vi "Datastream.vi"(0 "Tab Main":T4(tab)=enum."Trap Control (RF)") -> ()   [LabVIEW 2013]
uses:
  <vilib>/rvi/interface/nirviMethod/nirviMethod.xnode
  <vilib>/express/express analysis/Spectral/XNode/ExpressSpectralMeasurementsBlockNode.xnode
  <vilib>/rvi/interface/nirviReadWriteControl/nirviReadWriteControl.xnode
  <vilib>/Analysis/NI_AALBase.lvlib
  <vilib>/express/express analysis/Spectral/Block/exnSpectralBlock spectral measurements PSD poly.vi
  <vilib>/Platform/TimedLoop/XDataNode/XDataNode.xnode
  <vilib>/Platform/TimedLoop/XDataNode/nitl_modes.ctl
  <vilib>/Platform/TimedLoop/XDataNode/XDNodeRunTimeDep.lvlib
  <vilib>/Platform/TimedLoop/XDataNode/wakeup.ctl
  <vilib>/Platform/TimedLoop/XDataNode/timing_clust.ctl
  <vilib>/userdefined/High Color/nirio_resource_hc.ctl
  openfpgaref.8.6.ctl
  <vilib>/Utility/miscctls.llb/LVMinMaxIncTypeDef.ctl
  <vilib>/vision/NI_Vision_Development_Module.lvlib
  <vilib>/rvi/interface/nirviCloseFPGA/nirviCloseFPGA.xnode
  <vilib>/Analysis/baseanly.llb/Mean (DBL).vi
  <vilib>/rvi/errors/niLvFpgaMergeErrorWithErrorCode.vi
  <vilib>/rvi/errors/niLvFpgaAdjustHostInterfaceError.vi
  <vilib>/FPGAPlugInAG/PCIe-7852R/niLvFpga_ReadFifo_PCIe-7852R.vi
  <vilib>/rvi/interface/nirviOpenFPGA/nirviOpenFPGA.xnode
  openfpgaref.initrf.ctl
  FPGA Bitfiles/UHR-FleezersInst_FPGATarget_intitializeRF201804.lvbitx
  <vilib>/FPGAPlugInAG/PCIe-7852R/niLvFpga_ConfigureFifo_PCIe-7852R.vi
  <vilib>/FPGAPlugInAG/PCIe-7852R/niLvFpga_Run_PCIe-7852R.vi
  <vilib>/FPGAPlugInAG/PCIe-7852R/niLvFpga_Close_PCIe-7852R.vi
  <vilib>/FPGAPlugInAG/PCIe-7852R/niLvFpga_Open_PCIe-7852R.vi
  <vilib>/FPGAPlugInAG/PCIe-7852R/niLvFpga_Reset_PCIe-7852R.vi
  NiFpgaLv.dll
  <vilib>/Utility/error.llb/Error Cluster From Error Code.vi
  <vilib>/FPGAPlugInAG/PCIe-7852R/niLvFpga_Abort_PCIe-7852R.vi
  FPGA Bitfiles/UHR-FleezersInst_FPGATarget_UHR-Fleezers_Leonardo042018V4.lvbitx
  <vilib>/express/express analysis/Spectral/Block/exnSpectralBlock spectral measurements PSD WFM.vi
  <vilib>/Waveform/WDTOps.llb/WDT Append Waveforms DBL.vi
  FPGA Bitfiles/UHR-FleezersInst_FPGATarget_UHR-FleezersCont_IqK95Pvv9lYv5.3.lvbitx
panel:
  out "Actual setpoint":fxp<+/-,16,1> format="%.16g"
  in  "Target Force (pN)":dbl=10.5
  out "Current deltaFreq":dbl=20.03845214843774
  out "Tether Extension (nm, calculated)":dbl=1280.0838354247721 format="%0.2f"
  out "Trap X (AI1)":T1={"Trap 1"=0.030792236328125, "Trap 2"=-0.011322021484375}
  out "Trap Positions":waveform(dbl)[](graph)=[{"t0"=timestamp(2751.0000000002074 s since 1904-01-01), "dt"=0.15, "Y"=[-4.784226348419907e-12, -4.784226348419907e-12], "attributes"=variant("NI_ChannelName"=variant(string "Trap 1 Pos."))}, {"t0"=timestamp(2751.0000000002074 s since 1904-01-01), "dt"=0.15, "Y"=[0.0, 0.0], "attributes"=variant("NI_ChannelName"=variant(string "Trap 2 Pos."))}]
  out "Action (%)":dbl(knob)=-100.0 scale=-100.0..100.0
  out "Sigma/Mean 2":dbl=nan caption="Sigma/Mean" format="%#_2g"
  out "Rate sigma (Hz) 2":dbl caption="Sigma (Hz)" format="%0.2f"
  out "APD 2 Rate (Hz)":dbl format="%#_3p"
  out "Waveform Graph":dbl[](graph)=[5.0, 4.0, 2.0, 2.0, 5.0, 3.0, 2.0, 4.0, 0.0, 5.0, 4.0, 3.0, 5.0, 2.0, 4.0, 1.0, 5.0, 3.0, 0.0, 2.0, 2.0, 4.0, 2.0, 1.0, 2.0, 8.0, 2.0, 4.0, 4.0, 3.0, 3.0, 1.0, 5.0, 5.0, 3.0, 2.0, 7.0, 2.0, 4.0, 4.0, 1.0, 1.0, 3.0, 4.0, 3.0, 9.0, 0.0, 6.0, 4.0, 5.0, 2.0, 4.0, 4.0, 4.0, 4.0, 2.0, 3.0, 6.0, 3.0, 4.0, 4.0, 5.0, 5.0, 8.0, 5.0, 4.0, 4.0, 7.0, 4.0, 3.0, 1.0, 4.0, 5.0, 4.0, 2.0, 3.0, 3.0, 1.0, 2.0, 1.0] caption="APD Line Scan"
  in  "APD Ave N":dbl=10.0
  out "Int. Time (s)":dbl=3.0
  out "Sigma/Mean":dbl=nan format="%#_2g"
  out "Rate sigma (Hz)":dbl caption="Sigma (Hz)" format="%0.2f"
  in  "Tab Control 6":T2(tab)
  in  "APD 2 Offset":dbl
  in  "APD 1 Offset":dbl
  out "RMS (Ang)":dbl=0.5623803485708063 format="%_2g"
  in  "Bead Sep. Int. Time (s)":dbl=5.0 caption="Int. Time (s)"
  in  "Offset (nm)":dbl
  out "Mean":dbl=1.039039384389187 caption="Mean (pN)" format="%#_3g"
  out "Force":waveform(dbl)[](graph)=[{"t0"=timestamp(2751.0000000002074 s since 1904-01-01), "dt"=0.15, "Y"=[-1.511324813843883, -1.510992142739303], "attributes"=variant("NI_ChannelName"=variant(string "T1 X"))}, {"t0"=timestamp(2751.0000000002074 s since 1904-01-01), "dt"=0.15, "Y"=[0.567256952484741, 0.566583628488821], "attributes"=variant("NI_ChannelName"=variant(string "T2 X"))}]
  out "APD Chart":waveform(dbl)[](graph)=[{"t0"=timestamp(2751.0000000002074 s since 1904-01-01), "dt"=0.02, "Y"=[0.0, 0.0, 0.0, 0.0, 0.0, 0.0, 0.0, 0.0, 0.0, 0.0, 0.0, 0.0, 0.0, 0.0, 0.0], "attributes"=variant("NI_ChannelName"=variant(string "APD 1"))}, {"t0"=timestamp(2751.0000000002074 s since 1904-01-01), "dt"=0.02, "Y"=[0.0, 0.0, 0.0, 0.0, 0.0, 0.0, 0.0, 0.0, 0.0, 0.0, 0.0, 0.0, 0.0, 0.0, 0.0], "attributes"=variant("NI_ChannelName"=variant(string "APD 2"))}]
  in  "Calibration":u16(ring)=2 items=["None", "Position", "Force"]
  out "T1 X":dbl=-1.511158478291593 caption="T1 X (pN)" format="%0.2f"
  out "T2 X":dbl=0.5669202904867809 caption="T2 X (pN)" format="%0.2f"
  out "Bead Separation":waveform(dbl)(graph)={"t0"=timestamp(2751.0000000002074 s since 1904-01-01), "dt"=0.15, "Y"=[13.487296816964651, 13.48037403257866], "attributes"=variant("NI_ChannelName"=variant(string "T1 X"))}
  out "Bead Mean (nm)":dbl=13.506045465071283 caption="Mean (nm)" format="%0.2f"
  out "Difference":dbl=0.9442381878048121 caption="Difference (pN)" format="%.2g"
  out "APD 2":T3(plugin-control) caption="APD 2 (Cy5)"
  out "APD 1":T3(plugin-control) caption="APD 1 (Cy3)"
  out "Detection Laser Y":T3(plugin-control)
  out "Detection Laser X":T3(plugin-control)
  out "Saved APD":dbl[][](graph) caption="Most Recent Time Trace"
  out "Trap Delta Graph":dbl[](graph)=[195.1277413890926, 194.94364879261857, 195.1277413890926, 194.94364879261857, 195.1457432924014, 195.43991875047658, 195.71957055288706, 195.22283466303207, 195.1027968921228, 194.96782146458364, 195.3831317750734, 195.1011774517534, -429.02175121270034, -525.1398207234975, -525.9023663780167, -523.4888823406284, -525.9473090361441, -523.7419318917771, -524.0949760575616, -524.4391559902058, -526.3291828811887, -525.104560125752, -527.5180711612056, -523.2999128001393, -526.5498888630073, -524.7083600570088, -522.5173776695501, -525.5444120291477, -524.0271757467506, -525.2107691195308, -523.9441905667804, -526.0104515834323, -524.5961470121938, -524.5803642777907, -526.0323679419505, -525.3149691620972, 195.79450497322807, 195.82853060793795, 196.68216279584308, 196.2898441960903, 196.3201650436859, 195.81353342606087, 195.5969971411281, 195.85479324517004, 196.28760584932735, 195.71415572150602, 195.53926387431486, 195.04762359603245, 195.79764921332765, 195.88378244963528, 195.56420539798899, 195.741794878524, 195.6032010481766, 195.13266085703762, 194.68322569301654, 195.35368995164265, 195.60186007511763, 194.99358806317844, 195.21177044926304, 195.52777221791428, 194.99090803446128, 195.33201299997344, 195.42467754091498, 195.65002698602976, 194.27774929170903, 195.22405725927376, 194.985854699991, 194.9996132898822, 194.59974808624202, 195.7220675776397, 196.1457322027774, 195.6360297670298, 195.96840521144586, 195.75840129031178, 195.69255805851046, 196.02312629929207, 195.78888162161752, 195.54391018411803, 195.0409894387586, 195.1408221637013, 194.91519909765543, 194.60594658204025, 195.42734808737038, 195.85580612729714, 195.64566466717764, 195.3641014250282, 195.60986677692284, 195.45013103631618, 195.63127789873494, 195.62251894730127, 195.99686804379996, 195.24774895862328, 195.06110845431786, 194.90555601417262, 195.94974891216094, 195.73211689080654, 195.90340144038692, 194.76751114504316, 195.89818326233888, 196.14575638560157, 195.92471386015143, 196.1084929669487, 195.45133377639888, 196.1373206835992, 195.8163413467349, 195.73025336481143, 194.92953595992012, 194.91910228902657, 195.45385434460823, 194.96091536628842, 195.6577587288838, 194.86529279220602, 196.2093980122397, 195.7594747864935, 196.31704088898084, 196.08130185239867, 196.48443792564595, 196.3348992868127, 196.2353094132675, 195.9846539680845, 195.47411128340255, 196.07032027751424, 195.57883132745593, 195.92315342748176, 195.85849094608133, 195.35857373466646, 195.82252714914577, 196.19266592584984, 196.06829768319847, 196.01367559005777, 196.00825494831406, 195.48130864701162, 196.2637179819214, 196.28036321786578, 196.27834768918302, 195.9718959100877, 196.073961110216, 196.168277786751, 195.9583421843154, 196.86347865832388, 196.2867602914493, 195.78799428339462, 195.98177246709974, 196.13900102930782, 195.92961702885827, 195.43727715700658, 196.06546092635736, 195.6918834481868, 195.88586805630442, 195.04857632560203, 195.62239044470493, 195.69032839316466, 196.0479311245117, 195.8860517125541, 196.07743817657763, 195.3685150169999, 195.35154815641215, 195.28494544155998, 195.66198752530386, 195.05894590580883, 195.52930207065776, 195.84213885187415, 195.270250312172, 194.5866967067168, 195.1520057865041, 194.63999162715328, 194.79036391175285, 194.73194831689696, 194.87558241714495, 195.62504793174674, 195.87081864061898, 195.04954675224616, 195.53796549594406, 195.4517089657777, 194.75239090880007, 195.26541240898192, 195.34084334342066, 194.85592247386344, 195.2100297162633, 194.94549581456255, 195.2667160658109, 195.14476502965616, 195.49592306249042, 195.79311329595134, 195.4708674800024, 194.75395443996715, 194.94709681727662, 196.01273908957424, 195.75008058306295, 195.70936836053775, 194.91080812149102, 194.89789171149482, 194.70971045199803, 193.89929562495644, 193.80041274030728, 194.40324690045244, 194.0311073154403, 194.02319114984687, 194.25570564860837, 194.57546117265005, 194.58434377170832, 194.67543747084193, 194.7473969878548, 194.46456479843326, 193.8038777867239, 194.4581604188575, 194.0567708719643, 194.30607271267488, 194.92391007288865, 194.09807288830496, 194.3748789639088, 194.57307231720893, 194.44126432949685, 194.0117557653911, 192.89703238866568, 193.62791081122523, 193.60939532269603, 193.89644934859842, 194.53132222889602, 194.82081343731693, 194.38390279443533, 194.0012525479571, 195.26222216959474, 194.69722795519345, 195.38021509920873, 194.8573270281239, 195.12432640884418, 195.25967829797577, 195.0898507284719, 195.16239831905807, 195.26944775768956, 195.31153591500367, 195.58319716196473, 195.76877355890178, 195.83960403408346, 195.8370392589554, 195.53000631590126, 196.16564086525855, 196.34263798000939, 195.8933883680877, 195.9151707940182, 195.80431194061444, 195.3372222150889, 195.92415107857158, 196.2964745446386, 196.63500421220948, 196.08233687603504, 195.47185263390796, 196.5818754931753, 196.22140973176298, 196.78008679213448, 196.76596047767455, 196.49098863781165, 196.19992386388378, 196.53797020379224, 196.575766187157, 196.97936702981607, 196.85053141119965, 196.9801672722218, 197.39263003921474, 197.83446346712518, 197.5244908174333, 197.2380008970883, 196.95934976910564, 196.01180980042204, 196.43256420375891, 196.5854667715225, 196.55197882363674, 196.2694654932278, 195.71907476268828, 195.82634298775596, 195.67288078778756, 196.0131850680131, 195.59956348850957, 195.69726536197186, 195.04296079396576, 194.71455960234306, 195.14410588786046, 195.0996201049209, 195.14217745400884, 195.53084374703403, 194.86715896529603, 195.84479012049968, 195.53517964152323, 195.56618039814282, 195.7175436360598, 195.68096667381124, 194.70821036969056, 194.52347606123166, 194.92561086095415, 194.80124578262632, 195.5640837192954, 195.9847215202843, 196.19342135701334, 195.90765267771587, 195.6434435206318, 195.21087823434152, 195.2423992180488, 195.97432124193998, 195.2663250624259, 195.0855628375443, 194.80091416103792, 194.47459153795012, 194.81075498367468, 194.83671226840596, 194.56210196185637, 194.10703186851939, 194.46981481038824, 195.11180930766383, 193.91305219817644, 194.18430948799656, 194.9575411165179, 195.07820912077642, 195.34674885134933, 194.47836161719917, 195.29463805660407, 194.84050999827437, 195.08783111849115, 196.1884163042038, 196.2699018371984, 195.5292119158729, 195.70719232993432, 196.36940129643955, 196.16942126985435, 196.3165764283265, 196.17768578932765, 195.15088353415206, 196.07260691791646, 195.6415891027922, 196.108661317677, 196.47880502982088, 196.52452880433583, 196.68727248008867, 196.44422619042194, 196.39600406355447, 196.26007376364242, 196.6204491434689, 196.4186410090456, 195.8016405243738, 196.50921697938762, 196.58259633169487, 196.67243577614073, 196.2900316470787, 196.23671088707113, 195.8194804876422, 196.16518535142063, 196.39525811959578, 196.24863982455122, 195.8269855866686, 196.54081291328347, 196.21730108688374, 196.19391095115753, 196.18137150608803, 196.55268660065738, 196.1742743563899, 196.08778288288437, 196.60291260155853, 196.54006006546814, 196.80310618780746, 196.43197763196423, 196.35040554044815, 196.4671541475462, 196.2049097757863, 196.1995018668948, 196.43930537222127, 196.4032024932984, 196.08087773133136, 196.1654457677618, 194.30704032663505, 194.66472883168936, 194.65535427206063, 194.73122265123195, 194.22294508643637, 194.21724290353845, 195.0286142357327, 194.88733474368894, 194.5958510601391, 193.81897012957927, 194.39965513804586, 194.30911989595305, 195.00757264606403, 194.39897195475692, 194.80280531139846, 194.96342740324002, 195.37758369709036, 195.84511858630748, 195.28072714210555, 195.63232818111538, 195.67737793086022, 195.60008924848822, 195.6615441091611, 195.25733236105478, 195.11447862337442, 194.91763014472536, 194.3326431389758, 195.54356443200194, 195.41159857074163, 194.68770395597707, 194.1599449535533, 195.36363582231738, 194.4097755136973, 194.55164214258832, 194.435449072337, 194.35313887434836, 194.33667815470136, 194.24468474157248, 194.2621863351487, 194.8867538218054, 195.19463743744896, 194.52931183016503, 194.21932524500096, 194.49538656089823, 194.1072480708982, 194.5534696201468, 194.22744010420928, 194.8542872739206, 193.71302516684005, 194.61903971089458, 193.9507070321269, 193.69954480247395, 194.30996892674085, 193.65166417057253, 193.69637559717873, 193.43911515770657, 194.78014211062734, 194.60606450398814, 194.52636015350427, 193.97328229423835, 194.17940826901872, 194.24259953392726, 194.23630064774665, 194.66895165890557, 194.11122996575915, 194.05615174820468, 194.18420923459277, 193.34126423777033, 193.74941982034994, 194.02821522035066, 194.0143235802746, 194.5717991008229, 194.03019809817712, 194.15932322593778, 194.3911674136095, 194.29192875524998, 193.56380348214665, 192.95633790656558, 193.2013365133113, 193.8506139193916, 194.77516784865435, 194.5528991833616, 194.25360147425582, 192.98559683782972, 193.41911938993405, 193.60977159602885, 193.20952590179087, 194.5058434166223, 194.21209063719593, 194.22170823305427, 193.23243517439985, 193.1127123871724, 192.54648883563667, 192.92238521983057, 192.06859367476207, 192.44140509276582, 193.35890086041124, 193.79014794334574, 193.31056735001624, 193.1665259738477, 193.0388827857606, 192.71990313033305, 192.70330329239854, 192.7122679588063, 192.16677280006456, 192.31602912287073, 192.0943427815283, 192.2820119418231, 192.1158392986349, 193.20070359192638, 192.70871365902408, 192.46853029980988, 192.72811534015727, 193.1788000409978, 192.8693341985182, 192.46521551838663, 193.67564083703763, 193.06520469351142, 193.50016932066208, 192.80541001836727, 193.79229933912217, 193.58954858616968, 193.67582128719323, 192.9037311574721, 193.14449494006413, 193.15973095584442, 193.12103950531363, 194.28317714800906, 194.21254083365224, 193.74671221784445, 193.09919890967458, 192.87734238207454, 193.03679430187267, 193.87237748051479, 193.27024559737947, 193.66799432013477, 193.95690149069807, 194.16492089315312, 193.3065811747802, 193.2837774711388, 193.09561253274575, 193.01059327184754, 192.78761683546705, 192.663255416266, 193.55980370213948, 193.24040973712522, 193.13686947709536, 192.39244762723496, 192.82090494694438, 191.94090598927832, 192.04713180346505, 191.5526769209213, 191.28641504294941, 191.81574333164218, 191.74207311833416, 191.43621977847658, 191.2405059737383, 191.24771653136736, 191.74131024530013, 192.0649596369616, 192.19148253468862, 193.59157032767757, 193.1998221027851, 192.9640603292848, 193.97895901257448, 193.46898284521706, 193.53541329111104, 193.6185982909144, 192.80371343686022, 193.01563848967015, 192.66799142973395, 192.7924233469136, 192.45676375106598, 192.40976045629026, 192.21906102794523, 192.86016782138643, 192.58337912736368, 192.27045957389643, 192.5901304576169, 192.3568525305057, 192.66901308600183, 191.85669308831834, 192.07135419941025, 191.62796553440373, 192.0671644388864, 191.92714520780393, 192.38577475432436, 192.35733041199794, 192.74441784303593, 192.52884324062734, 192.33341422673072, 191.9185101572403, 192.87477604599093, 192.85673854694826, 193.06757755159424, 193.1631221754965, 193.04966121073357, 193.1213975035454, 193.37400225469548, 194.1627499208646, 193.8084620157765, 193.7321356456405, 193.8843407281942, 192.71795172495746, 193.54439590397467, 193.27348714226636, 192.7846248225893, 193.0279461033515, 193.43481950028072, 192.83815393813924, 192.54066379547865, 192.32923485489832, 192.81111835165373, 193.37957491352915, 192.9568944828736, 193.1042479226886, 193.48946801847524, 193.00220096744653, 193.88037287661325, 194.11168966767858, 193.58669080597474, 194.19381976737898, 194.68466295064607, 194.73791107278288, 193.87364925794907, 194.04599057923986, 193.38399371875718, 193.22344366833278, 193.4971347362934, 193.22083366784008, 192.69470990045104, 193.20571265443172, 192.95218272047714, 192.02648380452726, 193.57104885109723, 193.50121752514698, 193.90757358232437, 193.44059973847314, 194.08554655873166, 193.46997590177205, 193.56072623066916, 194.17632006245807, 193.62408119138487, 193.17668554969956, 192.5423219347074, 193.7126269357351, 193.89078914336937, 193.63533823818938, 193.9898962010278, 193.48818778017116, 193.61591375674084, 193.52576127391407, 193.56951285336245, 192.74470045475073, 193.07917877396403, 192.8600777562649, 192.68669541547516, 192.9683465648133, 192.80585511693553, 193.25527147537537, 192.85159117053112, 193.29405807699106, 193.1443122556482, 193.52520298977313, 194.0528551077228, 194.7934476111681, 194.44096891895208, 194.66739013871404, 195.17592945205493, 195.15866506515175, 194.9004811305315, 194.10913524520373, 194.36627181332133, 194.4393959325142, 195.2772829131915, 194.0114140717206, 194.9023642293428, 194.29837644013762, 194.20643924253528, 193.9450673379147, 195.00684849603493, 193.71537067880035, 193.91853312559908, 193.42569085227456, 194.04590805705794, 194.02094630103093, 194.2290305072278, 194.72287086346938, 194.501484602171, 194.45529783511518, 194.8994352870357, 193.57675456052743, 193.65867259748794, 193.67190143887018, 194.70717163867707, 194.41991699917276, 195.4143068845745, 194.6304077052846, 195.64081693525142, 195.14322630262348, 194.94030581030796, 195.01231005264177, 195.04678694616473, 195.31347182315548, 194.87121092959643, 195.0030942815161, 195.54081203906597, 195.41154542350398, 195.83020609312146, 195.28904750547014, 195.07505270182983, 194.94669075808596, 195.13710957596848, 195.29741462786444, 195.40891650935308, 195.02379805363563, 195.13623700503115, 195.29595367090042, 194.9976641459051, 194.8121489929793, 194.85329577095513, 195.66013937053296, 195.04239342081618, 194.28587467238415, 194.20653121724837, 194.2374065045274, 193.99539925124992, 194.76375643498056, 195.29805633182178, 194.5679953783944, 194.60867129694282, 194.3698229115216, 195.60430029047666, 194.28099514951484, 194.63143569668608, 194.35707983482473, 194.60681318037365, 194.84229348847106, 195.09902850311965, 195.137695619025, 194.647730931791, 194.60642059353853, 194.7432410089999, 194.62478788693446, 194.34112778228848, 193.944631425517, 193.60631406555396, 193.8109517870024, 194.3640026344529, 194.1485860478615, 194.44412727798306, 193.9145821450927, 195.31709564463236, 195.428404421401, 195.0560934127227, 194.75344872999446, 194.721769772353, 194.51358268434882, 194.5170195281805, 193.70966946350822, 194.1364054800781, 194.71980119178784, 194.28394175796197, 194.3422998445289, 194.31519880120592, 193.87639094381788, 193.93587478001257, 194.5005168436859, 194.32948537562504, 194.59773770828636, 194.70261575179885, 194.53045322737285, 194.87059323590017, 194.41661229386395, 194.4446677654742, 194.93793458267294, 194.74457398683109, 194.2430294991925, 194.4922544737386, 194.0248974023972, 194.90123369501572, 194.50318649656364, 194.37850403021696, 193.3191410503598, 193.9184273820053, 193.69918121623544, 193.81580819135868, 194.00524747711955, 194.59245896947044, 193.8369730928203, 194.36364588116027, 194.16100021151334, 194.226249782199, 194.1632029388034, 194.35865511881408, 194.37392559584623, 194.89865249009605, 193.8660099379936, 194.43503457839313, 194.1894594532385, 194.41472043789878, 194.27365093149777, 195.25615337690627, 194.2800443838674, 194.0178813174178, 194.72295639964466, 194.9084746551318, 195.1620342982616, 194.9939502088701, 194.9126371433374, 194.92927284376503, 194.23645134185736, 194.59405512800186, 194.50993186791152, 194.59801675640819, 194.949633500534, 194.75392426378946, 194.40343504534133, 194.52520811688404, 194.16311317361254, 194.87344464249588, 195.47458145824078, 195.39570418549187, 195.2938502099509, 195.2058998430147, 195.02258008292463, 195.0331878288569, 195.09163000169818, 195.23456277623202, 194.46804503180383, 194.451228060466, 192.818226505579, 193.21936695829157, 193.8255208213551, 193.99113232942057, 194.038669122063, 193.67222611834262, 193.55372451469594, 192.90710995858603, 193.5531067276803, 193.24463066001027, 192.59722315661452, 192.3700483577156, 192.97633493423714, 192.50935280497376, 192.47135968853576, 193.80654001512045, 194.08250691165034, 193.99547409638433, 194.15360322501365, 194.5665539498847, 194.77924657321535, 194.12506852762925, 194.71964803350727, 193.99352901918613, 194.6430533942662, 194.7839415207895, 194.8438930001213, 193.89786720663693, 194.41376019505628, 194.25937873871788, 194.7453054489786, 194.8827906543466, 194.05549549003277, 194.08703104022322, 194.5113290508469, 193.87547665520748, 194.42061075759838, 194.56150151804698, 194.53975393212573, 194.26591771986688, 194.23343387014086, 195.05276528960343, 194.68676699559848, 194.41024997012573, 194.78441757982256, 195.56715138805436, 195.69030456620303, 196.04383341725605, 195.6577607827503, 196.1027697087297, 194.9568548575708, 194.824216124434, 194.97576250901975, 195.010158058172, 195.0269760143274, 195.4205598203613, 194.81357467939932, 194.63905920593325, 194.9614403360289, 194.73971556431655, 194.75682862628747, 194.84265245695957, 195.1323478168085, 195.19068791895532, 195.22981901673066, 194.8743771528704, 194.24550077104033, 194.28979871373832, 194.59392600904619, 194.779481078806, 195.70705842979552, 194.7566261314893, 195.26349160195727, 194.77165713222504, 194.36946161999265, 195.21909913218636, 195.3669041744504, 195.76404258751694, 195.947887283831, 194.55194484412323, 194.80824313587772, 194.77157334093775, 194.18009532363456, 195.04962885338807, 194.60629729208733, 194.90839930488553, 194.56946754803846, 193.99374435316844, 194.6810730719125, 194.86852444640292, 194.4924721371618, 194.95637557577803, 195.13478588676276, 195.38050749043825, 194.78983154190118, 194.83456463640013, 194.32235859435102, 195.67517738429373, 196.15532830799532, 195.33001983035538, 195.18685910851437, 195.12087583623688, 195.4222387037011, 194.97529659559243, 194.4018380371024, 195.6943699599037, 195.38136018613483, 196.00597591629764, 194.8543456557395, 195.156726090314, 194.731358718926, 193.90004113846422, 194.60950408481727, 193.98545052017897, 194.20080031940742, 194.637252561261, 194.9737106544493, 194.4673524273019, 194.52277430244095, 194.23274763995946, 194.73761057768812, -1.181138255103479, -0.9306612010476698, -0.968697403030232, -0.678816234800252, -0.5560113191591722, -0.4127948071346603, -0.7408470265185336, -0.8480834757737306, -1.0222956314732552, -0.5563786473367922, -0.6418676273555444, -1.2379838563538788, -1.0448697771569941, -1.2372615645938483, -1.6257163283095042, -0.9082354464276396, -1.0242831432790216, -1.1086673647503074, -0.9068727581792908, -0.5190992479509662, -0.4329529060155246, -0.6921237117365915, -1.477156136548249, -0.6807994529225017, -0.7388181038842601, -0.5994707305280262, -1.3281974180488163, -1.1353516882326016, -0.7088383308748933, -1.0274732562996767, -0.6065968003155602, -1.3085944461130268, -0.7661789188806116, -1.1420934946254135, -1.1702478542604915, -0.781602618432724, -1.2012502071892412, -0.9973756771573492, -0.8568881497148246, -0.49425589259117464, -0.9166795925932667, -1.3269864601168613, -0.9182701383355583, -0.7850817917079325, -1.1677923940618449, -0.8204650639218696, -0.7746912042816816, -0.7038488013784088, -1.309462258801505, -0.5958262948242079, -1.0436911456846087, -1.169155553674131, -0.665621790183184, -0.7462416800662273, -0.6910849420477647, -0.6971459724697611, -0.4221445066202163, -1.2493169860682425, -1.406585973419622, -1.0720217246747628, -1.1715994313971696, -1.5258142587014083, -1.1961076591271742, -0.7364053702721676, -1.2195907750064032, -0.9404195726959337, -1.1702950257828069, -0.3711370569602539, -0.9912402964341505, -0.9571005338795922, -1.1074228297493405, -1.266791708511818, -1.1815876194650379, -1.0169525198467362, -0.7364878992502963, -0.8894863894314788, -1.3060005507963233, -0.8342775126161777, -0.9882817866601372, -1.1132789395451401, -0.8479240880011987, -1.0337805905653599, -0.7940971945091877, -1.1503947002112471, -1.2025216621937513, -0.950495964006143, -1.1310221708559887, -1.1050195861421104, -1.1287669873429498, -0.7889214296357241, -1.0220959999223007, -0.9882349027086792, -0.8345184927457132, -0.6978300372188491, -1.1466472317286471, -0.563238729564544, -0.6921745162229245, -0.6537528501936611, -1.0440620431160719, -0.4073378725340491, 11.154952105080923, 10.477872520209203, 10.43494522215152, 9.89510912740074, 9.933179714778685, 9.349136327710386, 9.65964853707204, 9.289632966890554, 9.479632186983054, 9.051483663412565, 8.463894597215319, 8.339417435576323, 8.340843719323859, 8.47211947351163, 8.824545874808024, 7.90359998372694, 7.933833536254328, 7.975535484935174, 7.680553283667431, 7.679946529727328, 8.153372304559573, 7.8368271611012466, 7.605794344154638, 7.711158693673921, 7.868856857006886, 7.291304315927828, 7.210759865513816, 7.429958966537178, 7.3154814826274475, 7.499416537690106, 7.241807839159601, 7.493887616612923, 8.064065742016377, 8.1043153942267, 7.832850984054888, 7.761204475466879, 8.250507372321746, 7.757476580801014, 7.964224325524025, 8.385268583080702, 8.122022261310223, 8.267339430956149, 8.515131135634864, 8.618045620654247, 8.951268577733215, 8.544545827482771, 9.001257459105029, 9.333454227490012, 9.052596353746903, 9.731599488679166, 9.715094760302811, 9.723423794897887, 9.556463961236027, 10.459167408538852, 10.868418385346281, 11.020027214387863, -1.4457845653758916, -3.023268292240515, -4.154664410465992, -6.668532241264293, -8.850183233615645, -10.86431389929157, -13.850132208660863, -17.19279194073515, -21.85801201579043, -26.088628225765884, -32.104704168792296, -38.16843290845312, -45.83146135122661, -53.94509072709745, -63.14698315041828, -72.67062764899414, -82.87304530964586, -94.39433196750909, -106.00593342017147, -118.24070155251609, -125.3204907372069, -132.63232801211478, -145.4899318726121, -158.65518840858337, -171.87672948504053, -185.1293343979983, -198.85004395233537, -211.98216967406464, -211.5284472162117, -198.0631970714449, -184.49459849659073, -170.9347653615273, -157.3880007601632, -144.0100375564163, -131.7862475042209, -123.87560960265046, -117.25854227362635, -105.41214293313234, -93.91104405470622, -82.62793062823654, -72.30068676439792, -62.668788629910395, -53.51041378154629, -45.49587327568823, -38.42304531502697, -31.58838934164615, -26.23051625875261, -21.62893915296762, -17.36691779425857, -13.73571744562537, -10.979747157255638, -8.690768472031039, -6.730374452808182, -4.371269800428158, -2.8965602581654717, -1.93422207774079, -0.4003482182789633, -0.268466419462308, -0.16360446918836502, -0.24410982088309058, -0.4959641819081818, -0.24653370321507867, -0.16923224975874585, -0.5238073335296733, -0.3647660222546121, -0.3658154175791622, 0.1612110082935383, -0.3622105387146643, -0.5994717881763542, -0.09701276946070114, 0.10785832233334691, -0.24287546040553473, -0.3121191611961694, -0.5233152333550284, 0.14874588967650548, -0.6858296085420853, -0.13631478866462698, 0.016529970207016242, -0.4556148631420889, -0.0014818995327366413, -0.3730053961436903, -0.051660525376146404, 0.05745606794886732, -0.09728588482332312, -0.0795508288620185, -0.27454251697094606, 0.032573669651277004, -0.5284999763367715, -0.47659730740020634, 0.08997024413310323, -0.08778634107573982, -0.6922186091249137, -0.7764272051021863, 0.010313340320275144, -0.5975194307390227, -0.15289553091393615, -0.09448127102174819, -0.36662188267750967, -0.291900872705602, -0.23897484488627702, -0.3691012578907352, -0.22066199968620936, 0.13484208801123276, -0.28505840452089826, -0.4189912200496282, -0.08527041517092027, -0.13137304350173573, -0.6812485630823996, -0.37268634759383, 0.06153482204309335, -0.3210139229822432, 0.024066981842467472, -0.3784150474652246, -0.4035409981674658, -0.31629719811781143, -0.21733669266051614, 0.1403607465244281, -0.20108565110209908, -0.0334989225074428, -0.7131640209955665, -0.008283537169177069, -0.10410270961637447, -0.7005327434777248, -0.6375139225980262, -0.1967021333427923, -0.4999719858588917, -0.4125226903637681, -0.15214522151034704, -0.4653484570496326, -0.05683458280531983, 0.07597987759528291, -0.200166769994792, -0.5312128487854051, -0.21912307852912571, -0.27479519550989384, -0.1217214242907867, -0.13592805301805322, -0.09504090319167058, 0.18306036952676907, -0.30334973152022937, -0.0668015864304018, -0.002031001694032253, -0.41183755997104565, -0.5238763835087941, -0.014762064778398032, -0.20708055738365005, -0.765605361803882, -0.2215386931403025, -0.45553093595800637, -0.47049153287583384, -0.5037158560133776, -0.21333163635080488, -0.06602474675418857, -0.18677195432853277, -0.030083866546450844, -0.4659262786423081, -0.3782800560153974, -0.2882719782684533, -0.533960162642943, -0.2760402187016064, -0.5794724901254118, -0.28422949762890354, -0.3029201280188493, -0.13197105407556553, -0.3806528517903496, -0.2413942388503999, -0.1721212928016026, -0.45231230265985356, -0.2335147388027593, 0.1980271577688154, 0.05811690060175212, -0.6489983230354981, -0.02470307340653788, -0.11366370934118908, -0.3126087490796654, -0.051051450039286794, -0.25334810059245083, -0.42665693649162895, -0.40317662083928285, -0.40294034476870594, -0.21426400472946872, -0.04027223842972372, -0.4448269062120699, -0.5556613924247797, -0.011379218946074743, -0.06903910529703539, 0.1210881790036159, -0.4002154323598608, 0.0513405094636149, -0.5108641793254198, -0.3307126623655845, -0.038793910290931155, 0.21987026846631452, -0.13069965777319648, -0.1819820976978921, -0.4061128334220707, -0.23233445876404146, -0.21784579014018812, 0.2041022705071509, 0.07348563542567976, -0.1152909470202379, -0.31721014421313687, 0.3788163074933094, -0.12209198791843279, -0.24069574312894726, -0.18065669720134825, -0.02047655128979553, -0.1851714313482875, -0.5255208558924139, -0.2558007212867448, -0.15840817836840393, 0.303638134063559, -0.6328939314915305, 0.09466138882523167, -0.35261535931591337, -0.019585098826367275, 0.09100368643699519, 0.1621172079354638, -0.4105394739937325, -0.2126743324503957, -0.2703370562974967, -0.2517955610183842, 0.14364668396202007, -0.7488799171411541, 0.021290725337112848, -0.33481807938530517, -0.1686647423017794, -0.0087701175484034, -0.7908262538991352, -0.29154448836299507, -0.5666767203941292, -0.09427221985297585, -0.4569994536186478, -0.34233902145513295, 0.1818393306593813, -0.34699175328680876, -0.5612031837941422, -0.2094915449082917, -0.2826552538900906, -0.13293581458524206, -0.3869360858178711, -0.8100542276330879, -0.1273044517106957, -0.38718489525341915, 0.12390346658815132, -0.6790662580765772, -1.089908691798595, -0.16817951838614387, 0.007636498942218406, -0.25832112901424664, 0.09324635304798001, -0.4471106429408635, 0.14391930531390407, -0.09330029825259156, -0.7842918714677807, -0.5467228576051039, -0.307257078043437, -0.11087579623947813, -0.20682582692623497, -0.46990427527514145, -0.5101931273880314, -0.2761812914109637, -0.20175954604678215, -0.22534458217562636, -0.3984364268846021, -0.2354207368245851, -0.8508320024121924, -0.12342746793590753, -0.34407018937679723, -0.5241976267436832, -0.12022330007904602, -0.2747149884105492, -0.08654690137992804, 0.12157708170854276, -0.06551357930019519, -0.5836800603647656, -0.0004656223845622698, -0.049843414946024844, -0.41593524313210184, 0.2157299762409508, -0.07676665267579108, 0.15031522580948964, -0.17362501155395993, -0.15596738018039424, -0.6171658246397104, -0.2969334293209033, -0.021180188399525512, -0.7959913600629194, -0.07630225261447143, -0.19194168909257647, -0.33821174297839307, 0.5709727817869396, -0.34827366253339087, -0.5349749385605537, -0.09000731512979532, -0.1867526605282378, -0.301012260183506, 0.29019150805320404, -0.08875522841719907, 0.038907934906715624, -0.46386761953670375, 0.12250108878861143, -0.05289854280495121, -0.22315723410823518, -0.043032096339945314, -0.04893127592718882, -0.3514771004373216, -0.029221027610788264, -0.20097986421360714, -1.05306224286927, -0.6114054395320072, -0.23694303698371888, -0.35806358800362226, -0.20819283254667398, 0.13042785650564825, 0.34476399469339647, 0.6205383449009672, 0.04591989294455634, -0.08269813571280582, -0.10267241006421668, 0.13354238261047557, -0.49669424431333375, 0.06473163130509962, -0.26267818376964036, 0.5074445333930585, 0.2413601937336769, 0.11439937734771088, -0.0037242085933533176, -0.01967342681621531, -0.5021093609685235, -0.24119494376530315, -0.35251030211921186, -0.035549066539892316, -0.27187442416289254, -0.34216166532548487, -0.16250037408419993, -0.5120184980956692, -0.3408056270061184, -0.05108972057397343, -0.03551887983503177, -0.1489388837326029, -0.21693038448841695, -0.6059634018552732, -0.14580206536651086, -0.2883437156999552, -0.17223323572511384, -0.46086812987267267, 0.11308377614472398, -0.09484136868919812, 0.21212695783765867, -0.08982731659180387, -0.45072348238573956, -0.11660184595283374, -0.5197312649597258, -0.1590792225662917, -0.2976140385920055, -0.2510614720920258, -0.49806590198980294, -0.42621931328829754, -0.023109617434310503, 0.045972158655654294, -0.26999020816569047, -0.19281765421372882, -0.3266615781840355, -0.3067467153654867, -0.0647415491900385, 0.084274228301912, -0.5248734797464332, -0.1463933090383006, -0.8809021078312524, -0.32324618020988216, -0.10697274406201979, -0.3071225744111721, -0.23398242965515437, 0.1338199230891336, -0.16447171493131352, -0.057722376256272856, -0.38820377305166426, -0.17964880375697356, 0.3059897728205956, -0.31312165571365114, -0.30651344943299025, -0.06721161554854171, -0.4346286869708339, -0.5987781924821751, -0.14296709913526362, -0.03815596251803388, -0.11269431437581445, -0.09079534105561127, -0.44483019277077074, -0.2504967666936232, -0.43089778955502867, -0.25247405207642126, -0.28143724627501365, -0.2778693744942181, 0.009082265501091369, -0.3758316534986055, -0.2681477975584319, -0.3552501015866808, -0.3542966021663698, 0.159257343366896, -0.08557998811112066, 0.634124239690215, 0.021661674558361765, -0.008896997078086555, -0.12067845395755294, -0.3843878378578116, -0.01838732219742767, 0.4445720751525627, 0.041246066869853104, -0.2944000731264599, -0.6996288473868282, 0.09313210038528807, 0.12584448026351336, -0.3874153002397561, -0.7041798988712322, -0.5559437030611865, -0.37675956144835077, -0.11820889511749888, 0.1922172348998441, -0.15688371439208515, 0.11119668218355572, -0.08365493108811606, -0.35690632160430713, -0.27887771037038256, 0.10105950968481148, -0.28378911623955905, 0.2689564673297382, -0.41395951783402585, -0.1279323815856951, -0.13995556773994955, -0.4185514309612067, -0.09971993363991538, -0.273333282640864, -0.19875980957768669, -0.30097463567126403, -0.00913995239022758, -0.09006755964861335, -0.13520552234465388, -0.12539004858533587, -0.2192860789849439, -0.22886855144859275, -0.14189127956923142, 0.09414830699518073, -0.06123822901533815, -0.3650678853735849, 14.58674543997585, 14.58086853086594, 14.874029532086357, 14.74606356131514, 14.634679023324686, 14.413703314420282, 14.116005070713292, 14.713145715101806, 14.692431770347197, 14.730111044630874, 14.877621224724187, 14.377874925443294, 14.112798364413347, 15.028348263927588, 14.203248372689902, 14.66070475228214, 15.302764020955703, 14.636660603832844, 14.422230568609773, 15.23315366556353, 14.044282663649616, 14.737794735672823, 13.940514961236067, 14.589449147346782, 14.425672237609131, 14.416145548371064, 14.852487668491847, 14.566129285481223, 15.334618343113169, 14.053863435574268, 14.879141625650618, 15.067556309753455, 15.41208376062141, 14.607663205453516, 14.893956925913233, 15.05362544780561, 15.102185519836786, 14.77619835143903, 14.084531931230002, 14.524176201904636, 14.71944350002321, 14.940750014555425, 14.60629149989373, 14.943121133617339, 14.847325698391002, 14.383364451932355, 14.958433512392705, 14.606220227973058, 14.89489649111278, 14.900776283709147, 14.398468885978184, 15.326384296821002, 14.97238427149251, 14.866421830707486, 15.272957395031648, 14.544889088680542, 14.406356036182578, 14.544014562132707, 14.595500804297815, 14.834609807509135, 15.229531864953051, 14.835055157742136, 14.747596940062389, 14.170905036002052, 14.206095976497163, 14.530398434656975, 14.784887331146795, 14.314838709804533, 14.776979653447953, 14.434567743078674, 14.80193218375885, 14.833783059181783, 14.816773043923872, 14.695160903327304, 14.816751295739188, 14.603798567711785, 14.791503438203646, 14.644427239666324, 14.346813486445228, 14.602590077275739, 14.32118424340111, 14.782415382163633, 15.076045713457336, 14.529531351203925, 14.78132699392687, 15.009139650856767, 15.079703090967582, 14.37442383958873, 15.01026611958403, 14.404423356340105, 14.72169896457567, 14.597223008148259, 15.105489951922412, 14.284936874591981, 14.302001116956859, 14.127095414658651, 14.660257462017631, 14.742936661815683, 14.483122142327275, 14.582366265315613, 15.275438902211485, 14.638402021123765, 15.102971209412331, 14.339437763696688, 14.695840244536484, 14.348787284017671, 14.941823459504533, 14.988346272486599, 14.892801246087805, 14.680147858355268, 14.862205758798606, 15.137916727483496, 14.529593339136946, 14.645227374774134, 14.69915608302531, 14.881573354564413, 14.308820809064285, 15.05527053114089, 14.552651062148824, 14.368033176517818, 15.05156135077882, 15.376311040251625, 15.495321141780245, 14.644538305599037, 14.530728475052818, 14.90694792193477, 14.46259754723406, 14.83799031587843, 15.140671555996626, 14.672585125371615, 14.270287301745235, 14.692377963106509, 14.503017990885983, 14.126202131103831, 14.534188343478862, 14.758766618184056, 15.305987337918076, 14.287633530486035, 14.469020086702004, 14.165159245796994, 15.179992703336824, 15.368599812895965, 15.513838500491067, 14.357527959071637, 14.67103892152834, 14.718908180249995, 14.572332796620232, 14.751507922826276, 14.773746868921956, 14.83568273187342, 14.440673008507323, 14.40992208707178, 14.074382365895527, 14.67880613813646, 14.947177344046953, 14.63497688221762, 14.238409760045506, 14.668579646772853, 14.91321181349657, 14.810228227698445, 14.727900736991732, 14.808092520827206, 14.876766033697507, 14.879293069275889, 15.08505337024418, 15.10348425284057, 15.11889626590774, 14.921216254068629, 15.037155917980723, 14.929893165111633, 15.504466890316454, 14.379450300817258, 14.52062062590487, 14.635486783710148, 14.477204687484598, 14.834340951259422, 14.263551913983846, 14.129210279052966, 14.662689634011052, 14.297483768503831, 14.224736688059135, 14.076311459853095, 14.708738505307615, 14.102414781489472, 14.948612214796608, 15.787525492101151, 15.524926912717628, 15.862635316751149, 15.260252564624084, 15.45932470579366, 15.296299899917054, 14.797318124560704, 14.668978891775666, 13.833004423238375, 14.884525963522504, 14.167442376533996, 14.554812475005683, 13.989917936779781, 14.349315364834206, 14.392875747875895, 14.491032340950731, 14.748052138015517, 15.133264327323774, 14.908373914681743, 14.30384856586024, 13.967458696316388, 15.457068170870967, 14.696945686160337, 14.368669988991824, 14.855721542961714, 14.77614555125433, 15.025059896138249, 14.87944820008602, 14.632886671111159, 14.598982907315524, 14.556659257334616, 14.760999893572796, 14.072857699680545, 14.208951753393261, 14.933006712078665, 14.825509610336153, 14.603817210102537, 14.502572893905352, 14.674262531782093, 14.69880928408708, 14.897890755726051, 15.130187598020614, 14.699471796075585, 14.812893492771483, 14.330125703669902, 14.825877557624738, 14.814231618398438, 15.421183660100006, 14.526061057389068, 14.301110067176086, 14.190782960637954, 14.087264265918028, 14.841283459995442, 14.468874593848604, 14.913694700797087, 14.661986964687914, 15.203304308335925, 15.475333005130793, 14.85266709671909, 14.643037183340429, 15.073735394579035, 14.899344463483505, 14.880127946507354, 14.834145900155209, 14.536951744513582, 15.355128088568636, 14.760136347520824, 15.212607369838395, 14.677427818156902, 14.810912796338174, 14.69269128532416, 14.02605968657589, 14.486395072845127, 14.29469071240165, 15.749617439132722, 14.609560110166534, 14.790695263936966, 14.61882166960561, 14.81523989386789, 14.89163888927931, 14.154428144592986, 14.587214767568197, 14.558798961108613, 14.739468245742769, 14.552443143668192, 14.710635784683591, 14.885868549397445, 14.163825084088698, 14.165268439677263, 15.034306577063447, 14.97296079443682, 15.113375945279952, 14.56601427767967, 15.008962754490693, 14.757235262352413, 15.09282113688066, 15.155959347307622, 14.893292065442328, 14.79599941353292, 14.805909894780525, 15.314874216930084, 15.329524235648044, 14.528916517777114, 14.77276826436076, 14.659843602018812, 14.326257931167174, 14.516747017389564, 14.207416937651999, 15.000727645549972, 15.000992464442069, 14.790889516290013, 14.772990076156894, 14.486334030988122, 14.323503901697789, 14.895153796144514, 14.23147454922834, 14.52412510469905, 14.611187362245264, 15.238307811114725, 14.389247610356422, 15.188765474797076, 15.514828247709387, 14.708906874268678, 14.886704042714658, 14.673348900663912, 14.514265627625326, 14.968818210509756, 14.477554564994032, 14.66555448893747, 14.585668148632593, 14.558627267385987, 14.131051542687706, 14.68642385433418, 14.658289994664603, 14.274808359245522, 14.810116576093817, 15.071810260116685, 14.818704654906144, 15.348504341182803, 15.278672286989144, 14.408109424515663, 14.802269801579454, 15.021775384529036, 14.798928882887534, 14.284479334773147, 14.721482755417838, 14.143686579099306, 14.93290104564803, 14.46744831884087, 14.366312257950637, 14.70801711777066, 14.788485833677425, 14.87699405875761, 14.33688389986622, 13.962954801216835, 14.15084951133311, 14.042292777939313, 14.90556094188048, 14.448977652339291, 14.39010364042913, 14.585503090275342, 14.26266675029999, 15.092635206955425, 14.898089833357007, 14.523388852755213, 14.738618983578426, 15.275276291614556, 15.003203764692575, 14.526961982760609, 14.453491482988804, 14.300125594292787, 14.085062163297328, 14.85399636682719, 14.672723976334833, 14.390788502630366, 14.794711865570164, 14.621890180482751, 14.295388033184421, 15.796319807144878, 15.487196186563281, 15.201368202428595, 14.749542990524565, 14.78683946797301, 14.453620322607128, 14.421501353012104, 13.959172283048353, 14.726499370638074, 14.784312165341063, 14.88061915372863, 15.166598749980805, 14.47231013316989, 15.497000414443232, 14.268500020674793, 14.648145044222348, 14.806190094250809, 15.24998607141454, 14.675389722468513, 14.65791845285019, 14.901136151593873, 14.431295496085403, 14.290847144769872, 14.24447139894798, 14.792349204583244, 14.614396564393932, 14.54734207295917, 14.978927915527473, 14.695260493128927, 14.985631848826788, 14.251086610121947, 14.53082103249701, 14.600611602099562, 14.29773315102109, 14.46128356704596, 14.549216493376688, 14.77345816516152, 14.557527152323427, 14.232661669637395, 14.844223456582846, 14.277168324284794, 14.758139613594041, 14.639835896501406, 14.625179232335297, 14.885420394022033, 15.339542586279443, 14.085467433275053, 14.95927750618667, -66.06084534839279, -153.5687587415229, -151.73227656412828, -150.8849374320742, -149.88921368841815, -149.7434948463669, -149.32213586968064, -148.42013138702583, -148.79721403068248, -149.3042686018203, -149.51045096838556, -150.68724885182112, -149.8096505665673, -149.69780499660249, -150.28400398623373, -150.67615222441108, -149.60113231479602, -150.11081223999187, -148.83880044942507, -148.21801543658947, -148.86192359695576, -149.27232640619496, -149.7801596898833, -149.4512824775526, -150.04369431178992, -149.54969404473, -147.98649036665503, -148.80654777222207, -149.498566152966, -150.11182253309488, -149.91830031006938, -149.91651646112422, -149.08205344938727, -149.68170229465056, -149.72426218329878, -149.3293791988728, -150.14071102794142, -149.8430952788477, -148.9083792110304, -149.7769522409082, -149.59229088909814, -149.16837001958498, -149.04391317387916, -148.72196239941556, -149.1236986996601, -149.20640542897684, -148.95647719912745, -149.1724570853978, -148.92045852308516, -149.53946655755374, -149.63741914053054, -149.7333801237655, -149.51565938570923, -148.9172547076595, -149.23048627758578, -149.32745185633746, -148.36661434934854, -149.96171865770583, -149.56819528214618, -149.67978453994058, -150.19453806146328, -149.76301199908912, -150.01392419630886, -124.7198894723075, 18.955412619127603, 18.81750146953981, 19.176982860723925, 18.908439659937965, 18.851845780441597, 18.7300453668233, 18.838443095038702, 18.62681078104262, 18.61114861986854, 18.901297322734486, 19.138021135554272, 18.847635937378797, 19.142351426544224, 18.987593943253444, 19.139432820352678, 18.956283548835007, 18.3068258966927, 18.10735779102941, 17.743692691717573, 17.802564159422733, 18.0149181545895, 18.674168398672663, 19.118380930634892, 19.099405375131195, 7.460639649864058, 16.121348204860713, 16.342298527662415, 16.00379978872999, 16.215564979071807, 15.950753718657786, 15.925459492969422, 15.94889321224302, 16.350272447845352, 16.419032487440557, 16.087300547760055, 16.320456918005235, 16.05548405398671, 16.1347934488961, 16.410949637180774, 16.364155407356083, 15.68947281474842, 16.106915802414225, 16.248776699748408, 15.805364961710664, 16.041118051316534, 16.406356189066745, 15.991913527476001, 16.27261885541458, 15.98429568263203, 16.4585182176367, 16.12276694465873, 16.19315917934673, 15.371440404308172, 15.702157092833648, 15.812307077784919, 15.620164095080401, 16.064688806204583, 16.293325258372295, 16.533960458568806, 15.623652201942924, 15.445487590407634, 15.97212452345662, 15.845651606982662, 16.001176358694675, 16.27914251023148, 16.36964033873429, 16.29051294234939, 15.538354564850916, 15.728077973627334, 16.47253054332538, 16.482050881128163, 16.08918117299733, 15.730491465319611, 16.15381480061373, 16.46737881326507, 15.814334645290447, 16.462719458805864, 15.787789715364331, 16.41814002712438, 16.051492170025565, 15.971162135999933, 16.24667568849787, 15.360142321722423, 16.184643685910075, 15.727409482986914, 15.784620995662491, 16.17189475441712, 16.85580302279279, 15.755738017007566, 15.294893587960185, 16.156970077723, 16.15331738854412, 15.904551128583929, 16.401265174611307, 15.586314186230776, 16.09968760796412, 15.61649671464918, 15.861384354928518, 15.925190304638418, 15.938492134741603, 16.069767107273133, 16.305778385270344, 16.342946566696355, 16.248129513040073, 16.52115562473159, 16.217376435434133, 15.75119392527804, 16.008974443557268, 15.861046371271982, 16.206734306603266, 16.344783902787075, 15.865893502111698, 15.860454957202464, 16.119730728691312, 15.686106403036922, 15.776229681230118, 16.50641251403726, 16.75097919504658, 15.841613793229659, 15.970862230380646, 15.4493388952522, 16.384765006499716, 16.296260119583287, 16.472661897931523, 16.09637047132635, 15.832189572422749, 15.657257760945951, 16.13091310852894, 15.542949273253038, 15.610518059063617, 16.264255517264168, 16.026159799417794, 16.06977326879347, 15.982709329861223, 15.680141859526968, 15.930106762330377, 15.702103163703656, 16.332159899704227, 16.710402964858737, 15.493549109697696, 16.210183486309187, 15.822826698500137, 15.497574104248548, 16.052638859949447, 15.478616888392898, 16.057710436328087, 16.149234031846138, 15.704416189163318, 16.27339054959906, 15.451686543238756, 16.048346533729365, 15.855240669086418, 15.708920088024975, 15.69298713536044, 16.287522105485426, 16.357590673236643, 15.703704263774036, 15.905672457859142, 15.610981680356403, 15.891310219811192, 16.022954710083873, 16.081274670191867, 15.948866340800375, 15.832564515939733, 16.338214574475195, 15.869617245853773, 16.566940056792767, 15.970925042590258, 16.42570693195622, 16.42563005122146, 16.324699527391225, 16.012351014860986, 16.68098198510074, 15.910636925794272, 16.11354885746317, 16.443600144809462, 15.799448655147543, 17.1461154172168, 16.03981995134166, 16.45609913595291, 16.437746596187953, 16.56160902767857, 16.143281553720204, 15.684448169023348, 15.520496006253284, 16.106254118153444, 15.819646306170812, 16.141213451013133, 15.89782063479612, 15.718638795206646, 16.196536847517223, 15.872983589943455, 16.69793312466312, 16.14457836605638, 15.959815898324841, 16.135632464426923, 16.429895602212568, 16.147600029118724, 16.27982830250454, 16.52207227650164, 15.165116803280156, 15.776252163577698, 16.348095337076522, 15.794284585357989, 16.028931835978412, 15.658431491195858, 15.954074347266271, 15.88747342161146, 16.36759205757102, 15.5114698768101, 16.250460512486995, 16.072863361801755, 15.273689399948907, 15.77617732743431, 16.234902257299403, 15.587180969286361, 16.285275845099683, 15.921566572622039, 16.470076839576855, 16.201387797677693, 16.027971633360625, 15.821344300181021, 16.58887932642244, 16.37878720649485, 15.930180842881356, 16.322581541729562, 16.409760788663302, 16.500311364124205, 15.419560736572793, 16.283821863547413, 15.688168992047439, 15.186223358198038, 16.357616028387252, 15.899677552009175, 16.11352808450296, 16.416922194993912, 16.06041981617731, 16.168667112474758, 15.862779637351064, 16.19207629968246, 16.082595035090502, 15.849823812645267, 15.882869870479988, 16.084379681300828, 15.787947695074855, 15.517459799515072, 15.823252185483186, 16.35424573251734, 16.30701679688489, 15.724670757435273, 15.990586356523828, 16.439984935533325, 16.338616971334083, 15.847941145120569, 15.767721855639223, 16.071120357425222, 15.931410525708975, 15.811123467989201, 16.832810425671532, 16.27166051984065, 16.5582922355308, 15.85009134721945, 16.124245603664125, 15.62577492364174, 16.5452731492298, 15.230137576186348, 16.210749930760997, 16.098907610058458, 16.367188620252193, 16.72062851102455, 15.12594139443341, 16.605357469723653, 16.79880197363862, 15.933497554062555, 16.172449432844036, 16.760314345841902, 16.357667129655873, 16.367136069778464, 15.808330497761395, 16.883714335439343, 16.576590100294315, 16.288596142105902, 16.229827021025855, 16.329363044767934, 16.346089126407744, 16.648552105185654, 16.46289034367319, 16.315861496515364, 17.05537632969269, 16.495917187737156, 16.933029194570345, 15.869578855723992, 16.059316663980724, 15.346432077653018, 16.289110687165817, 16.02968992876552, 15.769605035193972, 15.695481564065005, 15.290292375417646, 15.89593197795679, 15.821932648673087, 15.822152008042696, 16.172317366544277, 15.907073836457801, 15.335264429465015, 15.308690344629541, 15.409736870824785, 15.171493051944926, 15.421192653595016, 15.159759966241985, 15.161633886690876, 16.162311438679062, 15.42362308717467, 15.800981018479606, 14.741987354006634, 15.31530109589752, 14.952291012234825, 13.969140739481352, 15.315755390011491, 15.971987960769352, 16.05251868530575, 16.11641286706037, 15.477204335483625, 16.59941815533531, 15.696191342596407, 15.825634677188154, 15.81848582229084, 15.966467404196667, 15.181212353889038, 16.064192686639156, 16.008329155267532, 15.995950138373562, 15.487548766897351, 16.245585999924895, 16.319571714043963, 15.82368966700067, 15.65144481174739, 16.153732390039487, 15.778638297912957, 16.185269130701972, 15.731242539389353, 16.165971779236298, 15.63402707575083, 15.441048072675562, 16.021633851151876, 16.079865019235633, 16.204158769966977, 15.38435286319651, 16.173159837931696, 15.82331405266458, 15.922830206729568, 15.806959738212125, 15.483182439577716, 15.765666673683414, 16.921623312775495, 16.453403571262527, 16.04729195268181, 16.8494871384484, 16.555320688609093, 15.82675805366985, 15.93830176982405, 16.141294607343895, 16.313468084772488, 16.206280334394638, 16.352282887773224, 16.399384857534713, 16.7249300728221, 15.50939837356284, 15.91207565589798, 16.559222545245753, 16.25644661873024, 15.977761275421216, 16.195875111604572, 16.092952332922238, 16.003926094558864, 15.42226856399498, 16.500100471452537, 16.16263957041963, 15.502773435207873, 16.10685695471974, 15.915074490950392, 16.359036767257287, 16.079810116951105, 15.876698483591799, 15.960017235365385, 16.375739222665075, 16.243181244200407, 16.10676092146461, 15.597809551696502, 15.964787352713746, 16.19007900365015, 15.890455801176532, 16.06382690322697, 15.734690104549125, 15.822100320590227, 15.90032375765765, 15.925239930501416, 15.905615331872934, 15.815751948011114, 16.19624322543973, 15.680856931080934, 16.36034473726673, 15.826819825934209, 17.00515509521744, 16.49020217427318, 16.36702704695009, 16.625750620531704, 15.957878711763229, 16.33739825577323, 15.891074926150234, 16.254668045556325, 15.49297637532319, 15.68263275927217, 15.764844826837939, 16.102619641377487, 15.898037827687684, 16.08510637117597, 16.175856354624326, 15.751552455098553, 16.350797272770315, 15.735169791221601, 15.928388682283526, 16.016811290308873, 16.086910897427305, 16.255026132606986, 16.363165660991992, 15.470796617167517, 16.395342433725638, 15.983400398977109, 15.782564501352429, 16.488942210819886, 15.446040932149842, 16.329333542761542, 16.197388174345104, 16.08453093219218, 15.623062824959428, 15.681005600685491, 15.521798957586093, 16.630649526198763, 16.53914594910323, 16.791984500732287, 15.514626203714341, 16.22483833068045, 16.107330763876757, 16.10026779123216, 16.482011232189443, 15.715047668522331, 15.507040187304987, 15.883808909546458, 16.410355217843975, 16.495420007180925, 15.746596595091784, 16.24554027755264, 15.924896669331764, 16.146301402151046, 16.737706078308413, 16.016532289969128, 16.13035987093635, 15.544593328474953, 16.478982012256374, 16.017109552313052, 16.67337074297929, 15.954367976445349, 15.90961131347168, 16.235511332100273, 15.981965253764647, 15.533262899964141, 15.473486763583427, 16.19799144071385, 16.230058517433715, 15.62280186971367, 15.893098083024318, 15.52709933824932, 15.828556517688039, 16.068832775864163, 16.29892140379804, 16.462039773468906, 15.782288844590255, 16.342966315095474, 16.086788589945957, 15.70554250889134, 15.652637410008671, 16.387263761417845, 16.094725248426514, 15.856020328583503, 16.119473847697044, 15.928651350376448, 15.693231773413988, 15.654019994844973, 16.53309965336768, 15.690623461021364, 15.658908425158234, 16.254232216256657, 16.34608232069646, 15.765280338858066, 16.19034059122401, 16.385860271851698, 15.7885824633158, 15.790818051358919, 16.039159870081264, 15.751934445257177, 15.582403931131449, 16.33376888929847, 15.843685544823131, 15.1787673964926, 15.967086875339458, 16.09341166985201, 16.220785729451062, 16.076435429428887, 15.581647534470267, 15.173810573926469, 16.034076074549816, 15.771379343965469, 16.287642271609403, 16.093797317523613, 15.765936903386603, 16.49800853297014, 15.775772011038562, 16.423404826780278, 15.761356117737787, 15.39790728515314, 15.826665129973694, 16.298869215232244, 16.180858187145738, 16.022140882336227, 16.074127843888938, 15.615076695288101, 16.0787615118254, 16.208216438283067, 15.383982324479147, 16.571913677029286, 15.698248243739886, 16.175758282184976, 15.794783306823694, 16.145529945568878, 16.353843315243935, 15.45505123914045, 16.706351795346066, 16.15057495398914, 15.70588725671035, 16.39414161913054, 16.22979901177754, 15.796768841004974, 15.479988220315967, 15.939625428661186, 15.991328470330679, 16.114790012950614, 15.668301565555995, 15.753925473416972, 15.890254182784942, 15.831702160173876, 16.280022632214184, 16.474123804070445, 15.630380778033647, 16.78319412582794, 16.097909944459012, 16.290686148726884, 16.277624631631152, 16.111106665510682, 16.183664298176033, 16.002849325503878, 16.401489664016168, 15.782398491809426, 16.017352940319906, 16.13298882743219, 15.990807359878719, 15.750711316868298, 16.246918771249565, 15.598363222221204, 16.01160437577694, 15.844319250608848, 16.085360557899627, 15.516162696331994, 15.702997836266064, 16.71577116505518, 16.11499744804987, 16.028672971916137, 16.412691222614985, 16.227565110085212, 15.675769716103073, 15.77953638167429, 15.605496223996965, 15.23392667091269, 16.019059882034306, 16.410639454208322, 16.044156261355017, 16.182969170679378, 15.901019544979027, 15.642129334591575, 16.67554976895083, 15.914354242573015, 16.18039692232827, 15.371006016748707, 16.103201913160408, 15.702412391961525, 15.796310282288792, 16.32258487885317, 15.581620769049847, 15.756254078037195, 15.342396609269196, 16.090441366593744, 15.871915636061004, 16.31772665783741, 16.790823174633225, 15.939004266107881, 16.081364798236354, 16.296155243065247, 15.998413915283775, 16.11432714267179, 15.925328351902143, 16.337926231175615, 16.312710480973287, 15.513507264401825, 16.05616298907623, 15.449083638647519, 16.105457775472342, 16.00037792745269, 16.726469899900593, 16.612229440384677, 16.01300304518633, 15.759197541730856, 16.396000358353746, 16.377733099661583, 16.15500355491207, 15.861708031900854, 15.81075848871337, 16.44730316482632, 16.320428659027385, 15.974057336392304, 15.801455990320404, 16.441264725892925, 15.79105378485693, 16.30965341083419, 15.866072970226448, 16.473025881959778, 15.982929098517138, 16.426657358995417, 15.87169185736009, 16.0492706376513, 15.693813149520778, 15.552332639521879, 15.972331658831731, 15.762018771574956, 16.115589474755655, 16.253708875746913, 16.352814830722043, 16.388965960368413, 16.022464010208203, 15.932252600023261, 16.106164753591166, 16.662716301727947, 15.833356386073117, 15.884014803954432, 16.074295280456113, 16.225425613347554, 15.6795719146088, 16.743556490416253, 16.25998551954086, 16.573304582345802, 16.03687255645736, 16.09776415521015, 16.23159082242225, 16.11876466145695, 16.336304318086427, 15.925805562567497, 16.425762833009053, 16.484492664113137, 15.895361129882058, 15.80955467549244, 16.244562763493946, 16.11946081391676, 16.099871078098513, 16.295718680284637, 16.053532183005125, 15.913062187292505, 15.49972949604069, 16.073649428985295, 10.036030952845428, 9.52416954207984, 10.22192932323909, 9.564645943856286, 10.07927548083934, 10.058818111997615, 9.991292284060098, 9.944354740259758, 9.742465071839906, 10.182340371197549, 9.672836967467308, 9.661697732555833, 9.855696584076803, 9.554902217667946, 9.990388031459947, 10.583432047614401, 9.62856632901359, 10.052475923566934, 9.658382821576787, 9.484753109557492, 9.76116058493048, 9.651713218339271, 10.009210719800544, 9.844044630837303, 9.671397440377234, 10.541186956335356, 9.966233256190204, 9.434404469801072, 10.327568385633151, 9.706890568933996, 9.453153423443908, 10.047890969448561, 9.684769216241305, 9.661753453763904, 9.926258140861886, 9.721459685987737, 9.508001818047124, 9.589183159050851, 9.70465493622427, 9.655013165717339, 10.225364915017419, 10.218251449099931, 9.389294643387114, 9.625175927959512, 9.49573197576345, 9.625828607646657, 10.111863694698357, 9.803884423477877, 10.188226893530013, 9.579826706489886, 10.350432719527474, 10.319283183301103, 9.550513631218058, 9.987153822262036, 9.827501718091888, 9.768681663581052, 9.552304428987194, 9.783923299745636, 9.969711418976232, 10.063621239047336, 10.03450617279287, 9.990902953337727, 9.87535109276072, 9.948423423533958, 9.969478349768686, 10.214827708686807, 9.681312525728593, 9.621333277090725, 9.688132123037105, 9.866243614667411, 9.75024923851269, 9.976408375093277, 9.967240584769888, 9.976395398423804, 9.660577810046043, 9.784856114117261, 9.755998671381692, 10.227268728783205, 10.012096677935272, 10.23325818232961, 9.980484796815025, 9.725424341652086, 10.05186514042769, 9.1042229746956, 9.603706748114805, 9.772398642149692, 9.697251390869113, 9.933632234287797, 9.83130807461501, 9.572477386816834, 9.761005665614823, 9.879330470473043, 9.663337778952934, 9.875257355935295, 9.491710174865576, 9.635574934932887, 9.941055178110815, 10.005036435971029, 9.805403724984469, 10.042489961861188, 10.054383587575565, 9.740704899953244, 9.743606194267963, 9.591898424742762, 9.649719104269893, 9.387724981404304, 9.702798919481703, 10.139046195164513, 9.424906065429687, 10.279941731954192, 9.743431552116578, 9.477371070540961, 9.688841311086108, 9.827600467074301, 9.650173589212974, 9.712422304780528, 9.656337222885824, 9.626302694906197, 10.104750690366913, 9.792185743899754, 9.746101079535011, 9.535441567335361, 10.183343224762606, 9.791261784486808, 9.900498743289521, 9.640550214902445, 9.417067013052128, 9.695439863596087, 9.75852863226546, 10.157748144971416, 9.770353988376836, 9.974570417022893, 9.915654596102868, 9.757306479233135, 10.223466648612673, 10.092624450288206, 9.4633706341562, 9.912302612571443, 9.629500833256992, 9.78382328126692, 9.942993730194285, 9.940213664412111, 9.72952319187472, 10.078838275759193, 9.565500189820517, 9.641380622006148, 9.656297933057527, 9.765174497974275, 9.578077550434545, 9.52427324169454, 9.674440399527402, 9.688881047378695, 9.564700254737774, 9.585890428137088, 9.85896570463454, 9.40324067480819, 10.023028401448677, 9.870638984777514, 9.68244573469406, 9.6843171567596, 9.573475558360029, 10.115476961582267, 10.54142704814035, 9.846790741626073, 10.027171182407473, 9.695586564014153, 10.025305372984427, 9.197875051717414, 9.849582664156783, 10.185716001552064, 9.715325283581338, 9.723306009692017, 9.536267387173503, 9.245971459407759, 10.409968305980973, 10.12445812981265, 9.602190985409504, 9.549807513241658, 9.659904003784867, 9.409323097925268, 9.642267960664295, 10.057572395608995, 9.619357218508746, 9.393867744045357, 9.816284091808324, 9.670156608581841, 9.654725767634842, 9.687457398747894, 9.426133629180363, 9.820367177947613, 9.625099205752825, 9.607136498470917, 9.853516890671246, 10.08496722832954, 9.742211071696689, 9.616476821318049, 9.683254104045202, 10.096099766690795, 9.563168866543705, 9.782054203295033, 10.163321656270062, 9.552053457096356, 10.170585163891099, 9.733149857559722, 9.15459492753754, 9.499708148140273, 9.288539339794442, 10.235087668568383, 9.823879905568285, 9.883032923138641, 9.357208932643422, 10.222945079515345, 9.547149373051138, 10.238130100383088, 10.016885301775405, 10.25938378097706, 9.921554473734162, 10.13109183153405, 10.028945518424985, 10.01984595835447, 9.884626893589981, 9.925611513590171, 9.89215813501931, 10.39939119820036, 9.71666743298899, 10.081281885587554, 10.501610915261118, 10.235701616969445, 9.399954438782217, 9.929804209193511, 10.22795674482607, 9.428501130073613, 9.805785584734638, 10.283114627230798, 10.184721590892627, 9.629876572920567, 9.714072289410385, 9.73237551671277, 10.065047577523202, 10.10689437499627, 9.832063572691146, 10.225971175917556, 10.084932065495062, 9.527666895248144, 9.748147328436088, 9.543291925552666, 10.055439821735202, 9.70351916981603, 9.7217163597074, 10.199096210043185, 9.806637835046175, 10.308250370957575, 9.86738314811878, 9.352620472855302, 10.079112487428207, 9.450277848854254, 9.775066060331833, 9.616163766572093, 10.018362161538978, 9.788258097034257, 10.009405657030864, 9.980978175953336, 10.130690955983155, 9.946244826315931, 9.688180712953525, 9.78279832854851, 9.424144189370494, 10.110956390479119, 10.081520250385163, 10.177815669153965, 9.854672265341787, 9.701052482728867, 9.48158473374066, 9.4517839513364, 9.8553539866621, 9.899468541313162, 9.97619362530691, 9.474119643324844, 10.145212049524485, 10.120647911024598, 9.822234789075445, 9.67880485262821, 9.95903857514082, 10.102748542790849, 9.641796853827278, 9.713503076950671, 10.246639578004324, 9.762750849877255, 9.848443703673894, 9.938923477407958, 9.713323769686955, 9.486187527889573, 9.77006400681944, 9.191062812914733, 9.702982902380466, 9.727233487565258, 9.823467968372988, 9.96516773687097, 9.945104945879676, 9.802456371313127, 10.178094100510714, 9.764736495511114, 9.784630251965433, 9.881048559068963, 9.776917255772304, 9.881951588090217, 9.73409100669575, 10.028073603215352, 9.780215179322326, 10.033178290851026, 9.801260594908873, 9.685473235202979, 9.680036918288831, 9.483984318108487, 10.164424958262362, 9.985465201383661, 9.891123177923284, 9.549262292366409, 9.973741218829076, 10.025080904602248, 29.28380147012024, 28.855850762104048, 28.2383529871353, 27.714113515941087, 26.95336994134646, 26.336941358816205, 26.039846788943887, 26.186804598580913, 26.510728957075305, 26.66705243349079, 26.446102919968016, 26.212617394476602, 25.86572747627675, 25.741708440838366, 25.580049744509175, 25.24340824669468, 25.58798502343151, 25.75635364852762, 25.85988765264062, 25.92967844621668, 26.045989005518773, 26.071900965537328, 25.992158844611936, 25.79715021763733, 25.396967873225837, 24.955667619411457, 24.58331442543134, 24.21001377307663, 23.851901000781886, 23.42220530425081, 22.87061765282377, 22.482597619575557, 22.180360678637385, 21.948666871286203, 22.046433701485668, 22.590926528590366, 23.3458066325338, 23.422786972712437, 23.1604438005215, 22.99059764354573, 22.868273491402768, 22.769490027613934, 22.60663401259764, 22.478182695906145, 22.383331148164892, 22.239892922633302, 22.123191632193006, 22.021574328314657, 21.912832033994476, 21.7538641707476, 21.646686093499696, 21.5116673990089, 21.365558974115892, 21.288478172953766, 21.161502151515773, 21.032122010043924, 20.932782002118604, 20.83350967578524, 20.74591152706154, 20.614819155373198, 20.52827826070299, 20.414981817690563, 20.32983249942402, 20.280234082931294, 20.192334707299732, 20.24553215914265, 20.27957239043449, 18.969686185628987, 18.083643975679777, 18.063262238729397, 18.38880011733283, 18.544733056260785, 18.645590715798697, 18.75818478133457, 18.737718254189442, 18.695918788155108, 18.640233329788643, 18.68801838445178, 18.41142624558797, 18.020626846705685, 17.681810388441455, 17.585714404789666, 17.43095935908741, 17.304924139205035, 17.1723674093001, 17.13592372835623, 17.036757755360277, 16.844089668888195, 16.72914400121355, 16.62999028055708, 16.442438628858486, 16.417185494125306, 16.289818998075017, 16.219717400096837, 16.177088963683328, 16.12963732831257, 15.931638188159848, 15.842961121771493, 15.630234646923729, 15.271361994054931, 14.96547945623347, 14.700680989274673, 14.454470921120405, 14.345646668405507, 14.106069522801604, 13.864640906036607, 13.646376205767027, 13.338466024629321, 13.086411716453513, 13.03682953748545, 12.992639051519856, 12.945646034363822, 12.767732585878647, 12.578476544185092, 12.299781802104892, 12.047685714885855, 12.033396504586738, 12.001757273456239, 11.93915292519657, 11.9080331854743, 11.844621021438956, 11.750500794480876, 11.729464766794328, 11.596726910777814, 11.485090822319826, 11.281268965691714, 11.087229870799158, 10.942751601981584, 10.764823631907685, 10.665465261696276, 10.556585112296109, 10.479428841881012, 10.436439366117643, 10.340509016653499, 10.501347096878108, 10.702073226330349, 10.67862900704085, 10.720338623193264, 10.665136623457103, 10.581089359422009, 10.539949866734853, 10.672426011246571, 10.821265796589335, 11.12612685555938, 11.512148225680189, 11.818324645342582, 12.124558667984175, 12.54802139366178, 12.837639308676287, 13.051347333938269, 13.303171771161107, 13.401729296733697, 13.492344364213245, 13.614751218796009, 13.688507558398166, 13.81067216271785, 13.867258241365501, 13.99667456312079, 14.08709932200747, 14.19787227478547, 14.383385801423362, 14.487166313948096, 14.605604245125644, 14.767665514227831, 14.880988538570794, 14.968217828206186, 15.17692369497242, 15.303488520263437, 15.469886061734927, 15.67369861836895, 15.840235933405161, 15.958846695610537, 16.191997439802574, 16.2975610062381, 16.389436203907557, 16.575310136816928, 16.725744560355814, 16.814914948637593, 17.028471020207995, 17.13333758416733, 17.253721869037854, 17.368881089337393, 17.519356247609508, 17.628242381589676, 17.732212927472702, 17.911771628991755, 17.993441236638038, 18.1027474202987, 18.294831074142927, 18.407960703237222, 18.53431127675006, 18.718536827061392, 18.85979453674774, 18.967764378136174, 19.13614828554018, 19.261479343105684, 19.426596346012914, 19.565241572614372, 19.73984129431605, 19.86925454928538, 20.052029037144614, 20.231447955962604, 20.372857924631127, 20.49762098197742, 20.693766499016558, 20.81031135787173, 20.95755114365393, 21.111696382705478, 21.231792628718814, 21.323359316655804, 21.451504548956514, 21.52782539004932, 21.60845736279192, 21.753767172223657, 21.88805389660359, 22.010372955288297, 22.176242117296756, 22.300741810167803, 22.42741311839772, 22.51792908790115, 22.64365275111282, 22.69784620393916, 22.772026041801425, 22.904512192760837, 23.026655997395782, 23.112804363518023, 23.23976661703296, 23.32945151855742, 23.409747537880968, 23.55636120444674, 23.601896458364436, 23.7373370369509, 23.826978315508818, 23.926685956604192, 24.089567863963662, 24.19055974091759, 24.314860675611122, 24.473921324031114, 24.574099311937577, 24.707704538742387, 24.862497103627053, 24.975182987791282, 25.104924562850034, 25.176330200456714, 25.254307826338604, 25.355798395571696, 25.479645046375435, 25.58326264639573, 25.7476867921, 25.913814540200708, 26.063805952222445, 26.23055756992977, 26.393119199387296, 26.496761332264942, 26.68013220098038, 26.79926590657292, 26.924836896173783, 27.018581006342977, 27.16374525782122, 27.251874525939183, 27.407612035847308, 27.56749500849837, 27.678299728858704, 27.852391716460517, 27.987989463564777, 28.108008793516692, 28.162880274368213, 28.17253579673766, 28.363327133636606, 28.253351024582045, 28.099984163594527, 28.01703773385302, 27.900926370283194, 27.745206980861944, 27.651639378690888, 27.503563848075707, 27.352071254837334, 27.23540585553999, 27.065154459231405, 26.864341823509672, 26.805996613220785, 26.752347749171392, 26.690265096065485, 26.65506354276404, 26.502955721845765, 26.367528946258318, 26.229404446795783, 26.093235080582367, 25.98423849887039, 25.879680118130473, 25.778141540309782, 25.71134070890073, 25.57967697281905, 25.499946840827945, 25.429030961479377, 25.334663676076843, 25.260816673680733, 25.174988396717346, 25.058553304537266, 24.921662141983365, 24.8028151287338, 24.635925267095928, 24.496190355965922, 24.378955139689538, 24.175120002889958, 24.051364063688148, 23.917085840996034, 23.768845618992287, 23.595489999188892, 23.479847561521016, 23.319509142103783, 23.180486986476026, 23.077337055345165, 22.927792029117647, 22.778490920491198, 22.662443551963687, 22.543428643438833, 22.35940986828133, 22.23876138890968, 22.0834423009285, 21.927412017797195, 21.831273784155062, 21.68853279386608, 21.537530199442557, 21.39203220878636, 21.26389847801503, 21.13196296744019, 20.962924641690336, 20.837678542312545, 20.69709109580729, 20.562597805811773, 20.472589127463408, 20.324227016127697, 20.172864841789302, 20.058533576310985, 19.899124291893894, 19.714184586642173, 19.59220253384138, 19.446142218227518, 19.267207909130455, 19.14970380690583, 19.043265079548814, 18.85628713970961, 18.78417021955325, 18.608226536895224, 18.410792660089694, 18.306040740544162, 18.132148352097847, 17.914646609647072, 17.838655345874386, 17.656996612863995, 17.54675186768321, 17.409890927508766, 17.30776130953445, 17.15763861429936, 16.993809124275366, 16.885920402909882, 16.778349446831044, 16.538582770690773, 16.490249066497892, 16.323933289379557, 16.162752250273996, 16.08216322906554, 15.919720713220562, 15.722371056327495, 15.644226901463433, 15.50592291654254, 15.313225783345489, 15.224461637985549, 15.098170994820098, 14.886740190522609, 14.804197407779295, 14.623372917048176, 14.435680754398179, 14.31370051029928, 14.136514976801493, 13.949789922616205, 13.838410542490585, 13.658959729707828, 13.515762404945448, 13.343128053136013, 13.235940687854452, 13.026311634029677, 12.818569251955916, 12.742502510820545, 12.581285758625164, 12.311739521358408, 12.057433664676308, 11.822002844937401, 11.425768226442544, 10.91900176768002, 10.36743323913363, 9.972719322677554, 8.96502178877903, 3.693620115907079, -6.705225495915015, -5.019991780753701, -5.1429300422992785, -5.105868172849589, -5.725086573076386, -6.003149243819397, -5.567549600747633, -5.331373204485708, -5.216718828051388, -5.082114638553193, -4.795893745385522, -4.626744366698205, -4.746634321817684, -4.241222881474529, -4.38474423003947, -3.8019711334359365, -3.722907376899032, -3.6669454621778566, -3.384083191453509, -2.9079826954716856, -2.7768343779369395, -2.4280858594175525, -2.6070453610322972, -1.8407313555921618, -1.7330418348373704, -1.5458047411697793, -1.1060290296065345, -0.8633541780751242, -0.9289629227937635, -0.5141789515171604, -0.5073285601636539, 0.023548162720735455, 0.2208646941786192, 0.5300660170512672, 0.47689083823609124, 1.042894720186946, 1.2493858110248377, 1.5616441466363216, 1.7535935852094235, 1.9244853012324725, 2.1027686539727495, 2.274075078741522, 2.259280023053692, 3.034530573367663, 3.002879730054053, 3.341566268864793, 3.7563310214274033, 3.7647181361330126, 3.8850485669971473, 4.312245622486614, 4.359448932129542, 4.478640209753913, 5.049556170499718, 5.1490275380855905, 5.702519493621559, 5.643943449614121, 5.495333384043621, 5.958987990425897, 6.116089305804019, 6.241506002725941, 6.564068385491933, 6.569837855242216, 6.671088277340115, 6.737867787115353, 6.937705746412705, 7.190173465780598, 7.4579982643306515, 7.521628702340976, 7.422786678991427, 7.682280455531379, 7.730349664615977, 7.803941286816093, 8.076988250750865, 8.301083754435588, 8.60903969646005, 8.492513852694731, 8.583914906058792, 8.989533591586657, 8.8468334902202, 9.137764094493566, 9.414362054831631, 9.738416329250526, 9.562216365162314, 9.829556865860866, 9.686962331097174, 10.198234630064848, 10.320999689200384, 10.562448796896236, 10.680252442998018, 11.141519798740589, 11.129248909429592, 11.260490645176505, 11.533390692716242, 11.955724843965301, 11.99038335825744, 12.20056413169609, 12.265034805387014, 12.480324607685963, 12.646845865553118, 12.846839231226948, 13.064963706439386, 13.08969826147575, 13.194029516029927, 13.361230033723846, 13.016857307254286, 13.409405682969911, 13.502998027104477, 13.73958180342214, 13.391455298157837, 13.501337408849682, 13.40946074604658, 13.444491938489483, 13.561742593073454, 13.446046302739543, 13.327228179268378, 13.213368575206125, 13.134885204314553, 13.178140580192792, 12.992316162754555, 13.033310645695579, 12.885424215552659, 12.997856421722457, 12.706525981150445, 12.951083270653017, 12.952275132002042, 12.970575499043111, 12.72599403218738, 12.859988039840117, 12.961321928875108, 13.201858778725104, 12.961448379875677, 13.08269908155694, 12.7698408543673, 13.175788493970536, 13.646933797705142, 13.242204724970613, 13.534405636239445, 13.343225187495678, 13.39408622765902, 13.429838966753662, 13.475376846283302, 13.064429608689167, 12.824961343652582, 12.675081356511166, 12.58885926768505, 12.332100997992095, 12.227616667760048, 12.20724007222619, 11.950595547620734, 11.981200879877786, 11.946889452720912, 11.99018208582321, 11.790895852292465, 12.140729449348699, 11.877006549619495, 11.630456778713471, 11.845407209677528, 11.663941371903302, 11.763485427688746, 12.147038657301255, 11.819970412114559, 11.81401097389339, 12.110369041736426, 12.227502511818333, 12.217511654084584, 12.500098355706735, 12.651345488557538, 12.398598588219405, 12.334319234652146, 12.248637274790942, 12.682407066907901, 12.329650526858671, 12.391044231898368, 12.295547629025874, 12.097560635109755, 12.057493980648854, 12.15654054517533, 12.046098563511002, 12.419730049345883, 11.648032254205518, 11.810150542020436, 11.417117681931153, 11.570887233497714, 11.097759085906413, 11.092097254063251, 11.032433777402915, 10.86809945004855, 10.67866829022733, 10.396583390091582, 10.41037171860063, 10.075023272079633, 10.00915745002164, 9.739269348217238, 9.613293963952572, 9.695801945905181, 9.6400450782293, 9.267277805778804, 9.285653436281592, 9.019351715644149, 8.794427614411113, 8.678332738745375, 8.470559715588063, 8.419195810215548, 8.093654624835528, 7.703931861942598, 7.898189442462748, 7.843772261967006, 7.425356124826763, 7.326242832825505, 7.229819206819126, 6.990690652836754, 6.763956574866841, 6.280230338925216, 6.465482950620629, 6.385740705481803, 6.254302493295772, 5.772007899524432, 5.759767116634666, 5.564327856857893, 5.700433936855302, 5.138143021502353, 5.010004903422173, 4.86009041815105, 4.480578209592095, 4.258799641965825, 4.22998339761339, 3.992923269126989, 3.983976215674625, 3.495136198053337, 3.775910678332031, 3.187740990132246, 3.1345003395475457, 2.880139754745274, 2.806876373465082, 2.6856959029264384, 2.233741931056107, 2.1749157925622944, 1.8696808958947622, 1.9301138464954493, 1.8629616172209578, 1.4192539153981043, 1.1822209077931136, 0.8550188359635555, 0.7056417641917081, 0.7829481960031393, 0.04445088685299847, -0.13428713013756965, -0.17853922325292704, -0.5660373257467155, -0.5586810364767762, -1.0593910465349676, -0.9423479614496708, -1.6227308420610251, -1.9145111378927924, -1.7795985041234088, -2.0501527473726195, -2.3019337349554982, -2.6977920308856476, -2.6320455451064335, -3.0879498670615924, -2.950720264274815, -3.2802418612556883, -3.4953384719252965, -3.5887905996263747, -3.7376871570518544, -4.088424621510533, -4.319162938619369, -4.816320944058791, -4.984256201062925, -4.802832547165761, -5.301177833125873, -5.663161153585592, -5.492288024322468, -5.591667108973079, -5.832605767918858, -5.712287930472244, -5.342928313354063, -5.576056572786711, -5.0660800467404705, -5.117876865874063, -5.343617412969936, -4.983450744856476, -5.084332271293897, -4.842883763261444, -4.672838482369811, -4.373277682778183, -4.276256918365337, -3.878085211295708, -3.3920844697559622, -3.1332046771802666, -2.879081073956859, -2.5107686158361893, -2.442821545576887, -2.06705488674453, -1.6411530300560502, -1.7220839333673226, -1.5588757253340053, -0.9167856244418954, -0.7839194118820447, -0.33961163433789, -0.15236186231114163, -0.04486614277854223, 0.43546183834933083, 0.5044989225644902, 0.8165726562220523, 0.7889410631514072, 1.346807222763394, 1.2383098815342255, 1.1362862976236638, 1.3822523312531367, 1.5231460505114858, 1.8150065909760378, 1.9146721788384093, 1.966412014336341, 2.263181012566054, 2.237514962005805, 2.926429823980852, 3.350111295898376, 3.1542080013638873, 3.751066999616351, 3.9130358583278775, 4.13520313082802, 4.323750266552105, 4.651317248068186, 4.7650005384534175, 4.7923989977319925, 5.092882650243138, 4.95175208108743, 5.144657020793701, 5.153490056229116, 5.5909211532248895, 5.202714329921465, 5.708371788425102, 5.839756547364665, 5.868393344665464, 5.978614255838053, 6.30983143722152, 6.336683278749941, 6.363017045554367, 6.5106725151543365, 6.651123262048696, 6.768015663820039, 6.745101164622604, 7.25507988695253, 7.010046767795046, 7.5212134398509205, 7.583348298045014, 7.846487630515144, 7.923998049907523, 8.007911536048802, 8.270141496063225, 8.191328426887399, 8.351262995597306, 8.723616763104058, 8.689600930799351, 9.012747105714395, 9.197248559869841, 9.497725590521188, 9.314314774325613, 9.602009813104596, 10.028304523023987, 10.027802610940784, 10.066311690764735, 10.046929878192676, 10.430589480096085, 10.51717242946731, 10.900348242510503, 11.025498189622224, 11.3622727007585, 11.488782155179198, 11.407581773615867, 11.79014114313772, 12.114366806414756, 12.068015903580257, 11.652055246161684, 12.38220156234749, 12.19711095398372, 12.292946743397419, 12.357806475020677, 12.56014797820815, 12.45119899776593, 12.339491129763168, 12.443308307460564, 12.300469921544519, 12.662376204605833, 12.586491510260991, 12.736395396259029, 12.335706539788067, 12.5942700565413, 12.361505453502538, 12.968912070147116, 12.689939951632272, 12.556973682781274, 12.575524450033296, 12.761548717073314, 12.618457912314625, 12.861290924173899, 12.657393729044696, 12.761204925947581, 12.544123142963777, 12.788455858731767, 12.595408423083438, 13.192769351934174, 13.173076460675315, 13.221466416809882, 13.1518809584042, 13.260542025856491, 13.485893478684911, 13.263048668879403] caption="Most Recent Time Trace"
  out "Save APD Deriv":dbl[][](graph)=[[950.0, 950.0, 4283.333333333336, -20058.333333333336, -366.66666666666606, 66.66666666666606, 13191.666666666666, -8641.666666666668, -150.0, 966.6666666666661, 4041.6666666666642, -24908.333333333336, 533.3333333333339, 291.66666666666606, 14275.000000000002, -7141.666666666668, -341.66666666666606, 91.66666666666788, -2316.666666666666, -716.6666666666661, 4283.333333333334, -4158.333333333332, 58.33333333333394, 425.0, 41.66666666666788, 1783.3333333333321, -10258.333333333334, 458.33333333333394, 400.0, 14208.333333333334, -1691.6666666666679, -541.6666666666661, -175.0, 1650.0, -15399.999999999998, 75.0, 16.66666666666606, 3300.000000000002, -7258.333333333334, -8.33333333333394, 274.9999999999991, 8691.666666666668, -7500.0, -250.0, 291.66666666666606, 9808.333333333334, -5800.000000000002, -675.0, -108.33333333333394, 2933.333333333334, -9308.333333333332, -141.66666666666788, 66.66666666666606, 8683.333333333332, -7624.999999999998, 75.0, -358.3333333333321, 3791.666666666666, -2508.333333333334, -775.0, 591.6666666666661, 2700.0, -4975.0, -200.0, 641.6666666666661, 658.3333333333339, -3591.666666666666, -91.66666666666788, 400.0, 1175.0, -3641.666666666666, -208.33333333333212, -50.0, 2675.0, -1525.0, 83.33333333333212, -200.0, 1533.333333333334, -3508.333333333334, 325.0, -158.33333333333212, 4633.333333333334, 25.0, 208.33333333333394, 433.33333333333394, 958.3333333333321, -2083.333333333334, -108.33333333333212, -133.33333333333394, 550.0, 366.66666666666606, 350.0, -266.66666666666606, -300.0, -300.0, 75.0, 75.0, 91.66666666666606, -208.33333333333212, 75.0, 241.66666666666606, 116.66666666666606, -233.33333333333394, 41.66666666666788, -75.0, 433.33333333333394, -158.33333333333394, 541.6666666666661, 450.0000000000009, -166.66666666666606, -824.9999999999991, 183.33333333333394, 83.33333333333212, -358.33333333333303, -400.0, 175.0, -283.33333333333394, -50.0, 591.6666666666661, 8.33333333333394, -166.66666666666606, 408.33333333333394, 0.0, 33.33333333333394, -175.0, 424.9999999999991, 575.0, -25.0, -383.33333333333394, 308.33333333333394, -458.33333333333394, 450.0, 716.6666666666679, -433.33333333333394, -41.66666666666606, -283.33333333333394, 316.66666666666606, -183.33333333333394, -450.0, -58.33333333333394, -633.3333333333339, -925.0000000000009, -300.0, 275.0000000000009, -408.33333333333394, 258.3333333333321, 733.333333333333, 125.0, 350.0, -83.33333333333394, 83.33333333333394, -708.333333333333, -108.33333333333394, -141.66666666666788, 550.0, 16.66666666666788, 225.0, 308.33333333333303, 33.33333333333394, -316.66666666666606, -758.3333333333321, -191.66666666666788, -366.66666666666606, -233.33333333333394, -400.0, -308.33333333333394, -291.66666666666606, -216.66666666666606, 191.66666666666788, -100.0, 608.3333333333339, -183.33333333333394, -241.66666666666788, -266.6666666666679, -316.66666666666697, 50.0, 75.0, 66.66666666666788, 125.0, 16.66666666666606, -358.33333333333303, 533.3333333333321, 41.66666666666606, -325.0, -291.66666666666606, -1275.0, -941.6666666666661, 375.0, -75.0, 441.66666666666606, -2700.0, -166.66666666666788, -841.6666666666661, 1316.6666666666642, -2258.333333333334, 0.0, -166.66666666666606, 1175.0, -1533.3333333333321, -175.0, -400.0, 2475.0, -3391.666666666668, 200.0, -316.66666666666606, 1408.333333333334, -2941.666666666668, -466.6666666666679, -583.3333333333339, 1691.6666666666679, -633.3333333333339, 541.6666666666679, -250.0, -66.66666666666606, -41.66666666666606, -191.66666666666606, 116.66666666666606, 250.0, -2200.0, -558.3333333333339, 75.0, -1850.0, -1141.666666666666, -408.33333333333394, -216.66666666666606, 150.0, -2800.0, 516.6666666666679, 241.66666666666606, 1091.666666666666, -1466.666666666666, 58.33333333333394, -41.66666666666788, 1308.333333333334, -1100.0, -75.0, 266.66666666666606, 2950.0, -1575.0, 175.0, -116.66666666666606, 2108.333333333332, -583.3333333333339, -375.0, 183.33333333333212, 675.0, -800.0, 183.33333333333394, 241.66666666666788, 241.66666666666606, 175.0, -91.66666666666788, 291.6666666666679, 2533.333333333334, -25.0, -925.0, -16.66666666666606, 3358.333333333334, -2425.0, 8.33333333333212, 850.0, 2208.333333333334, -5733.333333333334, -50.0, 483.3333333333321, 6450.000000000002, -1141.6666666666679, -141.66666666666606, -50.0, 1150.0, -7691.666666666668, -100.0, 400.0, 4191.666666666666, 50.0, 383.33333333333303, -616.6666666666661, 4275.0, -4300.0, 616.6666666666661, -241.66666666666606, 1875.0, -3908.333333333334, 658.3333333333339, -566.666666666667, 4116.666666666668, 75.0, 141.66666666666606, 358.3333333333321, 2833.333333333332, -266.6666666666679, 483.3333333333321, -108.33333333333394, -158.33333333333394, -525.0, 1716.666666666666, -841.6666666666661, -291.6666666666679, -75.0, 766.666666666667, 25.0, 566.6666666666661, -1033.3333333333321, -258.33333333333394, 666.6666666666679, 2125.0, -1116.6666666666679, 58.33333333333394, -308.33333333333394, -58.33333333333212, -625.0, 691.6666666666661, 125.0, 2166.666666666668, -2316.666666666668, -475.0, 233.33333333333394, 3558.333333333332, -1791.6666666666679, -200.0, -883.333333333333, 33.33333333333212, 8.33333333333212, 291.66666666666606, -458.3333333333321, 3916.666666666666, -1166.666666666666, 175.0000000000009, 466.66666666666606, 2766.666666666668, -75.0, -325.0, 33.33333333333212, 2866.666666666668, -5625.0, -633.3333333333339, 158.33333333333212, 2291.666666666668, -1283.3333333333321, 375.0, -233.33333333333394, 1100.0, -2741.666666666666, 125.0, 308.33333333333394, 575.0, -2100.0, -175.0, -33.33333333333394, 3158.333333333332, -116.66666666666606, 25.0, 558.333333333333, 1366.666666666666, -3050.0, 225.0, -66.66666666666788, -416.66666666666606, -1433.333333333334, -166.66666666666788, 8.33333333333212, 1216.6666666666679, -1591.666666666666, -566.6666666666661, -316.66666666666606, 308.33333333333394, -400.0, 166.66666666666606, 125.0, 1025.0, 291.6666666666679, 266.66666666666606, -225.0, 241.66666666666788, 408.33333333333394, 200.0, 483.3333333333321, 633.3333333333321, 616.6666666666679, 433.33333333333394, 33.33333333333394, 1000.0, -283.33333333333394, -200.0, -433.3333333333321, 458.33333333333394, -3850.0, -75.0, 33.33333333333394, -91.66666666666606, -100.0, 133.33333333333394, 466.66666666666606, 191.66666666666606, -183.33333333333212, 83.33333333333212, 200.0, 216.66666666666788, -591.6666666666661, -225.0, 458.33333333333394, 658.3333333333339, -8.33333333333394, 241.66666666666788, 216.66666666666788, -108.33333333333212, -691.6666666666661, -1241.666666666666, -66.66666666666606, 350.0, -675.0, -908.3333333333339, 583.333333333333, -433.33333333333394, -675.0, 308.33333333333394, -16.66666666666606, 33.33333333333212, -58.33333333333394, -550.0, -408.3333333333321, 166.66666666666606, 333.3333333333321, 208.33333333333394, 258.3333333333321, 333.33333333333394, -250.0, -258.33333333333394, -191.66666666666606, -316.66666666666606, 100.0, 500.0, -200.0, 908.3333333333339, -608.3333333333339, 308.33333333333394, -41.66666666666606, 1308.3333333333321, 158.33333333333394, -58.33333333333394, 708.3333333333339, -300.0, -466.66666666666606, -425.0, 283.33333333333303, 266.66666666666606, -700.0, 8.33333333333394, 291.66666666666697, 1133.333333333334, 125.0, 533.3333333333339, 141.66666666666606, 525.0000000000009, 333.3333333333321, -324.9999999999991, 1133.333333333333, 183.33333333333394, -525.0, -158.33333333333212, 75.00000000000001, 91.66666666666667, 25.0, -75.0, 8.333333333333343, -66.66666666666666, 0.0, 16.666666666666657, 33.33333333333333, -83.33333333333334, -16.666666666666657, -108.33333333333334, -58.33333333333334, 50.0, 16.666666666666657, -41.66666666666667, -25.0, 33.33333333333333, 0.0, -58.33333333333334, 74.99999999999999, -33.33333333333334, -66.66666666666666, 25.0, -8.333333333333343, 50.0, 0.0, -33.33333333333334, 16.666666666666657, 0.0, -25.0, 0.0, -108.33333333333333, -25.0, -25.0, -33.33333333333333, -16.66666666666667, 16.666666666666657, 25.0, 8.333333333333343, 91.66666666666666, -91.66666666666667, 16.666666666666664, -41.66666666666666, -25.000000000000014, -16.666666666666657, 16.666666666666657, 58.33333333333333, -116.66666666666666, -33.33333333333333, 58.333333333333314, -99.99999999999997, 16.666666666666686, -16.666666666666686, -33.33333333333334, -133.33333333333337, 58.333333333333314, -16.666666666666657, 16.666666666666657, 75.0, 8.333333333333343, 83.33333333333333, 25.0, 0.0, 0.0, -33.33333333333334, -33.33333333333334, -16.666666666666686, 8.333333333333343, 66.66666666666669, -58.333333333333314, 0.0, 50.0, 25.0, 50.0, 83.33333333333331, -58.33333333333334, -41.66666666666666, 41.66666666666666, 16.666666666666657, -33.333333333333314, 83.33333333333334, 8.333333333333343, -25.0, 8.333333333333343, 8.333333333333343, 75.00000000000001, 66.66666666666667, 33.333333333333314, 100.00000000000001, 41.66666666666667, -25.000000000000014, 141.66666666666666, 58.33333333333334, -41.66666666666667, 58.33333333333333, 0.0, 25.0, 75.0, -50.000000000000014, -50.0, 8.333333333333314, 25.0, 133.33333333333334, 116.66666666666666, -33.333333333333314, -75.00000000000001, 0.0, -16.666666666666657, -91.66666666666666, 58.33333333333333, 41.66666666666667, -50.000000000000014, -100.0, -16.66666666666667, -50.0, -58.33333333333334, 8.333333333333343, 74.99999999999999, 49.999999999999986, -33.33333333333333, -24.999999999999986, 0.0, 33.33333333333333, 8.333333333333329, -33.33333333333334, 8.333333333333329, -58.33333333333333, 16.66666666666667, -25.0, 58.33333333333333, -33.33333333333333, 33.333333333333336, -49.999999999999986, -25.0, 8.333333333333329, -41.666666666666664, -16.66666666666667, 41.66666666666667, -650.0, -41.66666666666666, 0.0, -16.66666666666667, 25.0, -16.666666666666657, 8.333333333333329, -50.0, -16.66666666666667, 0.0, 8.333333333333314, 58.33333333333334, -41.66666666666666, 0.0, -8.333333333333343, -25.0, -41.66666666666666, 25.0, 266.6666666666667, -316.66666666666663, 33.33333333333333, -25.0, 0.0, -8.333333333333343, 933.3333333333334, -158.33333333333331, 550.0, -1341.6666666666667, -16.66666666666667, -66.66666666666666, 33.33333333333333, 58.33333333333333, 1833.3333333333335, -241.66666666666666, 1158.3333333333333, -1491.6666666666667, -8.333333333333314, -41.666666666666664, 0.0, -8.333333333333329, 3500.0, -641.6666666666666, 2883.3333333333335, -3683.333333333333, 41.66666666666667, 8.333333333333314, -16.66666666666667, -41.66666666666667, 4966.666666666666, -1366.6666666666665, 3800.0, -5200.0, -41.66666666666667, -66.66666666666666, -8.333333333333314, -41.66666666666666, 3475.0, -1650.0, 3158.3333333333335, -4158.333333333333, -58.33333333333333, -33.33333333333334, -116.66666666666667, 25.0, 3083.333333333333, -2408.3333333333335, 4191.666666666667, -916.6666666666666, 0.0, -8.333333333333329, -124.99999999999997, 33.33333333333334, 1725.0, -2900.0, 5600.0, -799.9999999999998, 49.999999999999986, 0.0, -41.66666666666666, 8.333333333333329, 1450.0, -2333.3333333333335, 3133.3333333333335, -775.0, 8.333333333333343, 8.333333333333329, -41.66666666666667, 8.333333333333329, 850.0000000000001, -3475.0, 4783.333333333333, -1216.6666666666667, 50.0, -41.66666666666666, -33.33333333333334, -25.0, -891.6666666666665, -3433.333333333333, 5208.333333333333, -2150.0000000000005, 0.0, 8.333333333333329, -91.66666666666667, 8.333333333333329, -1141.6666666666665, -908.3333333333333, 1125.0, -3966.666666666667, 25.0, -49.99999999999999, 8.333333333333314, -58.333333333333336, 2750.0, -1983.3333333333333, 3091.6666666666665, -6408.333333333333, 83.33333333333333, -125.00000000000001, -100.00000000000001, 16.666666666666657, 1533.3333333333335, -3741.6666666666665, 783.3333333333334, -5125.0, 25.0, -16.666666666666657, -166.66666666666666, -91.66666666666666, 3883.3333333333335, -2508.333333333333, 3033.333333333333, -3116.666666666667, 8.333333333333329, -58.33333333333333, 0.0, -25.0, 4250.0, -1608.3333333333333, 1666.6666666666665, -1775.0, 66.66666666666667, -25.0, 8.333333333333343, 0.0, 6291.666666666666, -1566.6666666666667, 1125.0, -899.9999999999999, -58.33333333333333, -25.0, -24.999999999999986, 33.33333333333334, 2050.0, -550.0, 416.66666666666663, -816.6666666666666, -75.0, 8.333333333333329, -83.33333333333331, 16.666666666666657, 666.6666666666666, -241.66666666666669, 33.33333333333333, -41.66666666666667, 33.33333333333333, -16.666666666666657, -8.333333333333343, -66.66666666666666, 41.66666666666667, -66.66666666666667, 208.33333333333331, -58.33333333333334, 41.66666666666666, 16.66666666666667, -16.66666666666667, -99.99999999999999, -8.333333333333343, -58.33333333333334, 225.00000000000003, -66.66666666666666, 25.0, -16.666666666666657, 8.333333333333343, 16.666666666666657, 83.33333333333334, -516.6666666666666, 1225.0, 75.0, -100.0, -66.66666666666667, 41.66666666666666, -25.0, 266.6666666666667, -1075.0, 1075.0000000000002, -66.66666666666666, -66.66666666666666, -50.0, -50.0, 41.66666666666666, 125.0, -2408.3333333333335, 1266.6666666666665, -200.00000000000003, 50.000000000000014, 0.0, 58.333333333333336, 66.66666666666667, 449.99999999999994, -4141.666666666667, 983.3333333333339, -441.66666666666663, -33.33333333333334, 25.0, 16.66666666666667, -25.000000000000014, 500.0, -3808.333333333333, -141.66666666666652, -75.0, -91.66666666666666, 8.333333333333343, -16.666666666666657, 8.333333333333329, 508.3333333333333, -658.3333333333335, -1825.0, -1091.6666666666667, 75.0, 41.66666666666667, 0.0, 75.0, 325.0, -1391.6666666666667, -1675.0, -475.0, -91.66666666666667, 33.33333333333333, -91.66666666666667, 75.0, 1141.6666666666667, 1366.666666666667, -1791.6666666666665, -1158.3333333333333, -8.333333333333329, 16.66666666666667, 0.0, -33.33333333333334, 1833.3333333333335, -633.3333333333333, -816.6666666666667, -1500.0, 16.66666666666667, 0.0, -16.66666666666667, -8.333333333333343, 4241.666666666666, 1241.666666666667, -3583.333333333333, -366.66666666666663, 124.99999999999999, 75.0, 8.333333333333343, -75.0, 808.3333333333334, 275.0000000000002, 308.3333333333335, -1325.0, 16.666666666666664, -25.0, 33.33333333333334, -108.33333333333331, 2391.666666666667, 1833.3333333333335, -2233.333333333333, -558.3333333333333, 25.0, 25.0, -33.33333333333333, -16.66666666666667, 1541.6666666666665, -3025.0, 58.33333333333303, -416.6666666666667, 33.333333333333314, -16.666666666666657, -33.333333333333314, -66.66666666666666, 1033.3333333333333, -6175.0, 2500.0, -200.00000000000003, 0.0, -16.666666666666657, 75.0, 25.0, 741.6666666666666, -3900.0, 4025.0000000000005, -141.66666666666669, 75.0, 8.333333333333329, -41.66666666666666, -83.33333333333333, 483.3333333333333, -4516.666666666667, 1224.9999999999998, 0.0, -8.333333333333343, -16.666666666666657, -25.0, 8.333333333333329, 175.0, -2058.333333333333, 916.6666666666667, -16.66666666666667, -66.66666666666667, -74.99999999999999, 49.999999999999986, -8.333333333333329, 25.0, -416.66666666666674, 58.33333333333333, 8.333333333333329, 8.333333333333314, 25.0, -33.33333333333333, 0.0, 50.0, -49.999999999999986, 91.66666666666669, 0.0, -50.0, 16.66666666666667, -8.333333333333343, -25.000000000000014, 41.66666666666667, -58.33333333333333, 383.33333333333337, -8.333333333333329, 8.333333333333336, 33.33333333333333, 33.333333333333336, -16.666666666666657, -100.0, -225.00000000000003, 1391.6666666666665, -49.999999999999986, -16.666666666666657, 33.333333333333336, 0.0, 8.333333333333329, 258.33333333333337, -1591.6666666666667, 1333.3333333333333, -58.33333333333333, -49.999999999999986, -33.33333333333333, -8.333333333333329, -33.33333333333333, 525.0, -3008.333333333333, 2200.0, -133.33333333333331, 33.33333333333333, 16.666666666666657, -33.33333333333334, 16.666666666666657, 33.33333333333333, 41.66666666666666, -66.66666666666666, 50.0, -58.33333333333333, -50.0, 8.333333333333329, -83.33333333333333, 8.333333333333329, -16.666666666666657, 0.0, -41.66666666666667, 8.333333333333329, -33.33333333333333, -16.666666666666657, 8.333333333333343, -41.66666666666667, -58.33333333333333, 0.0, -8.333333333333336, -41.66666666666667, 16.666666666666657, -16.66666666666667, -41.66666666666667, -25.0, -16.666666666666657, -8.333333333333343, -108.33333333333333, 33.33333333333334, -8.333333333333343, -66.66666666666666, 58.33333333333333, 16.66666666666667, 41.66666666666667, 16.666666666666657, -41.66666666666667, 25.0, 58.33333333333333, 0.0, -16.666666666666657, 66.66666666666667, -16.66666666666667, -25.0, 58.33333333333334, 66.66666666666666, -50.0, -25.0, 16.666666666666686, 850.0, -2166.666666666667, 1433.3333333333335, -316.66666666666663, -25.0, 66.66666666666666, -33.33333333333333, 8.333333333333329, 683.3333333333333, -1966.6666666666665, 1891.6666666666665, 41.66666666666666, 66.66666666666666, 8.333333333333329, 91.66666666666666, 50.00000000000001, 600.0, -2091.6666666666665, -133.33333333333326, -108.33333333333333, -58.33333333333334, 16.66666666666667, 50.00000000000001, 50.0, 308.3333333333333, -2466.666666666667, 1541.6666666666665, -16.66666666666667, 25.000000000000014, -91.66666666666666, -58.333333333333336, -16.666666666666657, 100.0, -2266.6666666666665, 1600.0, -50.0, -24.999999999999993, -33.33333333333334, 33.33333333333333, 41.66666666666667, 208.33333333333331, -716.6666666666666, 958.3333333333334, -25.0, 0.0, -8.333333333333329, 41.66666666666667, -66.66666666666667, 16.66666666666667, -783.3333333333333, 391.66666666666663, 66.66666666666666, -25.0, -91.66666666666667, 25.000000000000014, -25.0, 16.66666666666667, -333.33333333333337, 150.0, 50.0, -49.99999999999999, -33.33333333333334, 41.66666666666667, -100.0, 41.66666666666667, -200.0, -33.33333333333333, 16.666666666666657, -16.66666666666667, -91.66666666666666, -25.0, -16.66666666666667, -83.33333333333331, -16.666666666666657, -41.66666666666667, -25.0, -33.33333333333334, -16.66666666666667, -33.33333333333333, 0.0, -74.99999999999999, 25.0, -41.66666666666667, 58.33333333333334, -33.33333333333333, 75.0, 16.66666666666667, 0.0, -41.66666666666666, -41.66666666666666, -41.666666666666686, 183.33333333333334, -91.66666666666667, -25.0, 58.33333333333334, 91.66666666666667, -141.66666666666669, -58.33333333333334, -16.666666666666657, 491.66666666666663, -8.333333333333329, 8.333333333333343, -25.0, 91.66666666666667, -83.33333333333331, -124.99999999999997, 116.66666666666663, 1000.0, 8.333333333333343, -66.66666666666666, -50.0, 75.0, -275.0, -375.0, -208.33333333333331, 583.3333333333334, -8.333333333333343, 108.33333333333333, 41.66666666666667, 200.0, -275.0, -300.00000000000006, -300.0, 1616.6666666666667, -99.99999999999999, 25.0, 66.66666666666667, 358.3333333333333, -258.33333333333337, -408.33333333333337, 158.33333333333337, 983.3333333333335, 16.666666666666657, -25.000000000000014, -66.66666666666667, 316.6666666666667, -950.0000000000001, -191.66666666666669, 58.33333333333337, 116.66666666666669, -25.000000000000014, -58.33333333333333, -16.66666666666667, 150.0, -158.33333333333334, -283.3333333333333, 58.33333333333337, 225.00000000000006, -416.6666666666667, 8.333333333333329, -41.66666666666666, 275.0, -391.66666666666663, 8.333333333333371, 99.99999999999994, 108.33333333333337, -216.66666666666666, -41.66666666666667, 0.0, 308.33333333333337, -66.66666666666663, -141.66666666666663, 66.66666666666669, -33.33333333333337, -66.66666666666666, 0.0, 100.00000000000001, 150.00000000000003, -208.33333333333331, -416.6666666666667, 33.33333333333337, 574.9999999999999, 41.66666666666666, 33.33333333333334, 33.33333333333333, 133.33333333333334, -1058.3333333333333, -333.33333333333337, 8.333333333333371, 766.6666666666666, -25.0, -41.66666666666667, 91.66666666666669, 150.0, -500.0, -183.33333333333337, -150.0, 550.0, 0.0, 8.333333333333336, -16.66666666666667, 8.333333333333343, -1050.0, -291.6666666666667, 33.33333333333334, 241.66666666666666, 0.0, -33.33333333333334, 58.33333333333334, 66.66666666666666, -241.66666666666669, -208.33333333333334, 91.66666666666667, 58.33333333333334, -8.333333333333329, -41.66666666666667, 33.33333333333334, 50.0, -141.66666666666666, -124.99999999999999, 16.66666666666667, -41.66666666666666, -116.66666666666666, -33.33333333333334, -83.33333333333331, 16.66666666666667, -99.99999999999999, 0.0, -83.33333333333334, 150.0, -41.66666666666667, 25.0, -58.33333333333333, 41.66666666666667, -58.33333333333334, -16.666666666666657, 16.666666666666657, 8.333333333333329, -8.333333333333329, -25.0, 16.666666666666657, -16.666666666666657, 8.333333333333343, -66.66666666666667, 33.33333333333334, -50.0, -16.666666666666657, 50.0, -8.333333333333343, -50.0, 8.333333333333343, -8.333333333333329, 16.666666666666664, 8.333333333333343, -25.0, 33.33333333333334, 25.000000000000014, 75.0, -66.66666666666667, -83.33333333333331, 33.33333333333333, -49.999999999999986, -8.333333333333343, 25.0, -25.0, 8.333333333333329, -16.666666666666657, 0.0, 83.33333333333333, -191.66666666666669, 100.0, 41.66666666666666, 8.333333333333329, -400.0, 125.0, -16.66666666666667, 66.66666666666667, -341.66666666666663, 683.3333333333334, 33.33333333333333, 125.00000000000001, -733.3333333333333, 66.66666666666666, 158.33333333333331, 0.0, -350.0, 1100.0, -41.66666666666667, -33.33333333333333, -466.6666666666667, 116.66666666666669, -141.66666666666666, -91.66666666666666, -216.66666666666663, -191.66666666666674, -33.33333333333333, -83.33333333333333, -1533.3333333333335, -408.3333333333333, -66.66666666666667, 25.0, -475.0, 425.0, 58.33333333333333, 49.999999999999986, -633.3333333333333, 183.33333333333331, -58.33333333333333, 108.33333333333331, -266.66666666666663, -191.66666666666663, -8.333333333333329, 91.66666666666667, -125.0, 166.66666666666669, -25.0, 41.66666666666667, -58.333333333333314, 199.99999999999994, -41.66666666666666, 141.66666666666669, -33.333333333333314, -50.0, 16.666666666666657, 33.33333333333334, 433.3333333333333, 291.6666666666667, -33.33333333333333, 16.66666666666667, -483.3333333333333, -33.33333333333337, -33.33333333333334, -8.333333333333329, -16.66666666666667, 0.0, 16.666666666666657, -33.33333333333334, 16.66666666666667, -33.33333333333334, -58.333333333333336, 41.66666666666667, 33.33333333333333, -33.33333333333333, 83.33333333333333, 8.333333333333329, 0.0, 58.333333333333336, 0.0, 58.333333333333336, -58.33333333333333, -41.66666666666667, -33.333333333333336, -16.66666666666667, -16.666666666666657, -8.333333333333329, -33.33333333333333, 16.66666666666667, 41.66666666666667, -16.666666666666657, -75.0, 41.66666666666667, -16.66666666666667, 50.0, 0.0, 0.0, -158.33333333333334, 133.33333333333334, -16.66666666666667, 58.33333333333333, 25.000000000000014, -116.66666666666666, -25.0, 25.0, -83.33333333333334, 175.0, -241.66666666666669, 158.33333333333331, -116.66666666666667, -133.33333333333334, -25.000000000000014, 16.666666666666657, -66.66666666666666, 283.3333333333333, -183.33333333333331, 625.0, -275.0, -25.0, -33.333333333333336, -33.333333333333336, 100.0, 1016.6666666666666, -41.66666666666667, 200.0, -566.6666666666667, 741.6666666666667, 16.66666666666667, 8.333333333333329, 216.66666666666669, 750.0, -141.66666666666669, 658.3333333333334, -283.33333333333337, -300.0, 75.0, 16.666666666666657, -8.333333333333314, 425.0, -225.0, 241.66666666666666, -141.66666666666669, -191.66666666666669, 8.333333333333314, -25.0, -75.0, 616.6666666666667, -75.0, 283.3333333333333, -266.66666666666663, 33.333333333333314, -116.66666666666667, 24.999999999999986, -58.333333333333314, 108.33333333333331, -116.66666666666667, 266.6666666666667, -758.3333333333334, 16.666666666666686, 8.333333333333343, 0.0, -2016.6666666666667, 475.0, -358.33333333333337, 716.6666666666667, -533.3333333333334, -75.0, 33.33333333333333, -16.666666666666657, -166.66666666666669, 666.6666666666667, -175.0, 416.66666666666663, -133.33333333333334, 66.66666666666663, -41.66666666666667, -25.0, -41.666666666666686, 1341.6666666666667, -133.33333333333331, 533.3333333333333, -225.00000000000003, -16.66666666666663, 125.0, -58.333333333333336, -58.333333333333314, 950.0, -66.66666666666667, 258.33333333333337, -483.33333333333337, -75.00000000000003, -50.0, 74.99999999999999, -41.666666666666686, 858.3333333333334, -83.33333333333334, 25.0, -408.33333333333337, -16.66666666666667, -58.333333333333336, -8.333333333333329, -33.33333333333334, 475.00000000000006, -33.333333333333336, 58.33333333333334, -466.6666666666667, 83.33333333333333, -66.66666666666666, -41.66666666666667, -50.0, 166.66666666666666, -41.66666666666667, -8.333333333333329, -75.0, -33.33333333333333, 41.66666666666667, -24.999999999999986, 8.333333333333329, 166.66666666666669, -58.33333333333334, -8.333333333333329, -41.66666666666666, 41.66666666666667, 50.0, 0.0, 0.0, 0.0, 0.0, 0.0, 0.0, 0.0, 0.0, 0.0, 0.0, 0.0, 0.0, 0.0, 0.0, 0.0, 0.0, 0.0, 0.0, 0.0, 0.0, 0.0, 0.0, 0.0, 0.0, 0.0, 0.0, 0.0, 0.0, 0.0, 0.0, 0.0, 0.0, 0.0, 0.0, 0.0, 0.0, 0.0, 0.0, 0.0, 0.0, 0.0, 0.0, 0.0, 0.0, 0.0, 0.0, 0.0, 0.0, 0.0, 0.0, 0.0, 0.0, 0.0, 0.0, 0.0, 0.0, 0.0, 0.0, 0.0, 0.0, 0.0, 0.0, 0.0, 0.0, 0.0, 0.0, 0.0, 0.0, 0.0, 0.0, 0.0, 0.0, 0.0, 0.0, 0.0, 0.0, 0.0, 0.0, 0.0, 0.0, 0.0, 0.0, 0.0, 0.0, 0.0, 0.0, 0.0, 0.0, 0.0, 0.0, 0.0, 0.0, 0.0, 0.0, 0.0, 0.0, 0.0, 0.0, 0.0, 0.0, 0.0, 0.0, 0.0, 0.0, 0.0, 0.0, 0.0, 0.0, 0.0, 0.0, 0.0, 0.0, 0.0, 0.0, 0.0, 0.0, 0.0, 0.0, 0.0, 0.0, 0.0, 0.0, 0.0, 0.0, 0.0, 0.0, 0.0, 0.0, 0.0, 0.0, 0.0, 0.0, 0.0, 0.0, 0.0, 0.0, 0.0, 0.0, 0.0, 0.0, 0.0, 0.0, 0.0, 0.0, 0.0, 0.0, 0.0, 0.0, 0.0, 0.0, 0.0, 0.0, 0.0, 0.0, 0.0, 0.0, 0.0, 0.0, 0.0, 0.0, 0.0, 0.0, 0.0, 0.0, 0.0, 0.0, 0.0, 0.0, 0.0, 0.0, 0.0, 0.0, 0.0, 0.0, 0.0, 0.0, 0.0, 0.0, 0.0, 0.0, 0.0, 0.0, 0.0, 0.0, 0.0, 0.0, 0.0, 0.0, 0.0, 0.0, 0.0, 0.0, 0.0, 0.0, 0.0, 0.0, 0.0, 0.0, 0.0, 0.0, 0.0, 0.0, 0.0, 0.0, 0.0, 0.0, 0.0, 0.0, 0.0, 0.0, 0.0, 0.0, 0.0, 0.0, 0.0, 0.0, 0.0, 0.0, 0.0, 0.0, 0.0, 0.0, 0.0, 0.0, 0.0, 0.0, 0.0, 0.0, 0.0, 0.0, 0.0, 0.0, 0.0, 0.0, 0.0, 0.0, 0.0, 0.0, 0.0, 0.0, 0.0, 0.0, 0.0, 0.0, 0.0, 0.0, 0.0, 0.0, 0.0, 0.0, 0.0, 0.0, 0.0, 0.0, 0.0, 0.0, 0.0, 0.0, 0.0, 0.0, 0.0, 0.0, 0.0, 0.0, 0.0, 0.0, 0.0, 0.0, 0.0, 0.0, 0.0, 0.0, 0.0, 0.0, 0.0, 0.0, 0.0, 0.0, 0.0, 0.0, 0.0, 0.0, 0.0, 0.0, 0.0, 0.0, 0.0, 0.0, 0.0, 0.0, 0.0, 0.0, 0.0, 0.0, 0.0, 0.0, 0.0, 0.0, 0.0, 0.0, 0.0, 0.0, 0.0, 0.0, 0.0, 0.0, 0.0, 0.0, 0.0, 0.0, 0.0, 0.0, 0.0, 0.0, 0.0, 0.0, 0.0, 0.0, 0.0, 0.0, 0.0, 0.0, 0.0, 0.0, 0.0, 0.0, 0.0, 0.0, 0.0, 0.0, 0.0, 0.0, 0.0, 0.0, 0.0, 0.0, 0.0, 0.0, 0.0, 0.0, 0.0, 0.0, 0.0, 0.0, 0.0, 0.0, 0.0, 0.0, 0.0, 0.0, 0.0, 0.0, 0.0, 0.0, 0.0, 0.0, 0.0, 0.0, 0.0, 0.0, 0.0, 0.0, 0.0, 0.0, 0.0, 0.0, 0.0, 0.0, 0.0, 0.0, 0.0, 0.0, 0.0, 0.0, 0.0, 0.0, 0.0, 0.0, 0.0, 0.0, 0.0, 0.0, 0.0, 0.0, 0.0, 0.0, 0.0, 0.0, 0.0, 0.0, 0.0, 0.0, 0.0, 0.0, 0.0, 0.0, 0.0, 0.0, 0.0, 0.0, 0.0, 0.0], [-100.0, -100.0, 166.66666666666697, -708.333333333333, -550.0, -225.0, 700.0, -1041.666666666667, 91.66666666666697, 108.33333333333394, 208.33333333333303, -1441.666666666667, 250.0, -166.66666666666697, 633.333333333333, 316.66666666666697, -83.33333333333303, 316.66666666666697, 33.33333333333394, -475.0, -283.33333333333394, 416.66666666666697, 150.0, -258.33333333333394, -166.66666666666697, 166.66666666666697, -225.0, 366.66666666666697, 308.33333333333303, 658.333333333333, -541.666666666667, -291.66666666666697, 66.66666666666697, 516.666666666667, -791.666666666667, 258.33333333333303, 391.66666666666697, -483.33333333333303, -325.0, -425.0, 316.66666666666697, 483.33333333333303, -400.0, 175.0, -158.33333333333303, 41.66666666666697, -675.0, 16.66666666666606, 108.33333333333303, 333.33333333333303, -150.0, 433.33333333333394, 316.66666666666697, 141.66666666666606, -741.6666666666661, -116.66666666666697, 291.66666666666697, 266.66666666666697, -66.66666666666697, 350.0, 75.0, -75.0, -316.66666666666697, -141.66666666666606, -116.66666666666697, -383.33333333333303, 25.0, 116.66666666666697, 208.33333333333303, 641.666666666667, -250.0, 175.0, -533.333333333333, 600.0, -525.0, -25.0, 83.33333333333303, -541.6666666666661, -141.66666666666697, 650.0, 508.33333333333303, 191.66666666666606, 691.666666666667, 91.66666666666697, -191.66666666666606, -8.33333333333303, -75.0, -108.33333333333303, 391.66666666666697, 175.0, -166.66666666666606, 749.9999999999995, -16.66666666666606, -16.66666666666606, -391.66666666666697, 58.33333333333303, 225.0, -158.33333333333303, 108.33333333333303, -133.33333333333303, -291.66666666666606, -166.66666666666606, 58.33333333333394, 133.33333333333394, 125.0, -291.66666666666697, 141.66666666666606, -200.0, 341.66666666666697, -183.33333333333303, 100.0, -16.66666666666697, 583.333333333333, -108.33333333333303, 0.0, 0.0, 416.66666666666697, 125.0, 150.0, -375.0, 133.33333333333303, -16.66666666666697, 316.66666666666697, -191.66666666666606, 658.333333333333, 33.33333333333303, 283.33333333333303, -150.0, 83.33333333333303, -225.0, 50.0, -483.33333333333394, -150.0, -241.66666666666606, -150.0, -50.0, -41.66666666666697, -250.0, -358.33333333333394, 658.3333333333339, 58.33333333333303, 508.33333333333303, -283.33333333333303, 58.33333333333303, 158.33333333333303, 400.0, 491.66666666666697, 458.33333333333394, 391.66666666666697, -83.33333333333303, -150.0, -100.0, -325.0, 350.0, 425.0, 25.0, 125.0, 133.33333333333394, 200.0, 233.33333333333303, -275.0, -500.0, 275.0, -33.33333333333303, -250.0, 275.0, 83.33333333333303, -233.33333333333303, -325.0, 50.0, -225.0, -275.0, -233.33333333333303, 8.33333333333303, 116.66666666666606, -191.66666666666697, 200.0, -58.33333333333303, 358.33333333333394, 633.333333333333, -425.0, -58.33333333333303, 375.0, -191.66666666666697, 258.33333333333303, -91.66666666666606, 75.0, -241.66666666666697, -150.0, 175.0, 266.66666666666697, 291.66666666666606, -541.666666666667, 50.0, 100.0, -41.66666666666606, 0.0, -191.66666666666697, -16.66666666666606, 250.0, 266.66666666666606, 108.33333333333303, -400.0, 200.0, 325.0, 83.33333333333303, -241.66666666666606, -275.0, -166.66666666666697, 125.0, -108.33333333333303, -241.66666666666606, 500.00000000000045, 200.0, -425.0, 425.0, -266.66666666666606, -91.66666666666606, -575.0, 108.33333333333394, 116.66666666666606, 608.333333333333, -200.0, -183.33333333333348, 308.33333333333303, -450.0, -341.66666666666606, -575.0, -8.33333333333303, -158.33333333333303, -341.66666666666606, -175.0, -183.33333333333303, -208.33333333333303, -300.0, 50.0, 66.66666666666697, -316.66666666666697, -366.66666666666606, 125.0, 133.33333333333303, -33.33333333333303, -100.0, 166.66666666666606, 541.666666666667, -133.33333333333394, 175.0, -100.0, 108.33333333333394, -391.66666666666697, -350.0, -491.66666666666697, 316.6666666666665, 350.0, -150.0, -66.66666666666697, 266.66666666666697, 58.33333333333394, -191.66666666666697, 66.66666666666697, -516.6666666666661, -58.33333333333303, -641.666666666667, 33.33333333333303, -133.33333333333394, -41.66666666666606, -375.0, 375.0, -108.33333333333303, 58.33333333333394, 225.0, -100.0, 300.0, 383.33333333333394, 0.0, -383.33333333333303, 158.33333333333303, 358.33333333333394, -333.33333333333303, -41.66666666666697, -216.66666666666697, 366.66666666666697, -8.33333333333394, -483.33333333333303, -141.66666666666697, -8.33333333333303, -191.66666666666697, 8.33333333333394, 16.66666666666697, 233.33333333333303, -633.333333333333, -58.33333333333303, 41.66666666666606, 16.66666666666697, -141.66666666666697, 208.33333333333303, 983.3333333333335, 25.0, 183.33333333333394, 200.0, -325.0, 300.0, 233.33333333333394, -350.0, -441.66666666666697, 241.66666666666697, -8.33333333333303, -133.33333333333303, -433.33333333333303, -91.66666666666606, -58.33333333333394, 141.66666666666697, 16.66666666666697, 141.66666666666606, 66.66666666666697, -100.0, 300.0, -450.0, -191.66666666666697, -91.66666666666606, -41.66666666666606, 433.33333333333303, 108.33333333333303, 175.0, 8.33333333333394, 225.0, -250.0, 408.33333333333303, 275.0, 358.33333333333394, -208.33333333333303, 150.0, 258.33333333333303, -308.33333333333303, 66.66666666666606, 233.33333333333394, -25.0, 141.66666666666697, -41.66666666666697, 316.66666666666697, 183.33333333333303, 75.0, 91.66666666666697, 16.66666666666606, -25.0, -50.0, 8.33333333333303, -333.33333333333303, -466.66666666666697, -133.33333333333303, -200.0, 50.0, -416.66666666666697, 300.0, 141.66666666666606, 100.0, -108.33333333333303, 383.33333333333394, -658.3333333333339, -158.33333333333394, -66.66666666666697, 275.0, 8.33333333333303, 108.33333333333394, 333.33333333333394, 166.66666666666697, 258.33333333333303, 166.66666666666697, -175.0, 233.33333333333303, -350.0, 241.66666666666606, -25.0, 175.0, 300.0, 150.0, -50.0, -75.0, -216.66666666666697, -483.33333333333303, -8.33333333333394, 183.33333333333394, 141.66666666666697, -58.33333333333303, 116.66666666666606, -108.33333333333303, -58.33333333333394, -241.66666666666697, 125.0, 25.0, 191.66666666666606, 33.33333333333394, 141.66666666666606, 433.33333333333303, -33.33333333333303, 291.66666666666697, 166.66666666666697, 133.33333333333303, 308.33333333333303, -475.0, 183.33333333333303, -16.66666666666606, -383.33333333333303, -8.33333333333394, -66.66666666666606, -33.33333333333303, -125.0, -283.33333333333303, -291.66666666666697, 108.33333333333303, -108.33333333333394, -258.33333333333303, 150.0, -8.33333333333303, -50.0, -216.66666666666606, 425.0, 433.33333333333394, -225.0, 208.33333333333303, -91.66666666666697, 16.66666666666697, 325.0, 541.6666666666661, -16.66666666666697, -16.66666666666697, 258.33333333333303, 66.66666666666697, -8.33333333333394, -350.0, 141.66666666666697, -191.66666666666697, 66.66666666666697, 325.0, 291.66666666666697, -250.0, 83.33333333333303, 183.33333333333303, -233.33333333333303, 33.33333333333303, 191.66666666666697, 216.66666666666697, -133.33333333333303, 33.33333333333303, 75.0, -366.66666666666697, -400.0, 83.33333333333303, 141.66666666666606, -33.33333333333303, -258.33333333333303, -391.66666666666697, 758.333333333333, -58.33333333333303, 41.66666666666697, 383.33333333333303, 8.33333333333394, -133.33333333333394, 150.0, -150.0, 33.33333333333334, 41.66666666666666, 25.0, 25.0, -8.333333333333343, -66.66666666666669, -16.666666666666657, 8.333333333333343, -50.0, -8.333333333333343, -91.66666666666669, 16.666666666666686, 50.0, 16.666666666666686, -58.33333333333334, -8.333333333333314, -25.0, 41.66666666666666, 8.333333333333343, 83.33333333333334, 41.66666666666666, 33.33333333333334, 50.0, -75.0, -8.333333333333314, 75.0, -33.33333333333334, 41.666666666666686, -16.666666666666657, 25.0, 66.66666666666666, -116.66666666666666, 66.66666666666667, 25.0, -91.66666666666669, 50.0, 8.333333333333343, 150.00000000000003, 0.0, -41.66666666666666, -91.66666666666666, -33.333333333333314, -58.333333333333314, -41.666666666666686, -75.0, 0.0, 33.33333333333334, 41.666666666666686, 8.333333333333314, 25.0, 41.666666666666686, 16.666666666666686, -41.66666666666667, 58.333333333333314, 25.0, 50.0, 33.333333333333314, -16.666666666666657, -50.0, -75.0, 41.666666666666686, -58.33333333333334, -83.33333333333334, 58.33333333333334, 66.66666666666669, 133.33333333333331, 74.99999999999999, 116.66666666666667, -16.666666666666657, 108.33333333333333, -75.0, -116.66666666666667, -91.66666666666666, -33.333333333333314, -50.0, -8.333333333333314, 25.0, 8.333333333333343, 0.0, -25.0, 8.333333333333343, -83.33333333333333, -41.66666666666666, 41.666666666666686, 8.333333333333314, 75.00000000000001, -16.666666666666657, 50.0, 50.0, -83.33333333333334, 0.0, 83.33333333333334, -58.333333333333314, 33.33333333333333, -25.0, -16.666666666666686, 41.66666666666666, 0.0, -58.333333333333314, -33.33333333333334, -41.666666666666686, 25.0, 25.0, 83.33333333333334, 41.666666666666686, 58.33333333333333, -100.0, 50.0, -33.333333333333314, -8.333333333333343, 75.0, -33.333333333333314, -58.33333333333334, 8.333333333333343, 50.0, 150.0, 50.0, 66.66666666666669, -16.666666666666657, 8.333333333333314, 8.333333333333314, -33.333333333333314, -8.333333333333343, 8.333333333333314, 33.333333333333314, -8.333333333333314, 66.66666666666666, 8.333333333333343, 25.0, -50.00000000000003, 41.66666666666666, 116.66666666666666, -50.0, 33.33333333333334, 0.0, 8.333333333333343, 41.66666666666666, 8.333333333333314, -16.666666666666657, -16.666666666666657, 74.99999999999999, 141.66666666666669, 41.66666666666666, -49.99999999999997, -41.66666666666666, -25.0, -108.33333333333331, 33.33333333333334, 50.0, -33.333333333333314, -58.33333333333334, 0.0, 16.666666666666657, -58.33333333333334, -8.333333333333343, 50.0, 33.33333333333334, 41.666666666666686, -75.0, -41.66666666666667, -66.66666666666669, 25.0, 0.0, -8.333333333333343, 33.333333333333314, 58.333333333333314, 8.333333333333314, 50.0, 8.333333333333343, 24.999999999999986, -58.33333333333334, 41.666666666666686, -33.333333333333314, 41.66666666666666, -91.66666666666669, -25.0, 16.666666666666657, 58.33333333333333, -33.33333333333334, 216.66666666666666, -8.333333333333343, 41.66666666666666, -16.666666666666686, 75.0, -58.33333333333334, 16.666666666666657, -8.333333333333343, 225.0, -25.00000000000003, 166.66666666666666, -158.33333333333334, 0.0, 50.0, 58.33333333333334, -16.666666666666657, 216.66666666666666, -108.33333333333334, 58.333333333333314, -200.00000000000003, 33.33333333333334, 33.33333333333334, 8.333333333333343, 25.0, 99.99999999999997, -175.0, 216.66666666666666, -50.0, -74.99999999999999, 16.666666666666657, -25.0, 100.0, 58.33333333333334, -133.33333333333334, 249.99999999999997, -333.33333333333337, -91.66666666666667, -83.33333333333331, 58.33333333333334, 141.66666666666669, 149.99999999999997, -216.66666666666666, 283.33333333333337, -91.66666666666669, -50.0, -25.0, 66.66666666666666, 75.0, 8.333333333333314, -250.00000000000003, 300.0, -66.66666666666669, 33.33333333333334, -25.0, 50.0, -116.66666666666666, 0.0, -125.0, 266.66666666666663, 33.333333333333314, 16.666666666666686, -8.333333333333343, 83.33333333333333, -33.33333333333334, 33.333333333333314, -124.99999999999997, -16.666666666666686, -283.33333333333337, 8.333333333333314, 16.666666666666686, -33.333333333333314, 33.33333333333334, 158.33333333333331, -33.333333333333314, 75.00000000000003, -341.66666666666674, -50.0, 33.33333333333334, -50.0, 0.0, 150.0, -91.66666666666666, -33.33333333333334, -125.0, 25.0, 108.33333333333331, 33.333333333333314, -50.0, 275.0, -166.66666666666666, 0.0, -225.0, 33.333333333333314, -50.0, -75.0, -25.0, 258.3333333333333, -33.333333333333314, 16.666666666666686, -216.66666666666669, 33.33333333333334, -16.66666666666667, -50.0, -25.0, 266.66666666666663, -108.33333333333331, 33.33333333333334, -108.33333333333334, -16.666666666666686, -50.0, -8.333333333333314, -66.66666666666666, 41.666666666666686, 16.666666666666657, -58.333333333333314, -33.33333333333334, 25.0, -16.666666666666657, -33.333333333333314, -8.333333333333343, -41.666666666666686, -91.66666666666666, 124.99999999999999, 16.666666666666657, 0.0, -75.0, -58.33333333333334, -33.333333333333314, 33.33333333333334, 41.66666666666666, 8.333333333333343, -8.333333333333343, -25.0, -33.33333333333334, 25.0, 8.333333333333314, 0.0, 16.666666666666686, -8.333333333333314, -58.333333333333314, 50.0, 33.333333333333314, 75.0, -133.33333333333334, 66.66666666666667, 33.33333333333334, -16.666666666666657, -58.33333333333334, 91.66666666666666, 58.333333333333314, -33.33333333333334, -83.33333333333331, -50.0, -133.33333333333331, 75.0, 0.0, 75.0, 16.666666666666657, 0.0, -74.99999999999997, 16.666666666666657, -150.00000000000003, 16.666666666666686, -16.666666666666686, 8.333333333333343, 83.33333333333331, 8.333333333333343, 58.33333333333333, 83.33333333333331, -166.66666666666669, 75.0, -33.33333333333334, -16.666666666666657, -8.333333333333343, -33.33333333333334, 8.333333333333329, 16.66666666666667, -175.0, 83.33333333333331, 58.33333333333334, -50.0, -74.99999999999999, 58.33333333333334, 33.33333333333334, -41.66666666666666, -33.333333333333314, -91.66666666666663, 83.33333333333334, 141.66666666666666, 50.0, -75.0, -16.666666666666657, 75.0, -141.66666666666666, -41.666666666666686, -33.333333333333314, -66.66666666666666, -66.66666666666669, -25.0, 0.0, 49.99999999999997, 16.666666666666686, -16.666666666666686, -83.33333333333331, -75.00000000000003, -58.33333333333334, 50.0, 16.666666666666686, 150.0, 8.333333333333314, 75.00000000000003, -116.66666666666667, -50.0, 50.0, 58.333333333333314, -8.333333333333314, 191.66666666666669, -241.66666666666663, -66.66666666666669, -83.33333333333334, -33.33333333333334, -100.0, -8.333333333333314, -16.666666666666686, 99.99999999999997, 8.333333333333314, 33.333333333333314, -41.66666666666666, -108.33333333333334, 125.0, -75.0, 8.333333333333343, 25.0, 33.33333333333334, -50.0, -75.0, -58.33333333333334, 50.0, -50.0, 8.333333333333343, 58.333333333333314, -116.66666666666666, 166.66666666666669, 58.33333333333334, -100.0, -41.66666666666666, 16.666666666666657, 33.33333333333334, 83.33333333333331, -166.66666666666663, 58.333333333333314, 58.33333333333334, 58.333333333333314, 41.66666666666666, -91.66666666666666, -50.0, 141.66666666666669, -166.66666666666669, 41.666666666666686, -50.0, -41.66666666666666, 99.99999999999999, -133.33333333333331, -25.0, 124.99999999999999, -166.66666666666669, 83.33333333333334, 66.66666666666669, -33.33333333333334, 50.0, 33.33333333333334, 33.33333333333334, 66.66666666666666, -66.66666666666666, 66.66666666666666, -8.333333333333314, 33.33333333333334, -50.0, -66.66666666666669, 41.66666666666666, 0.0, 0.0, -24.999999999999986, -25.0, -16.666666666666657, -33.33333333333334, -50.0, 25.0, -33.33333333333334, -75.0, -41.66666666666666, -49.999999999999986, 8.333333333333343, 75.0, 41.66666666666666, 0.0, 50.0, -16.666666666666657, -16.666666666666657, -66.66666666666669, -8.333333333333343, 16.666666666666686, -75.0, -33.33333333333334, -8.333333333333314, -8.333333333333343, 58.333333333333314, 16.666666666666657, 25.000000000000014, 25.0, 25.0, 25.0, -49.999999999999986, -116.66666666666669, 8.333333333333371, -75.0, -75.0, -133.33333333333334, 50.0, -133.33333333333331, -8.333333333333343, -200.00000000000003, 66.66666666666669, -16.666666666666686, 41.66666666666666, 108.33333333333334, 16.666666666666686, 58.33333333333334, 91.66666666666667, -58.33333333333334, 0.0, -50.0, 0.0, -25.0, -141.66666666666669, -41.66666666666666, 183.33333333333331, -16.666666666666657, 91.66666666666666, -25.0, -16.666666666666657, -66.66666666666666, 16.666666666666657, 0.0, -66.66666666666666, 25.0, 58.33333333333334, 0.0, 33.33333333333334, -41.666666666666686, 0.0, 66.66666666666666, 33.33333333333334, 16.666666666666657, -91.66666666666666, 0.0, -66.66666666666666, -8.333333333333343, -83.33333333333334, 16.666666666666657, -41.66666666666666, -41.66666666666666, -8.333333333333343, -33.33333333333334, 8.333333333333314, 33.33333333333334, -66.66666666666666, -25.0, 33.333333333333314, 8.333333333333314, -16.666666666666686, 83.33333333333334, -8.333333333333343, -16.666666666666657, -50.0, -24.999999999999986, 158.33333333333334, -149.99999999999994, 249.99999999999994, -91.66666666666667, 25.0, -25.0, -125.00000000000003, -50.0, 116.66666666666669, -375.00000000000006, 116.66666666666669, -41.666666666666686, -50.0, 25.0, 8.333333333333343, -83.33333333333331, -83.33333333333331, -308.33333333333326, 116.66666666666663, 50.0, 75.0, 8.333333333333314, 41.666666666666686, -75.0, 100.0, -325.0, 200.0, -16.666666666666657, -33.33333333333334, -133.33333333333334, 50.0, 16.666666666666657, 50.0, -333.3333333333333, 166.66666666666669, -25.0, 8.333333333333343, 66.66666666666669, -16.666666666666657, -8.333333333333314, -49.999999999999986, -49.99999999999997, 66.66666666666666, 150.0, -108.33333333333334, -33.333333333333314, 33.33333333333334, 66.66666666666667, 25.0, -91.66666666666669, 41.66666666666666, 66.66666666666669, 41.66666666666666, -83.33333333333334, 0.0, 8.333333333333343, 8.333333333333314, -91.66666666666667, -50.0, -16.666666666666686, -58.33333333333334, -50.0, 25.0, -25.0, -8.333333333333314, 25.0, 8.333333333333314, -33.33333333333334, -8.333333333333314, 99.99999999999997, 41.66666666666666, -33.33333333333334, 16.666666666666686, -16.666666666666686, -50.0, 75.0, 58.33333333333334, 0.0, -8.333333333333343, 33.33333333333334, 41.666666666666686, -16.666666666666657, -50.0, 50.0, -25.0, 41.666666666666686, 33.33333333333334, 99.99999999999999, -83.33333333333331, -41.66666666666666, 24.99999999999997, 25.0, -50.0, 41.66666666666666, -66.66666666666666, -41.66666666666666, -49.999999999999986, -25.0, -50.0, 133.33333333333334, 25.0, -25.0, 25.0, -100.0, -50.0, -66.66666666666669, -33.33333333333334, 166.66666666666669, 0.0, 33.33333333333334, 75.0, 25.0, -74.99999999999997, -50.0, 125.0, 250.00000000000003, -58.333333333333314, 0.0, -25.0, 125.00000000000001, -133.33333333333334, -33.333333333333314, -83.33333333333337, 275.0, 83.33333333333334, 41.66666666666666, -25.0, 108.33333333333331, -75.0, -58.33333333333337, 25.0, 233.33333333333334, 100.0, -16.666666666666657, 50.0, 25.0, -108.33333333333334, 41.66666666666666, -83.33333333333331, 108.33333333333334, 33.333333333333314, -33.33333333333334, 33.33333333333334, 83.33333333333334, -16.666666666666657, -66.66666666666669, 99.99999999999997, 91.66666666666666, -100.0, -58.33333333333334, 16.666666666666657, 125.00000000000003, 33.333333333333314, -66.66666666666666, 50.0, 16.666666666666686, 50.0, -100.0, 8.333333333333343, 216.66666666666669, -8.333333333333314, -8.333333333333314, -91.66666666666666, -41.666666666666686, -141.66666666666669, -75.0, 66.66666666666666, -141.66666666666666, -16.666666666666657, -83.33333333333331, -108.33333333333331, 175.0, 58.333333333333314, 41.66666666666666, 16.666666666666686, 16.666666666666686, -216.66666666666666, -41.666666666666686, 75.00000000000003, 83.33333333333334, 0.0, 16.666666666666657, 8.333333333333343, 66.66666666666666, -124.99999999999997, -100.0, 8.333333333333343, 233.33333333333331, -16.666666666666686, -8.333333333333343, -33.33333333333334, -16.666666666666657, -258.33333333333337, -41.66666666666666, -83.33333333333333, -8.333333333333314, -16.666666666666657, -33.33333333333334, -175.0, 49.99999999999997, -124.99999999999997, -50.0, 100.00000000000003, 33.33333333333334, -33.33333333333334, 8.333333333333343, 66.66666666666669, 25.0, 0.0, -66.66666666666669, 41.66666666666666, 8.333333333333314, 116.66666666666667, -25.0, 16.666666666666657, 33.33333333333334, 75.0, -33.333333333333314, -8.333333333333343, 66.66666666666666, 58.33333333333334, 0.0, 50.0, 100.0, 75.00000000000001, 8.333333333333343, -25.0, 33.333333333333314, -83.33333333333334, -25.0, 66.66666666666666, -16.666666666666657, -33.333333333333314, 75.0, -16.666666666666657, -58.33333333333334, -41.666666666666686, 8.333333333333343, -58.33333333333334, -41.66666666666666, -66.66666666666666, 0.0, -16.666666666666657, -58.33333333333334, -58.33333333333334, 16.666666666666686, -33.33333333333334, 8.333333333333314, 25.0, -8.333333333333314, 8.333333333333343, -8.333333333333314, 25.0, 25.0, 41.66666666666666, 16.666666666666686, -8.333333333333343, 41.66666666666666, -16.666666666666686, -75.0, 16.666666666666657, 25.0, -8.333333333333314, 16.666666666666657, 25.0, -33.33333333333334, 8.333333333333343, -191.66666666666669, 100.0, 58.333333333333314, 0.0, -16.666666666666657, -8.333333333333371, -58.33333333333334, 41.66666666666666, -91.66666666666666, 8.333333333333314, -66.66666666666667, 8.333333333333343, -124.99999999999997, 74.99999999999997, -25.000000000000014, 16.666666666666686, 66.66666666666666, -8.333333333333343, 41.66666666666666, 66.66666666666667, -83.33333333333331, 0.0, -91.66666666666666, 141.66666666666669, -316.66666666666663, -33.33333333333334, 0.0, -58.33333333333334, -58.33333333333334, 149.99999999999997, 0.0, -74.99999999999999, 58.33333333333334, -58.333333333333314, -75.0, 66.66666666666667, -50.0, 158.33333333333331, 58.33333333333334, 133.33333333333334, -50.0, -33.33333333333334, -124.99999999999999, 58.33333333333334, -83.33333333333334, 41.666666666666686, -8.333333333333343, -41.66666666666666, 175.0, 166.66666666666669, 66.66666666666669, 166.66666666666666, 50.0, 41.66666666666666, -33.333333333333314, 25.0, -75.0, -33.33333333333334, 83.33333333333334, 16.666666666666657, -66.66666666666666, 25.0, 33.333333333333314, -108.33333333333333, 8.333333333333343, 150.0, 100.0, 50.0, -58.33333333333333, -91.66666666666666, -16.666666666666657, -58.33333333333334, -108.33333333333334, -8.333333333333314, 8.333333333333314, 8.333333333333314, 0.0, 8.333333333333314, 0.0, 0.0, -8.333333333333314, -58.33333333333333, 83.33333333333331, 8.333333333333343, 0.0, 0.0, -16.666666666666657, -41.666666666666686, -41.666666666666686, 75.0, 8.333333333333343, 8.333333333333314, 25.0, -50.0, -41.66666666666666, 99.99999999999999, 16.666666666666657, 125.0, -66.66666666666669, 100.00000000000001, 58.333333333333314, 49.99999999999997, -83.33333333333334, -33.33333333333334, -133.33333333333331, -8.333333333333343, -58.333333333333314, 133.33333333333334, -108.33333333333334, 8.333333333333343, -25.0, 50.0, -33.33333333333334, 158.33333333333331, 75.0, 41.66666666666666, -16.666666666666657, 25.0, 0.0, -8.333333333333343, -91.66666666666666, 66.66666666666669, -83.33333333333334, 41.66666666666666, -83.33333333333334, 16.666666666666657, 0.0, -50.0, -108.33333333333334, 50.00000000000003, -91.66666666666669, 91.66666666666669, 16.666666666666657, 75.0, -16.666666666666686, 16.666666666666657, 8.333333333333343, 133.33333333333331, -16.666666666666657, 16.666666666666686, -124.99999999999997, 116.66666666666669, -33.33333333333334, 50.0, -8.333333333333343, 33.333333333333314, -150.0, 91.66666666666669, -75.0, -24.99999999999997, 49.999999999999986, 0.0, 0.0, 158.33333333333334, -41.666666666666686, 225.0, -33.333333333333314, -33.33333333333334, -75.00000000000001, -16.666666666666686, -99.99999999999997, 150.00000000000003, 16.666666666666686, 25.0, 8.333333333333343, -58.33333333333334, -83.33333333333334, 8.333333333333314, -58.333333333333314, 100.00000000000003, 25.0, 108.33333333333331, -158.33333333333334, -41.66666666666666, 91.66666666666666, 0.0, 58.33333333333334, 91.66666666666666, -66.66666666666669, 125.0, 0.0, -66.66666666666669, 66.66666666666666, 41.66666666666667, -83.33333333333334, 125.00000000000003, 41.66666666666667, -8.333333333333314, -141.66666666666666, 25.0, 41.666666666666686, -16.666666666666686, -33.33333333333334, 25.0, -83.33333333333334, 50.0, 41.66666666666666, -41.66666666666666, 16.666666666666657, 66.66666666666669, 41.66666666666666, 33.333333333333314, -33.33333333333334, 50.0, -91.66666666666666, -50.0, 8.333333333333314, -58.33333333333334, -33.333333333333314, 41.666666666666686, 58.33333333333333, -16.666666666666657, 16.666666666666657, 41.666666666666686, -8.333333333333343, 0.0, 0.0, 0.0, 0.0, 0.0, 0.0, 0.0, 0.0, 0.0, 0.0, 0.0, 0.0, 0.0, 0.0, 0.0, 0.0, 0.0, 0.0, 0.0, 0.0, 0.0, 0.0, 0.0, 0.0, 0.0, 0.0, 0.0, 0.0, 0.0, 0.0, 0.0, 0.0, 0.0, 0.0, 0.0, 0.0, 0.0, 0.0, 0.0, 0.0, 0.0, 0.0, 0.0, 0.0, 0.0, 0.0, 0.0, 0.0, 0.0, 0.0, 0.0, 0.0, 0.0, 0.0, 0.0, 0.0, 0.0, 0.0, 0.0, 0.0, 0.0, 0.0, 0.0, 0.0, 0.0, 0.0, 0.0, 0.0, 0.0, 0.0, 0.0, 0.0, 0.0, 0.0, 0.0, 0.0, 0.0, 0.0, 0.0, 0.0, 0.0, 0.0, 0.0, 0.0, 0.0, 0.0, 0.0, 0.0, 0.0, 0.0, 0.0, 0.0, 0.0, 0.0, 0.0, 0.0, 0.0, 0.0, 0.0, 0.0, 0.0, 0.0, 0.0, 0.0, 0.0, 0.0, 0.0, 0.0, 0.0, 0.0, 0.0, 0.0, 0.0, 0.0, 0.0, 0.0, 0.0, 0.0, 0.0, 0.0, 0.0, 0.0, 0.0, 0.0, 0.0, 0.0, 0.0, 0.0, 0.0, 0.0, 0.0, 0.0, 0.0, 0.0, 0.0, 0.0, 0.0, 0.0, 0.0, 0.0, 0.0, 0.0, 0.0, 0.0, 0.0, 0.0, 0.0, 0.0, 0.0, 0.0, 0.0, 0.0, 0.0, 0.0, 0.0, 0.0, 0.0, 0.0, 0.0, 0.0, 0.0, 0.0, 0.0, 0.0, 0.0, 0.0, 0.0, 0.0, 0.0, 0.0, 0.0, 0.0, 0.0, 0.0, 0.0, 0.0, 0.0, 0.0, 0.0, 0.0, 0.0, 0.0, 0.0, 0.0, 0.0, 0.0, 0.0, 0.0, 0.0, 0.0, 0.0, 0.0, 0.0, 0.0, 0.0, 0.0, 0.0, 0.0, 0.0, 0.0, 0.0, 0.0, 0.0, 0.0, 0.0, 0.0, 0.0, 0.0, 0.0, 0.0, 0.0, 0.0, 0.0, 0.0, 0.0, 0.0, 0.0, 0.0, 0.0, 0.0, 0.0, 0.0, 0.0, 0.0, 0.0, 0.0, 0.0, 0.0, 0.0, 0.0, 0.0, 0.0, 0.0, 0.0, 0.0, 0.0, 0.0, 0.0, 0.0, 0.0, 0.0, 0.0, 0.0, 0.0, 0.0, 0.0, 0.0, 0.0, 0.0, 0.0, 0.0, 0.0, 0.0, 0.0, 0.0, 0.0, 0.0, 0.0, 0.0, 0.0, 0.0, 0.0, 0.0, 0.0, 0.0, 0.0, 0.0, 0.0, 0.0, 0.0, 0.0, 0.0, 0.0, 0.0, 0.0, 0.0, 0.0, 0.0, 0.0, 0.0, 0.0, 0.0, 0.0, 0.0, 0.0, 0.0, 0.0, 0.0, 0.0, 0.0, 0.0, 0.0, 0.0, 0.0, 0.0, 0.0, 0.0, 0.0, 0.0, 0.0, 0.0, 0.0, 0.0, 0.0, 0.0, 0.0, 0.0, 0.0, 0.0, 0.0, 0.0, 0.0, 0.0, 0.0, 0.0, 0.0, 0.0, 0.0, 0.0, 0.0, 0.0, 0.0, 0.0, 0.0, 0.0, 0.0, 0.0, 0.0, 0.0, 0.0, 0.0, 0.0, 0.0, 0.0, 0.0, 0.0, 0.0, 0.0, 0.0, 0.0, 0.0, 0.0, 0.0, 0.0, 0.0, 0.0, 0.0, 0.0, 0.0, 0.0, 0.0, 0.0, 0.0, 0.0, 0.0, 0.0, 0.0, 0.0, 0.0, 0.0, 0.0, 0.0, 0.0, 0.0, 0.0, 0.0, 0.0, 0.0, 0.0, 0.0, 0.0, 0.0, 0.0, 0.0, 0.0, 0.0, 0.0, 0.0, 0.0, 0.0, 0.0, 0.0, 0.0, 0.0, 0.0, 0.0, 0.0, 0.0, 0.0, 0.0, 0.0, 0.0, 0.0, 0.0, 0.0, 0.0, 0.0, 0.0, 0.0, 0.0, 0.0, 0.0]] caption="Most Recent Time Trace"
  out "Delta Fl. 1":dbl
  out "Delta Fl. 2":dbl
  out "All Signals":waveform(dbl)[](graph)=[{"t0"=timestamp(2751.0000000002074 s since 1904-01-01), "dt"=0.02, "Y"=[0.0, 0.0, 0.0, 0.0, 0.0, 0.0, 0.0, 0.0, 0.0, 0.0, 0.0, 0.0, 0.0, 0.0, 0.0], "attributes"=variant("NI_ChannelName"=variant(string "APD 1"))}, {"t0"=timestamp(2751.0000000002074 s since 1904-01-01), "dt"=0.02, "Y"=[0.0, 0.0, 0.0, 0.0, 0.0, 0.0, 0.0, 0.0, 0.0, 0.0, 0.0, 0.0, 0.0, 0.0, 0.0], "attributes"=variant("NI_ChannelName"=variant(string "APD 2"))}, {"t0"=timestamp(2751.0000000002074 s since 1904-01-01), "dt"=0.15, "Y"=[-0.020049210394969354, -0.02003592505550746], "attributes"=variant("NI_ChannelName"=variant(string "T1 Y"))}, {"t0"=timestamp(2751.0000000002074 s since 1904-01-01), "dt"=0.15, "Y"=[0.03074231675925172, 0.03074526419399293], "attributes"=variant("NI_ChannelName"=variant(string "T1 X"))}, {"t0"=timestamp(2751.0000000002074 s since 1904-01-01), "dt"=0.15, "Y"=[2.9160941496017294, 2.916128360850853], "attributes"=variant("NI_ChannelName"=variant(string "T1 Sum"))}, {"t0"=timestamp(2751.0000000002074 s since 1904-01-01), "dt"=0.15, "Y"=[-0.002644972968316131, -0.002638961391604115], "attributes"=variant("NI_ChannelName"=variant(string "T2 Y"))}, {"t0"=timestamp(2751.0000000002074 s since 1904-01-01), "dt"=0.15, "Y"=[-0.011335016186436862, -0.011341032214389745], "attributes"=variant("NI_ChannelName"=variant(string "T2 X"))}, {"t0"=timestamp(2751.0000000002074 s since 1904-01-01), "dt"=0.15, "Y"=[2.746599475081634, 2.746642933439132], "attributes"=variant("NI_ChannelName"=variant(string "T2 Sum"))}, {"t0"=timestamp(2751.0000000002074 s since 1904-01-01), "dt"=0.15, "Y"=[-0.526083166086966, -0.5261552546492463], "attributes"=variant("NI_ChannelName"=variant(string "T1 FB X"))}, {"t0"=timestamp(2751.0000000002074 s since 1904-01-01), "dt"=0.15, "Y"=[3.0920304879909737, 3.0920243537705665], "attributes"=variant("NI_ChannelName"=variant(string "T2 FB Sum"))}, {"t0"=timestamp(2751.0000000002074 s since 1904-01-01), "dt"=0.15, "Y"=[-0.7128125059590501, -0.7128388598091219], "attributes"=variant("NI_ChannelName"=variant(string "T2 FB X"))}, {"t0"=timestamp(2751.0000000002074 s since 1904-01-01), "dt"=0.15, "Y"=[2.9122738731040343, 2.91227808465834], "attributes"=variant("NI_ChannelName"=variant(string "T2 FB Sum"))}, {"t0"=timestamp(2751.0000000002074 s since 1904-01-01), "dt"=0.15, "Y"=[-0.0023344523453474137, -0.002339854121524665], "attributes"=variant("NI_ChannelName"=variant(string "PSD Y"))}, {"t0"=timestamp(2751.0000000002074 s since 1904-01-01), "dt"=0.15, "Y"=[-0.0026477858821374683, -0.002642139957884409], "attributes"=variant("NI_ChannelName"=variant(string "PSD X"))}, {"t0"=timestamp(2751.0000000002074 s since 1904-01-01), "dt"=0.15, "Y"=[0.014415417950986964, 0.014429639576402777], "attributes"=variant("NI_ChannelName"=variant(string "PSD Sum"))}]
  in  "Signals to Plot":i32(listbox)=9
  out "Trap Disp. Freq. (Hz)":dbl=6.666666666666667 caption="Freq. (Hz)" format="%#_6p"
  out "Display Period (s)":dbl=0.15 caption="Period (s)" format="%#_6p"
  in  "Trap Disp. Downsample":dbl=10000.0 caption="Downsample" max=20000.0
  in  "APD Disp. Scale":dbl=0.1 caption="Scale (Divide,\nfor above plot only)"
  in  "APD Disp. Downsample":dbl=2.0 caption="Integrate" min=1.0 max=30.0 step=1.0
  out "APD Display Freq. (Hz)":dbl=50.0 caption="Freq. (Hz)"
  out "APD Display Period (s)":dbl=0.02 caption="Period (s)"
  out "FFT 1":cluster{"f0":dbl, "df":dbl, "magnitude":dbl[]}[](graph)=[{"f0"=0.0, "df"=16.666666666666668, "magnitude"=[-331.1367572010275, -79.05506245821404, -86.61411242440559, -88.4728176091699, -90.3181253945935, -94.12566333707997, -92.52740723119955, -94.92192587982518, -99.60936585245742, -96.87568627870715, -94.02570383337763, -83.8058550151726, -97.57441397235512, -101.59968530846606, -101.523049255742, -103.35038532190343, -101.58594091014982, -102.96098031851216, -91.39759462745924, -103.75019963279499, -104.45030075054324, -103.04245334279298, -104.0720279134107, -106.06482372394834, -103.69131867828104, -104.40395035115309, -105.96420043276396, -107.6735556337804, -106.673030006608, -107.34889066208132, -108.05626565233933, -106.25659018850432, -105.29934513380842, -105.43096056709592, -108.3728498841465, -106.0555440144992, -105.78001282181421, -107.48741857324953, -108.67624970548897, -105.39976667156175, -105.91413119232612, -109.4222808198164, -107.0898971593174, -107.91164191890915, -108.26032038855709, -107.58332347164534, -108.23559688234297, -108.01271040303237, -107.66511723652701, -106.51901583170391, -109.27249501469946, -108.55647681594805, -107.93499259231463, -107.05068166453935, -109.13641475410455, -109.29679733781423, -108.19360835527803, -109.57747591546632, -109.58364591011674, -110.47061433372711, -109.8144340420426, -108.79067462293897, -107.54887553357234, -107.99559866705923, -108.85023923652685, -109.68733225238618, -108.51101278437793, -108.51620475114115, -108.22212402200637, -104.63726950302143, -110.2989919678048, -107.61796444414897, -108.68882962798736, -104.79193983043893, -103.59504263746938, -93.64633660288543, -101.9191640501395, -105.73717393151816, -108.92572458793902, -107.43962662800902, -107.79595323081325, -107.0923101993207, -108.17603277205289, -107.87074270713183, -109.20899066381877, -108.61832060412445, -109.10072003106593, -105.76480632823524, -108.60877649218978, -109.67541158970121, -110.2286232768028, -109.84952155309578, -109.33772024076384, -109.95251642394683, -110.14777282585466, -109.13825677905699, -110.05989365698167, -109.39359990189426, -110.56255614635295, -109.66477183197163, -108.9397158528824, -110.26529907650465, -109.20049464984628, -108.20183857013548, -109.09752250184418, -108.00440442238454, -108.35465963524055, -111.16774134451799, -110.34812550238405, -108.94506763426756, -108.72845542102493, -109.41512344014713, -112.44661664432377, -110.35437330889101, -111.32939440655925, -109.42989530434981, -110.98084669076195, -111.92160561143541, -108.57755551751093, -111.40042616180912, -110.15284955891853, -112.21455132279115, -111.40787773511747, -108.82949641635288, -110.13442122547907, -111.42229298204664, -112.06314940885191, -110.6015308813694, -109.51144097251623, -111.15989713761475, -110.25535755335385, -109.65868178057926, -110.51649885452997, -109.77194745285269, -108.4234206864394, -109.50892632093968, -109.46471287444389, -107.92241289271415, -109.72283805386196, -108.63426821579918, -110.37316681536255, -111.09713996884652, -110.32903619589223, -105.32012665515045, -107.36858557554393, -108.00382215905725, -110.06430686942338, -108.81666625979916, -110.01277074453823, -110.94194741225512, -109.65934609082873, -107.80979136006962, -112.81333866824724, -111.61474300955487, -109.83998277184975, -109.45953946904639, -109.79640584952526, -108.19172301667324, -109.28894656674316, -107.61471301278785, -108.83814006090513, -109.08866847726084, -108.20250571862371, -107.96222236861584, -107.03811197900873, -108.93533000393974, -107.74482548035408, -110.79811544577694, -111.1387476496877, -107.42970105883512, -109.18442281176472, -108.73546184641192, -108.71800246690864, -108.51945944378063, -108.06825856571285, -107.27210712368412, -108.12304695877637, -107.84933283677306, -109.73682373154998, -109.32284761503395, -109.31328817453769, -106.68762108642842, -109.79203616876461, -109.9020278896408, -110.27080024357275, -108.54152101558762, -111.00464391726017, -112.42244020766577, -110.82707315747889, -111.00344011890857, -109.90461839395674, -109.42877207451863, -109.73549298167016, -111.67494793393293, -108.85799077901427, -108.5348443278263, -109.803781083881, -108.30644755543659, -108.5079527456017, -111.2055351312823, -108.53089994340155, -108.01739789012176, -108.70360662855235, -107.95873456794631, -109.58297170693093, -108.9372401694271, -110.15921663527153, -109.22399119911955, -110.89883651739237, -108.92840112258382, -110.0545300523626, -109.05961065387005, -109.45831398589371, -108.61239387653227, -110.13001256174265, -108.80060224137931, -109.46327400696283, -108.0177965824709, -109.29727944627197, -110.3237255895986, -109.03258262543821, -110.97880178489321, -109.70034895077919, -111.16405638194153, -109.17324451464711, -109.65698250854277, -108.96750235822178, -112.00534231585624, -108.69274607723942, -108.98110446396657, -108.40723795464795, -111.44459094807324, -111.74799245277113, -111.1601960491512, -108.92048232753773, -110.30506377784799, -111.33145973979093, -110.91850998672503, -110.33684985776448, -108.90206518366908, -109.28458878227542, -108.98773986023751, -110.85813863075646, -109.00041591105906, -110.84543686681204, -109.84382395806176, -109.69722434763266, -108.50915601095721, -107.80829925826895, -110.59736107582401, -109.75377770317087, -109.3992084496136, -110.51151565846742, -112.49753959826434, -109.7299632589479, -109.54070743868353, -109.90314341132164, -111.05974202976806, -109.03766862152392, -109.46667095459878, -109.52800799036197, -111.3163121356807, -110.07817134522178, -108.69251657453547, -109.40472158898045, -109.71400709815576, -110.60534468715097, -109.46937396724682, -107.70342491418788, -109.86331122597839, -108.64971387994616, -110.90117371097081, -108.34928840565928, -110.04172889660904, -111.52979926554961, -110.34759300823305, -109.62712781837159, -109.24131154553284, -110.23196152450447, -108.68509612326807, -108.0246905483419, -106.61876139289784, -101.5519630114271, -80.57695480953835, -102.03744443354402, -107.1449217193017, -110.0695213407169, -106.61597783999268, -110.79221011808191, -109.58974545931426, -109.1149802216988, -109.20993813088597, -109.63768480465863, -110.10428394219181, -109.08445084271477, -108.83472375362581, -109.69508502050168, -108.05588796178941, -110.62586360101581, -109.95315261676905, -107.52208264977473, -108.80708007514875, -110.43484881098874, -110.45942171588936, -107.83804717866751, -109.98973910294193, -109.3496496054193, -108.425252911127, -110.94579264380809, -108.54181722177951, -108.67696070083541, -108.4150202151644, -109.24973583101504, -112.0454922608961, -111.29046597340738, -110.75018248960077, -109.38326363603683, -109.2033340336957, -109.45076170874889, -109.52878049853727, -109.32340869724774, -110.98123395128233, -110.75736340635505, -109.7218385823809, -107.97422606064993, -109.77313701758703, -110.95948744392717, -110.08996774172691, -108.51011830110778, -109.78063140243836, -110.65996628628228, -109.83684298615616, -110.33329049188029, -110.13755118968292, -110.3717925645783, -108.55302219178951, -106.86811628734195, -108.6302156589162, -108.75341391045045, -108.32589578384841, -108.70061474734084, -112.30742263527534, -109.16842570592085, -109.29767035534508, -108.87829025017463, -108.2255616391397, -108.4316108616088, -108.82995906929271, -110.40135575415563, -109.51623498946435, -109.79409808792403, -107.03832759632121, -108.36534528684132, -109.72010868372905, -107.90933028179892, -106.95643597294047, -111.29929166165778, -110.23001135794706, -108.98838015381585, -109.79115357104436, -108.18627479511115, -108.14988122174307, -109.12074063466532, -109.41904850488358, -111.40409873721113, -108.83156790193294, -108.77032248953847, -108.88363158686694, -108.47515048290681, -105.94172147874599, -109.38146940214403, -109.21277078848794, -108.11309390545507, -110.70840012427504, -109.5504457849329, -109.52330684534209, -110.06776026911132, -108.21949434182314, -111.21266686269992, -108.78581501170974, -108.43115799297222, -109.63260325780062, -109.84070220619535, -109.72041980780126, -110.29615941882527, -110.60316734262464, -108.79165446414692, -110.95840439895592, -109.64926233107009, -109.16526769544322, -108.65292362430982, -109.56113898129935, -109.85693046339026, -108.92316027325207, -109.79492493553914, -109.38157962945887, -110.24545136266825, -109.30031463492487, -109.0795429936869, -111.4091719525013, -108.63499083917162, -108.43863465339358, -109.23207864880891, -111.21947487191643, -109.24525201480154, -109.56842406077318, -109.46711940800672, -111.91389548262572, -108.15655736690546, -108.71882059966947, -111.26328503478568, -110.95027143873176, -108.4853106242357, -110.36902802777546, -109.9314203579182, -108.77686164101732, -108.71871020068312, -111.04829661168574, -109.95072655339462, -109.88221342875462, -109.53241732756136, -108.2625005404823, -108.00677030040697, -110.19659317581693, -108.93858924796267, -109.46817875483995, -110.78063992017232, -111.11066570318451, -110.78774336696706, -109.19199744617812, -108.54914256407436, -109.28414960420909, -110.64143585101183, -110.5855350821307, -109.47578632252726, -108.89705360836223, -109.89214013612292, -107.93271261027171, -109.32631601340563, -108.60274611341092, -109.40110159872573, -110.889237682208, -110.01391165813328, -109.99747108785071, -108.65542819213674, -110.37211847668736, -110.44656500845738, -110.8128133834973, -108.8909299260433, -110.19551227077532, -111.37647266643523, -110.83802189730321, -109.98519377913681, -110.52378970770522, -108.16970420057817, -110.70974729773344, -110.76836765494402, -110.26884275594577, -109.22041044268806, -109.87809744746195, -107.76823252107832, -109.12119474042969, -110.28066108731146, -108.55000033509207, -110.18152097767907, -110.73030521152278, -111.49470908029893, -110.2320929919509, -110.03370979233021, -109.79181668155233, -108.6673501209991, -109.86695766650877, -107.88926518046961, -110.95525003776572, -109.18130359755742, -110.42618009658618, -107.90341931158893, -111.44736855661769, -110.72634267386593, -109.29945988519303, -107.67889101961411, -108.81148059987765, -109.13375212757057, -109.8122873383549, -109.80176697684155, -109.96342275204768, -109.90406635707086, -108.75674342748256, -110.12362902701081, -109.82151095527837, -108.62543344241836, -110.09171852771195, -110.21434637862887, -109.97254504855631, -109.27043209093468, -111.35149588204125, -110.12399876776051, -111.65983675538546, -109.28788875768564, -110.86554069990251, -111.26990906470603, -108.60956517491746, -111.49613890850938, -111.79685722966795, -109.26269485364045, -110.38555615546439, -109.40641023162068, -110.966136593156, -108.78892524584494, -110.29340727375603, -111.44032043281035, -109.95212021173755, -109.79233511584334, -112.41184021118175, -109.73687851881148, -108.65493879781806, -110.76132988919045, -108.43230346094671, -110.32968175895853, -110.29890782023821, -108.77609076424456, -110.3298662333555, -109.47734504217333, -108.2677295732245, -109.21234363352882, -107.83278941978479, -108.85136784424789, -108.43241251530755, -109.76609391460555, -108.53204373005357, -110.9660641972934, -110.3152512161094, -110.72570499399905, -109.23877906286317, -111.72407743101837, -109.20311421918561, -108.06021800233717, -109.29288625761943, -108.78395253409145, -111.85250172876302, -108.78827588901797, -109.79775055719482, -109.12089297455859, -109.49896359356035, -110.34432647103819, -107.94700097960238, -109.30489238477631, -108.89170290869342, -108.82574563272509, -110.11024077194833, -107.37946433552314, -109.60167933458756, -107.80625057819019, -110.11489057210264, -107.35436859378505, -105.69819484613895, -109.11280625683739, -109.27770293057978, -107.7053735252589, -109.75022444894368, -109.3310543596577, -107.87683693707739, -108.19931495338068, -109.26462246191564, -106.71885779297867, -100.00018022217961, -92.54434511397295, -107.20472143807373, -107.39203415155283, -110.04461177268398, -108.48860496315312, -109.0057168110333, -108.37627790492552, -108.4108380728248, -109.65509454313073, -109.64243000632982, -97.04219069306761, -109.0928856629964, -107.9760697315632, -107.52611064047497, -108.87702814778996, -109.08437599027614, -110.70097118837974, -109.00969860961283, -110.38275386163214, -110.0699155421545, -106.91498895181175, -106.22178738309017, -109.36827866896039, -107.59953130968307, -109.19516217272808, -108.31502495393616, -109.384158926223, -107.11670654202719, -108.09436312738853, -110.14559230873704, -109.84997663447679, -107.83465335309926, -108.60947100624459, -108.9932479423645, -109.17174810371898, -108.79457339828916, -109.40909327982367, -109.6328723628302, -109.51081854476179, -107.63054408568418, -109.63728404010122, -108.51163794839918, -107.55002282725216, -108.97796212764939, -107.24648164623483, -112.21470452291085, -108.74294024554423, -109.62070777514892, -108.05768666239368, -109.8224946685739, -109.34575507446003, -108.53536952609525, -109.60789300457671, -107.56681538208278, -109.22777325016398, -108.79047910308894, -110.10332477250668, -108.00206387955672, -108.45604004720035, -109.00645795765472, -109.81039564269616, -108.92785144634745, -108.3978471520567, -107.94411095685999, -110.53486519304262, -108.8773780319227, -109.03345093296107, -107.30746693745031, -108.54277704832029, -108.77629108166091, -108.91111762599647, -107.74965195880401, -109.97375370738439, -109.76326492689246, -107.91717581777407, -109.0730556927617, -107.66804873204664, -110.40438871064791, -108.05794247751498, -108.80206615156494, -107.51329354700796, -108.83687012994949, -107.57713176895379, -107.94774159581414, -109.41894615439651, -107.10869425078764, -110.51480854078629, -108.92221367099775, -109.91358786461535, -110.1744263092835, -109.30795472883494, -107.91359710691006, -109.77888185049835, -109.52060975706438, -108.66686651982212, -108.71041801553639, -110.13619546359467, -108.87957097273856, -109.72150387215271, -109.00776068810654, -109.70251113927438, -110.75769213896399, -108.53234896741436, -109.69439526582246, -110.15412541604617, -108.25183374628219, -107.97402569656481, -110.34920156998648, -108.45106995186384, -108.82031145748209, -111.38690005057539, -107.01968459818563, -110.3044500039584, -110.8755481852125, -111.08915057663255, -107.94824988655199, -110.21669144934839, -109.90539774633154, -109.58985438756767, -110.12258796623348, -109.41689951612143, -109.31128210476795, -109.00258476567323, -109.11093063041056, -108.83347064311234, -108.32685287566952, -109.44770946560935, -108.40145063144861, -109.68448193892085, -108.76525439243828, -107.62837139034596, -107.39300298848994, -109.36993934990318, -109.2465218489418, -106.66307369796812, -110.15891092764934, -109.57151745419041, -108.92425698310808, -109.8036704717834, -108.79751146756549, -109.25926431818017, -108.46260574057584, -109.1967554647261, -110.63319560262356, -109.02343067385144, -111.22073171487528, -109.4731095097105, -109.69335000085164, -109.48782989577005, -107.95204227683271, -108.19468255763758, -111.36195112053247, -109.55696116543685, -110.3130767640534, -108.9621824253354, -109.99735074896789, -109.20198058456344, -108.12100614259485, -111.27227490807289, -110.09248554008288, -109.14395535060149, -110.80882692379708, -109.22632926901655, -108.64497210802793, -111.00030482190711, -111.1317849358033, -107.43140429257826, -107.9783302193555, -109.2639893652291, -108.97008485446163, -108.66556668859064, -108.12995785876932, -109.73001061107855, -108.09691302413727, -110.68391499215569, -112.78583642012705, -108.7093037763389, -110.67868795924797, -109.0190959349128, -108.36247198231372, -109.82829353258869, -108.24916379311045, -109.84154533905823, -108.55470160833775, -109.75438989348815, -108.82865632118325, -107.63622268162582, -111.00943492886312, -110.81824358463759, -109.46028423652966, -107.52479398900992, -108.99087806823736, -109.94494831750349, -110.26788355564504, -109.8954055022304, -106.9478122391182, -108.91705388158901, -107.76095584490312, -109.28456723055147, -109.7982307261767, -108.98552661346622, -109.98937979783426, -110.57907422426224, -108.68113463944836, -108.06257240208589, -110.0707224529617, -109.19515280354733, -109.35868842818849, -110.37311467065695, -109.0404734478992, -108.16686395270187, -108.61859220485148, -109.19986437876149, -108.19707189725302, -110.06564239663074, -108.87850403465154, -110.63824157544798, -107.36918104067212, -108.7008736325543, -110.9359398265406, -111.08529123080929, -108.44209934821818, -109.79529621208783, -108.38917887958179, -108.169117639508, -109.24332926356216, -110.50584058811704, -109.63592524002665, -109.32261039377495, -109.16720880524552, -109.3084314664462, -109.5812223978583, -107.70213196487856, -108.0557884982431, -110.67058020007828, -111.68459781023608, -109.66270627185824, -110.52536245663693, -109.70208409132103, -108.78645420809342, -109.23122088059863, -109.24601474121832, -111.25604763816514, -109.50225851581177, -107.32434217163818, -109.28548556764925, -107.59972621660836, -110.46928774723048, -109.25950101547609, -110.32016453935465, -107.78482761561703, -107.89462895091089, -107.51366154391481, -108.08036891159172, -109.53371809947035, -101.2452927166745, -109.32763325689056, -107.52166868423687, -109.89648659445174, -109.11350200980485, -109.81336712738089, -110.02799517445062, -108.02767143538516, -107.97850220501483, -109.50772934896838, -109.31069875721964, -108.49991657749598, -105.60880911233095, -109.79128597340213, -106.91084537903113, -107.84880087118997, -109.63628170511824, -109.03203967193224, -110.64186113413658, -110.98027990365594, -112.33841002907062, -111.01793075565425, -108.58025797022215, -110.4259296883756, -110.38643255981424, -108.93051671115133, -110.97544177116494, -108.63883100482677, -108.37581711765226, -108.90240163126536, -107.94688047875466, -109.9482937437732, -110.09097112364414, -110.09805032265376, -111.44307114024532, -109.15483789122554, -110.9713708217832, -107.8548737634672, -111.41418477109195, -109.45699779859628, -97.03595099331734, -109.16746744169623, -109.66209204485918, -112.57048704774604, -109.73989735035725, -108.16252575067017, -110.7546980664636, -108.91536673403449, -109.20509151422344, -111.0260632167785, -109.62924582406518, -110.45466277291722, -110.2973970018937, -109.67550222925419, -108.84481022020094, -107.23686414357573, -111.79004633370906, -109.85453094194085, -109.45617270081004, -110.73920606732504, -108.90879956851099, -109.67774425528265, -109.4745715721361, -110.18080454693559, -109.26079184315502, -109.41692499885505, -109.02240975088358, -107.80833423058168, -109.32657361431549, -107.87138278655101, -110.910364670719, -109.70067156846706, -108.55301754282077, -109.4243252157005, -109.77567725161107, -107.83737232063925, -110.36509412773016, -109.6371048811367, -109.49430894422814, -108.55509251499753, -108.03996302911446, -110.4385715838736, -110.08864436068788, -109.48922484379962, -109.90865554258562, -109.7491963238264, -110.04796094537969, -107.413043439116, -108.54229076126079, -108.2522516728666, -109.75464941327974, -110.26795832300996, -109.28073673851144, -108.62990200974927, -109.89408067552287, -109.09160284731726, -109.90740624925795, -109.92534708896517, -109.79578862362752, -109.97278346890566, -107.80679350393824, -112.81728446281548, -108.09689504419987, -109.89549991422173, -108.43930976031248, -109.95153099843282, -108.18277483720716, -111.89607792605433, -109.52567003805, -109.17125106979698, -109.64300739407085, -108.21045178846524, -109.64036472149706, -109.02324448538845, -109.039163008889, -110.41006510134076, -109.50289952116489, -110.4732620447796, -110.08777181504614, -110.15589511434341, -109.55705089158471, -109.2547682932589, -110.86823885471617, -109.96330502176939, -109.85995369810554, -110.63211290903473, -112.08007783432191, -110.24725218052279, -107.62861148917592, -110.08691795849435, -108.89793794632287, -111.07702220466341, -109.46946126482341, -109.19747345337464, -110.70018609416007, -109.66366205691908, -110.78032312133551, -108.05724200456513, -108.195661625627, -110.90724508408255, -110.08307674771669, -110.76863516643007, -110.46620425061583, -109.16986788877276, -109.61921294239114, -108.51159432329543, -109.96308336765689, -107.38178944242856, -111.95930944846394, -109.3329826827624, -109.59119636368249, -108.83148571828912, -110.46194288788257, -105.87694286145472, -107.985886302892, -109.2975019660806, -111.05138725716857, -109.60005889204612, -110.92871351729086, -110.73480546964537, -108.41587420326718, -109.84275465824477, -108.8249071047676, -107.65358887817105, -108.3254150042995, -111.47362100321767, -112.7287536850025, -108.8217125660507, -109.50232320231771, -110.29587061625348, -109.30644535112089, -107.69178032077258, -110.84522325672016, -109.3735891463141, -109.12506388923123, -109.65582307934665, -111.11427272192576, -112.19827973435466, -109.11306367925813, -108.19203577968261, -107.89831568266465, -108.85805249169313, -109.51100049661844, -111.71546684086955, -109.53880495724334, -107.07739286222231, -110.66836728754211, -111.5415170557177, -110.16051267940297, -110.6107546662698, -111.36389129556191, -107.77888179117923, -110.34160392509817, -109.61287125994414, -110.23791773883013, -111.00669159903549, -110.97165069538953, -109.43965413392434, -110.6813161690388, -110.31441293654314, -111.96129906273796, -108.15998218707462, -110.08095912053633, -109.41084567452768, -109.28774416263552, -110.80159950384204, -110.41956747809755, -108.85005186267244, -107.9069227847757, -108.84249369063123, -109.92569208845894, -109.34109797584448, -109.41334788055491, -108.76462023086997, -108.22069272136177, -107.0786679601274, -108.30206755098202, -108.57613406368954, -110.83330887636482, -111.93966942736989, -109.76373713473264, -108.25782074884941, -108.16490627215555, -109.93351470267982, -110.75525684428368, -108.22814762283093, -109.73442331991602, -107.53145627482685, -108.27195221226805, -110.33032779278457, -109.48951857415828, -108.12599093700939, -107.97627415508097, -108.81426859968796, -111.21764717894752, -109.80856212352333, -110.92658779118501, -109.71551885834796, -110.38682741010847, -108.87671328341361, -109.68368600774755, -108.35359806351899, -111.7519400010676, -109.89407081573103, -108.24301180922755, -110.00646944788126, -108.6685299083706, -107.52856885980722, -111.7622363038509, -111.0025144494897, -108.64719599357296, -110.62968467177518, -108.821509935539, -107.94915453463719, -111.53070432277694, -109.87282048586256, -110.71167589371663, -109.79225006081626, -109.96203471712074, -110.29921092232489, -110.10644439440416, -111.28815007382043, -111.19165661703703, -108.46024117100558, -110.22528296512183, -110.32184972386672, -110.05120383416072, -109.78792549362107, -109.00355659956696, -108.85989369286315, -113.00899556732638, -110.91756826567867, -111.25016866167897, -111.84225040552181, -110.54451635944174, -110.72722829912917, -109.60759702177283, -110.49362602516815, -108.74419542915284, -110.3379671069179, -109.66259088220754, -110.45956400953156, -109.13956157147233, -109.27130155486806, -110.83015602667983, -109.17970724944131, -109.09662765889193, -108.0447366108107, -108.9536269357457, -110.35663108940085, -108.73418835472056, -113.42965806805827, -111.81270536656905, -110.06155590173537, -108.76582224646269, -106.7488061675813, -108.5700320158723, -111.11038264410035, -110.41435767488723, -109.12763443489911, -109.30517580756394, -111.61251165371237, -109.8116632664339, -109.36845864976851, -109.00390009629231, -110.54359197165573, -109.52629258465976, -110.75932197632896, -109.50903215359567, -107.42652056246085, -107.81146496533543, -103.22224383145215, -108.53803076819163, -109.78623360072066, -109.66306634612869, -110.80245829141279, -111.87835085452016, -102.27372781471168, -111.27763038431458, -108.45838423437681, -108.79077917058028, -109.31951755762685, -110.05415097017186, -109.5535934823387, -111.62732254641111, -110.73478247119641, -109.9468722686683, -110.39698367573979, -109.30612942398305, -109.7578384694043, -109.34817295524313, -105.56944757301993, -110.1940418750125, -109.27076023513962, -111.03491935225027, -112.2980497521063, -110.65725497955563, -109.0567530102422, -110.31700596563523, -109.64508026365678, -109.6190471404421, -110.52566833759428, -109.68595899227789, -109.7431160985074, -110.4798230300751, -109.45506977604765, -110.69504157940786, -110.63067849573177, -108.06456949500138, -107.99354148885966, -108.11349194720599, -109.15944121207349, -110.61766925164031, -110.14145801314527, -110.67420842201165, -111.91532881806512, -112.15901550030345, -109.94774413630104, -109.2819568305201, -110.94623189179737, -110.17685430287735, -110.39082916961016, -109.53953238698966, -110.76940623620611, -109.89327922318515, -109.10275695043765, -110.21445972656734, -110.58968777252528, -110.57016757660259, -109.59208496373341, -109.07946946465374, -109.10762003745964, -110.36892993974607, -109.81864495218393, -112.12972189864566, -109.26185849434863, -111.56305819991357, -111.36019621828058, -110.3397604159226, -109.58675612753163, -110.58041217474447, -106.34739062044932, -108.6722699609389, -110.03906060709869, -109.16794717548382, -109.65012481802809, -109.35377624077988, -110.51889143862303, -110.03397458059777, -110.7981307056636, -110.56653507062292, -107.61367005067231, -109.99279736988825, -111.79875182878175, -108.60382315996031, -109.71381533228038, -108.60388131505613, -107.0933685540362, -107.86037690830757, -108.40980028847238, -108.83869602763895, -110.76921375395764, -109.96766364716046, -110.8256171465781, -110.13805084291067, -108.5349140035878, -110.57158437465219, -110.8920694413417, -108.71646695477324, -108.33274238445665, -108.96152108305608, -111.03750932994224, -109.48915027983756, -110.29725207211165, -110.79527247268442, -109.47969936716117, -109.79306701834035, -110.16840035577498, -110.29840230783668, -109.15306387075587, -110.72651274964761, -109.08881658764956, -110.8349724030761, -110.64653625576447, -111.40392562616867, -109.94581588927414, -108.85136340231294, -109.77228546607624, -111.48297395390018, -109.7334001251941, -109.30537415590783, -109.63937411233408, -109.69785848648013, -109.3523781030017, -112.04667421182404, -111.56311816195343, -108.18548447362308, -110.63388993686104, -111.39768634137992, -109.87157345395542, -108.6734208287271, -109.46213300216168, -111.75774769437145, -110.10245994173216, -109.52385139033495, -110.96513097775451, -111.8709319163154, -111.54948269614047, -110.29760900080463, -108.52168175904663, -111.09033925738258, -111.14752744054172, -108.83074523709202, -109.05704141259113, -111.74377805749482, -109.57200906899736, -108.84121318623825, -110.86657990204343, -109.54363603755047, -110.89448416316372, -109.58965570570145, -110.21012263847972, -110.4063470702923, -109.5021950342969, -110.33648801598177, -110.90551031296536, -109.69205870504638, -109.8648503154861, -110.28183391384131, -109.65970942950766, -108.43615680946908, -111.11790511866548, -110.89043476451553, -113.64898442872548, -113.08004494963895, -110.81525412051718, -113.91009875719509, -110.95802128672312, -110.40944585634135, -110.33464695414992, -109.98984645778987, -110.18795067005652, -110.62364351231234, -110.44029833291248, -109.01598585569788, -110.95430216511514, -109.77987141110621, -108.54452361812068, -111.41780266439777, -110.47172771858405, -109.06084635984516, -109.30794593246578, -108.8764083815745, -108.18222749506985, -110.31330487887435, -109.04176821738014, -108.8558386035048, -109.47888284507395, -110.01459604573937, -110.48596659065309, -112.6781342298378, -109.85522803775775, -109.0569534499285, -109.08991286548698, -110.89485727880403, -109.18715778948663, -111.50381433568144, -111.3545424730884, -110.07710926239977, -111.99977850157067, -109.47444853853723, -109.81605328527645, -110.74995213151195, -112.56834665925544, -108.52052472391404, -110.89121213995557, -112.02004142355113, -108.66413739656008, -111.10053848695652, -110.41241079991636, -111.80152991764473, -110.21746151515111, -110.63265128607344, -109.483042128511, -112.78639954059729, -109.47114195846122, -109.23309637902875, -108.97133643967169, -110.08909147812822, -111.01105271457081, -111.18602432128249, -110.04633990216801, -109.53453538673071, -108.81939452082017, -111.13486114285661, -111.65877073200598, -111.63763706753498, -112.14107810664572, -113.6231865196724, -109.31743865878806, -109.18551713085722, -108.74951309653638, -109.28206426212142, -112.36687029711229, -110.10933061193728, -111.29501093502684, -108.19021080564794, -109.34497312126749, -110.37228033937312, -108.63277512903049, -110.61033993911002, -111.2975761598062, -111.49780004751436, -109.91019436685814, -109.32789992989028, -111.4482538110117, -110.1538439123475, -110.66347034043578, -110.05055133068794, -108.53002033538341, -111.7522199783972, -113.49108651193104, -108.03793940563418, -110.07108694011555, -110.83958739865201, -109.62805629409038, -112.69637731014087, -109.57996950503268, -110.104850643722, -108.83376203949506, -108.69400304840181, -110.59434352922563, -110.69121011800921, -110.18694553784364, -111.90598571547098, -110.30230802494223, -109.66810649416752, -112.6017099000434, -111.00296745333219, -110.64462650261785, -111.4775358707403, -111.98753241268494, -112.26574909791167, -112.04796822399412, -110.65853064447325, -109.6623218025264, -109.40559579075378, -110.42174451813142, -109.18991987957241, -111.02050178263048, -112.77950487440032, -110.42443751566815, -111.35440372400903, -108.5263524245987, -105.07498063939795, -107.15444425741984, -110.4508720018025, -110.25163264819463, -111.1383261104107, -109.91171620173931, -110.52200560606038, -110.5299174299573, -109.34628087255733, -110.26101817411786, -109.65071853372183, -109.66953335961068, -110.83590602054682, -110.980546313788, -109.4110066989163, -111.47223607390256, -110.00281523859483, -109.4088722967626, -109.00401922839337, -109.59655302543185, -109.7359970854586, -111.46016206343049, -110.23478747568004, -109.29441275295858, -109.82941912510167, -110.43088525283673, -108.21649744751299, -108.70220592702613, -105.2334473604296, -110.60620657984927, -107.97533820921146, -110.7664079806058, -110.56406610911355, -111.76465470250328, -108.84172809688911, -111.03661078143631, -109.85351980370237, -110.70091167176791, -109.52380717508088, -108.4356492672842, -112.25498760397127, -110.69648730540193, -110.36748838594507, -109.99090797924349, -111.2678642544111, -110.42541694325627, -111.4575545259775, -109.3211175669008, -112.7465573314208, -109.56208667784249, -111.59733497772172, -109.42295730962105, -108.55804089331346, -108.71397903286748, -110.09188290952392, -108.90810063278326, -110.31333217069538, -109.69794714542728, -109.06210020835357, -112.42465112160288, -111.74630553904855, -109.99304310093493, -108.93867687355595, -113.1669287525049, -109.09193568851137, -109.27500368450697, -108.99643325722404, -110.53962759110647, -111.2052088429852, -110.05855563908841, -110.30763723153481, -110.03411001268613, -109.6161415052669, -110.6304714466923, -110.17116005754627, -109.0753171640551, -110.92564270851628, -109.60831770517053, -110.25913363817017, -107.76644895378317, -109.2619309023068, -107.64198246311884, -107.37056168314048, -107.31978563121643, -107.68171928702894, -104.57515288104209, -104.75187637758803, -105.27246893266054, -106.96524396060869, -105.93920355631757, -103.66449995825586, -104.08476660009461, -104.53081578265315, -103.0148493379086, -106.74751670818362, -104.92309629919443, -103.98320340724693, -104.81633219413234, -105.77996356028235, -107.12559309216644, -107.28196039053535, -108.84583578337953, -109.4494696919565, -109.15525441177898, -109.7634811359225, -110.79433338587495, -108.44440079452527, -108.79597700117748, -109.98590735173822, -110.72144284267539, -109.30550753718086, -109.70072152916897, -109.65801130162137, -109.65949265997646, -109.82238573025273, -110.30669821947491, -109.83394128869384, -108.90433312205332, -110.664046708231, -110.39926453734134, -110.37725911098757, -112.12508639032839, -110.26795666332589, -108.98741993218054, -107.76168841100478, -109.82334992872889, -110.83516363498563, -112.60649745671253, -111.1960726449926, -111.03919163866381, -112.05129034965563, -108.83187987662883, -109.57240688505179, -109.32857861150738, -109.54934849013647, -108.29359879300195, -111.5179112931669, -109.52702486426027, -109.95429980789645, -110.7011078611564, -109.43204524997455, -105.56031249677113, -107.70609254346495, -108.78303653454363, -108.11457060956113, -110.44215460317537, -110.78267897406572, -110.33119812901934, -109.34449539666907, -108.82636558484161, -107.1834151347969, -108.83808254322192, -108.2542825327446, -108.80298057862501, -107.59922121598055, -108.9131916496929, -109.51519107961856, -107.7704986323755, -108.79678029009878, -111.13791068210752, -110.402746275919, -111.31702623823912, -108.49812727557243, -110.63723264798182, -109.32890666586829, -110.29721723278237, -111.66560929315017, -111.04227698307153, -111.36927505376269, -112.5203298417673, -109.93967930487354, -110.14533835678606, -110.3868348991775, -110.85413569165249, -108.44519725537315, -107.93391978795047, -109.82778679299085, -109.79311153223738, -109.25261055399044, -111.47738679135526, -111.11775495397512, -108.65898844492045, -110.26505495390529, -111.02017977446526, -110.34817965403467, -107.55161094495372, -110.21667403085983, -112.43970497917284, -110.70535338255132, -110.79438078890512, -109.81809822502822, -108.99167960596515, -106.5556893069368, -97.51736665041192, -105.29926513345109, -108.72453297392224, -108.23203912463346, -109.50324111400698, -110.9939986929772, -108.05367524487318, -108.37339392211176, -109.8553291283933, -110.46179639493138, -112.48795697163695, -111.88145079973545, -110.8678969738583, -110.62677605624849, -111.83824818603244, -109.76798658735359, -109.6654742351465, -112.58543522753767, -110.3406716250781, -109.55013159400883, -108.00481229232405, -109.90793236599207, -111.28597960985334, -110.54144527494444, -110.14704702870655, -111.2652554338908, -110.97520848958668, -108.63647576273343, -110.52472680617548, -113.16137826273847, -109.62457037485827, -109.53869420402964, -110.71399284283449, -108.55435337782664, -108.09492728294455, -112.2373886856363, -110.3693019226993, -111.65116752865308, -111.3223986412311, -109.67734725401074, -111.36420709226297, -109.14293108556625, -110.5982939020188, -110.29596476096043, -112.69847120697035, -108.39052787054206, -109.06205229490357, -110.00045399262885, -110.71775009467346, -110.69530760167493, -112.54144940754935, -109.55755373438097, -107.88943697845929, -109.98578587243783, -110.14202980613851, -110.80051915904802, -109.11327182471621, -109.50637030500913, -109.77023677605327, -109.98552825925917, -110.40235854896, -109.37603004890141, -111.36989177909379, -110.8399811877331, -109.30394670937987, -112.2769814990538, -109.10893172594731, -109.17733972841754, -108.35968166480572, -112.64492569586005, -110.13779257328873, -110.64439690778532, -108.45446935516622, -108.97325006911116, -110.54637968933774, -110.66412364132371, -111.38627695224784, -109.8942998516069, -110.36392017322382, -109.92355133054227, -109.61886697310419, -109.71969465343778, -109.85627196259388, -112.1407808286419, -111.1013489416651, -110.70428953307596, -109.3454280179969, -110.22984684615578, -109.53826801613613, -107.83673208330934, -108.72742563398342, -109.5745872123195, -108.83031823548816, -110.89059911076627, -109.87842545384129, -109.21980161063786, -109.07140273870678, -109.04628915564135, -108.79255665097845, -105.20875397856382, -110.0838008881032, -109.68293832806683, -111.24644641302518, -110.01257579497496, -110.99281477454484, -108.99296184719546, -110.96495665514604, -110.70404386182749, -108.25078498739035, -100.77667501455139, -107.61479263900088, -110.06600976399395, -110.02035637581871, -111.45524052052504, -109.975541184397, -111.07333860975358, -108.4808974233161, -109.59513524582242, -110.74711589861774, -109.50005300854993, -105.23071652566294, -111.81094849223531, -109.0168079712372, -111.89029991620679, -109.90672274216391, -109.30959446424889, -108.23718655264584, -110.10868108588909, -109.21139771899594, -110.33333323577992, -110.25792318324204, -110.67825932924109, -112.33148517950511, -108.9724848367048, -110.78371843797613, -111.40913868573313, -110.2930522718577, -111.9538408094371, -108.63639312641844, -112.4462941079034, -110.40266356498321, -108.66617580940074, -109.44306834729083, -111.08962916641603, -110.52132608161017, -110.53757698855654, -111.5587344449704, -109.77722315102946, -110.40060629757771, -109.45395807961631, -108.77558572395142, -109.0151938598724, -109.80739619986889, -108.9332873172888, -112.49933978358132, -111.28667321897437, -110.40629082858706, -109.9829216820938, -108.85102919990373, -110.84179127037925, -110.27309817549309, -109.88857884367955, -112.24517967927224, -110.23377125710859, -111.26951227953063, -110.09782138347559, -109.77508406986834, -110.55359722398646, -110.09534729906368, -109.96333904888587, -110.29372855476366, -111.36651812163072, -109.97141184588116, -110.16701683369045, -112.8562627359291, -110.66651146857079, -108.78873821095968, -108.59208174618087, -110.31784275318834, -109.43177042415276, -112.80272887161644, -111.79874205007107, -111.08216899537892, -110.73699224045636, -111.04738767291953, -110.43395896705012, -111.62106163510778, -111.32599933330843, -110.29360981749807, -109.66562228449096, -109.21316193790335, -110.06363162177448, -110.54480468587292, -109.31791670875509, -112.65386492377107, -109.91857609999171, -110.57233605624137, -110.7597333064856, -111.49767138733276, -109.36548654843229, -112.34145274183716, -110.52831153822652, -111.55802243871352, -111.81399803046556, -110.17680125962372, -111.23811621944807, -110.48042049674514, -112.43786993562033, -109.56507357271987, -110.67030752598993, -110.86377249100713, -109.06001892813467, -111.37023727930494, -109.52881096984436, -112.95107295160436, -110.49467818026214, -109.29804210589607, -109.89270706931751, -109.46354468058833, -112.10350702955014, -111.06083529077077, -110.49996587015904, -111.1617248913634, -108.84725633199014, -111.42852695852422, -110.01433866707184, -109.11616968390972, -110.76961079765468, -111.80403513904453, -109.84442686379181, -109.65447921666167, -111.3378640555306, -110.8882647652338, -112.58014202075226, -109.67128881545659, -111.73429980763389, -110.82258070774773, -110.71895931098041, -112.5117489008152, -109.16182299471309, -109.71651258790612, -109.7770618808562, -111.94294809571427, -111.1629115541574, -109.57489224865171, -109.8402445779754, -111.17931450307283, -110.09045865447595, -109.23658206733491, -112.54929616847242, -110.5150381158864, -111.32296447909377, -111.64472156295191, -111.65832771066007, -111.03359562742956, -110.85303206770837, -110.80655337650862, -109.3712696310075, -110.57313454785879, -111.18525355670417, -111.67423695430561, -112.00829831274282, -111.08915434609605, -110.3298290221436, -108.68552957386795, -112.11377370993225, -110.80288297661977, -110.33640536217185, -109.5907971201988, -107.9195263775506, -108.50223113159429, -111.91191347156142, -110.29585599512956, -109.50902788911351, -110.76819145749467, -108.86899533416589, -112.09963049260891, -110.13374376572433, -110.15881393584463, -110.87392107947531, -109.18658540731009, -109.72734703956934, -110.18732487568724, -108.76554115185057, -109.94122289815374, -110.39583285609643, -111.09540935727229, -110.6618176357367, -111.6281345666718, -109.69686483639367, -110.31633402076315, -110.61246951748903, -111.73300235294965, -111.34221378834899, -109.46708370903485, -110.70412671997354, -110.7007891485379, -110.31685483435038, -111.03016917417074, -110.94517365625376, -109.46580797053619, -111.20935248224806, -109.20661126636224, -109.50147037097533, -110.14241781654353, -109.8510950344643, -111.3794198224028, -111.28966889207122, -110.43347441663424, -109.86759980279523, -111.92101892013198, -109.31594011390644, -112.92253433794441, -110.74000829597605, -110.3690783911604, -111.9386136764295, -111.04196305034188, -110.41800427558245, -110.94287511448232, -111.66035388807579, -107.53723747644062, -110.68014818358719, -111.86628806511304, -110.12097497430523, -109.69880468221378, -111.4312783987915, -109.18240866486639, -111.45649839248873, -110.1242345454651, -113.75911576151633, -112.71747598882953, -110.9614554157337, -110.92294419716129, -110.87229098694876, -111.09943759113875, -109.48107247947176, -108.62783006742795, -110.8108025857779, -111.63342408317932, -112.0221522906341, -109.96411229549527, -111.29821085030613, -110.04566676239914, -108.41674583097112, -107.50256474992416, -108.68086611003493, -110.3738906060137, -108.86763212826641, -109.81681043446049, -111.04539822346567, -111.73290882980949, -109.75238769150758, -110.55268275367449, -110.48423701377924, -112.1116140908134, -109.53952175199518, -108.538611608547, -111.3788321484912, -110.36378736224961, -110.37712171023523, -109.82150687920334, -109.17046632238393, -105.1169578108227, -110.84067642540583, -112.91626789016587, -111.32030958133453, -108.93375913686056, -112.44450956563915, -111.1596840012794, -110.17380444915341, -109.634859036508, -110.68819277718731, -110.0648098825346, -108.87385575091399, -111.99676414571755, -111.32585405719519, -110.59892045991457, -110.32589048340424, -111.1172696292077, -109.79946399891651, -110.10030723919304, -110.71841081343656, -112.23013150012054, -108.94400401141407, -109.71044551701596, -111.77560214164039, -109.68779520039777, -110.96119601299907, -113.66477058855787, -110.17794649102234, -110.30159876509862, -110.11953836266514]}, ...(2 in all)]
  out "FFT 2":cluster{"f0":dbl, "df":dbl, "magnitude":dbl[]}[](graph)=[{"f0"=0.0, "df"=16.666666666666668, "magnitude"=[-324.19011195451765, -78.1272953812706, -85.85545438627958, -89.30587144190069, -92.90590394398903, -93.63083388385274, -91.8644929119412, -95.26924857401164, -97.0710469181336, -98.01148078956652, -99.33043660296804, -95.58776817681839, -99.9570097527269, -101.45494093095093, -101.51838334751548, -101.00386616525799, -103.01963069818913, -103.20223925731209, -103.53783076500916, -103.48065647812659, -103.97797518531912, -104.58942778240602, -104.46991277190502, -104.59813972158683, -104.56685024229951, -104.69893799348945, -105.05669000016238, -106.17061117835001, -106.43303821862656, -107.39468286383597, -106.2899368267905, -105.7863846168199, -105.17170638885071, -104.53818172761852, -106.70340956723133, -106.55444321137247, -106.67654843051936, -107.79888413750199, -107.86424326005849, -106.09722609215336, -107.71648639013972, -107.79500725395155, -106.17330953637067, -105.43663624517525, -108.04970689199158, -109.92106271611999, -106.2505251183406, -110.60221373795562, -107.11377887451098, -108.4126937286195, -108.37794745021417, -113.22457316369011, -106.38281814065472, -107.55385617652075, -108.93026538982782, -106.19334142366085, -108.90462602264525, -107.63084712174981, -109.12192537022624, -107.90627042480016, -109.44472079190832, -108.91731458372392, -105.74102972706788, -105.74407510394178, -107.5989477192235, -106.2838630137392, -107.46190542725505, -107.38881299750702, -109.08024783239452, -104.97871836903269, -106.65424712290651, -107.04966019632134, -106.16202578092883, -102.98374199247179, -99.1568704142098, -87.07383781389657, -96.41471411313154, -102.65176579899618, -107.65674867775193, -102.85397890306213, -107.58658613411464, -104.79044898833125, -106.65282019869865, -108.65027966345534, -109.46169054950127, -108.69969979291741, -110.4048706652988, -108.81020193837274, -109.42808902484134, -108.85398463561398, -108.3849716744813, -109.1844457168716, -109.32787859535676, -111.01992124870878, -106.64843449415699, -108.9926343573667, -111.59837822080355, -110.57121677672183, -111.17280164669164, -110.68901970586144, -111.69013245592781, -109.90200577018311, -109.3554172126163, -110.7515368822992, -109.2863324212524, -109.66209701262974, -108.50795548698007, -110.58126481096504, -112.36093896766921, -109.78612141282203, -108.85120530917233, -109.91424431080952, -109.84698632196245, -110.93960894966105, -109.77214706089354, -110.30762971422381, -108.77791302937449, -110.79522659679036, -108.47242514643455, -111.20629758187835, -109.05996769621125, -111.13574821570619, -107.79388178889101, -111.5768481279296, -110.52058839597171, -111.58729762739313, -108.99000864386126, -111.6585121505227, -110.50715371958135, -108.87151956974363, -110.30486244367107, -108.32392040018144, -108.1769507919999, -110.43198471512189, -109.81454097966842, -110.26717009815644, -110.82924135076777, -110.34103661156989, -110.0692667126265, -109.34555682020833, -109.1694484721415, -109.9940980324044, -110.81940616215803, -108.21162003366862, -107.97087538330561, -107.55312461506225, -110.60339321606872, -110.09004629292225, -109.05860430198882, -113.1412749514818, -109.81628200948371, -108.62343219429849, -109.48172424209761, -110.85978755785311, -109.47778611557064, -108.81728552967951, -107.47864241666747, -107.61735128422292, -109.62511618983821, -110.32417726356636, -108.24287897478176, -108.60460879530194, -110.2181558494026, -107.95550802888957, -110.80234484950323, -111.09955733353904, -109.43923052503506, -108.98949130235951, -110.05778199870154, -110.36224432927585, -108.13523430027999, -110.681114579241, -110.49106131529867, -108.73493328004297, -110.07663907252234, -109.9968931372618, -112.10715231091008, -108.80994125105168, -111.63774865669372, -111.54355694032755, -111.64024217585788, -109.34986300492378, -108.88053713185408, -111.14370830146245, -111.17327416167232, -110.36311492990576, -109.99414559884396, -112.96912007380595, -111.43191437097785, -111.71327312809349, -108.77202323682606, -110.25970374932486, -112.59574277180732, -109.77247894866957, -110.09219852365874, -111.7197662726775, -109.85454092697009, -110.06789440397942, -110.38055758638309, -111.04251386932805, -111.54279434240568, -109.74385329575985, -110.98924544863415, -111.17898077762852, -110.98364252730245, -110.75024385843372, -109.24766708578407, -109.67753987004863, -110.6537235844391, -111.84436313010086, -109.12654337292446, -109.65519521121124, -111.1845162935778, -110.5009101465602, -110.22980642268818, -110.88540043278346, -110.29249073109453, -108.80459864528464, -107.49372141121728, -108.50353962704821, -110.00730069533373, -112.012876492648, -109.01283702976382, -109.07442203290057, -108.2961442983685, -111.60962842680907, -108.84312815413224, -108.6276642979969, -108.75132871638827, -109.30004903844721, -107.20359872252604, -109.12175943862074, -110.43914247337625, -109.55954680842791, -110.37116786618797, -108.55907813251434, -110.19249995041955, -106.95269845697632, -111.07027929458712, -110.1073996792702, -110.61729280468039, -109.6419175310234, -109.47995019876329, -109.66602827275211, -110.01953864498805, -108.45989120418268, -109.79778555296474, -109.94663827736616, -109.52410616839379, -110.58014441463794, -110.09182359045897, -111.0487262011397, -110.49609187214915, -110.6114701312941, -111.17752423063314, -109.74965389041003, -108.58973724447526, -108.84292130035902, -108.90689510645983, -110.69840140049361, -111.30494362640982, -111.00224390075273, -110.50848328538423, -111.59232911931113, -109.30826761863756, -108.44510893127558, -109.63744704504391, -108.95037574307332, -111.36486409910674, -112.74508631930381, -111.03952454593811, -110.57133212903979, -110.59969855145111, -108.25570461975128, -110.44617635200193, -110.32190307214704, -110.95204704643322, -112.0595421753479, -110.45342552693265, -112.50183987758867, -110.08217804938009, -108.90353583389084, -107.02032313792242, -88.3334978919524, -107.92027625495886, -109.83148570028482, -110.30427997450572, -110.92855407802753, -109.67404674397338, -111.03606345823586, -110.58277018943096, -109.77692362669393, -109.39170901729935, -110.20711662408928, -109.41601946806779, -110.34213214925832, -111.2283900972803, -111.51682597931386, -110.47069117801351, -110.93808974285523, -111.11277478000933, -112.50698886748012, -112.12918507523611, -110.46316790252011, -109.9387334819968, -109.78723249688426, -107.13037722044297, -108.16132376075751, -109.07255491017162, -108.85068428558272, -110.28038153100799, -107.77611023481016, -110.69754506886444, -110.09495581837979, -109.21214884561816, -112.62718526248648, -109.22048725312992, -109.17793923163308, -110.87372121410577, -109.71902632604333, -112.61041177225496, -109.6374750969677, -110.74738952366951, -108.93404661877067, -109.84938675700889, -112.25316361679832, -110.30788094875312, -109.26929069321925, -111.20853536783942, -110.05212566057608, -111.72448131932816, -111.55474439772887, -111.81988954424324, -108.44452452934028, -109.21897824914645, -109.55634869894358, -111.36318572800242, -110.05777399011298, -109.64458567712875, -108.73315084760529, -108.93332091319675, -108.4816455312154, -108.80120578498936, -108.1804470361839, -109.7177707524778, -109.31977709844544, -109.33603116022124, -111.46120546572519, -111.7480378245176, -109.17907150677627, -110.47970652472505, -109.73718750984082, -109.7935026884937, -110.40458408612054, -110.91781389491092, -108.39352075861481, -108.27512197925346, -109.59155075404814, -110.40183121737397, -109.25423373270381, -108.37769008625712, -107.91335995938509, -109.5576520703013, -107.27392145737491, -110.98592762117059, -108.41809950647861, -111.48163889400448, -109.70961684769624, -109.22952568656495, -109.76504719131209, -108.86928627177666, -107.97855299877004, -109.8412204399902, -109.6690048999326, -112.28329030175193, -111.54977099314607, -109.55689540119126, -107.93716711232997, -109.84247640855929, -111.5098351445789, -109.14317615215809, -110.28319116384824, -110.57901069942578, -107.2890252845352, -109.66754569546274, -110.15708115946433, -108.83782190109405, -111.60783857760667, -111.46884385151185, -109.21985333366634, -109.63605494317056, -110.87999187262697, -112.26992029775087, -111.05491095860552, -109.22795442529183, -108.99135781712076, -110.46475190704264, -109.35746113713218, -109.29125989270668, -107.40922407684049, -109.24391685563656, -110.41554602144217, -110.68952735085914, -110.62457364102458, -110.39856310555466, -108.84256124354566, -110.01614601335088, -109.8071306678428, -110.2804500736802, -108.76205061238203, -110.3962440297242, -108.98253716257014, -109.32990745926702, -111.17276766165281, -110.41113652364085, -110.36616199963426, -112.09767002991742, -108.43599666470733, -110.91876588140981, -109.05329272502944, -107.07198690769708, -108.72934463903034, -108.6666471996132, -108.97529973794413, -109.68895260146817, -109.2658844652487, -109.75690097249196, -109.38585024123027, -110.17593039468063, -107.87223111061134, -108.15261097418302, -110.09277437980633, -110.8665497655964, -108.43061614348413, -110.3052458526819, -109.22446919161898, -110.51909692711594, -110.06620699121913, -109.53439413051383, -110.31952463872884, -111.4732125902982, -110.41443606663168, -109.9579358088152, -109.930778061577, -108.5473214465574, -109.34719220288939, -109.16964653934396, -110.04824158176345, -109.42616539603762, -108.3556027482992, -110.62331917617789, -111.3652147859356, -110.12362012120938, -110.13175448595814, -111.20110099151856, -111.50643914621541, -108.11659117128028, -111.06037600347967, -109.03822892917451, -108.25678204604324, -110.82608024151122, -109.15887945314851, -109.88255674562845, -111.18322672526185, -110.95836040044516, -107.91535345885436, -110.66285812468733, -109.61906549925033, -109.58059721670746, -109.65198009505977, -109.65950565672951, -108.95264505276342, -109.23343669003113, -110.74308548011575, -106.39170014998685, -109.61471203101753, -108.24258770956924, -109.84609566640096, -107.83834185503922, -108.93052854090027, -107.55568820082641, -109.758551082242, -110.65892780872205, -111.99907420485852, -110.71043004141137, -110.62257237494617, -109.15610413532767, -106.87403836327807, -108.19175324576331, -110.27819583792918, -110.23918003777561, -108.29703377268754, -110.07182881114713, -109.60256111108491, -111.00394752430006, -110.30750337485472, -108.78309624082331, -109.24103013025798, -108.76979253891403, -109.91618737478264, -108.83915940855513, -110.92536150834754, -109.72250903746432, -108.96533939688658, -111.08949280651164, -109.20335070860871, -109.37826578362439, -109.77953166722301, -110.1867310744785, -110.07114559821346, -110.7003631567182, -107.86455899696074, -108.94113264174617, -109.35999427135138, -109.33627364788704, -108.96588828808375, -109.08716536982254, -108.73575375369026, -109.47770132070654, -109.83726171472907, -110.73516506891792, -110.56827134787686, -107.65667508354096, -109.30200115708924, -109.28406803847896, -110.55374624323233, -111.2017766725333, -108.50851279608973, -109.79494403619485, -109.08320018013063, -110.21850624918747, -108.4652936555984, -108.74837610538873, -108.81326140648238, -108.83830180036702, -108.785270477003, -110.01845876259073, -108.76030368637825, -108.57879884880157, -110.6610608456059, -108.74669367794318, -111.55956030460833, -110.22906685783455, -110.48411613865359, -109.48060880085136, -112.77556331479562, -108.2676071206087, -108.8571136162698, -108.56944905160177, -109.16406757131058, -111.42259299295839, -108.25216316582294, -110.48487127684025, -109.69532331373831, -108.13992755196784, -109.2987762526628, -109.82536192480795, -111.28650061088359, -109.12820736404241, -109.37960655471406, -108.96014976926716, -107.97535047619023, -112.31953123574708, -109.06198330523004, -107.52722515967098, -107.31555373665437, -99.89671790804692, -107.44442600896275, -110.6549218761941, -108.02265794322076, -109.63582761762919, -110.00574746987859, -109.51565124961209, -109.3550083591902, -110.4541529175301, -107.85799722437162, -105.1197113090786, -110.25038075579738, -110.39710812865657, -109.3618876098789, -107.6131301952152, -109.21529527621463, -108.7995754403799, -108.48347353145697, -106.45678488065816, -109.60427918561142, -110.81194387812535, -109.52215044127382, -109.88751598659705, -109.30205143590227, -110.74984456751768, -109.03952092986351, -110.69170786328897, -110.39236248162467, -108.65456161733339, -107.60439764386904, -109.97367926606955, -110.2754359970249, -108.81546418006434, -106.99691398176165, -108.42047325825182, -107.24499915944605, -109.28116135603187, -108.70650358781573, -108.05516916105047, -107.20893100196241, -112.07029265690055, -109.38099990478445, -111.53461820465232, -108.11312509555277, -108.76714028655223, -109.89565008459624, -107.71879172001115, -108.08434857420214, -108.79142773619792, -107.25153085963885, -110.05595039449301, -109.31604222314259, -109.94405791565286, -109.04715370361387, -108.89278831045846, -108.84682466376424, -110.0067927716526, -107.63768959294084, -108.98109382020348, -111.4720219575084, -110.76023788797733, -108.78599647633777, -106.59726674064618, -108.66715709719243, -107.99134359630926, -110.11396713841884, -107.21091759882775, -108.08576824949941, -108.80217666857972, -111.72949572713338, -107.33126296136014, -107.33731660097102, -108.04470462977443, -109.42963925921418, -111.03517778720736, -109.55293581015796, -107.99948151285162, -106.59480934999681, -107.63777243313498, -108.96490626068824, -108.8948210299064, -108.30870516747477, -109.13612869658097, -109.59971429402015, -110.2571461001396, -108.7655464686992, -109.81144209568883, -109.80796806645141, -109.20948481699544, -108.68653880881129, -109.26329796696166, -109.22428132233863, -110.12571678351438, -109.14615461144786, -107.08261621308327, -109.11338327144382, -107.75421565039201, -107.45291780756361, -109.00477000647248, -107.41031480478154, -109.98948062864928, -107.45953654921264, -106.37522884807879, -107.7786128523167, -108.03610987358499, -108.05926797128022, -108.59400205554164, -109.89620453365603, -109.03811240487515, -109.96909236705363, -109.28212981785472, -109.6772152101994, -108.26493868190678, -110.55558039199732, -106.6252818398841, -110.19075011176416, -109.56520012524705, -109.8023423576176, -111.2697570480663, -108.26752571816566, -112.00337375484828, -109.85709226796116, -109.36922081321148, -108.8424844298318, -111.2512302139209, -110.61775974680471, -110.22501328999012, -107.76874906708105, -110.71023653476604, -109.4025656165291, -107.66667684986125, -107.59759854092948, -107.94763263251238, -107.3888591871119, -108.62692803125044, -109.18012867988286, -107.78662871481455, -108.5072814073944, -109.50348958982907, -109.95177634938378, -107.78756251182895, -108.03865042797304, -110.1814993556385, -109.34937567548833, -109.52162025123161, -109.50819015441117, -108.20953105254624, -110.52154040214435, -109.3324404469266, -109.2696617050831, -109.54675609195674, -108.5940367000989, -109.40184828664549, -108.2518305610941, -108.55972691669434, -109.03647225394408, -108.48166656251695, -107.42023429066523, -109.42453054302521, -110.09532345960083, -108.78315822119662, -109.97508586102265, -108.22687406536997, -109.17110028890058, -110.15390449992647, -107.88577458651508, -108.28851074361447, -108.52030295163331, -110.03496861709483, -109.40014319167584, -107.73048113044877, -108.17571683963915, -110.34839852994926, -108.55894048192191, -108.74107339998285, -111.17734138993401, -110.22946440841412, -109.45511941802884, -108.0657300641843, -109.33797363184166, -106.95974095511333, -107.93068343723691, -109.78867669512647, -107.2087297624043, -109.542665021243, -110.05035859052961, -110.30235238883523, -109.20586170783808, -109.2796396673401, -109.14260673746566, -108.22019460542734, -109.99011886871159, -109.89103038547285, -110.36964772493243, -108.62340319923602, -109.06779821699769, -109.21830861066148, -107.7402395759509, -107.7178850938205, -113.45665085929117, -109.24039191621704, -109.30387033426037, -107.61849760982835, -109.41430582703529, -109.11482836392241, -111.89328423764577, -111.84653367963301, -109.00674896486915, -109.84488648739638, -109.41914760797953, -108.53442910169935, -109.66883322968232, -107.68762956301386, -109.82583101109167, -107.83405397804887, -108.78052031141966, -107.37842078941692, -105.40843158543845, -108.81430898189338, -109.57374640194516, -109.41111270322058, -108.82621700188898, -110.2552502368822, -110.23903890097205, -110.52171662278697, -108.21249857906324, -109.97268479379733, -108.20088823960992, -108.85682002802234, -110.11642849164285, -109.94087886999255, -111.63180946270296, -108.20899499456195, -106.73341567332112, -109.90003508676807, -110.14688274481229, -109.62259307329889, -107.57811196819495, -106.88584597822792, -109.16132624528932, -109.78677836397806, -108.59319344451784, -108.55877448618652, -109.46883711353044, -108.47309455543844, -108.09487065732198, -109.82219079158135, -109.63780237877428, -109.28348848877269, -107.62893405379826, -109.46986737961593, -108.03089712610223, -110.3931917410696, -106.06970126043262, -109.41866550703786, -105.31710372440419, -109.20218082282653, -108.28467118008108, -108.80026326744611, -107.40729224715713, -111.07322915141532, -107.1057186510818, -107.98286374205958, -108.51298722989311, -108.69632670891366, -107.96509231988331, -108.15882223414738, -106.85862416470376, -109.70705792539056, -108.64519930633055, -106.78708421443504, -109.43552377900174, -109.4474526498122, -109.10135248755788, -111.43316642580763, -109.33457343739448, -110.23547887071898, -108.95690647379442, -109.21159903769149, -108.12969562680841, -110.82751409340537, -108.55724349027832, -109.8796329603075, -108.50369978374582, -107.43145467247209, -108.60003323209516, -108.77155705999647, -109.33806063660796, -108.37500858898439, -109.65641721611547, -109.81905873737344, -108.03483220769625, -110.48028107566635, -108.60527372219985, -109.28768201151478, -99.8804125587218, -108.8913334544964, -108.23534920737794, -111.07646463287153, -108.59029790589766, -110.3405916586831, -107.66387718565608, -108.73793152614131, -110.61440166477816, -108.76211382544581, -110.23236978486065, -109.10669297094852, -109.15247609779597, -109.00539004923506, -110.14424353412238, -110.55445060661157, -109.48721312920799, -108.17040942305823, -108.77592227268228, -108.77130256578067, -107.82494496098512, -109.57266989523707, -108.75767497229612, -108.13688624150026, -107.8280716764963, -105.676279602552, -107.6370316684844, -109.73508547021689, -109.25365178573009, -108.86767843317584, -109.70969944273735, -108.91917504090888, -109.97734866522867, -112.17308993943783, -110.28356299479682, -110.7927103729386, -110.30837645846702, -107.56364161860179, -109.50188349731121, -109.36065627483853, -109.75389877587511, -109.81713476007774, -108.14524057525358, -109.43832376796216, -110.89342891210596, -108.15657882822792, -106.84106061627887, -107.83091759905821, -108.61794662682962, -109.57142366843581, -109.85402645528154, -110.12877022469837, -109.19414429724044, -110.56168468006764, -108.74720588273881, -107.90448559921305, -108.54421401507743, -105.06700039841249, -109.17937358052484, -108.94317576365822, -107.79410219455083, -109.24955437598658, -108.23334395173994, -108.98759227946937, -107.05986359444529, -107.20956512998849, -109.00295831471958, -109.43119556916457, -108.93348410522628, -108.99932477701081, -106.6448790859128, -109.06877251308666, -107.67053918439544, -109.15052780608639, -110.16878033319385, -106.55101141640301, -108.02811045752685, -111.52173447126572, -110.16854119242062, -110.93164036911654, -111.25979320890855, -108.82629030379024, -108.52004501839738, -107.09697056562636, -108.94233383169858, -107.37962568194772, -109.1239201710643, -108.93949898577122, -110.62573772949195, -110.09592372075662, -107.56136391005947, -110.45600430869621, -108.79481000016084, -109.41462449554598, -109.30248158488335, -108.70735295493108, -109.9174743694956, -109.94232543385962, -110.71725446170196, -110.0346196158573, -110.34814317845934, -110.6651078322521, -107.55409880424479, -108.71734776861287, -109.50902203986271, -110.40207542979611, -108.7847687630861, -111.10599488129682, -109.30824728923263, -108.20134064331717, -110.55959112431609, -107.77099734327174, -110.23862843385446, -108.48520797666865, -108.54205896654946, -107.79288769037599, -109.84022250170581, -108.02758364115576, -109.35132492327935, -108.87009749667932, -109.86905123364855, -109.19826752168308, -106.835240323691, -109.37910022114056, -110.80633973102931, -109.12703823829597, -111.07432699570984, -111.8064506085314, -110.09349947650527, -108.66467295777367, -108.75119108236053, -112.63983351316729, -110.90940743670113, -110.27973159222081, -109.57141664526549, -108.61645363771719, -109.31742355616147, -109.5839599160637, -110.01188998365383, -110.01923429741011, -108.94779759137936, -108.26169431000017, -109.24553201026085, -109.95709526422822, -110.68677343596859, -108.7678734483002, -110.47090469179284, -110.31604700116512, -110.10256600741997, -109.76634647265719, -110.8830805828562, -109.94609564072982, -109.20662382740542, -108.12492970530919, -110.5274435478767, -108.02351960398035, -110.6264936805739, -107.14559226383577, -109.13821777857531, -111.05324489472586, -110.15190797512811, -107.96366234783144, -110.03950681967147, -109.17476300510336, -110.41251816187909, -111.39219865477246, -111.32530426869943, -109.97369363558423, -108.98666403063845, -109.62049358645565, -109.58130494498671, -111.72738873188874, -110.39825891106616, -108.57430325757545, -111.28625510212446, -108.77421250595326, -109.75025415031793, -109.51948456745635, -108.82129398637998, -109.81362137198361, -107.86292494316123, -107.49318292857053, -109.66948564589373, -109.54288390056654, -107.99912445612077, -110.3497559614379, -108.00549349666127, -110.01361420523357, -108.4977916421456, -109.67078387286976, -109.85678367732866, -112.01237658746248, -108.4855625950998, -110.84880875737286, -110.9178674382154, -110.44187536727453, -108.75076921971127, -110.04946286646651, -109.99780941000827, -110.14242932305507, -109.56343773672316, -109.6278993388131, -108.77419573790174, -109.10543670530926, -109.7801848627463, -110.30733124104881, -113.13440550301436, -109.32709134514755, -109.74136656933283, -110.01525283266193, -109.43924662938396, -110.25325289253, -107.75460576671303, -110.60057027395933, -110.71458404922404, -110.15788509050662, -110.69167485018224, -110.96006652476157, -111.01156633983031, -111.6058448010008, -109.51364005052672, -109.76058205940885, -108.43421621088261, -109.47973949170208, -109.25533250208288, -109.47422603921065, -111.36411644613841, -107.27566171102698, -110.45098686173688, -109.93589296291184, -109.03803734663714, -110.53118128434016, -110.2408872254969, -110.0532234862915, -109.94185495614619, -110.2662004220774, -109.51094016962288, -108.5210104215432, -108.13691752270934, -110.18460088390265, -108.32609309150783, -109.89652230508281, -109.80923900768477, -109.01917388968883, -110.01248300968739, -109.43415605440147, -108.09823485138017, -107.40637725320931, -109.40632232658412, -111.97981999127656, -111.16609811629485, -111.64500793960192, -110.99793748693381, -109.55531276386903, -110.2535662621666, -108.17429802469516, -109.09425673355422, -110.23187110421917, -110.55358397926925, -109.93461124753053, -109.55604345832225, -109.44569510408274, -109.72185151080762, -109.52963702944834, -109.2303630328152, -109.74819502244243, -109.3932530349457, -109.17096788339686, -110.46153727064616, -113.1073731246639, -109.43753070459397, -108.13332547768168, -109.42294574929969, -108.45798401969856, -110.29453435046327, -112.66249403705643, -108.78314667434937, -105.9634478773668, -109.14327524669528, -108.50645190860273, -100.81571594994128, -104.4482859840643, -110.68926237051092, -109.12362553230196, -109.45234390564677, -107.91461416156068, -110.67788819353727, -110.05744935668449, -111.78333392154664, -106.83628914455993, -110.11115457346548, -109.13434608275826, -110.80006861194663, -110.35323502651462, -112.29149906501372, -109.01656376530778, -109.30871662948859, -109.79736315392456, -109.17848983603582, -108.09752397056482, -111.6039030763455, -109.27008844877828, -110.84475733314184, -109.72393917557073, -111.31060762894991, -110.78858793807466, -107.12841545099752, -109.54510865218204, -105.2805426080281, -106.28514149354733, -109.50656759582803, -110.14700878401054, -110.49737016725709, -109.19811547071924, -109.92527399676051, -110.7961615015146, -109.7447227818197, -109.49432012009893, -108.714081576733, -110.09766801550917, -109.08448507943001, -110.36154838733857, -109.86328656267403, -109.21144237434696, -112.4145136888034, -108.57567151011159, -109.66748589540896, -109.72985837578446, -109.29989238126763, -109.85868902806475, -111.01778182304162, -111.23625326328558, -110.01270868104203, -109.27067928081415, -109.71171312410247, -109.28697459293629, -110.67868067201007, -110.91353786857455, -111.21479955051575, -109.11315965407708, -109.40418681804496, -107.80511819596003, -107.37201025889816, -111.81969609169838, -109.89875624306032, -110.29328043898657, -109.74853280072202, -111.39527865400605, -109.47746221101964, -111.75141177452517, -109.31325306583483, -109.30117448911659, -109.3997781364162, -109.45356931295724, -109.60585285774386, -111.33951689512735, -107.74187210470228, -109.62706021606415, -108.72139655505221, -109.79552836110567, -110.64354037499807, -110.96138240913136, -110.02215059889615, -110.92978442698893, -110.0620778287114, -110.85019647293322, -111.77397403227091, -109.81257196800128, -109.15643451383403, -110.72777566469594, -108.7463769025616, -109.80959395914073, -111.24500986151126, -110.48863498350322, -110.30863780110901, -109.79331354195703, -110.34087081762074, -109.45183222569266, -109.6440990067103, -111.15034876658994, -112.14912485578341, -111.8886180186196, -110.57054820211916, -111.07556239924551, -110.5872832735073, -110.28912501038172, -108.91501133754849, -111.44575118962761, -109.90799859177967, -109.74421995550023, -108.70941446115883, -110.28822893097275, -109.70039554000401, -110.33701797570251, -110.79445894683306, -109.57694314608153, -108.816904416038, -109.66517126767175, -109.39501469321644, -110.85775022889956, -109.3689402795614, -112.09107318723095, -110.67985626248422, -110.32971146814747, -112.08166943494875, -109.93955548712543, -109.31722953035252, -110.2062913031861, -108.22565380081006, -110.680898028151, -111.95386604441454, -110.83354130587097, -108.5873626748948, -111.97536144124408, -109.23944159551515, -111.57859477689586, -110.80135186615524, -110.4800953731021, -110.14040729648133, -109.25873050390551, -108.87000960474569, -110.97091597211167, -110.15787270199012, -111.62434537618091, -108.5421625277294, -110.42258666403919, -110.96896115868603, -108.98253068925274, -109.54245055160168, -110.28051096122468, -109.48060498658319, -109.77618362117276, -111.64513838754992, -111.13945484239875, -110.18094280356001, -110.43757222770748, -110.81588360154201, -110.11656805555333, -108.47936291282355, -109.16476249859961, -109.3549985917136, -110.77753190334253, -111.46065694661178, -110.40387985996301, -109.95673803226478, -111.58660981285446, -108.59894875229345, -109.37333363882607, -110.26849699991793, -109.30500469266264, -109.23789020998296, -110.82000706486865, -109.25927538839868, -111.03285659417519, -111.08899832832414, -110.69361682858042, -109.45187168573815, -109.9614018482838, -109.70209527974106, -112.11903952100165, -109.59713611623246, -110.70292028698111, -110.12743849746808, -110.63315585514292, -108.60450276298175, -109.32832664986026, -109.99753023477764, -109.46644696130294, -109.1781290160558, -111.58830180575129, -111.67229040267557, -111.3750024136205, -108.33616679452298, -109.99797067800029, -110.50892429124391, -108.66074740829372, -111.17094662568759, -109.87538933985836, -109.152526628291, -110.44623159817101, -110.21603106403009, -110.64376935639365, -109.36897426842583, -108.67303022227141, -109.89327693080823, -111.50442955563923, -111.37532237834381, -109.38132821290205, -109.73509680539144, -110.53918379735906, -111.22869870340647, -109.39977573957616, -110.3674665334106, -110.5366125953241, -109.99025356764304, -109.97300035646616, -109.87631077033762, -109.64608829594286, -113.02486102973394, -108.26250283140733, -109.62234918138763, -111.18766216512655, -110.33666026406992, -110.5808115327039, -108.2971671321189, -110.10964334161903, -110.61254021379767, -109.89852549557533, -110.16562049054073, -109.41433790018287, -111.2453823439446, -110.45554802599901, -113.11454453784393, -110.7333866145056, -110.00858191882439, -108.54745315874294, -110.08430415376903, -111.9006972727596, -110.3031506154679, -110.26331790366497, -109.36797925566673, -109.04860552478912, -111.83514212681175, -111.38960737633833, -109.01429665187288, -110.96404839103826, -108.95488871107163, -109.09652004914592, -111.884304581971, -110.57566691021339, -111.95113404442795, -110.13677174050159, -108.10078686353354, -107.69442565416006, -112.42676605669463, -109.12681161784135, -109.23120766087519, -110.57649395555585, -110.22143082743162, -108.40065951773644, -109.46923168308618, -111.39095086729745, -110.46375658526013, -111.45145283328486, -112.22610823637353, -110.61090190564383, -112.22250292674809, -111.7379343196361, -110.18530386733481, -108.93867365671692, -111.89304844956082, -109.06146134986984, -110.98405731832798, -109.76366821333497, -108.08326795663608, -109.95041147835065, -112.94140614324155, -111.79814935135965, -108.07337559063119, -109.13733403265212, -111.74906646037496, -111.12228668433455, -110.02899450462209, -110.22237716929811, -109.0224776891049, -110.18135850497721, -113.32516073881047, -111.3576490243877, -110.60510094465171, -109.6935518470342, -110.36313473154901, -111.95933240129618, -109.49625308071019, -109.18827910216122, -110.54311407822692, -108.4811035913567, -112.81280225723607, -108.86530665787413, -110.85796435061886, -110.40059714639627, -108.19250716343407, -108.96956521802292, -108.61281798886506, -109.78061525370413, -111.58885511891798, -109.06279169160345, -111.43043988466789, -111.63169336321079, -109.54702536206447, -109.62860636296405, -109.47865811135546, -108.02265793654806, -109.97461304995515, -110.72549884050886, -111.57309413919933, -110.03317891949746, -110.39570411598524, -110.27606115470397, -110.63294457306095, -110.71821689302902, -110.38076268941819, -111.51223508887897, -110.40703572670697, -112.24933273737743, -109.74954300082398, -108.46020292937696, -111.05315219575881, -110.38635148390118, -109.58268303790976, -112.34211536832117, -108.45894118755307, -108.96463982695337, -110.56040438523046, -110.67803313671729, -111.07349872375121, -110.42184162876096, -111.82081126435692, -108.85923651136297, -112.57723799596502, -113.65690874668172, -112.62314325834605, -110.70357529341362, -110.959925221544, -111.26336183001875, -108.1350700630152, -107.94545932312926, -111.17610778209841, -110.20386728310686, -108.55646511121591, -109.8400922569145, -111.73466587035968, -110.47272877573613, -108.33011124048193, -107.93042857580332, -108.60928277989103, -109.25240966798974, -108.96403833602028, -106.94222615757475, -109.37086694261907, -106.72743097285155, -109.03160193412796, -107.3549903889451, -106.8543848510082, -107.83503929060929, -106.30745467433752, -108.36915807168845, -107.13065938379303, -107.84769200880969, -106.08004345082777, -108.15244601930225, -108.37254117816573, -106.57863034819223, -108.1283698227614, -108.19776505569902, -107.58283412238643, -108.17365133196301, -108.6794309781181, -107.91552140588759, -111.60122989270022, -107.04360635941174, -111.55535949001795, -109.39870426166594, -109.55937904851662, -111.81389508925734, -109.88957041098786, -110.84764586896561, -110.59130246272693, -111.15944135223884, -110.19496154041607, -111.51861903129362, -110.74798816525838, -111.37312965175558, -110.10842817220238, -110.73198099204856, -111.36708667993291, -110.30840247819665, -110.11744489669044, -110.55237850846444, -108.2073528237766, -112.70750856801911, -110.99917956040802, -109.84949484779976, -111.3403161887679, -110.08924435263565, -110.17749213365616, -112.10849123224503, -110.94270741299202, -109.29350963424746, -110.33477486966507, -112.19620157705627, -111.45484078395934, -111.86858843505124, -110.22491147345858, -108.96177661263177, -108.67862820579893, -107.55155410582937, -108.27984439169573, -108.72682528077233, -110.64231212183269, -109.32873093119183, -112.98564364754564, -110.78933114228725, -108.50921025910479, -107.91087245586935, -112.57350030929283, -111.75871577457525, -108.42095298945462, -112.31266064114303, -110.1295657579673, -109.67444664474456, -110.33749884929306, -109.16098218724147, -109.63554874360221, -109.15892392675141, -111.90580809179818, -108.81196712336858, -111.42223552606656, -109.90571484965518, -109.99739812086352, -111.64103850263211, -111.31463957090885, -110.61247447444549, -110.20960333715526, -110.1707327818923, -109.70412636554525, -110.97278093107532, -110.24386747740314, -109.81378546061525, -110.83784085086458, -109.77357954318757, -111.22663832948885, -111.14563050139252, -110.87152231402447, -110.34246044319893, -109.97174570657546, -110.23599592972218, -111.08206161770731, -110.0073315341242, -111.11748366902188, -112.04005964728601, -109.81290191679287, -109.68543639040858, -112.01143296194752, -110.13641850530031, -108.19348942447623, -109.7534468948808, -109.36697824644176, -97.56454580435337, -104.97829040517887, -108.1539132982256, -110.048991273122, -107.46172505860011, -110.49269280640675, -109.94209901400029, -109.38576869679022, -111.43699124347364, -110.89973083498887, -111.2994445418276, -109.25144782032437, -113.25676258473536, -110.82078737428088, -109.97779571182073, -113.36294799183014, -111.38584551238931, -112.17267897274873, -108.56430946159155, -112.06841286528645, -110.36822473102735, -109.54758527532016, -110.48190506674653, -110.03535695860182, -109.3951469796576, -112.41910682256774, -111.38124138857238, -109.37850389100952, -111.65544568836181, -111.55876881606889, -109.3029209617236, -109.20030046194076, -108.82610577621037, -110.53329453526098, -109.96090595542142, -109.67834229432077, -110.62303603007352, -109.8388817181171, -109.22430039793213, -108.92749786663613, -110.05794249283548, -109.58534943218437, -110.50493887507297, -109.96373022997366, -111.0645036323456, -111.28501675364454, -109.77386932343008, -108.8952247140968, -110.09242801628717, -112.90943444063141, -110.72299296247249, -109.39094335967056, -110.95165384057718, -109.59809519359453, -110.4978602309597, -109.67109981692639, -111.2489619905986, -110.0937750887109, -109.76771021128954, -108.32976315018955, -111.3058145792439, -111.09464974601362, -110.99797900696136, -109.174315000222, -109.630351559617, -110.26289147175856, -110.22688407202517, -109.96748050100612, -112.13247633583758, -110.59994952890855, -110.93023020153811, -109.22457750926695, -110.26162558926984, -110.09713110375579, -111.73858994918328, -109.78183160058515, -109.7603471824367, -110.96016892586911, -111.23309626937036, -109.83093663960678, -114.05354944347246, -111.58202863059464, -110.42281828744524, -110.9521484732059, -112.5120328206343, -111.614891937737, -109.84428787405484, -111.61119567831453, -110.43095563229411, -111.71833448430398, -110.01132196809407, -109.37558169247951, -109.14091380022785, -110.42663661754088, -110.3598013572826, -109.78207135281417, -109.94058843992468, -109.88210328447205, -108.6217811850147, -107.17834387173707, -110.6447226986756, -111.10704778101115, -111.24396771977769, -110.47849395539598, -110.75150631628034, -109.67662689396347, -109.23145032835053, -108.83780193265358, -109.43468321661163, -102.22521103859944, -106.90009867479111, -108.91580608784525, -109.58671397003187, -110.56692028436989, -108.75103142680105, -111.00795573084157, -110.75039085328763, -109.48222099288613, -111.8621134816908, -110.26507966786443, -108.885924716389, -109.30841399453053, -112.3188631425597, -111.05677697153163, -108.8268571902449, -109.63028152237679, -114.82339015806369, -107.03435216376964, -111.34847692589166, -109.61354114874855, -112.32687758049907, -109.59816404231358, -111.64248480241805, -111.84075757907273, -110.44017657636552, -110.15181635726277, -111.93813663582833, -109.11826378836209, -109.99779889778326, -109.927119030584, -109.4389650887841, -111.52448814187727, -111.38736268499642, -110.51920914917922, -108.64230614681055, -108.90307263595304, -110.57246891832371, -109.65575340646116, -109.80359672370373, -108.83368585528197, -111.09385004343437, -108.83430005497769, -112.37784208819113, -109.50005381621696, -109.67421750136593, -111.39664088797532, -109.70867599669316, -109.52498993629875, -111.12341349673187, -110.0484037026941, -109.55138667646308, -111.06614422098669, -109.4785941493091, -110.25724082617013, -110.93950616855716, -110.53487953881397, -111.45722057988401, -110.32393446412904, -110.34361936710438, -108.6610336097813, -109.53631603696368, -108.06930707969195, -107.68056561368934, -108.73860971027449, -108.87111384617579, -108.40433837098611, -110.55999576884835, -106.83832061167207, -108.28786975902513, -109.18482905697472, -107.81071696594883, -107.91047268802457, -108.79613111673706, -111.05361322310213, -109.97897453479862, -109.12920563729425, -111.20538391490288, -109.26286135293664, -111.31400407177502, -109.92167984752287, -110.70854322826071, -108.59406515713611, -109.69371333227458, -109.36664873267313, -110.35521729513704, -110.40667924006368, -112.0181844636846, -111.01529188207431, -110.59246505728431, -109.95068312717868, -110.75807466894047, -109.58596443762707, -111.12127793384956, -109.59041634463125, -111.56255571372793, -110.43405578864342, -108.39660324329928, -111.1420710307505, -113.64788483868595, -111.67645688353934, -111.36878760365944, -109.68523694561108, -110.11608766310304, -109.25670490330123, -110.73546181099229, -111.77855039399805, -107.9662794718261, -109.67483334602832, -109.891258579519, -110.24757768183042, -109.50202895993814, -110.07763831916637, -109.96891925839451, -110.97268925927641, -109.31698133827767, -112.27933593506792, -110.36206721075725, -109.47379463718867, -110.27836850941338, -110.63738280998388, -111.3611682777485, -110.72689155959884, -111.55480904927032, -111.16689658479412, -110.35555645743601, -111.56609319131051, -110.88279459952174, -114.73607246523177, -109.95813757295693, -107.64639932425493, -111.26486783320321, -112.03946356928121, -111.8915972448334, -110.35245920812773, -110.83155104803564, -110.67437747473863, -110.9959682920065, -110.7815352345103, -111.13722283763049, -112.54797265493127, -110.06894780898469, -111.65186554925783, -111.83545188116254, -110.65894756123697, -108.48458025065264, -112.43760714427981, -114.1368408201927, -110.40065777895025, -110.1066998945526, -108.60654239598591, -110.5716060205154, -110.74257357180736, -111.1136089342442, -111.53539811075092, -113.2559601458872, -109.2003227548348, -110.42285840441025, -111.4086884998834, -111.61503050693868, -110.8194303494779, -108.9701587059964, -112.58521089509063, -110.10873915265242, -112.43440038319561, -110.03468788439882, -111.57896603236308, -110.21939233582523, -109.03614470500777, -110.11738923539659, -109.55359574898291, -110.416473622654, -109.4626868574157, -111.17164025076731, -110.3579689035081, -109.04338716157822, -112.36157114517567, -109.32125615922843, -112.71105693789394, -110.11019129547768, -108.96439402555632, -111.107663418839, -111.48306369859839, -110.9317530461794, -107.98628540532181, -111.1636972328743, -110.47837837583148, -109.04649309175733, -110.27110334963734, -111.35803630614352, -110.77259078859605, -111.46352820533895, -111.16789261049541, -109.2376344776325, -111.6795794983659, -111.74292205167644, -109.40835022991612, -111.02163652600731, -108.79482078001607, -110.6718658416566, -111.08747067599332, -112.15383726791498, -109.47049126158717, -109.061574046483, -111.23993049318979, -111.02521156588335, -109.46012868444186, -110.13918914826291, -112.08180381836377, -110.61929875223015, -111.4424805369965, -111.43420275069585, -109.71347556238717, -110.24726273025648, -109.7860268673935, -109.94126895018422, -111.41948668868926, -108.90555991781676, -110.81242861886172, -109.65007052722677, -112.12672329335953, -110.01123170946096, -111.13980448279096, -113.92013682657084, -108.6000853867411, -110.66793592761913, -110.61237681642844, -110.00839105230496, -109.38083187034974, -109.46119372195675, -110.3708067287448, -108.55518656223285, -113.33935987443276, -111.92184778392033, -111.80820718236087, -107.36852757311246, -109.51077803361602, -110.066791721019, -108.756710558672, -107.91391289865918, -110.72851430959301, -111.39074956442978, -112.928843679455, -109.87348280521556, -112.21371750380071, -110.82495902297394, -109.94006136010094, -110.58757785050143, -110.2790091349881, -111.43884888223081, -108.09540986530712, -109.63783244641691, -110.19577975613292, -110.01690033746098, -112.75938920157155, -109.27158857362184, -111.19519821680541, -110.14381902425255, -110.45955291199236, -111.55660330002316, -110.75604254261134, -111.02122553784838, -111.6490091060193, -110.93362819419399, -110.49033159684308, -110.70789549836027, -110.41991882034145, -110.0264093421208, -109.18432746063652, -110.15292268755287, -112.40733942236504, -111.32869665965416, -110.95418667871114, -111.14291568823575, -111.75555369152653, -112.98146297069803, -109.73870744292117, -111.33806139459435, -110.18838799491355, -112.60408243005732, -110.26112648646833, -110.58257045107274, -109.75155437454112]}, ...(2 in all)]
  in  "FFT 1 Choice 1":u16(ring) items=["T1 Y", "T1 X", "T1 Sum", "T2 Y", "T2 X", "T2 Sum", "T1 FB X", "T1 FB Sum", "T2 FB X", "T2 FB Sum", "PSD Y", "PSD X", "PSD Y Sum", "none"]
  in  "FFT 2 Choice 1":u16(ring)=3 items=["T1 Y", "T1 X", "T1 Sum", "T2 Y", "T2 X", "T2 Sum", "T1 FB X", "T1 FB Sum", "T2 FB X", "T2 FB Sum", "PSD Y", "PSD X", "PSD Y Sum", "none"]
  in  "FFT 1 Choice 2":u16(ring)=1 items=["T1 Y", "T1 X", "T1 Sum", "T2 Y", "T2 X", "T2 Sum", "T1 FB X", "T1 FB Sum", "T2 FB X", "T2 FB Sum", "PSD Y", "PSD X", "PSD Y Sum", "none"]
  in  "FFT 2 Choice 2":u16(ring)=4 items=["T1 Y", "T1 X", "T1 Sum", "T2 Y", "T2 X", "T2 Sum", "T1 FB X", "T1 FB Sum", "T2 FB X", "T2 FB Sum", "PSD Y", "PSD X", "PSD Y Sum", "none"]
  in  "Compute FFT":bool
  in  "Reset FFT":bool
  in  "# Spectra to Ave.":dbl=25.0
  out "Ave. Time (s)":dbl=1.5
  out "1 Channel":waveform(dbl)(graph)={"t0"=timestamp(0 s since 1904-01-01), "dt"=1.4999999999999999e-05, "Y"=array[20000 elements], "attributes"=variant("NI_ChannelName"=variant(string "T1 Y"))}
  out "Slow mean":dbl=-0.021350993491001932 format="%0.2f"
  in  "Slow mean N ave.":dbl=1.0 min=1.0 step=1.0
  out "Mean Intensity":dbl=-0.021350993491001957
  out "Sigma":dbl=0.006231607115497778
  out "Sigma/Mean":dbl=-0.2918649719098079
  in  "Subtract mean":bool
  in  "High Res. Display":u16(ring) items=["T1 Y", "T1 X", "T1 Sum", "T2 Y", "T2 X", "T2 Sum", "T1 FB X", "T1 FB Sum", "T2 FB X", "T2 FB Sum", "PSD Y", "PSD X", "PSD Y Sum"]
  out "APD 1 Rate (Hz)":dbl format="%#_3p"
  out "Feedback overload":bool
  in  "Confocal Linescan":bool
  in  "Speed (nm/s)":dbl=100.0
  in  "Furthest Withdraw (MHz)":dbl=15.0
  in  "Confocal Image":bool
  in  "T1 offset_x (mV)":dbl=44.132512662199076 format="%#_2g"
  in  "T1 kappa_x (pN/nm)":dbl=0.1608167093260824 min=0.0 step=0.001 format="%#_2g"
  out "Time (s)":dbl=40.5
  in  "Start Saving":bool
  in  "Cal sets to save":u32=50 min=1 step=1
  in  "Comment (data description)":string="testing confocal setup"
  out "Calibrating Trap...":bool
  in  "Save Calibration":bool
  in  "N sets to save":u32=200 caption="N Sets"
  in  "Save N Sets":bool
  out "Progress":u16(slide) scale=0.0..100.0
  out "Buffer Status":dbl(slide) scale=0.0..1.0
  out "Overflow (data lost)":bool
  in  "Reset":bool
  in  "T1 alpha_x (nm/V)":dbl=701.8425766517444 step=10.0 format="%#_3g"
  in  "T2 alpha_x (nm/V)":dbl=806.869454518421 step=10.0 format="%#_3g"
  in  "T2 kappa_x (pN/nm)":dbl=0.13871102209446912 min=0.0 step=0.001 format="%#_2g"
  in  "T2 offset_x (mV)":dbl=-16.403354316809207 format="%#_2g"
  in  "Trap Raster Scan":bool
  out "Current Position":dbl[](array[numeric])=[4.2944, 4.91027471, 2.9278058] format="%7_7g"
  in  "Pump write delay (ms)":dbl=300.0
  in  "All Pump Parameters":T5={"Pump 1"={"Diameter (mm)"=4.61, "Units"=4.0, "Volume"=100.0, "Rate"=50.0}, "Pump 2"={"Diameter (mm)"=4.61, "Units"=3.0, "Volume"=0.0, "Rate"=0.0}, "Pump 3"={"Diameter (mm)"=4.61, "Units"=4.0, "Volume"=100.0, "Rate"=250.0}}
  in  "Tab Interlacing Feedback":T6(tab)=enum."Feedback on Trap Position"
  in  "RF phase reset before cycles":bool
  in  "Phase increment trap 2":fxp<+/-,64,32>
  in  "Phase increment trap 1":fxp<+/-,64,32>
  in  "Phase offset method":u8=3
  in  "Next trap write delay (ticks)":u16
  in  "DIO count 3 (ticks)":u32=200
  in  "DIO count 2 (ticks)":u32=200
  in  "DIO count 1 (ticks)":u32=200
  in  "BD 2 Amplitude 3 (%)":dbl min=0.0 max=75.0 step=1.0
  in  "BD 2 Amplitude 2 (%)":dbl min=0.0 max=75.0 step=1.0
  in  "BD 2 Amplitude 1 (%)":dbl min=0.0 max=75.0 step=1.0
  in  "BD 1 Amplitude 3 (%)":dbl min=0.0 max=75.0 step=1.0
  in  "BD 1 Amplitude 2 (%)":dbl=42.0 min=0.0 max=75.0 step=1.0
  in  "BD 1 Amplitude 1 (%)":dbl=40.0 min=0.0 max=75.0 step=1.0
  in  "Freq or Amp switch first":bool=TRUE
  in  "Swap F1 and F2":bool
  in  "Freq switch delay":u16=9
  in  "Amp switch delay":u16=4
  in  "Raster to target force?":bool
  in  "MCL Step Increment (V_int)":dbl=3.0
  in  "MCL/AOM Scale Tweak":dbl=1.0
  in  "MCL Step Position Ratio":dbl=0.5
  in  "Move MCL Also?":bool
  out "Initial delta (MHz)":dbl=20.0
  in  "Restart DMA? (AOD)":bool=TRUE caption="Restart DMA?"
  in  "Save scans":bool=TRUE
  out "AOD Scan I":u64=2 caption="Scan I"
  out "AOD Scanning":bool caption="Scanning"
  in  "Start AOD Scan":bool caption="Start Scan"
  out "Progress 2":u16(slide) caption="Progress" scale=0.0..100.0
  in  "Abort save 2":bool caption="Abort save"
  out "MCL Count":dbl=782931.6080202644
  out "Trap 2 amplitude":ext
  out "Trap 1 amplitude":ext
  in  "PID gains":T7={"proportional gain (Kc)"=0, "integral gain (Kc*Ts/Ti)"=5, "derivative gain (Kc*Td/Ts)"=0}
  in  "Semi Passive ON":bool
  in  "DNA stiffness (pN / nm)":dbl=0.1
  in  "Semi Passive mode":enum16{"None", "Use Feedback", "Sharp Jump"}(ring)
  in  "Jump Force (pN)":dbl
  in  "Tab Control 8":enum32{"Main Setting", "Details"}(tab)
  in  "Real time offset \ncorrection for setpoint":bool=TRUE
  in  "Negate offset difference":bool
  out "B factor":dbl=0.9916156324677038
  out "Trap Pos FB Int Signal":fxp<+/-,24,9>=42.09515380859375 format="%.18g"
  out "Trap Pos FB Int-Norm Signal":fxp<+/-,16,1>=0.042083740234375 format="%.16g"
  out "Trap X AI1 (DMA)":T8={"Set 1"=0.030731201171875, "Set 2"=-0.0113525390625}
  in  "N El. to Ave.":dbl=10000.0
  out "Trap Pos FB Action":i64=-32767
  out "Mean T1 Position (nm)":dbl=-4.784226348419907e-12 caption="Mean T1 (nm)" format="%0.2f"
  out "Trap 1 Position RMS (A)":dbl caption="RMS (Ang)"
  in  "Setpoint offset\nCorrection values":dbl[](array[numeric])=[0.024496601698410773, 0.024671186719617436, 0.024845771740824106, 0.025020356762030765, 0.02519494178323743, 0.025369526804444095, 0.025544111825650764, 0.025718696846857424, 0.025893281868064093, 0.026067866889270756, 0.026242451910477423, 0.026417036931684082, 0.02659162195289075, 0.026766206974097418, 0.02694079199530408, 0.027115377016510744, 0.027289962037717407, 0.027464547058924076, 0.02763913208013074, 0.027813717101337402, 0.027988302122544065, 0.02816288714375073, 0.028337472164957394, 0.02851205718616406, 0.028686642207370723, 0.028861227228577393, 0.02903581224978405, 0.029210397270990722, 0.029384982292197385, 0.02955956731340405, 0.02973415233461071, 0.029908737355817377, 0.030083322377024047, 0.03025790739823071, 0.030432492419437372, 0.030607077440644035, 0.0307816624618507, 0.030956247483057368, 0.03113083250426403, 0.0313054175254707, 0.03148000254667736, 0.03165458756788402, 0.03182917258909068, 0.03200375761029735, 0.032178342631504014, 0.03235292765271068, 0.03252751267391735, 0.03270209769512401, 0.03287668271633068, 0.033051267737537346, 0.033225852758744005, 0.03340043777995067, 0.03357502280115733, 0.033749607822364, 0.033924192843570664, 0.03409877786477733, 0.034273362885983996, 0.034447947907190656, 0.03462253292839732, 0.03479711794960398, 0.03497170297081065, 0.035146287992017314, 0.03532087301322398, 0.035495458034430646, 0.035670043055637306, 0.03584462807684397, 0.036019213098050645, 0.036193798119257305, 0.03636838314046397, 0.03654296816167063, 0.0367175531828773, 0.03689213820408396, 0.03706672322529063, 0.037241308246497296, 0.037415893267703955, 0.03759047828891062, 0.03776506331011729, 0.03793964833132395, 0.03811423335253061, 0.03828881837373728, 0.038463403394943946, 0.038637988416150605, 0.03881257343735727, 0.03898715845856393, 0.0391617434797706, 0.03933632850097726, 0.03951091352218393, 0.039685498543390596, 0.03986008356459726, 0.04003466858580393, 0.040209253607010595, 0.040383838628217254, 0.04055842364942392, 0.04073300867063058, 0.040907593691837246, 0.04108217871304391, 0.04125676373425058, 0.041431348755457245, 0.0416059337766639, 0.041780518797870564, 0.04195510381907723, 0.042129688840283896, 0.04230427386149057, 0.04247885888269723, 0.042653443903903895, 0.04282802892511056, 0.04300261394631722, 0.04317719896752389, 0.043351783988730554, 0.04352636900993721, 0.04370095403114388, 0.043875539052350546, 0.04405012407355721, 0.04422470909476388, 0.04439929411597054, 0.044573879137177204, 0.04474846415838387, 0.044923049179590537, 0.045097634200797196, 0.04527221922200386, 0.04544680424321053, 0.045621389264417195, 0.04579597428562386, 0.04597055930683052, 0.04614514432803718, 0.046319729349243846, 0.04649431437045051, 0.04666889939165718, 0.046843484412863845, 0.04701806943407051, 0.04719256456184452, 0.04736536676840916, 0.04753446267808822, 0.047696991448649737, 0.04784953848765512, 0.04799284096907562, 0.048127712917801824, 0.048257934523222495, 0.04838705366421733, 0.04851995197559876, 0.04865949840047511, 0.04880178465045004, 0.0489357994772595, 0.04905304538798107, 0.0491519464532862, 0.049234486275402736, 0.04930263064515607, 0.04935733149089569, 0.04939552771001872, 0.04941451823245213, 0.04941830757306315, 0.049410747020732684, 0.049392795273013504, 0.049367258833286985, 0.049339629147657244, 0.049311849604908836, 0.04928407006216041, 0.049256290519411994, 0.04922851097666357, 0.04920073143391515, 0.04917295189116673, 0.04914517234841831, 0.049117392805669895, 0.049089613262921473, 0.04906183372017306, 0.04903405417742463, 0.04900627463467622, 0.0489784950919278, 0.048950715549179374, 0.04892293600643097, 0.04889515646368254, 0.048867376920934125, 0.0488395973781857, 0.04881181783543728, 0.04878403829268886, 0.04875625874994044, 0.048728479207192026, 0.0487006996644436, 0.04867292012169519, 0.04864514057894676, 0.04861736103619835, 0.048589581493449926, 0.048561801950701505, 0.04853402240795309, 0.04850624286520466, 0.04847846332245625, 0.04845068377970783, 0.04842290423695941, 0.048395124694210985, 0.04836734515146257, 0.04833956560871415, 0.04831178606596573, 0.048284006523217314, 0.048256226980468886, 0.04822844743772048, 0.04820066789497206, 0.048172888352223636, 0.048145108809475215, 0.048117329266726794, 0.04808954972397837, 0.04806177018122996, 0.048033990638481544, 0.048006211095733116, 0.0479784315529847, 0.04795065201023628, 0.04792287246748786, 0.04789509292473944, 0.04786731338199102, 0.0478395338392426, 0.04781175429649418, 0.04778397475374576, 0.047756195210997346, 0.047728415668248925, 0.047700636125500503, 0.04767285658275208, 0.04764507704000366, 0.04761729749725524, 0.047589517954506826, 0.047561738411758404, 0.04753395886900998, 0.04750617932626157, 0.04747839978351315, 0.047450620240764727, 0.047422840698016305, 0.047395061155267884, 0.04736728161251948, 0.047339502069771056, 0.047311722527022634, 0.04728394298427421, 0.04725616344152579, 0.04722838389877737, 0.047200604356028956, 0.047172824813280535, 0.047145045270532114, 0.0471172657277837, 0.04708948618503528, 0.04706170664228686, 0.047033927099538436, 0.047006147556790015, 0.0469783680140416, 0.04695058847129318, 0.04692280892854476, 0.046895029385796344, 0.04686724984304792, 0.0468394703002995, 0.04681169075755108, 0.04678391121480266, 0.04675613167205424, 0.046728352129305824, 0.0467005725865574, 0.04667279304380899, 0.04664501350106057, 0.046617233958312146, 0.046589454415563725, 0.046561674872815303, 0.04653389533006689, 0.046506115787318475, 0.046478336244570054, 0.04645055670182163, 0.04642277715907321, 0.04639499761632479, 0.04636721807357637, 0.046339438530827955, 0.04631165898807953, 0.04628387944533112, 0.0462560999025827, 0.04622832035983428, 0.046200540817085856, 0.046172761274337434, 0.04614498173158901, 0.04611720218884059, 0.04608942264609218, 0.046061643103343757, 0.04603386356059534, 0.04600608401784692, 0.0459783044750985, 0.04595052493235008, 0.04592274538960166, 0.045894965846853236, 0.045867186304104815, 0.0458394067613564, 0.045811627218607986, 0.045783847675859565, 0.045756068133111144, 0.04572828859036272, 0.0457005090476143, 0.04567272950486588, 0.04564494996211747, 0.04561717041936905, 0.04558939087662063, 0.04556161133387221, 0.04553383179112379, 0.04550605224837537, 0.045478272705626946, 0.045450493162878525, 0.04542271362013011, 0.045394934077381696, 0.045367154534633275, 0.045339374991884854, 0.04531159544913643, 0.04528381590638801, 0.04525603636363959, 0.04522825682089117, 0.045200477278142755, 0.045172697735394333, 0.04514491819264592, 0.0451171386498975, 0.04508935910714908, 0.045061579564400656, 0.045033800021652234, 0.04500602047890381, 0.04497824093615539, 0.044950461393406985, 0.04492268185065856, 0.04489490230791014, 0.04486712276516172, 0.0448393432224133, 0.04481156367966488, 0.044783784136916464, 0.04475600459416805, 0.04472822505141963, 0.04470044550867121, 0.044672665965922786, 0.044644886423174365, 0.044617106880425944, 0.04458932733767752, 0.04456154779492911, 0.044533768252180694, 0.04450598870943227, 0.04447820916668385, 0.04445042962393543, 0.04442265008118701, 0.04439487053843859, 0.04436709099569017, 0.04433931145294175, 0.04431153191019333, 0.04428375236744492, 0.044255972824696496, 0.044228193281948075, 0.044200413739199654, 0.04417263419645123, 0.04414485465370281, 0.0441170751109544, 0.04408929556820598, 0.04406151602545756, 0.04403373648270914, 0.04400595693996072, 0.0439781773972123, 0.043950397854463884, 0.04392261831171546, 0.04389483876896704, 0.04386705922621863, 0.043839279683470206, 0.043811500140721785, 0.04378372059797336, 0.04375594105522494, 0.04372816151247652, 0.04370038196972811, 0.04367260242697968, 0.043644822884231264, 0.04361704334148285, 0.04358926379873443, 0.04356148425598601, 0.043533704713237587, 0.043505925170489165, 0.04347814562774075, 0.04345036608499233, 0.043422586542243916, 0.043394806999495494, 0.04336702745674707, 0.04333924791399865, 0.04331146837125023, 0.043283688828501816, 0.0432559092857534, 0.04322812974300498, 0.04320035020025656, 0.04317257065750814, 0.04314479111475972, 0.043117011572011296, 0.04308923202926288, 0.04306145248651446, 0.04303367294376604, 0.043005893401017625, 0.0429781138582692, 0.04295033431552078, 0.04292255477277236, 0.04289477523002394, 0.04286699568727552, 0.0428392161445271, 0.042811436601778684, 0.04278365705903027, 0.04275587751628185, 0.04272809797353343, 0.042700318430785006, 0.042672538888036585, 0.042644759345288163, 0.04261697980253975, 0.04258920025979133, 0.04256142071704291, 0.04253364117429449, 0.04250586163154607, 0.04247808208879765, 0.04245030254604923, 0.04242252300330081, 0.042394743460552387, 0.04236696391780398, 0.04233918437505556, 0.04231140483230714, 0.042283625289558716, 0.042255845746810294, 0.04222806620406188, 0.04220028666131346, 0.04217250711856504, 0.042144727575816616, 0.0421169480330682, 0.04208916849031978, 0.04206138894757136, 0.04203360940482294, 0.04200582986207452, 0.0419780503193261, 0.041950270776577675, 0.04192249123382926, 0.041894711691080846, 0.041866932148332425, 0.041839152605584004, 0.04181137306283558, 0.04178359352008716, 0.04175581397733874, 0.04172803443459032, 0.0417002548918419, 0.04167247534909349, 0.04164469580634507, 0.04161691626359665, 0.04158913672084823, 0.041561357178099806, 0.0415335776353514, 0.04150579809260298, 0.041478018549854556, 0.041450239007106135, 0.041422459464357714, 0.04139467992160929, 0.04136690037886087, 0.04133912083611246, 0.04131134129336403, 0.04128356175061562, 0.04125578220786719, 0.04122800266511878, 0.04120022312237036, 0.04117244357962194, 0.041144664036873516, 0.041116884494125094, 0.04108910495137668, 0.04106132540862826, 0.04103354586587984, 0.041005766323131417, 0.040977986780383, 0.04095020723763458, 0.04092242769488616, 0.04089464815213774, 0.04086686860938932, 0.0408390890666409, 0.04081130952389249, 0.04078352998114407, 0.040755750438395646, 0.040727970895647225, 0.040700191352898804, 0.04067241181015039, 0.040644632267401976, 0.04061685272465355, 0.04058907318190513, 0.04056129363915671, 0.04053351409640829, 0.04050573455365987, 0.04047795501091145, 0.040450175468163034, 0.04042239592541461, 0.0403946163826662, 0.04036683683991778, 0.04033905729716935, 0.040311277754420935, 0.040283498211672514, 0.0402557186689241, 0.04022793912617567, 0.04020015958342725, 0.040172380040678836, 0.04014460049793042, 0.040116820955182, 0.04008904141243358, 0.04006126186968516, 0.04003348232693674, 0.04000570278418832, 0.03997792324143991, 0.03995014369869149, 0.039922364155943066, 0.039894584613194645, 0.03986680507044622, 0.0398390255276978, 0.03981124598494939, 0.03978346644220096, 0.039755686899452546]
  in  "Tab Green Scanning":enum32{"Timing", "MCL Scan", "Analog Out"}(tab)=enum."MCL Scan"
  out "APD 2 Gate Late Counter":u32
  out "APD 2 Gate Relative Phase":i16
  in  "Phase Adj. (APD 2 Gate)":i16=20
  in  "Initial Phase Adjustment (APD 2 Gate)":i16=45
  out "APD 1 Gate Late Counter":u32
  out "APD 1 Gate Relative Phase":i16
  in  "Phase Adj. (APD 1 Gate)":i16=20
  in  "Initial Phase Adjustment (APD 1 Gate)":i16=50
  in  "Save APD Data\nwith Trap Data":bool=TRUE
  out "APD FIFO Elements Remaining":u32
  out "APD Acq Late Counter":u32
  out "APD Acq Relative Phase":i16
  in  "Phase Adj. (APD Acq)":i16=20
  in  "Initial Phase Adjustment (APD Acq)":i16
  in  "Invert APD Gate":bool caption="Invert Gate"
  in  "APD Gate OFF Count":u32=450 caption="Gate OFF Count"
  in  "APD Gate ON Count":u32=150 caption="Gate ON Count"
  in  "APD Gate":enum32{"ON", "OFF", "Interlace"}(radio)=enum."Interlace"
  in  "APD Integration Time (s)":dbl=0.01 caption="Integration Time (s)"
  out "APD Int. Count":u32=400000 format="%.0p"
  in  "Tab Control 5":enum32{"PSD X", "PSD Y", "Other Data Channel"}(tab)
  out "Data map":dbl[][](graph)=[[-0.01671932143166878, -0.016392818706373227, -0.016060241502617766, -0.016885058281480972, -0.016633639866051188, -0.01614297111485056, -0.01624632439809061, -0.016223291898502697, -0.016322135358181895, -0.015998827366942206, -0.01674383457317074, -0.016349622303473588, -0.01611571290004051, -0.015972334649942688, -0.016306900004507047, -0.016265804263496074, -0.0160006281874421, -0.01579815848604542, -0.015557994770877373, -0.01623934207097493], [-0.016401746716030643, -0.016486228679580477, -0.016405819418185925, -0.017006941359896506, -0.01609698301441303, -0.0159938373980257, -0.015449969664593804, -0.016068061784641922, -0.016115383931390913, -0.015648222289449794, -0.01653040435156989, -0.01664368093936457, -0.015976629115606142, -0.015769041987412753, -0.015716784490458328, -0.016104708313091028, -0.015807740113897233, -0.016007795937736217, -0.015716865824611653, -0.016131560547170874], [-0.016881180243279052, -0.016682362901092443, -0.01653521208533211, -0.016569663649832547, -0.016584350108926265, -0.015788034358096, -0.01572997381191265, -0.016848256863673278, -0.016450971094654886, -0.016646544202256155, -0.016533647976865372, -0.01643411945121718, -0.01642968729491641, -0.015287525792493872, -0.015664412933211656, -0.016705160893495323, -0.01634751515697455, -0.016385950364931786, -0.01641611962972788, -0.016336369365154098], [-0.016944386833653874, -0.017209095062396696, -0.01643647162326984, -0.0169434622427136, -0.01645749558522405, -0.016283892481898044, -0.016603972603686925, -0.016019804038190342, -0.01633990863890397, -0.016779562572954584, -0.01649257003377154, -0.01633196294664365, -0.01681717360495772, -0.016151141680784836, -0.015631110690343758, -0.01616762209708058, -0.01570812545409377, -0.016238042109499973, -0.016140009377557954, -0.015480352129179791], [-0.016627380272623872, -0.016987040432100503, -0.0162998105424607, -0.01635693474229572, -0.016728613514399027, -0.015877063835195653, -0.01632422175035657, -0.015987062444069455, -0.016082210905250194, -0.016795453503208664, -0.0170165982501747, -0.016041147401410074, -0.015844635002206515, -0.01588368721722097, -0.016415515701510675, -0.01625686223052733, -0.015522307984761095, -0.016125254990784654, -0.016133227363549094, -0.016093654313254407], [-0.016918226627058684, -0.016546339201955095, -0.016238630263811032, -0.01698719582491472, -0.016111760237599002, -0.016169388046078873, -0.01635628471807927, -0.016477982760217016, -0.016022494806163096, -0.01635452184408291, -0.016437829589091835, -0.01620151587720066, -0.016192846971583803, -0.016361330735626047, -0.015920360440429684, -0.015596058601637491, -0.015839057608204695, -0.01590683226225114, -0.016147455226815495, -0.016061133185195295], [-0.016634948322751798, -0.016569012123295146, -0.01662465918442623, -0.01677966319575081, -0.016244237674368125, -0.016934028324529424, -0.015994902143504568, -0.01577806108898649, -0.015702882269567658, -0.01637426003303808, -0.016516796952512437, -0.01646180977161214, -0.017050841082784957, -0.015210920961454804, -0.016180578875882937, -0.01607665952058283, -0.01643056573904152, -0.01624726697921726, -0.016811320756287537, -0.015704237088347145], [-0.016797771368752906, -0.01616083928333069, -0.016453251971550422, -0.01638112181272177, -0.01590261356594244, -0.01608147749759244, -0.016020370516697566, -0.01666407664114518, -0.01638481284701757, -0.016175328500489604, -0.015634096607040564, -0.01659680945708638, -0.01626086024191585, -0.016096523812787963, -0.015760521307245458, -0.01615157630765101, -0.01563169067138887, -0.016252628883934674, -0.016238504839935688, -0.016296984466382107], [-0.01667963634531472, -0.015869270181190567, -0.01639782773103042, -0.01636439382881424, -0.01666285543553242, -0.016692875783958446, -0.016121724588237546, -0.016079967645743654, -0.01632967716613466, -0.0165840590606689, -0.01625421166976198, -0.016098422085292646, -0.016839026057991122, -0.01618499247497865, -0.015391600029151147, -0.016339655626827314, -0.015612166346566772, -0.015935379715422582, -0.015751812989013417, -0.016043659821299468], [-0.016548348623009697, -0.016991017407413864, -0.016507403110123067, -0.016536793878207376, -0.016691120016137963, -0.01577327808799238, -0.016241167864690632, -0.016068735698142586, -0.015840387814149363, -0.016134357225980472, -0.015841333026290365, -0.0163038114660657, -0.01664004009343323, -0.015517995684912076, -0.01510255011893393, -0.016011490555515644, -0.01579492187645071, -0.016061693314939115, -0.016070791499276448, -0.015958266458419586], [-0.017158052821315092, -0.016990745992594425, -0.01659770916824297, -0.016038631482428484, -0.016146804022232154, -0.01576224906436341, -0.016188682344964726, -0.016682643876198163, -0.016363274145684666, -0.01639850086318443, -0.015896821220835786, -0.015725853678146523, -0.01601090474694708, -0.015561700057052, -0.015999978841264924, -0.01601836056022779, -0.016765653382201824, -0.016096916088969352, -0.016073837821775124, -0.015692878955540758], [-0.01663419671959083, -0.016709422884628247, -0.017440867448447667, -0.016794212435564802, -0.016747490720603195, -0.017381751349696366, -0.016447004176656708, -0.016200072448833015, -0.016045160782039845, -0.01632124390318996, -0.01679169430451878, -0.016160654157203025, -0.016749084172300182, -0.015317451826774697, -0.01616958983467165, -0.015522373654827837, -0.016042029406509332, -0.016273918604509642, -0.016417636335760946, -0.01644358854973573], [-0.016334373306253872, -0.016757773312361682, -0.016379901767213538, -0.016648254461466998, -0.016415141976627915, -0.016163802224577726, -0.01585938187523836, -0.01585373106879133, -0.015975877635193418, -0.01599748687305492, -0.016737850820893803, -0.01594503246026053, -0.01605934628998727, -0.0158171814426758, -0.015143820145612868, -0.016535815039113604, -0.01611350163485256, -0.01603586147994221, -0.016191023597649318, -0.015673182413705102], [-0.016700857633048308, -0.017051706885756718, -0.016395162126784154, -0.016864165985049667, -0.01667278712452, -0.016023236569300325, -0.015936447644162688, -0.01626053315184134, -0.016666644977778797, -0.01651990276982608, -0.01690611112853018, -0.016570014742366936, -0.016014494913507715, -0.016334286074074115, -0.01621235686701924, -0.01653022812336152, -0.01583634924223019, -0.016281303974484927, -0.01653990312391212, -0.015384206653677268], [-0.016471441301573585, -0.01647096314202187, -0.016715886966535524, -0.015878302888681167, -0.016818970876684446, -0.016713152489800882, -0.0154648252478201, -0.016328530500277577, -0.015836781582585016, -0.01591923201699931, -0.016315094505816256, -0.015951841421804724, -0.01608430179945204, -0.015957272458344565, -0.015751249520465478, -0.016350306857141315, -0.015517909552404317, -0.015884662571158274, -0.016211720964471307, -0.01537858018482844], [-0.01674440523726064, -0.016870567772511377, -0.016213148874409115, -0.016888734754126403, -0.017090609693170035, -0.01659256562080198, -0.01625635717081822, -0.016107107745803876, -0.016234190134722645, -0.016577197956586683, -0.01658670958631228, -0.016563728816596346, -0.016688515093891267, -0.016736196160361996, -0.015994597797780702, -0.016061666241292242, -0.015206770358209283, -0.01656914278587982, -0.01606315534154764, -0.015681866815853374], [-0.016944331036564515, -0.017205260427342613, -0.01677120483170293, -0.016402843466637763, -0.01674116281665193, -0.016423395631415146, -0.01525500299962603, -0.01627542397053335, -0.016664853908603776, -0.01620332976021642, -0.015950564835878013, -0.01610107356411497, -0.016396683154864377, -0.015976631236977498, -0.015478300298060717, -0.015835627632208554, -0.01604600189786053, -0.015850180758366084, -0.01603596051783181, -0.015769623989901102], [-0.016857923835780924, -0.016573198672727902, -0.016660307411618773, -0.016198760579099178, -0.016151481374992453, -0.01623511193332007, -0.015818969815924802, -0.01644510963983431, -0.015972042272190907, -0.01666642359581892, -0.01666443700190194, -0.016438254918363447, -0.016138118663893655, -0.015691974269895034, -0.016587077315345165, -0.015965118060360686, -0.015699839910512218, -0.01561194620613338, -0.016186792034230305, -0.016197922335520733], [-0.016756662992071368, -0.017021980605505502, -0.01671540550240299, -0.016161860765568574, -0.016256637402529132, -0.01604906368842445, -0.016092507257301394, -0.01617438393323743, -0.016105543848009572, -0.016246592326198385, -0.016142744624025374, -0.016159689527728567, -0.016177575339496836, -0.015961391152738445, -0.015789242903564853, -0.016290502978789936, -0.01590902706214275, -0.016035878036151207, -0.0163699057102928, -0.016166856731619543], [-0.016230743921604517, -0.01699457586491366, -0.01691575006710251, -0.01691567874763252, -0.016632348348462205, -0.01564006866069024, -0.015669555325846102, -0.01675726036853814, -0.015659388136628594, -0.01633203630678029, -0.016275904140963263, -0.01599466989252362, -0.01670183436780044, -0.016544315654085533, -0.015882735536646285, -0.01634814491721433, -0.015693511174422668, -0.015857069610244905, -0.015293298228102974, -0.01570879180052374], [-0.016746550537387085, -0.016635756849929545, -0.01704192789682773, -0.01592942336549498, -0.016565335498658518, -0.016559981627150607, -0.016370390094235444, -0.016204117687222342, -0.01636993721064581, -0.016019023809705737, -0.01624713908528634, -0.01653713290533686, -0.01654191191022731, -0.015871787270804183, -0.016600435605206076, -0.016053794928515903, -0.015786397557799592, -0.016167422435048453, -0.016149009764007245, -0.015779827376486453], [-0.017141787830569893, -0.01685604196926299, -0.016770676218784503, -0.01657265724540346, -0.016973351148096293, -0.016347677914333066, -0.015700463473615457, -0.0157292679709582, -0.016282549721629708, -0.015799962485816943, -0.0169651499113691, -0.017005390716294616, -0.01616841590634147, -0.01579805772887789, -0.015884669429112312, -0.01687947774540062, -0.015546104827296667, -0.01606408203496036, -0.015764690031214893, -0.016077969368821936], [-0.01755128513645066, -0.016614441354853425, -0.01642295621649906, -0.016572002735089818, -0.016539344978417192, -0.01665672671509038, -0.01610564101766388, -0.0167710479608722, -0.01604147346071364, -0.015915051759660022, -0.01690954942974296, -0.01618215110656205, -0.01687103577661275, -0.015704550539293104, -0.01567934362211993, -0.015968805810754147, -0.01586985536309292, -0.015848872001954256, -0.015923479964089694, -0.015604572794266433], [-0.01700702905775247, -0.016405242404623068, -0.016957584669743626, -0.01649808356316003, -0.015831866505709048, -0.01650461850371917, -0.015987113078007254, -0.015834023912635466, -0.015505062044615166, -0.016233666617861173, -0.016028249584376462, -0.016292798595496677, -0.016811560188299345, -0.015802581883183398, -0.015195148613460024, -0.015765465657774175, -0.016294889918615045, -0.01647530657977607, -0.016354233471026363, -0.01618598563271133], [-0.016283357847285636, -0.01655641981831666, -0.016127059444156554, -0.016293855360523378, -0.01631947219897442, -0.016398508430939616, -0.0164960599809452, -0.01635229032278839, -0.016150072161158744, -0.01646190473964058, -0.016283962555137702, -0.01689040784367708, -0.016767163139998632, -0.016438000493173108, -0.015954956500429416, -0.016569056147695202, -0.016605504963760735, -0.015329313107534112, -0.01578842030659742, -0.015421959499234628], [-0.016479987599589248, -0.01644678482494596, -0.016512996052180717, -0.01623094473834884, -0.016604746810030113, -0.016230213519226107, -0.016359208382350467, -0.01609761921903255, -0.016464485575532387, -0.015985272322973462, -0.015774520381458212, -0.01632178510310122, -0.016823351362691343, -0.01643553466150876, -0.015434648968053383, -0.01640702032901096, -0.015639626970513753, -0.01608966370811705, -0.016018362361111357, -0.01607982188546427], [-0.016959739645157706, -0.016680901866661726, -0.015836205448559966, -0.016650560318028734, -0.015979362423611275, -0.015641297610719303, -0.015788746501915876, -0.016033508703118756, -0.01595573902096323, -0.016363948579213562, -0.016349864006002027, -0.016495398899173445, -0.016242648234899834, -0.016920033344786076, -0.016276181128461735, -0.016473741446416813, -0.015963577017676644, -0.015565621002678179, -0.01634988477510272, -0.016759987490697584], [-0.016465195958807775, -0.016666490625723715, -0.016658908615375, -0.01597417902764041, -0.016394946754303752, -0.016153528909152313, -0.016275277887248356, -0.016575820504070977, -0.016165440248126276, -0.0158334592734765, -0.016393067206609387, -0.016885479811953534, -0.016471593134372298, -0.017124297138208497, -0.01548599428740715, -0.016309544928836586, -0.015739577267293366, -0.016315386973421362, -0.016361118135948566, -0.016635949477566882], [-0.016680470580762462, -0.016967020008211, -0.017070403001069857, -0.015793158201855152, -0.01661718510493328, -0.01621301409151063, -0.015497330917384148, -0.016267684516616924, -0.015545683307124036, -0.01584462817622427, -0.016830529260392843, -0.016203294725707643, -0.016943290418910587, -0.015581438668509352, -0.015578492450734066, -0.01643368853494311, -0.016285119780950222, -0.015912568651561352, -0.015719368411857025, -0.015732642681635923], [-0.017056323385982973, -0.017071971641855074, -0.01624203196673346, -0.016577086084052214, -0.016198385464505236, -0.015959998936922397, -0.015388246890736087, -0.01690871560472578, -0.016520770777269024, -0.016719342780151844, -0.01589885976225658, -0.016316317143634285, -0.015927259253864068, -0.01613903479860508, -0.015938319643326725, -0.015996730877187566, -0.01552190097834432, -0.016279927776335308, -0.015995176436170485, -0.015804091652970826], [-0.017190435316337342, -0.016575163169333516, -0.01629659819256952, -0.016774256975583077, -0.015978440181354282, -0.016162892801179076, -0.01620143768882657, -0.016215940324925678, -0.016085616640623322, -0.01624795446292185, -0.015590279490139558, -0.016351775677783426, -0.01628162630120476, -0.016736583715483217, -0.015290607493835316, -0.01675006130238602, -0.016112399997689694, -0.016085396155956493, -0.01584495781031281, -0.016031709625742012], [-0.017226310157841672, -0.0164663033859778, -0.01638852606295136, -0.01642215259901681, -0.016566243818266997, -0.016484045986143257, -0.016452209817223822, -0.016464707609223313, -0.01598467645947642, -0.016476401570535384, -0.015529223129381136, -0.016802343788985992, -0.016417294815804, -0.016305476633183012, -0.015407470515554668, -0.01588918182788552, -0.015839354895906106, -0.016859219988342257, -0.016188952756112908, -0.015382351679335257], [-0.017044276140355946, -0.016525294382434108, -0.01600036800318285, -0.01692841042125611, -0.016063543400203904, -0.0167008216867912, -0.01583944304325613, -0.015982843969462788, -0.01610446772754332, -0.01650934416727942, -0.016660683575282727, -0.016326108469991264, -0.01614299940648814, -0.016050548764700443, -0.016131072933532012, -0.016315196635999143, -0.016225473554238007, -0.01551847935196565, -0.015874550726858914, -0.01566897000262655], [-0.016174756903461544, -0.01692999553661901, -0.01705167048362926, -0.01660949009366751, -0.016107419352032235, -0.016188509519945497, -0.015585853922651487, -0.01612262091090234, -0.016426426055949322, -0.01609822137272688, -0.016735004284984756, -0.016043599908818165, -0.016651804571551146, -0.01556136051538674, -0.015408827232157843, -0.015855874683892428, -0.015887023972496795, -0.01599811437353065, -0.015655637769778918, -0.015893480415302176], [-0.016396467105890343, -0.01690556505247584, -0.0163054855200399, -0.016446662941364928, -0.01622691165873451, -0.016690239637868323, -0.015785441074554568, -0.016620593981308673, -0.015765446409343138, -0.016270811628848948, -0.016094841434208293, -0.01632812303243944, -0.01619217328151394, -0.015836234359203484, -0.016074598803568225, -0.01532030760600064, -0.01657169575010852, -0.016393493124135967, -0.01597552762388542, -0.015565046037824628], [-0.016299520764774443, -0.016637551393085426, -0.016299287907039765, -0.01610813956937386, -0.016305200311999217, -0.016601228593523636, -0.016288899767132464, -0.016305235511310533, -0.016063090550620947, -0.01683118193989227, -0.015518909238992087, -0.01620458965118359, -0.01645647074542291, -0.015677575909554008, -0.015332584749786342, -0.016079840062543812, -0.016278322310175185, -0.01605786016548567, -0.01657700147769983, -0.01606751816440997], [-0.016441387384698882, -0.017325914631361444, -0.017225293509456174, -0.016118796157285526, -0.016362377734664042, -0.01516634537172325, -0.01608508664570788, -0.01572299536201756, -0.01616493137153105, -0.01621315960010322, -0.016750280429064943, -0.016228195768808316, -0.01653543568323192, -0.01645026349483051, -0.016050647149129828, -0.01642593239180811, -0.0161192309302286, -0.01629438826737352, -0.015557310160813994, -0.016021567325025916], [-0.01686693458295582, -0.016740786564424494, -0.01648453245605215, -0.01640092243822592, -0.01555424864442638, -0.01667099748425638, -0.016069415470156286, -0.01638225749592203, -0.01607630099787768, -0.01614344420814296, -0.016216929728619375, -0.016309670684273796, -0.015741358140653132, -0.015770999475234804, -0.01601963602183988, -0.01615265943136728, -0.016152653946118384, -0.01698528285009184, -0.015969420465915152, -0.01578449323306024], [-0.01598619419452168, -0.016362732490235912, -0.016433844312774552, -0.016357999277320685, -0.015969441982301692, -0.01621147526376268, -0.016085473373391473, -0.016306341052304336, -0.015855664982231947, -0.015900633884010838, -0.016902356755211914, -0.016434765274207237, -0.016180164153866673, -0.015973977144992546, -0.01589274164800459, -0.01640268056199417, -0.016415161422386984, -0.01617112040367598, -0.016354725082739732, -0.016206639631885546], [-0.016048964224847716, -0.016745007333129024, -0.017180534108641177, -0.016329775174222558, -0.016582289070660373, -0.016075138720435006, -0.016345162602564738, -0.016090296577092385, -0.016153752753705675, -0.016379459268123033, -0.016228628993078524, -0.016712275509199688, -0.015795168051192618, -0.015386431874568587, -0.01610093851445945, -0.01633598707495066, -0.015921284689633122, -0.016330315102764423, -0.015994974665173196, -0.015537812293197398]]
  in  "Channel":i32=4
  out "MCL Scan I":u64=2
  out "MCL Scanning":bool
  in  "Start MCL Scan":bool
  out "wait to reset values":bool
  in  "Tab Scan Settings":enum32{"Scan Settings", "MCL FPGA Loop Timing"}(tab)
  in  "Restart DMA? (MCL)":bool=TRUE caption="Restart DMA?"
  in  "Center Scan":bool=TRUE
  in  "Save Data (MCL)":bool=TRUE caption="Save Data"
  out "Relative Phase (MCL)":i16 caption="Relative Phase"
  in  "Initial Phase Adj. (MCL)":i16 caption="Initial Phase Adj."
  out "MCL Late Counter":u32
  in  "APD 1 AO Mult.":i16=1 min=1
  in  "APD 2 AO Mult.":i16=1 min=1
  in  "Tab Control 7":enum32{"Green FB Signals", "Slow MCL Scan"}(tab)
  out "Green FB Plot":dbl(graph)=-10.00030518509476
  out "GI Late Counter":u32
  out "GI relative phase":i16
  in  "Initial Phase Adjustment (GI)":i16=4
  out "Green FB Signals (V)":cluster{"Y":dbl, "X":dbl, "Sum":dbl}={"Y"=-0.999969482421875, "X"=1.0, "Sum"=-10.00030518509476}
  out "Relative phase (Green FB)":i16
  in  "Initial Phase Adjustment (Green FB)":i16=50
  in  "Current When FB OFF (%)":dbl=10.0 min=0.0 max=100.0 step=1.0
  in  "Green int current ON count adj":u32=150
  in  "Green FB Gains":T7={"proportional gain (Kc)"=10, "integral gain (Kc*Ts/Ti)"=5, "derivative gain (Kc*Td/Ts)"=0}
  in  "Green FB Setpoint (mV)":dbl=100.0
  in  "Initial Phase Adjustment (GI) 2":i16=-100
  out "GI relative phase 2":i16
  out "GI Late Counter 2":u32
  in  "Negate X signals":bool
  in  "Trap Position FIFO Depth":u32=300000 format="%.0p"
  out "Trap AI FIFO El. Rem.":u32 format="%.0p"
  out "Relative phase (AI1)":i16
  out "Late Counter (AI1)":u32
  in  "Initial Phase Adjustment (AI1)":i16=185
  in  "AI Count (ticks)":u32=200
  in  "Trap AI FIFO Depth":u32=340000 format="%.0p"
  in  "Detector Type":string(combo)="UCB Fleezers 052511"
  in  "FPGA Ave.":dbl=1.0 min=1.0 step=1.0
  out "Trap Pos FIFO El Remaining":u32=171
  out "Trap AI FIFO Timeout":u16
  out "Trap Pos FIFO Timeout":u16
  out "Waveform Chart":i32(graph)=320000
  in  "Lost Tether Alarm Threshold (pN)":dbl=0.5
  in  "AOM X Cal (nm/MHz)":dbl=174.0
  in  "MCL X Cal (nm/V)":dbl=1174.0
  out "X RF Amplitude Limits (%)":T9={"Minimum"=0.0, "Maximum"=75.0, "Increment"=1.0}
  out "Y RF Amplitude Limits (%)":T9={"Minimum"=0.0, "Maximum"=75.0, "Increment"=1.0}
  in  "Read Lateness and Rel Phase":bool
  out "Vec Mean of T1 T2":dbl[](array[numeric])=[1.039290883164312, 1.038787885614062]
  out "AI labels":string[](array[string])=["T1 Y", "T1 X", "T1 Sum", "T2 Y", "T2 X", "T2 Sum", "T1 FB X", "T2 FB Sum", "T2 FB X", "T2 FB Sum", "PSD Y", "PSD X", "PSD Sum"]
  in  "Save Trap Pos. Data":bool=TRUE
  out "Current MCL (V)":dbl=5.657514378627918
  in  "Tracking factor":dbl=-0.45
  # "Trap interlacing RF phase control\n\n0 = no phase control\n1 = offset increments each trap cycle by values below\n2 = offset increment increases by increment factor each cycle\n3 = random phase (no parameters set)"
  # "Save Positions of Cambers"
  # "Trap Display:"
  # "APD Display:"
  # "originally 10k"
  # "Data Saving"
  # "Trap Manipulation"
  # "DAQ"
  # "Central frequency 80 MHz"
  # "F9"
  # "F10"
  # "Bead Calibration"
  # "Current Location"
  # "Select the chamber to go to"
  # "F4"
  # "Press F12 to move stage\nwith the mouse. F12 to cancel."
  # "F5"
  # "F6"
  # "F7"
  # "F8"
  # "Harvard Pump\n(sample channel for flow exp)"
  # "Chemyx Pump 2"
  # "Units: \n1 = ml/m\n2 = ml/h\n3 = ul/m\n4 = ul/h"
  # "Rate param is ul/h\nVolume param is ul"
  # "Oscillate Set 2 freq. (debugging)"
  # "BD 1"
  # "BD 2"
  # "X"
  # "Y"
  # "AOD Raster Scan"
  # "Approx. trap separations"
  # "X"
  # "Y"
  # "DON'T TURN ON\nUNTIL YOU CLOSE\nTHE LOOP"
  # "FPGA\nreading"
  # "DMA\ntransfer"
  # "APD Gates"
  # "APD 2"
  # "APD 1"
  # "X"
  # "2D"
  # "Y"
  # "1D"
  # "Green FB Measurement"
  # "Green Laser Interlacing"
  # "Digital Gate"
  # "Current Analog Control"
  # "was 87"
  # "originally 600k"
  # "Total AI Rates (NOT rates/trap)"
  # "originally 20k"
  # "(Samples/trap x Trap Sets)"
  # "(Samples/channel x\n8 if averaging (8 channels)\n4 if no averaging)"
  # "Trap 1"
  # "Trap 2"
  # "Flour./Trap 3"
  # "External Video Window"
  # "MCL Position Debugging"
  # "Temporary Control Storage\n(these used to be somewhere else, still want to keep them)"
  # "Y"
  # "X"
  # "Trap Position Difference Limits"
  # "Joystick Control"
  # "Setting Limit for the z-axis"
  # "Errors detected in determing Current Location"
  # "High Jog Velocity"
  # "Low Jog Velocity"
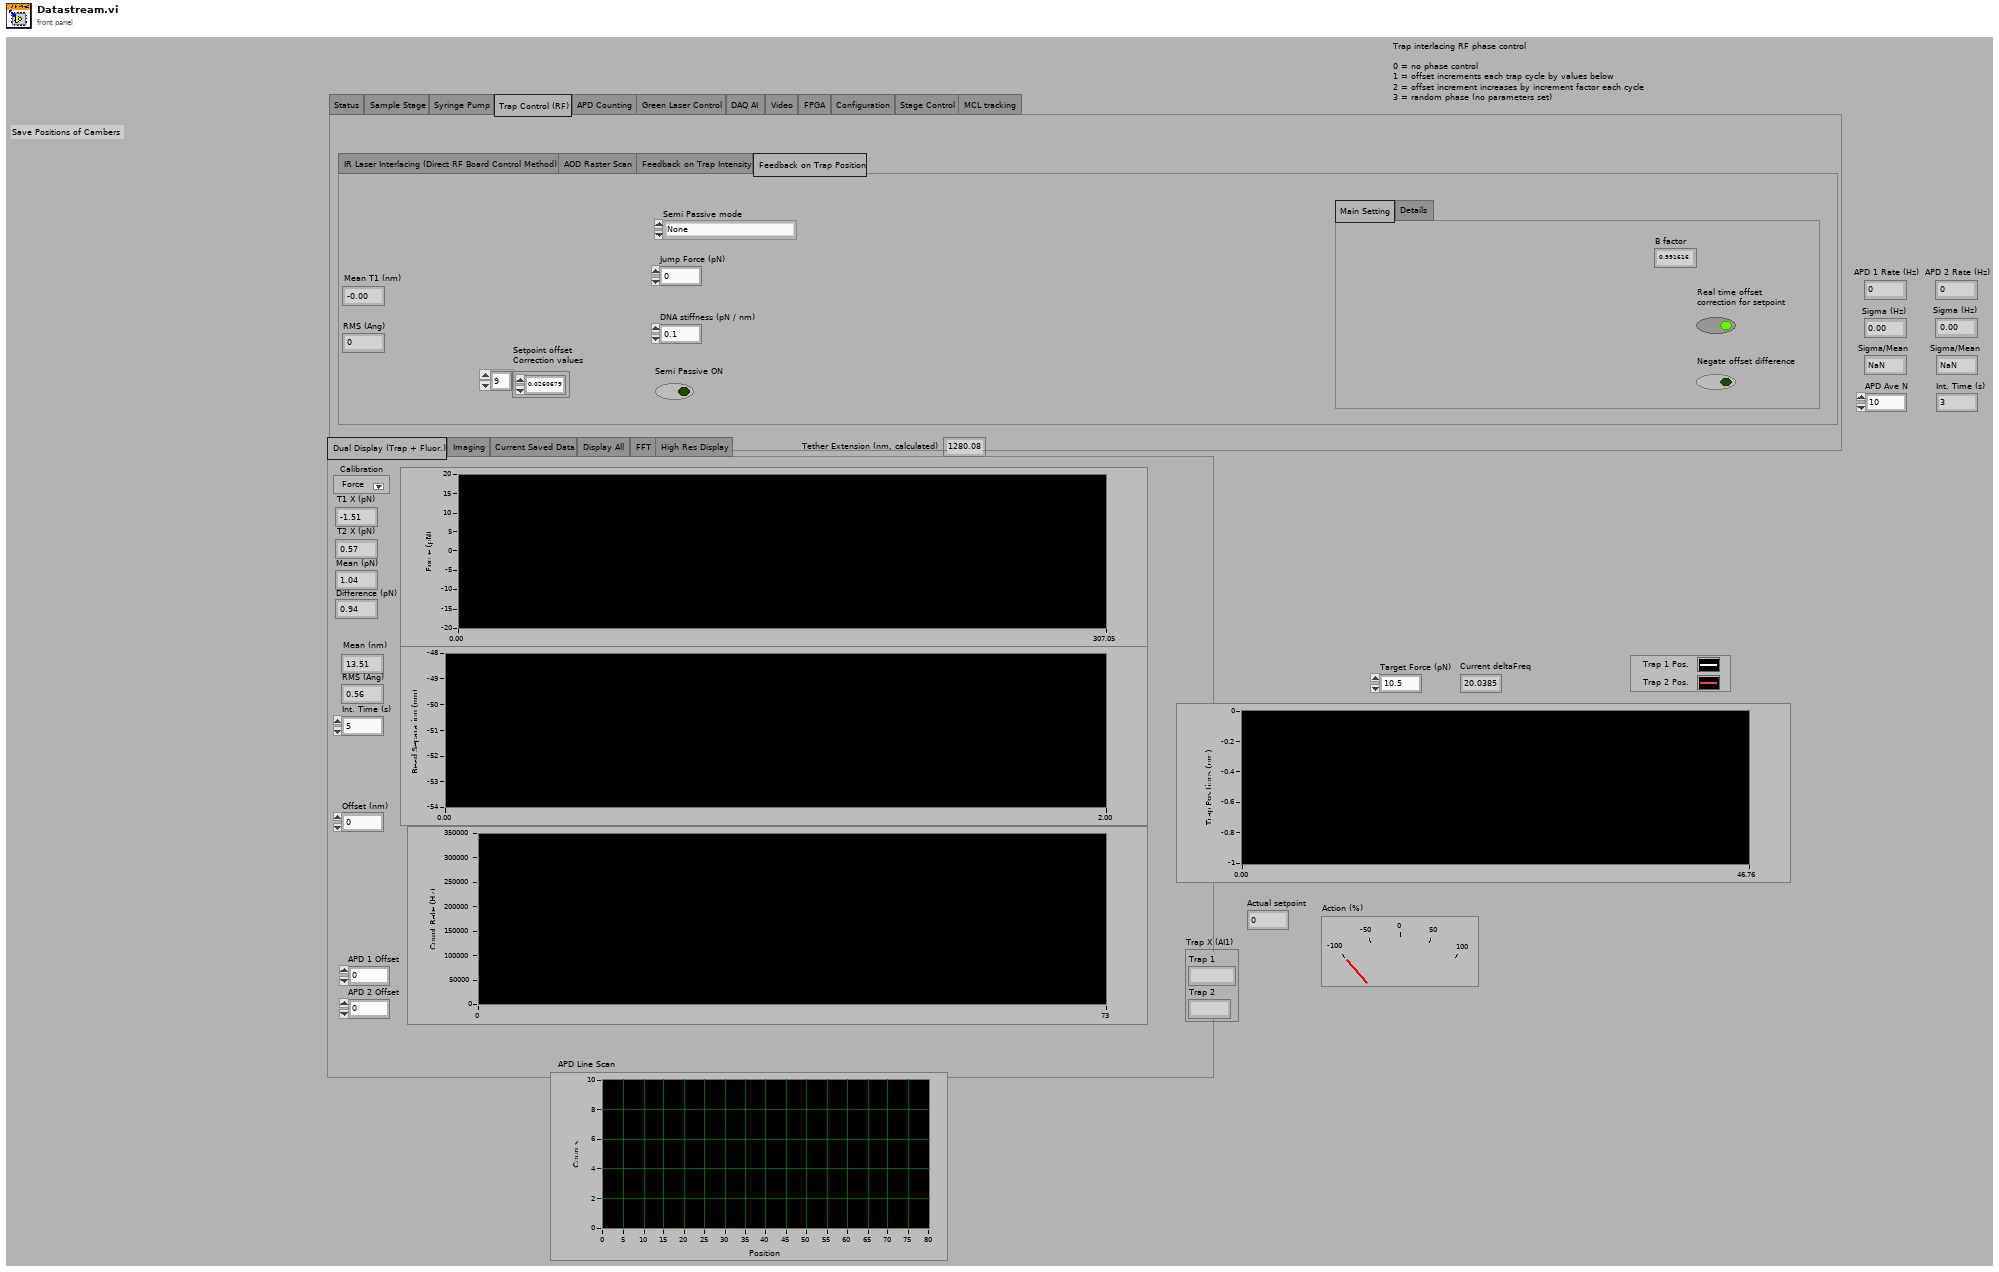
[diagram p1: front panel]
types:
  T1 = cluster{"Trap 1":fxp<+/-,16,1>, "Trap 2":fxp<+/-,16,1>}
  T2 = enum32{"Dual Display (Trap + Fluor.)", "Imaging", "Current Saved Data", "Display All", "FFT", "High Res Display"}
  T3 = typedef "IMAQ Image.ctl" = refnum<image>
  T4 = enum32{"Status", "Sample Stage", "Syringe Pump", "Trap Control (RF)", "APD Counting", "Green Laser Control", "DAQ AI", "Video", "FPGA", "Configuration", "Stage Control", "MCL tracking"}
  T5 = cluster{"Pump 1":cluster{"Diameter (mm)":dbl, "Units":dbl, "Volume":dbl, "Rate":dbl}, "Pump 2":cluster{"Diameter (mm)":dbl, "Units":dbl, "Volume":dbl, "Rate":dbl}, "Pump 3":cluster{"Diameter (mm)":dbl, "Units":dbl, "Volume":dbl, "Rate":dbl}}
  T6 = enum32{"IR Laser Interlacing (Direct RF Board Control Method)", "AOD Raster Scan", "Feedback on Trap Intensity", "Feedback on Trap Position"}
  T7 = cluster{"proportional gain (Kc)":i16, "integral gain (Kc*Ts/Ti)":i16, "derivative gain (Kc*Td/Ts)":i16}
  T8 = cluster{"Set 1":fxp<+/-,16,1>, "Set 2":fxp<+/-,16,1>}
  T9 = typedef "LVMinMaxIncTypeDef.ctl" = cluster{"Minimum":dbl, "Maximum":dbl, "Increment":dbl}
  T10 = typedef "Image Type" = u32
  T11 = typedef "nirio_resource_hc.ctl" = tag
  T12 = typedef "openfpgaref.initrf.ctl" = refnum<k20>
  T13 = typedef "openfpgaref.8.6.ctl" = refnum<k20>
  T14 = enum16{"CONNECT", "INITIALIZE VALVES", "DISCONNECT", "MOVE VALVE"}
  T15 = typedef "XDNodeRunTimeDep.lvlib/timing_clust.ctl" = cluster{"Expected End [f-1]":u64, "Actual End [f-1]":u64, "Finished Late? [f-1]":bool, "Expected End [i-1]":u64, "Actual End [i-1]":u64, "Finished Late? [i-1]":bool, "Expected Start [i]":u64, "Actual Start [i]":u64, "Expected Start [f]":u64, "Actual Start [f]":u64, "Source Name":string, "Structure Name":string, "Period":i64, "Deadline":i64, "Offset":i64, "Start":i64, "Priority":i32, "Timeout":i32, "Mode":T16, "Wakeup Reason":T17, "Error":errorcluster, "Source Type":string, "Secondary Source Type":string, "Global End Time":u64, "Global Start Time":u64, "Frame Duration":u64, "Iteration Duration":u64, "Assigned CPU":i32, "I/O Scan Engine Mode":u32}
  T16 = typedef "XDNodeRunTimeDep.lvlib/nitl_modes.ctl" = enum32{"No Change", "Process missed periods, maintain original phase", "Discard missed periods, maintain original phase", "Process missed periods, ignore original phase", "Discard missed periods, ignore original phase"}
  T17 = typedef "XDNodeRunTimeDep.lvlib/wakeup.ctl" = enum32{"Normal", "Aborted", "Asynchronous wakeup", "Timing source error", "Timed loop error", "Timeout"}
  T18 = cluster{"New Image":T3, "New Image":T3, "New Image":T3, "New Image":T3}
  T19 = enum32{"Normal Display", "Dual Display (APD)", "FFT", "High Res Display"}
  T20 = cluster{"Origin Pixel":cluster{"X":sgl, "Y":sgl}, "Angle Relative to Horizontal (deg)":sgl, "Axis Reference":u32}
  T21 = typedef "Simple Grid Descriptor" = cluster{"X Step":sgl, "Y Step":sgl, "Unit":T22}
  T22 = typedef "Image Unit" = enum32{"Undefined", "Angström", "Micrometer", "Millimeter", "Centimeter", "Meter", "Kilometer", "Microinch", "Inch", "Feet", "Nautical miles", "Standard miles", "Steps"}
  T23 = cluster{"averaging mode":u16, "weighting mode":u16, "number of averages":u32}
  T24 = cluster{"dB On (F)":bool, "unwrap phase (F)":bool, "convert to degree (F)":bool}
  T25 = enum16{"open", "replace", "create", "open or create", "replace or create", "replace or create with confirmation"}
  T26 = enum16{"big-endian, network order", "native, host order", "little-endian"}
  T27 = cluster{string, string, string, string, string, string, string, string}
  T28 = cluster{string, string, string, string, string, string, string, string, string, string, string, string}
  T29 = cluster{string, string, string, string, string, string, string, string, string, string, string, string, string}
  T30 = cluster{string, string, string, string, string, string, string, string, string, string, string, string, string, string}
  T31 = cluster{"f0":dbl, "df":dbl, "magnitude":dbl[]}[][]
  T32 = cluster{"Green FB Ch 0":i16, "Green FB Ch 1":i16, "Green FB Ch 2":i16}
  T33 = cluster{"Green FB Ch 0":dbl, "Green FB Ch 1":dbl, "Green FB Ch 2":dbl}
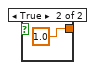
[diagram p4: hidden frame]
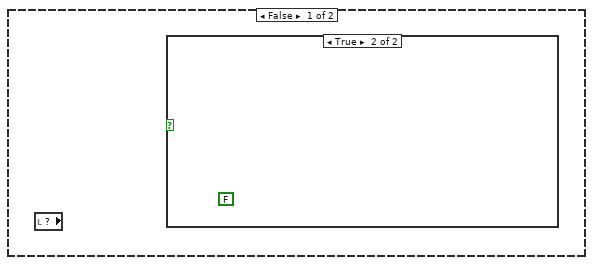
[diagram p7: hidden frame]
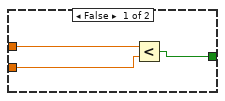
[diagram p10: hidden frame]
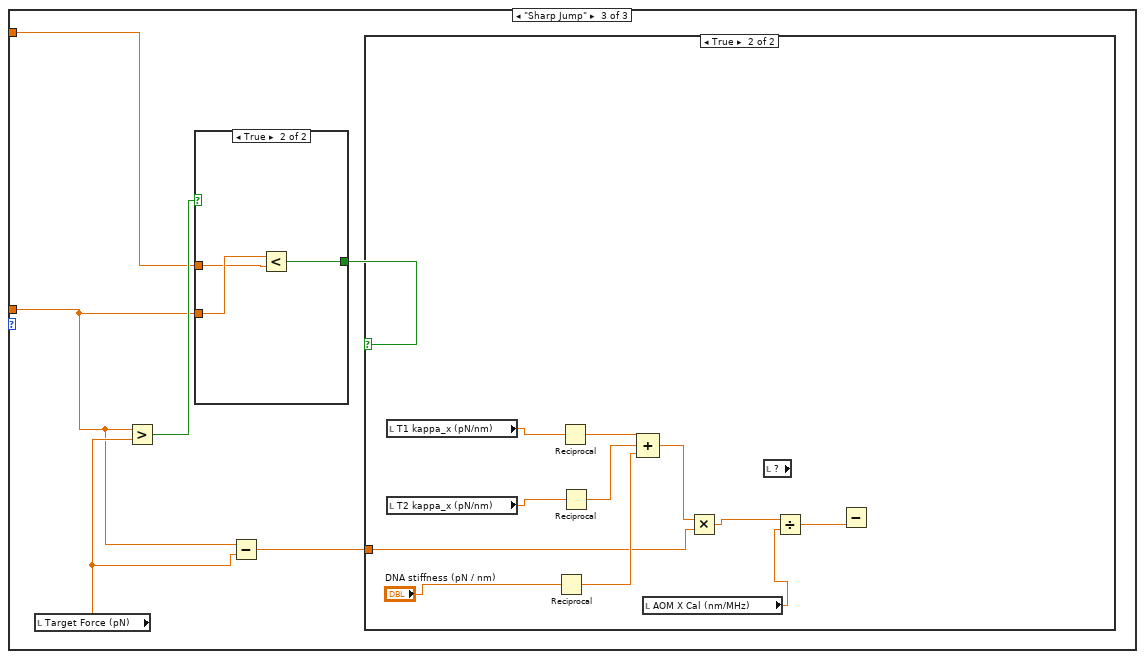
[diagram p11: hidden frame]
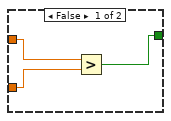
[diagram p13: hidden frame]
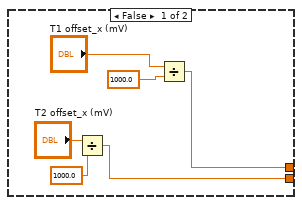
[diagram p14: hidden frame]
diagram:
  w87 = T9 {"Minimum"=60.0, "Maximum"=90.0, "Increment"=1.0}  # Bd 2 Freq Limits (MHz)
  w86 = T9 {"Minimum"=0.0, "Maximum"=75.0, "Increment"=1.0}  # Bd 1 Amp Limits (%)
  w26 = T9 {"Minimum"=60.0, "Maximum"=90.0, "Increment"=1.0}  # Bd 1 Freq Limits (MHz)
  w88 = T9 {"Minimum"=0.0, "Maximum"=75.0, "Increment"=1.0}  # Bd 1 Amp Limits (%)
  w73 = enum32{"Laser ON", "Laser OFF", "Interlace"}."Laser OFF" ("Green laser mode")
  w20 = 48
  w23 = 1000000.0
  (unwired) 3 ("Processor")
  w57 = T10 2 items=["Grayscale (U8)", "Grayscale (I16)", "Grayscale (SGL)", "Complex (CSG)", "RGB (U32)", "HSL (U32)", "RGB (U64)", "Grayscale (U16)"] ("Image Type")
  w118 = 40000000.0  # 40MHz, the FPGA tick rate
  w132 = 10.0 ("y")
  w131 = 32767.0 ("y")
  w139 = 6.0  # clock mult.
  w140 = 49152000.0  # TCXO frequ.
  # "Set starting RF limits"
  n1 = flat-sequence {
    tunnel: [w159] -> w10
    tunnel: [w167] -> w1
    tunnel: [w168] -> w103
    tunnel: w10 -> [w174]
    frame #0 {
      w159 = T11 "RIO0" ("resource name")
      # "init. FPGA board, mostly to initialize the RF board"
      n2 = xnode "Open FPGA VI Reference"("resource name"=w159) -> ("FPGA VI Reference Out"=w166:T12)  [unwired: 1 in, 1 out]
      n3 = xnode "Invoke Method"("FPGA VI Reference In"=w166) -> ("FPGA VI Reference Out"=w165:T12, "error out"=w164:errorcluster)  [unwired: 1 in]
      n4 = xnode "Invoke Method"("FPGA VI Reference In"=w165, "error in"=w164) -> ("FPGA VI Reference Out"=w162:T12, "error out"=w163:errorcluster)  [unwired: 1 in]
      n5 = call "Initialize RF boards - with FPGA init only vi v1.vi"("error in"=w163, "FPGA Interface"=w162) -> ("error out"=w160:errorcluster, "FPGA Interface 2"=w161:T12)
      n6 = xnode "Close FPGA VI Reference"("FPGA VI Reference In"=w161, "error in"=w160) -> ()  [unwired: 1 out]
    }
    frame #1 {
      w169 = TRUE
      # "run FPGA VI"
      n7 = xnode "Open FPGA VI Reference"("resource name"=w174) -> ("FPGA VI Reference Out"=w173:T13, "error out"=w172:errorcluster)  [unwired: 1 in]
      n8 = xnode "Invoke Method"("FPGA VI Reference In"=w173, "error in"=w172) -> ("FPGA VI Reference Out"=w171:T13, "error out"=w170:errorcluster)
      n9 = xnode "Read/Write Control"("FPGA VI Reference In"=w171, "error in"=w170, "PMODE"=w169, "RD"=w169) -> ("FPGA VI Reference Out"=w167:T13, "error out"=w168:errorcluster)
    }
  }
  n10 = To Unsigned Byte Integer() -> (unsigned 8bit integer=w81:u8)  [unwired: 1 in]
  n11 = Build Array("DIO count 1 (ticks)", "DIO count 2 (ticks)", "DIO count 3 (ticks)") -> (w83:u32[])
  n12 = Split 1D Array(array=w83) -> (first subarray=w85:u32[])  [unwired: 1 in, 1 out]
  n13 = Index Array(array=w83, index=w81) -> (element=w82:u32)
  n14 = Multiply(x="APD Integration Time (s)", y=40000000.0) -> (x*y=w94:dbl)
  n15 = Reciprocal(x="APD Integration Time (s)") -> ()  [unwired: 1 out]
  n16 = Add Array Elements(numeric array=w85) -> (sum=w84:u32)
  n17 = To Unsigned Long Integer(number=w94) -> (unsigned 32bit integer=w93:u32)
  "APD Int. Count" <- w93
  n18 = local read item#-1() -> ()  [unwired: 1 out]
  n19 = local read item#-1() -> ()  [unwired: 1 out]
  n20 = local read item#-1() -> ()  [unwired: 1 in]
  n21 = local read item#-1() -> ()  [unwired: 1 out]
  n22 = local read item#-1() -> ()  [unwired: 1 out]
  n23 = Select(t=w84, f=w82) -> ()  [unwired: 1 in, 1 out]
  n24 = local read item#-1() -> ()  [unwired: 1 out]
  n25 = Multiply(y=w131) -> (x*y=w128:dbl)  [unwired: 1 in]
  n26 = Multiply(y=w131) -> (x*y=w130:dbl)  [unwired: 1 in]
  n27 = local read item#-1() -> ()  [unwired: 1 out]
  n28 = local read item#-1() -> ()  [unwired: 1 out]
  n29 = Divide(x=w128, y=w132) -> (x/y=w127:dbl)
  n30 = Divide(x=w130, y=w132) -> (x/y=w129:dbl)
  n31 = local write "Trap Pos FIFO Timeout"(u16 0 ("Trap Pos FIFO Timeout")) -> ()
  n32 = local read item#-1() -> ()  [unwired: 1 out]
  n33 = local read item#-1() -> ()  [unwired: 1 out]
  n34 = To Word Integer(number=w127) -> (16bit integer=w126:i16)
  n35 = To Word Integer(number=w129) -> (16bit integer=w125:i16)
  n36 = Not() -> (.not. x?=w119:bool)  [unwired: 1 in]
  n37 = local read item#-1() -> ()  [unwired: 1 in]
  n38 = local read item#-1() -> ()  [unwired: 1 in]
  n39 = Multiply(y=1000.0) -> (x*y=w142:dbl)  [unwired: 1 in]
  n40 = local read item#-1() -> ()  [unwired: 1 out]
  n41 = local read item#-1() -> ()  [unwired: 1 out]
  n42 = local read item#-1() -> ()  [unwired: 1 out]
  n43 = local read item#-1() -> ()  [unwired: 1 out]
  n44 = local read item#-1() -> ()  [unwired: 1 out]
  n45 = Scale By Power Of 2(n=48, x=w142) -> (x*2^n=w143:dbl)
  n46 = local read item#-1() -> ()  [unwired: 1 out]
  n47 = local read item#-1() -> ()  [unwired: 1 out]
  n48 = local read item#-1() -> ()  [unwired: 1 out]
  n49 = Multiply(x=w140, y=w139) -> (x*y=w138:dbl)
  n50 = Divide(x=w143, y=w138) -> (x/y=w137:dbl)
  n51 = To Quad Integer(1:w137) -> (0:w135:i64)
  n52 = Multiply(y=32767.0) -> (x*y=w122:dbl)  [unwired: 1 in]
  n53 = local read item#-1() -> ()  [unwired: 1 out]
  n54 = local read item#-1() -> ()  [unwired: 1 out]
  n55 = Divide(x=w122, y=10.0) -> (x/y=w121:dbl)
  n56 = Multiply() -> (x*y=w134:dbl)  [unwired: 2 in]
  n57 = local read item#-1() -> ()  [unwired: 1 out]
  n58 = Multiply(x=3276.7) -> (x*y=w144:dbl)  [unwired: 1 in]
  n59 = local read item#-1() -> ()  [unwired: 1 out]
  n60 = To Word Integer(number=w121) -> (16bit integer=w120:i16)
  n61 = local read item#-1() -> ()  [unwired: 1 out]
  n62 = Multiply(x=w134, y=u64 2) -> ()  [unwired: 1 out]
  n63 = To Word Integer(number=w144) -> ()  [unwired: 1 out]
  n64 = local read item#-1() -> ()  [unwired: 1 out]
  n65 = Multiply() -> ()  [unwired: 2 in, 1 out]
  n66 = And() -> ()  [unwired: 2 in, 1 out]
  n67 = Divide() -> ()  [unwired: 2 in, 1 out]
  n68 = Unbundle By Name() -> ()  [unwired: 1 in, 2 out]
  n69 = Divide(x=w118, y="AI Count (ticks)") -> ()  [unwired: 1 out]
  n70 = local read item#-1() -> ()  [unwired: 1 out]
  n71 = Unbundle By Name() -> ()  [unwired: 1 in, 3 out]
  n72 = Unbundle By Name() -> ()  [unwired: 1 in, 2 out]
  n73 = local read item#-1() -> ()  [unwired: 1 out]
  n74 = local read item#-1() -> ()  [unwired: 1 in]
  n75 = Divide(y="FPGA Ave.") -> ()  [unwired: 1 in, 1 out]
  n76 = property on="AI Count (ticks)" class="DigNum (strict)"("Val(Sgnl)"="AI Count (ticks)") -> ()  [unwired: 2 in, 2 out]
  n77 = local read item#-1() -> ()  [unwired: 1 in]
  n78 = Reciprocal() -> ()  [unwired: 1 in, 1 out]
  n79 = local read item#-1() -> ()  [unwired: 1 out]
  n80 = local read item#-1() -> ()  [unwired: 1 in]
  n81 = local read item#-1() -> ()  [unwired: 1 in]
  n82 = local read item#-1() -> ()  [unwired: 1 in]
  n83 = local read item#-1() -> ()  [unwired: 1 in]
  n84 = xnode "Initialize FPGA settings (a mess)"("FPGA VI Reference In"=w1, "error in"=w103, "ai count"="AI Count (ticks)", "FB Gains"="PID gains", "FB output range"=cluster{"output high":i16, "output low":i16} {"output high"=3000, "output low"=0} ("FB output range 1"), "Scan freq.  increment"=w135, "AO1 (Y)"=w126, "AO2 (X)"=w125, "Scan freq.  increment (MCL)"=w120, "MCL Scan Axis"=w119, "BD 1 Delay (ticks)"="Freq switch delay", "Amp switch delay"="Amp switch delay", "Swap F1 and F2"="Swap F1 and F2", "APD Acq Rate Count"=w93, "APD to FIFO"=FALSE, "APD Gate Operating Mode"="APD Gate", "APD Gate ON Count"="APD Gate ON Count", "APD Gate OFF Count"="APD Gate OFF Count", "Invert APD Gate"="Invert APD Gate", "DIO count 1 (ticks)"="DIO count 1 (ticks)", "DIO count 2 (ticks)"="DIO count 2 (ticks)", "DIO count 3 (ticks)"="DIO count 3 (ticks)", "APD 1 AO scale factor"="APD 1 AO Mult.", "APD 2 AO scale factor"="APD 2 AO Mult.", "Next trap write delay (ticks)"="Next trap write delay (ticks)", "Phase offset method"="Phase offset method", "Phase Trap 1"="Phase increment trap 1", "RF phase reset before cycles"="RF phase reset before cycles", "Phase Trap 2"="Phase increment trap 2") -> ("FPGA VI Reference Out"=w75:T13, "error out"=w77:errorcluster)  [unwired: 25 in]
  n85 = Multiply(x="Current When FB OFF (%)", y=655.35) -> (x*y=w68:dbl)
  n86 = Multiply(x="Green FB Setpoint (mV)", y=3.2767) -> (x*y=w65:dbl)
  n87 = local read item#-1() -> ()  [unwired: 1 out]
  n88 = local read item#-1() -> ()  [unwired: 1 out]
  n89 = To Unsigned Word Integer(number=w68) -> (unsigned 16bit integer=w66:u16)
  n90 = local read item#-1() -> ()  [unwired: 1 out]
  n91 = local read item#-1() -> ()  [unwired: 1 out]
  n92 = To Word Integer(number=w65) -> (16bit integer=w63:i16)
  n93 = local read item#-1() -> ()  [unwired: 1 out]
  n94 = local read item#-1() -> ()  [unwired: 1 out]
  n95 = local read item#-1() -> ()  [unwired: 1 out]
  n96 = local read item#-1() -> ()  [unwired: 1 out]
  n97 = local read item#-1() -> ()  [unwired: 1 out]
  n98 = local read item#-1() -> ()  [unwired: 1 out]
  n99 = local read item#-1() -> ()  [unwired: 1 out]
  n100 = local read item#-1() -> ()  [unwired: 1 out]
  n101 = xnode "Initialize FPGA settings (cont.)"("FPGA VI Reference In"=w75, "error in"=w77, "Operating Mode 2"=w73, "Green FB Gains"="Green FB Gains", "Green FB Setpoint"=w63, "Current Out"=w66, "Green int current ON count adj"="Green int current ON count adj", "Operating Mode"=w73, "Force feedback"=FALSE, "Trap Pos to FIFO"=TRUE) -> ("FPGA VI Reference Out"=w74:T13, "error out"=w76:errorcluster)  [unwired: 16 in]
  n102 = xnode "Set QPD FIFO Depth"("FPGA VI Reference In"=w74, "error in"=w76, "Requested Depth"="Trap AI FIFO Depth") -> ("FPGA VI Reference Out"=w51:T13, "error out"=w50:errorcluster)  [unwired: 1 out]
  n103 = xnode "Set Position FIFO Depth"("FPGA VI Reference In"=w51, "error in"=w50, "Requested Depth"="Trap Position FIFO Depth") -> ("FPGA VI Reference Out"=w45:T13, "error out"=w44:errorcluster)  [unwired: 1 out]
  n104 = xnode "Invoke Method"("FPGA VI Reference In"=w45, "error in"=w44) -> ("FPGA VI Reference Out"=w33:T13, "error out"=w32:errorcluster)  [unwired: 1 in]
  n105 = flat-sequence "Initial FPGA Loop Relative Phase Adjustment, to store \"correct\" phases" {
    tunnel: w32 -> [w176]
    tunnel: w33 -> [w177]
    tunnel: [w177] -> w37
    tunnel: [w176] -> w36
    tunnel: [w189] -> w109
    tunnel: [w186] -> w107
    tunnel: w37 -> [w188]
    tunnel: w36 -> [w187]
    tunnel: w109 -> [w191]
    tunnel: [w192] -> w108
    tunnel: w107 -> [w192]
    tunnel: [w191] -> w106
    tunnel: w108 -> [w195]
    tunnel: w106 -> [w194]
    tunnel: [w197] -> w105
    tunnel: [w196] -> w104
    tunnel: [w199] -> w31
    tunnel: [w200] -> w34
    tunnel: w105 -> [w200]
    tunnel: w104 -> [w199]
    frame #0 {
      n106 = Wait (ms)(milliseconds to wait=u32 1000) -> ()  [unwired: 1 out]
    }
    frame #1 {
      n107 = xnode "Read/Write Control"("FPGA VI Reference In"=w188, "error in"=w187, "Phase count adjustment"="Initial Phase Adjustment (AI1)", "Phase count adjustment (GI)"="Initial Phase Adjustment (GI)", "Phase count adjustment (MCL)"="Initial Phase Adj. (MCL)", "Phase Count Adjustment (APD Acq)"="Initial Phase Adjustment (APD Acq)", "Phase count adjustment (APD 1 Gate)"="Initial Phase Adjustment (APD 1 Gate)", "Phase count adjustment (APD 2 Gate)"="Initial Phase Adjustment (APD 2 Gate)", "Phase count adjustment (Green FB)"="Initial Phase Adjustment (Green FB)", "Phase count adjustment (GI) 2"="Initial Phase Adjustment (GI) 2") -> ("FPGA VI Reference Out"=w186:T13, "error out"=w189:errorcluster)
    }
    frame #2 {
      n108 = Wait (ms)(milliseconds to wait=u32 1000) -> ()  [unwired: 1 out]
    }
    frame #3 {
      w193 = TRUE
      n109 = xnode "Read/Write Control"("FPGA VI Reference In"=w195, "error in"=w194, "+ phase"=w193, "+ phase (GI)"=w193, "+ phase (MCL)"=w193, "+ phase (APD Acq)"=w193, "+ phase (APD 1 Gate)"=w193, "+ phase (APD 2 Gate)"=w193, "+ phase (Green FB)"=w193, "+ phase (GI) 2"=w193) -> ("FPGA VI Reference Out"=w196:T13, "error out"=w197:errorcluster)
    }
    frame #4 {
      n110 = Wait (ms)(milliseconds to wait=u32 1000) -> ()  [unwired: 1 out]
    }
  }
  n111 = local read item#-1() -> ()  [unwired: 1 out]
  n112 = local read item#-1() -> ()  [unwired: 1 out]
  n113 = local read item#-1() -> ()  [unwired: 1 out]
  n114 = local read item#-1() -> ()  [unwired: 1 out]
  n115 = local read item#-1() -> ()  [unwired: 1 out]
  n116 = xnode "Final FPGA Phase Adjustment, to adjust on the fly"("FPGA VI Reference In"=w31, "error in"=w34, "Phase Count Adjustment (APD Acq)"="Phase Adj. (APD Acq)", "Phase count adjustment (APD 1 Gate)"="Phase Adj. (APD 1 Gate)", "Phase count adjustment (APD 2 Gate)"="Phase Adj. (APD 2 Gate)") -> ("FPGA VI Reference Out"=w8:T13, "error out"=w7:errorcluster)  [unwired: 5 in]
  n117 = Unbundle By Name(w26) -> ("Minimum"=w25:dbl, "Maximum"=w24:dbl)
  n118 = call "set RF board frequency - interlace.vi"("Board 2 Frequency Limits"=w87, "Board 1 Frequency Limits"=w26, "error in"=w7, "FPGA VI Reference In"=w8) -> ("error out"=w156:errorcluster, "FPGA VI Reference Out"=w157:T13)  [unwired: 6 in]
  n119 = Multiply(x=w25, y=w23) -> (x*y=w21:dbl)
  n120 = Multiply(x=w24, y=w23) -> (x*y=w22:dbl)
  n121 = Scale By Power Of 2(n=w20, x=w21) -> (x*2^n=w17:dbl)
  n122 = Scale By Power Of 2(n=w20, x=w22) -> (x*2^n=w16:dbl)
  n123 = Multiply(x=49152000.0, y=6.0) -> (x*y=w15:dbl)
  n124 = property on="BD 1 Amplitude 1 (%)" class="DigNum (strict)"("Data Range"=w88) -> ()  [unwired: 2 in, 2 out]
  n125 = property on="BD 1 Amplitude 2 (%)" class="DigNum (strict)"("Data Range"=w88) -> ()  [unwired: 2 in, 2 out]
  n126 = property on="BD 1 Amplitude 3 (%)" class="DigNum (strict)"("Data Range"=w88) -> ()  [unwired: 2 in, 2 out]
  n127 = Divide(x=w17, y=w15) -> (x/y=w14:dbl)
  n128 = Divide(x=w16, y=w15) -> (x/y=w13:dbl)
  n129 = To Unsigned Quad Integer(1:w14) -> (0:w12:u64)
  n130 = To Unsigned Quad Integer(1:w13) -> (0:w11:u64)
  n131 = xnode "Min/Max RF Bd Freq (FPGA units)"("FPGA VI Reference In"=w8, "FB Min frequency"=w12, "FB Max Frequency"=w11) -> ()  [unwired: 1 in, 2 out]
  n132 = property on="BD 2 Amplitude 1 (%)" class="DigNum (strict)"("Data Range"=w86) -> ()  [unwired: 2 in, 2 out]
  n133 = property on="BD 2 Amplitude 2 (%)" class="DigNum (strict)"("Data Range"=w86) -> ()  [unwired: 2 in, 2 out]
  n134 = property on="BD 2 Amplitude 3 (%)" class="DigNum (strict)"("Data Range"=w86) -> ()  [unwired: 2 in, 2 out]
  n135 = call "set RF board amplitude - interlace.vi"("Board 2 Amplitude Limits"=w86, "Board 1 Amplitude Limits"=w88, "error in"=w156, "FPGA VI Reference In"=w157, "Board 2 Amplitude 3 (%)"="BD 2 Amplitude 3 (%)", "Board 1 Amplitude 3 (%)"="BD 1 Amplitude 3 (%)", "Board 2 Amplitude 2 (%)"="BD 2 Amplitude 2 (%)", "Board 2 Amplitude 1 (%)"="BD 2 Amplitude 1 (%)", "Board 1 Amplitude 2 (%)"="BD 1 Amplitude 2 (%)", "Board 1 Amplitude 1 (%)"="BD 1 Amplitude 1 (%)") -> ("error out"=w29:errorcluster, "FPGA VI Reference Out"=w30:T13)
  n136 = flat-sequence "Trap, Fluidics Init." {
    tunnel: w30 -> [w202]
    tunnel: w29 -> [w201]
    tunnel: [w202] -> w149
    tunnel: [w201] -> w148
    tunnel: [w204] -> w147
    tunnel: w149 -> [w204]
    tunnel: [w203] -> w146
    tunnel: w148 -> [w203]
    tunnel: w147 -> [w207]
    tunnel: w146 -> [w206]
    tunnel: [w207] -> w28
    tunnel: [w206] -> w27
    tunnel: [w209] -> w42
    tunnel: [w213] -> w35
    tunnel: w28 -> [w213]
    tunnel: w27 -> [w208]
    frame #0 {
      (unwired) 1.0 ("Index")
      n137 = local read item#-1() -> ()  [unwired: 1 out]
      n138 = local read item#-1() -> ()  [unwired: 1 in]
    }
    frame #1 {
      n139 = Wait (ms)(milliseconds to wait=u32 50) -> ()  [unwired: 1 out]
      n140 = local read item#-1() -> ()  [unwired: 1 out]
    }
    frame #2 {
      n141 = local read item#-1() -> ()  [unwired: 1 out]
    }
    frame #3 {
      n142 = call "hamilton_controller.vi"("error in"=w208, "action"=T14."CONNECT") -> ("error out"=w210:errorcluster)  [unwired: 9 in]
      n143 = call "hamilton_controller.vi"("error in"=w210, "action"=T14."INITIALIZE VALVES") -> ("error out"=w209:errorcluster)  [unwired: 9 in]
    }
  }
  n144 = call "IMAQ Create"("Image Name"="APD 1 Image", "Image Type"=w57) -> ("New Image"=w56:T3)  [unwired: 3 in, 1 out]
  n145 = call "IMAQ Create"("Image Name"="APD 2 Image", "Image Type"=w57) -> ("New Image"=w55:T3)  [unwired: 3 in, 1 out]
  n146 = call "IMAQ Create"("Image Name"="Det. X Image", "Image Type"=w57) -> ("New Image"=w54:T3)  [unwired: 3 in, 1 out]
  n147 = call "IMAQ Create"("Image Name"="Det. Y Image", "Image Type"=w57) -> ("New Image"=w53:T3)  [unwired: 3 in, 1 out]
  n148 = node-c288(i64 1 ("Period"), 1 ("Processor")) -> (w115:T15)  [unwired: 2 out]
  n149 = Bundle("New Image"=w56, "New Image"=w55, "New Image"=w54, "New Image"=w53) -> (w52:T18)  [unwired: 1 in]
  n150 = timed-loop "Acquire Data" {
    tunnel: w35 -> [w500]
    tunnel: w42 -> [w499]
    tunnel: [w528] -> w39
    tunnel: [w522] -> w38
    timing: w115 -> [_]
    timing-out: [_] -> w114
    tunnel: w52 -> [w352]
    stop <- _ stop-if-true
    (unwired) u32 0 ("Number of Elements")
    w340 = "NI_ChannelName" ("name")
    n151 = node-c288() -> ()  [unwired: 2 out]
    n152 = First Call?() -> (First Call?: T/F=w306:bool)
    n153 = Or(x="Reset", y=w306) -> (x .or. y?=w307:bool)
    n154 = case "Check for reset" shown="True" w307 {
      tunnel: w500 -> [w631 w639]
      tunnel: w499 -> [w630 w638]
      tunnel: [w631 w633] -> w251
      tunnel: [w630 w632] -> w495
      frame False {
      }
      frame True {
        w636 = TRUE ("AI to FIFO")
        n155 = call "reset FPGA DMA.vi"("error in"=w638, "FPGA VI Reference In"=w639) -> ("error out"=w634:errorcluster, "FPGA VI Reference Out"=w635:T13)
        n156 = local write "Overflow (data lost)"(FALSE ("Overflow (data lost)")) -> ()
        n157 = xnode "Read/Write Control"("FPGA VI Reference In"=w635, "error in"=w634, "AI to FIFO"=w636, "APD to FIFO"=w636) -> ("FPGA VI Reference Out"=w633:T13, "error out"=w632:errorcluster)
      }
    }
    n158 = local read item#-1() -> ()  [unwired: 1 out]
    n159 = Or(x="Start AOD Scan", y="Trap Raster Scan") -> (x .or. y?=w454:bool)
    n160 = case "Start AOM raster scan" shown="True" w454 {
      tunnel: w251 -> [w1341 w1351]
      tunnel: w495 -> [w1340 w1350]
      tunnel: [w1341 w1345] -> w250
      tunnel: [w1340 w1344] -> w494
      frame False {
      }
      frame True {
        (unwired) TRUE ("Scanning...")
        n161 = case shown="True" "Restart DMA? (AOD)" {
          tunnel: [w1386 w1388] -> w1346
          tunnel: [w1385 w1387] -> w1347
          tunnel: w1351 -> [w1386 w1390]
          tunnel: w1350 -> [w1385 w1389]
          frame False {
          }
          frame True {
            n162 = local write "Overflow (data lost)"(FALSE ("Overflow (data lost)")) -> ()
            n163 = call "reset FPGA DMA.vi"("error in"=w1389, "FPGA VI Reference In"=w1390) -> ("error out"=w1387:errorcluster, "FPGA VI Reference Out"=w1388:T13)
          }
        }
        n164 = local write "Trap Raster Scan"(FALSE ("Trap Raster Scan")) -> ()
        n165 = case shown="False" "Move MCL Also?" {
          tunnel: w1347 -> [w1355 w1380]
          tunnel: w1346 -> [w1356 w1381]
          tunnel: [w1354 w1384] -> w1345
          tunnel: [w1353 w1383] -> w1344
          tunnel: "Raster to target force?" -> [w1352 w1358]
          frame False {
            w1357 = TRUE ("AI to FIFO")
            n166 = xnode "Read/Write Control"("FPGA VI Reference In"=w1356, "error in"=w1355, "AI to FIFO"=w1357, "APD to FIFO"=w1357, "Start scan"=w1357, "Raster to target force"=w1352) -> ("FPGA VI Reference Out"=w1354:T13, "error out"=w1353:errorcluster)
          }
          frame True {
            w1377 = FALSE ("1D or 2D Scan?")
            w1382 = TRUE ("AI to FIFO")
            # "Count for MCL loop"
            # "N total cycles"
            # "N steps"
            # "V_int"
            n167 = local read item#-1() -> ()  [unwired: 1 out]
            n168 = Sign() -> (0:w1363:dbl)  [unwired: 1 in]
            n169 = Compound Arithmetic op=MULTIPLY("MCL Step Position Ratio", "MCL/AOM Scale Tweak") -> (w1366:dbl)  [unwired: 1 in]
            n170 = local read item#-1() -> ()  [unwired: 1 out]
            n171 = Negate(x=w1363) -> (-x=w1360:dbl)
            n172 = Multiply(x=w1360, y="MCL Step Increment (V_int)") -> (x*y=w1362:dbl)
            n173 = Divide(x=w1366, y="MCL X Cal (nm/V)") -> (x/y=w1372:dbl)
            n174 = Multiply(x=32767.0 ("y"), y=w1372) -> (x*y=w1376:dbl)
            n175 = Divide(x=w1376, y=10.0) -> (x/y=w1371:dbl)
            n176 = local read item#-1() -> ()  [unwired: 1 out]
            n177 = local read item#-1() -> ()  [unwired: 1 out]
            n178 = local read item#-1() -> ()  [unwired: 1 out]
            n179 = Divide(x=w1371, y="MCL Step Increment (V_int)") -> (x/y=w1369:dbl)
            n180 = Absolute Value(x=w1369) -> (abs(x)=w1359:dbl)
            n181 = Compound Arithmetic op=MULTIPLY() -> (w1370:dbl)  [unwired: 3 in]
            n182 = local write "wait to reset values"(w1382) -> ()
            n183 = local write "MCL Scanning"(w1382) -> ()
            n184 = Divide(x=w1370, y=w1359) -> (x/y=w1367:dbl)
            "MCL Count" <- w1367
            n185 = xnode "Read/Write Control"("FPGA VI Reference In"=w1381, "error in"=w1380, "Scan steps (MCL)"=w1359, "Cycles per step (MCL)"=u64 1, "Scan freq.  increment (MCL)"=w1362, "1D or 2D Scan?"=w1377, "MCL Scan Axis"=w1377, "Cont. Scan (MCL)"=w1377, "MCL count"=w1367) -> ("FPGA VI Reference Out"=w1379:T13, "error out"=w1378:errorcluster)  [unwired: 1 in]
            n186 = xnode "Read/Write Control"("FPGA VI Reference In"=w1379, "error in"=w1378, "AI to FIFO"=w1382, "APD to FIFO"=w1382, "Start scan"=w1382, "Start scan (MCL)"=w1382, "Raster to target force"=w1358) -> ("FPGA VI Reference Out"=w1384:T13, "error out"=w1383:errorcluster)
          }
        }
      }
    }
    n187 = And(x="Save scans", y=w454) -> (x .and. y?=w493:bool)
    n188 = Compound Arithmetic op=OR("Start MCL Scan", "Confocal Image", "Confocal Linescan") -> (w452:bool)
    n189 = And(x="Save Data (MCL)", y=w452) -> (x .and. y?=w492:bool)
    n190 = case "Start MCL raster scan" shown="True" w452 {
      tunnel: w250 -> [w907 w920]
      tunnel: w494 -> [w906 w919]
      tunnel: [w907 w915] -> w277
      tunnel: [w906 w914] -> w276
      tunnel: [FALSE w913] -> w479
      tunnel: "Start MCL Scan" -> [_ w910]
      tunnel: "Confocal Image" -> [_ w909]
      tunnel: "Confocal Linescan" -> [_ _]
      frame False {
      }
      frame True {
        w913 = TRUE
        n191 = case shown="True" "Restart DMA? (MCL)" {
          tunnel: [w956 w958] -> w918
          tunnel: [w955 w957] -> w917
          tunnel: w920 -> [w956 w961]
          tunnel: w919 -> [w955 w960]
          frame False {
          }
          frame True {
            n192 = call "reset FPGA DMA.vi"("error in"=w960, "FPGA VI Reference In"=w961) -> ("error out"=w957:errorcluster, "FPGA VI Reference Out"=w958:T13)
            n193 = local write "Overflow (data lost)"(FALSE ("Overflow (data lost)")) -> ()
          }
        }
        n194 = case shown="False" w910 {
          selector: w910 -> [_ w924]
          tunnel: w909 -> [w923 _]
          tunnel: [w923 w924] -> w908
          frame False {
            n195 = property on="Confocal Image" class="Bool (strict)"("Value"=FALSE ("Start Confocal Map")) -> ()  [unwired: 2 in, 2 out]
          }
          frame True {
          }
        }
        n196 = local write "MCL Scanning"(w913) -> ()
        n197 = local read item#-1() -> (w912)
        n198 = local read item#-1() -> (w911)
        n199 = case shown="True" "Center Scan" {
          tunnel: w918 -> [w929 w954]
          tunnel: w917 -> [w928 w953]
          tunnel: [w927 w952] -> w915
          tunnel: [w926 w951] -> w914
          tunnel: [_ w941] -> _
          tunnel: [_ w940] -> _
          tunnel: w912 -> [_ _]
          tunnel: w911 -> [_ _]
          tunnel: w908 -> [_ _]
          frame False {
            w925 = TRUE ("AI to FIFO")
            n200 = xnode "Read/Write Control"("FPGA VI Reference In"=w929, "error in"=w928, "AI to FIFO"=w925, "APD to FIFO"=w925, "Start scan (MCL)"=w925) -> ("FPGA VI Reference Out"=w927:T13, "error out"=w926:errorcluster)
          }
          frame True {
            w950 = TRUE ("AI to FIFO")
            n201 = local read item#-1() -> ()  [unwired: 1 out]
            n202 = local read item#-1() -> ()  [unwired: 1 out]
            n203 = local read item#-1() -> ()  [unwired: 1 out]
            n204 = local read item#-1() -> ()  [unwired: 1 out]
            n205 = Decrement() -> (x-1=w931:dbl)  [unwired: 1 in]
            n206 = Decrement() -> (x-1=w933:dbl)  [unwired: 1 in]
            n207 = Multiply(y=w931) -> (x*y=w930:dbl)  [unwired: 1 in]
            n208 = Divide(x=w930, y=2.0) -> (x/y=w937:dbl)
            n209 = Multiply(y=w933) -> (x*y=w932:dbl)  [unwired: 1 in]
            n210 = Divide(x=w932, y=2.0) -> (x/y=w936:dbl)
            n211 = Select(t=w936, f=w937) -> (s? t:f=w935:dbl)  [unwired: 1 in]
            n212 = Select(t=w937, f=w936) -> (s? t:f=w939:dbl)  [unwired: 1 in]
            n213 = Subtract(y=w939) -> (x-y=w938:dbl)  [unwired: 1 in]
            n214 = Subtract(y=w935) -> (x-y=w934:dbl)  [unwired: 1 in]
            n215 = Not() -> (.not. x?=w945:bool)  [unwired: 1 in]
            n216 = Not() -> (.not. x?=w946:bool)  [unwired: 1 in]
            n217 = local read item#-1() -> ()  [unwired: 1 out]
            n218 = And(y=w946) -> (x .and. y?=w947:bool)  [unwired: 1 in]
            n219 = And(x=w946, y=w945) -> (x .and. y?=w948:bool)
            n220 = Select(s=w948, f=w934) -> (s? t:f=w940:dbl)  [unwired: 1 in]
            n221 = Select(s=w947, f=w938) -> (s? t:f=w941:dbl)  [unwired: 1 in]
            n222 = call "Volt to I16.vi"("Voltage In"=w941) -> ("I16 Voltage Out"=w944:i16)
            n223 = call "Volt to I16.vi"("Voltage In"=w940) -> ("I16 Voltage Out"=w943:i16)
            n224 = xnode "Read/Write Control"("FPGA VI Reference In"=w954, "error in"=w953, "AI to FIFO"=w950, "APD to FIFO"=w950, "Start scan (MCL)"=w950, "AO1 (Y)"=w944, "AO2 (X)"=w943) -> ("FPGA VI Reference Out"=w952:T13, "error out"=w951:errorcluster)
          }
        }
        "wait to reset values" <- w913
      }
    }
    n225 = local read item#-1() -> ()  [unwired: 1 out]
    n226 = local read item#-1() -> ()  [unwired: 1 out]
    n227 = local read item#-1() -> ()  [unwired: 1 out]
    n228 = local read "Trap AI FIFO Depth"() -> (w537:u32)
    n229 = xnode "Invoke Method"("FPGA VI Reference In"=w277, "error in"=w276, "Timeout (ms)"=-1) -> ("Data"=w313:u16[], "Elements Remaining"=→"Trap Pos FIFO El Remaining":u32)  [unwired: 1 in, 2 out]
    n230 = xnode "Invoke Method"("FPGA VI Reference In"=w277, "error in"=w276, "Timeout (ms)"=-1 ("Timeout")) -> ("FPGA VI Reference Out"=w253:T13, "error out"=w278:errorcluster, "Data"=w275:i16[], "Elements Remaining"=w279:u32)  [unwired: 1 in]
    "Trap AI FIFO El. Rem." <- w279
    n231 = xnode "Get APD Data"("FPGA VI Reference In"=w277, "error in"=w276, "Timeout (ms)"=-1) -> ("Data"=w386:u32[], "Elements Remaining"=→"APD FIFO Elements Remaining":u32)  [unwired: 1 in, 2 out]
    n232 = Subtract(x=w537) -> (x-y=w536:u32)  [unwired: 1 in]
    n233 = Decimate 1D Array(w313) -> (w310:u16[], w312:u16[], w311:u16[])
    n234 = Divide(x=w279, y=w536) -> (x/y=w535:dbl)
    "Buffer Status" <- w535
    n235 = To Unsigned Long Integer(number=w310) -> (unsigned 32bit integer=w309:u32[])
    n236 = Join Numbers(hi=w312, lo=w311) -> ((hi.lo)=w308:u32[])
    n237 = Equal?(x=w535, y=1.0) -> (x = y?=w533:bool)
    n238 = Join Numbers(hi=w309, lo=w308) -> ((hi.lo)=w302:u64[])
    n239 = call "IR AOM word to freq - vec.vi"("Frequency Word In (double vec)"=w302) -> ("Frequency Out"=w348:dbl[])
    n240 = case "Alert buffer overflow" shown="True" w533 {
      frame False {
      }
      frame True {
        n241 = call <vilib>:"Beep.vi"() -> ()  [unwired: 3 in, 9 out]
        "Overflow (data lost)" <- TRUE ("Overflow (data lost)")
      }
    }
    n242 = Decimate 1D Array(w348) -> (w347:dbl[], w346:dbl[])
    n243 = Array Size(array=w275) -> (size(s)=→"Waveform Chart":i32)
    n244 = Build Array(w347, w346) -> (w345:dbl[][])
    n245 = local read item#-1() -> ()  [unwired: 1 out]
    n246 = case "Deinterlace trap data, average down PSD" shown="1, Default" {
      selector: _ -> [_ _]
      tunnel: w275 -> [w990 w1055]
      tunnel: [w987 w1052] -> w409
      tunnel: [w990 w1054] -> w305
      tunnel: "Detector Type" -> [w989 w1050]
      tunnel: [w988 w1053] -> w408
      tunnel: [w986 w1051] -> w511
      frame 1, Default {
        n247 = Divide(x=w990, y=3276.7) -> (x/y=w991:dbl[])
        n248 = Decimate 1D Array(w991) -> (w1000:dbl[], w999:dbl[], w998:dbl[], w997:dbl[], w996:dbl[], w995:dbl[], w994:dbl[], w993:dbl[])
        n249 = case shown="\"IR-QPD + PSD + FB-QPD position\"" w989 {
          tunnel: w1000 -> [w1024 w1049]
          tunnel: w999 -> [w1023 w1048]
          tunnel: w998 -> [w1008 w1026]
          tunnel: w997 -> [w1009 w1036]
          tunnel: w996 -> [w1022 w1047]
          tunnel: w995 -> [w1021 w1046]
          tunnel: w994 -> [w1005 w1027]
          tunnel: w993 -> [w1004 w1025]
          tunnel: [w1003 w1033] -> w988
          tunnel: [w1002 w1032] -> w987
          tunnel: [w1001 w1031] -> w986
          frame "IR-QPD + PSD + FB-QPD", Default {
            w1001 = 0  # Channel pattern
            n250 = Divide(x=w1024, y=w1009) -> (x/y=w1011:dbl[])
            n251 = Divide(x=w1023, y=w1009) -> (x/y=w1010:dbl[])
            n252 = Divide(x=w1022, y=w1005) -> (x/y=w1007:dbl[])
            n253 = Divide(x=w1021, y=w1004) -> (x/y=w1006:dbl[])
            n254 = Build Array(w1011, w1010, w1009, w1008, w1007, w1006, w1005, w1004) -> (w1002:dbl[][])
            n255 = Bundle("T1 Y", "T1 X", "T1 Sum", "FB Sum", "PSD Y", "PSD X", "PSD Y Sum", "PSD X Sum") -> (w1020:T27)  [unwired: 1 out]
            n256 = Cluster To Array(cluster=w1020) -> (array=w1003:string[])
          }
          frame "IR-QPD + PSD + FB-QPD position" {
            w1031 = 3  # Channel pattern
            n257 = Negate(x=w1027) -> (-x=w1028:dbl[])
            n258 = Divide(x=w1049, y=w1036) -> (x/y=w1038:dbl[])
            n259 = Divide(x=w1048, y=w1036) -> (x/y=w1037:dbl[])
            n260 = Divide(x=w1047, y=w1027) -> (x/y=w1035:dbl[])
            n261 = Divide(x=w1046, y=w1028) -> (x/y=w1034:dbl[])
            n262 = Build Array(w1038, w1037, w1036, w1025, w1026, w1035, w1034, w1027) -> (w1032:dbl[][])
            n263 = Bundle("T1 Y", "T1 X", "T1 Sum", "FB X", "FB Sum", "PSD Y", "PSD X", "PSD Y Sum") -> (w1045:T27)  [unwired: 1 out]
            n264 = Cluster To Array(cluster=w1045) -> (array=w1033:string[])
          }
        }
      }
      frame 2 {
        n265 = case shown="\"UCB Fleezers 052511\"" w1050 {
          tunnel: w1055 -> [w1117 w1184 w1223 w1323]
          tunnel: [w1056 w1176 w1219 w1254] -> w1054
          tunnel: [w1083 w1167 w1221 w1301] -> w1053
          tunnel: [w1082 w1131 w1212 w1268] -> w1052
          tunnel: [w1076 w1166 w1253 w1299] -> w1051
          frame "IR-QPD + PSD + FB-QPD", Default {
            w1076 = 1  # Channel pattern
            # "time average x2 the 4th signal and the 4 psd signals (detection laser)"
            # "deinterlace 3 signals from qpd"
            n266 = Decimate 1D Array(w1117) -> (w1116:i16[], w1115:i16[], w1081:i16[], w1114:i16[], w1104:i16[], w1102:i16[], w1101:i16[], w1099:i16[])
            n267 = call "downsample 1D array - double.vi"("Ave N"=2.0, "Array In"=w1104) -> ("Array Out"=w1103:dbl[])  [unwired: 1 out]
            n268 = call "downsample 1D array - double.vi"("Ave N"=2.0, "Array In"=w1099) -> ("Array Out"=w1098:dbl[])  [unwired: 1 out]
            n269 = call "downsample 1D array - double.vi"("Ave N"=2.0, "Array In"=w1101) -> ("Array Out"=w1100:dbl[])  [unwired: 1 out]
            n270 = call "downsample 1D array - double.vi"("Ave N"=2.0, "Array In"=w1102) -> ("Array Out"=w1084:dbl[])  [unwired: 1 out]
            n271 = Decimate 1D Array(w1116) -> (w1113:i16[], w1085:i16[])
            n272 = Decimate 1D Array(w1115) -> (w1112:i16[], w1110:i16[])
            n273 = Decimate 1D Array(w1114) -> (w1111:i16[], w1109:i16[])
            n274 = Decimate 1D Array(w1081) -> (w1080:i16[], w1079:i16[])
            n275 = Interleave 1D Arrays(w1113, w1112, w1111, w1085, w1110, w1109, w1080, w1079, w1103, w1084, w1100, w1098) -> (w1097:dbl[])
            n276 = To Word Integer(number=w1097) -> (16bit integer=w1056:i16[])
            n277 = Divide(x=w1097, y=3276.7) -> (x/y=w1096:dbl[])
            n278 = Decimate 1D Array(w1096) -> (w1095:dbl[], w1094:dbl[], w1093:dbl[], w1092:dbl[], w1091:dbl[], w1090:dbl[], w1078:dbl[], w1077:dbl[], w1089:dbl[], w1088:dbl[], w1087:dbl[], w1086:dbl[])
            n279 = Divide(x=w1095, y=w1093) -> (x/y=w1063:dbl[])
            n280 = Divide(x=w1094, y=w1093) -> (x/y=w1062:dbl[])
            n281 = Divide(x=w1092, y=w1090) -> (x/y=w1061:dbl[])
            n282 = Divide(x=w1091, y=w1090) -> (x/y=w1060:dbl[])
            n283 = Divide(x=w1089, y=w1087) -> (x/y=w1059:dbl[])
            n284 = Divide(x=w1088, y=w1086) -> (x/y=w1058:dbl[])
            n285 = Bundle("T1 Y", "T1 X", "T1 Sum", "T2 Y", "T2 X", "T2 Sum", "T1 FB Sum", "T2 FB Sum", "PSD Y", "PSD X", "PSD Y Sum", "PSD X Sum") -> (w1064:T28)  [unwired: 1 out]
            n286 = Build Array(w1063, w1062, w1093, w1061, w1060, w1090, w1078, w1077, w1059, w1058, w1087, w1086) -> (w1082:dbl[][])
            n287 = Cluster To Array(cluster=w1064) -> (array=w1083:string[])
          }
          frame "IR-QPD + PSD + FB-QPD X position" {
            w1166 = 2  # Channel pattern
            # "convert\nADC numbers\nto volts"
            # "time average x2 the 3 psd signals (detection laser)"
            # "deinterlace 3 signals from qpds"
            n288 = Decimate 1D Array(w1184) -> (w1183:i16[], w1182:i16[], w1119:i16[], w1120:i16[], w1129:i16[], w1126:i16[], w1123:i16[], w1154:i16[])
            n289 = Decimate 1D Array(w1183) -> (w1181:i16[], w1168:i16[])
            n290 = call "downsample 1D array - I16.vi"("Ave N"=2.0, "Array In"=w1129) -> ("Array Out"=w1127:i16[])  [unwired: 1 in]
            n291 = call "downsample 1D array - I16.vi"("Ave N"=2.0, "Array In"=w1126) -> ("Array Out"=w1124:i16[])  [unwired: 1 in]
            n292 = Decimate 1D Array(w1182) -> (w1180:i16[], w1178:i16[])
            n293 = Decimate 1D Array(w1120) -> (w1179:i16[], w1177:i16[])
            n294 = Decimate 1D Array(w1154) -> (w1153:i16[], w1151:i16[])
            n295 = Decimate 1D Array(w1119) -> (w1152:i16[], w1150:i16[])
            n296 = call "downsample 1D array - I16.vi"("Ave N"=2.0, "Array In"=w1123) -> ("Array Out"=w1121:i16[])  [unwired: 1 in]
            n297 = Interleave 1D Arrays(w1181, w1180, w1179, w1168, w1178, w1177, w1153, w1152, w1151, w1150, w1127, w1124, w1121) -> (w1176:i16[])
            n298 = Divide(x=w1176, y=3276.7) -> (x/y=w1175:dbl[])
            n299 = Decimate 1D Array(w1175) -> (w1174:dbl[], w1173:dbl[], w1172:dbl[], w1171:dbl[], w1170:dbl[], w1169:dbl[], w1142:dbl[], w1140:dbl[], w1139:dbl[], w1137:dbl[], w1136:dbl[], w1135:dbl[], w1132:dbl[])
            n300 = Divide(x=w1174, y=w1172) -> (x/y=w1158:dbl[])
            n301 = Divide(x=w1173, y=w1172) -> (x/y=w1157:dbl[])
            n302 = Divide(x=w1171, y=w1169) -> (x/y=w1156:dbl[])
            n303 = Divide(x=w1170, y=w1169) -> (x/y=w1155:dbl[])
            n304 = Divide(x=w1142, y=w1140) -> (x/y=w1141:dbl[])
            n305 = Divide(x=w1139, y=w1137) -> (x/y=w1138:dbl[])
            n306 = Divide(x=w1136, y=w1132) -> (x/y=w1134:dbl[])
            n307 = Negate(x=w1132) -> (-x=w1130:dbl[])
            n308 = Divide(x=w1135, y=w1130) -> (x/y=w1133:dbl[])
            n309 = Bundle("T1 Y", "T1 X", "T1 Sum", "T2 Y", "T2 X", "T2 Sum", "T1 FB X", "T1 FB Sum", "T2 FB X", "T2 FB Sum", "PSD Y", "PSD X", "PSD Y Sum") -> (w1159:T29)  [unwired: 1 out]
            n310 = Build Array(w1158, w1157, w1172, w1156, w1155, w1169, w1141, w1140, w1138, w1137, w1134, w1133, w1132) -> (w1131:dbl[][])
            n311 = Cluster To Array(cluster=w1159) -> (array=w1167:string[])
          }
          frame "UCB Fleezers 052511" {
            w1253 = 2  # Channel pattern
            n312 = Select(t=i16 -1, s="Negate X signals", f=i16 1) -> (s? t:f=w1193:i16)
            n313 = Decimate 1D Array(w1223) -> (w1194:i16[], w1195:i16[], w1206:i16[], w1222:i16[], w1191:i16[], w1189:i16[], w1187:i16[], w1203:i16[])
            n314 = Multiply(x=w1193, y=w1195) -> (x*y=w1192:i16[])
            n315 = Decimate 1D Array(w1194) -> (w1251:i16[], w1241:i16[])
            n316 = Decimate 1D Array(w1192) -> (w1250:i16[], w1249:i16[])
            n317 = Decimate 1D Array(w1206) -> (w1200:i16[], w1199:i16[])
            n318 = Decimate 1D Array(w1222) -> (w1205:i16[], w1204:i16[])
            n319 = Decimate 1D Array(w1189) -> (w1188:i16[])  [unwired: 1 out]
            n320 = Decimate 1D Array(w1203) -> (w1202:i16[], w1201:i16[])
            n321 = Decimate 1D Array(w1187) -> (w1186:i16[])  [unwired: 1 out]
            n322 = Decimate 1D Array(w1191) -> (w1190:i16[])  [unwired: 1 out]
            n323 = Interleave 1D Arrays(w1251, w1250, w1205, w1241, w1249, w1204, w1202, w1200, w1201, w1199, w1190, w1188, w1186) -> (w1219:i16[])
            n324 = Divide(x=w1219, y=3276.7) -> (x/y=w1248:dbl[])
            n325 = Decimate 1D Array(w1248) -> (w1247:dbl[], w1246:dbl[], w1245:dbl[], w1244:dbl[], w1243:dbl[], w1242:dbl[], w1218:dbl[], w1216:dbl[], w1215:dbl[], w1213:dbl[], w1211:dbl[], w1208:dbl[], w1209:dbl[])
            n326 = Divide(x=w1247, y=w1245) -> (x/y=w1228:dbl[])
            n327 = Divide(x=w1246, y=w1245) -> (x/y=w1227:dbl[])
            n328 = Divide(x=w1244, y=w1242) -> (x/y=w1226:dbl[])
            n329 = Divide(x=w1243, y=w1242) -> (x/y=w1225:dbl[])
            n330 = Divide(x=w1218, y=w1216) -> (x/y=w1217:dbl[])
            n331 = Divide(x=w1215, y=w1213) -> (x/y=w1214:dbl[])
            n332 = Divide(x=w1211, y=w1209) -> (x/y=w1210:dbl[])
            n333 = Divide(x=w1208, y=w1209) -> (x/y=w1207:dbl[])
            n334 = Build Array(w1228, w1227, w1245, w1226, w1225, w1242, w1217, w1216, w1214, w1213, w1210, w1207, w1209) -> (w1212:dbl[][])
            n335 = Bundle("T1 Y", "T1 X", "T1 Sum", "T2 Y", "T2 X", "T2 Sum", "T1 FB X", "T2 FB Sum", "T2 FB X", "T2 FB Sum", "PSD Y", "PSD X", "PSD Sum") -> (w1229:T29)  [unwired: 1 out]
            n336 = Cluster To Array(cluster=w1229) -> (array=w1221:string[])
          }
          frame "IR-QPD + PSD + FB-QPD XY positions" {
            w1299 = 4  # Channel pattern
            # "time average x2 the 3 psd signals (detection laser)"
            # "deinterlace 3 signals from qpds"
            n337 = Decimate 1D Array(w1323) -> (w1322:i16[], w1321:i16[], w1300:i16[], w1320:i16[], w1266:i16[], w1312:i16[], w1311:i16[], w1288:i16[])
            n338 = Decimate 1D Array "QPD Y"(w1322) -> (w1319:i16[], w1302:i16[])
            n339 = call "downsample 1D array - double.vi"("Ave N"=2.0, "Array In"=w1312) -> ("Array Out"=w1287:dbl[])  [unwired: 1 out]
            n340 = call "downsample 1D array - double.vi"("Ave N"=2.0, "Array In"=w1311) -> ("Array Out"=w1286:dbl[])  [unwired: 1 out]
            n341 = Decimate 1D Array "Feedback Sum"(w1300) -> (w1284:i16[], w1282:i16[])
            n342 = Decimate 1D Array "Feedback Y"(w1266) -> (w1265:i16[], w1264:i16[])
            n343 = Decimate 1D Array "Feedback X"(w1288) -> (w1285:i16[], w1283:i16[])
            n344 = Decimate 1D Array "QPD Sum"(w1320) -> (w1317:i16[], w1315:i16[])
            n345 = Decimate 1D Array "QPD X"(w1321) -> (w1318:i16[], w1316:i16[])
            n346 = Interleave 1D Arrays(w1319, w1318, w1317, w1302, w1316, w1315, w1265, w1285, w1284, w1264, w1283, w1282, w1287, w1286) -> (w1310:dbl[])
            n347 = To Word Integer(number=w1310) -> (16bit integer=w1254:i16[])
            n348 = Divide(x=w1310, y=3276.7) -> (x/y=w1309:dbl[])
            n349 = Decimate 1D Array(w1309) -> (w1308:dbl[], w1307:dbl[], w1306:dbl[], w1305:dbl[], w1304:dbl[], w1303:dbl[], w1261:dbl[], w1275:dbl[], w1259:dbl[], w1260:dbl[], w1273:dbl[], w1257:dbl[], w1271:dbl[], w1269:dbl[])
            n350 = Divide(x=w1308, y=w1306) -> (x/y=w1292:dbl[])
            n351 = Divide(x=w1307, y=w1306) -> (x/y=w1291:dbl[])
            n352 = Divide(x=w1305, y=w1303) -> (x/y=w1290:dbl[])
            n353 = Divide(x=w1304, y=w1303) -> (x/y=w1289:dbl[])
            n354 = Divide(x=w1261, y=w1259) -> (x/y=w1258:dbl[])
            n355 = Divide(x=w1275, y=w1259) -> (x/y=w1274:dbl[])
            n356 = Divide(x=w1260, y=w1257) -> (x/y=w1256:dbl[])
            n357 = Divide(x=w1273, y=w1257) -> (x/y=w1272:dbl[])
            n358 = Negate(x=w1269) -> (-x=w1267:dbl[])
            n359 = Divide(x=w1271, y=w1267) -> (x/y=w1270:dbl[])
            n360 = Bundle("T1 Y", "T1 X", "T1 Sum", "T2 Y", "T2 X", "T2 Sum", "T1 FB Y", "T1 FB X", "T1 FB Sum", "T2 FB Y", "T2 FB X", "T2 FB Sum", "PSD X", "PSD Y Sum") -> (w1255:T30)  [unwired: 1 out]
            n361 = Build Array(w1292, w1291, w1306, w1290, w1289, w1303, w1258, w1274, w1259, w1256, w1272, w1257, w1270, w1269) -> (w1268:dbl[][])
            n362 = Cluster To Array(cluster=w1255) -> (array=w1301:string[])
          }
        }
      }
    }
    "AI labels" <- w408
    n363 = xnode "Read/Write Control"("FPGA VI Reference In"=w253) -> ("FPGA VI Reference Out"=w248:T13, "BD1 Frequency Out 1"=w264:u64)  [unwired: 1 in, 1 out]
    n364 = local read item#-1() -> ()  [unwired: 1 out]
    n365 = To Double Precision Float(number=w264) -> (double precision float=w261:dbl)
    n366 = Multiply(x=49125000.0, y=6.0) -> (x*y=w260:dbl)
    n367 = Multiply(x=w261, y=w260) -> (x*y=w258:dbl)
    n368 = Scale By Power Of 2(n=-48, x=w258) -> (x*2^n=w257:dbl)
    n369 = Divide(x=w257, y=1000000.0) -> (x/y=w252:dbl)
    n370 = case shown="True" {
      selector: _ -> [_ _]
      tunnel: w252 -> [_ w609]
      tunnel: w250 -> [_ w598]
      frame False {
      }
      frame True {
        n371 = local read "AOM X Cal (nm/MHz)"() -> (w607:dbl)
        n372 = local read item#-1() -> ()  [unwired: 1 out]
        n373 = Subtract(x=w609) -> (x-y=w608:dbl)  [unwired: 1 in]
        n374 = Multiply(x=w608, y=w607) -> (x*y=w606:dbl)
        n375 = local read "MCL X Cal (nm/V)"() -> (w603:dbl)
        n376 = Multiply(x=w606, y="Tracking factor") -> (x*y=w604:dbl)
        n377 = Divide(x=w604, y=w603) -> (x/y=w602:dbl)
        n378 = local read item#-1() -> ()  [unwired: 1 out]
        n379 = Add(y=w602) -> (x+y=w595:dbl)  [unwired: 1 in]
        "Current MCL (V)" <- w595
        n380 = Multiply(x=w595, y=32767.0) -> (x*y=w599:dbl)
        n381 = Divide(x=w599, y=10.0) -> (x/y=w596:dbl)
        n382 = To Word Integer(number=w596) -> (16bit integer=w597:i16)
        n383 = xnode "Read/Write Control"("FPGA VI Reference In"=w598, "AO2 (X)"=w597) -> ()  [unwired: 1 in, 2 out]
      }
    }
    n384 = local read item#-1() -> ()  [unwired: 1 out]
    n385 = local read item#-1() -> ()  [unwired: 1 out]
    n386 = Subtract(y=w252) -> (x-y=w249:dbl)  [unwired: 1 in]
    "Current deltaFreq" <- w249
    n387 = Compound Arithmetic op=AND("Real time offset \ncorrection for setpoint") -> (w254:bool)  [unwired: 2 in]
    n388 = case shown="True" w254 {
      tunnel: w249 -> [_ w612]
      tunnel: w248 -> [_ w611]
      frame False {
      }
      frame True {
        n389 = local read "T1 kappa_x (pN/nm)"() -> (w620:dbl)
        n390 = local read "T1 alpha_x (nm/V)"() -> (w621:dbl)
        n391 = local read "Negate offset difference"() -> (w622:bool)
        n392 = Multiply(x="Target Force (pN)", y=2.0) -> (x*y=w618:dbl)
        n393 = local read "Setpoint offset\nCorrection values"() -> (w627:dbl[])
        n394 = local read item#-1() -> ()  [unwired: 1 out]
        n395 = Divide(x=w612) -> (x/y=w629:dbl)  [unwired: 1 in]
        n396 = Select(t=-1, s=w622, f=1) -> (s? t:f=w623:i32)
        n397 = To Long Integer(number=w629) -> (32bit integer=w628:i32)
        n398 = Multiply(x=w621, y=w620) -> (x*y=w617:dbl)
        n399 = Divide(x=w618, y=w617) -> (x/y=w616:dbl)
        n400 = Index Array(array=w627, index=w628) -> (element=w626:dbl)
        n401 = Multiply(x=w623, y=w626) -> (x*y=w615:dbl)
        n402 = Add(x=w616, y=w615) -> (x+y=w614:dbl)
        n403 = To Fixed-Point(number=w614) -> (fixed-point=w610:fxp<+/-,16,1>)  [unwired: 1 in]
        "Actual setpoint" <- w610
        n404 = xnode "Read/Write Control"("FPGA VI Reference In"=w611, "Trap Pos. FB SP"=w610) -> ()  [unwired: 1 in, 2 out]
      }
    }
    n405 = case shown="True" {
      selector: _ -> [_ _]
      tunnel: [w587 _] -> w431
      tunnel: [w586 _] -> w429
      tunnel: w249 -> [_ w594]
      frame False {
        n406 = Divide(x="T2 offset_x (mV)", y=1000.0) -> (x/y=w586:dbl)
        n407 = Divide(x="T1 offset_x (mV)", y=1000.0) -> (x/y=w587:dbl)
      }
      frame True {
        n408 = local read item#-1() -> ()  [unwired: 1 out]
        n409 = local read item#-1() -> ()  [unwired: 1 out]
        n410 = Unbundle By Name() -> ()  [unwired: 1 in, 2 out]
        n411 = Divide(x=w594) -> (x/y=w593:dbl)  [unwired: 1 in]
        n412 = To Long Integer(number=w593) -> (32bit integer=w592:i32)
        n413 = Index Array(index=w592) -> ()  [unwired: 1 in, 1 out]
        n414 = Index Array(index=w592) -> ()  [unwired: 1 in, 1 out]
      }
    }
    n415 = Decimate 1D Array(w386) -> (w406:u32[], w354:u32[])
    n416 = local read item#-1() -> ()  [unwired: 1 out]
    n417 = Build Array(w406, w354) -> (w476:u32[][])
    n418 = Decimate 1D Array(w305) -> (w328:i16[], w327:i16[], w325:i16[], w324:i16[])  [unwired: 9 out]
    n419 = To Double Precision Float(number=w476) -> (double precision float=w477:dbl[][])
    n420 = local read item#-1() -> (w298)
    n421 = local read item#-1() -> ()  [unwired: 1 out]
    n422 = local read item#-1() -> (w299)
    n423 = local read "APD Integration Time (s)"() -> (w367:dbl)
    n424 = Divide(x=w328, y=w327) -> (x/y=w329:dbl[])
    n425 = Divide(x=w325, y=w324) -> (x/y=w326:dbl[])
    n426 = feedback #1(0.0) -> (w342:dbl)
    n427 = Add(y=w342) -> (x+y=w513:dbl)  [unwired: 1 in]
    n428 = feedback-in #1(w513) -> ()
    n429 = local read "AOM X Cal (nm/MHz)"() -> (w296:dbl)
    n430 = To Time Stamp(1:w342) -> (0:w341:timestamp)
    n431 = Split 1D Array(array=w329, index="N El. to Ave.") -> (second subarray=w332:dbl[])  [unwired: 1 out]
    n432 = Split 1D Array(array=w326, index="N El. to Ave.") -> (second subarray=w331:dbl[])  [unwired: 1 out]
    n433 = local read "Trap X AI1 (DMA)"() -> (w330:T8)
    n434 = Multiply(y="Trap Disp. Downsample") -> (x*y=w343:dbl)  [unwired: 1 in]
    "Display Period (s)" <- w343
    n435 = Bundle(w299, w298) -> ()  [unwired: 2 out]
    n436 = for "Trap AI" {
      tunnel: [w985] -> w507 mode=indexing
      tunnel: w341 -> [w976]
      tunnel: "Trap Disp. Downsample" -> [w983]
      tunnel: w409 -> [w981] mode=indexing
      tunnel: w408 -> [w980] mode=indexing
      tunnel: w340 -> [w979]
      tunnel: [w978] -> w378 mode=indexing
      tunnel: w343 -> [w977]
      n437 = Bundle By Name("Y"=w981) -> (w982:waveform(dbl))  [unwired: 1 in, 1 out]
      n438 = Set Waveform Attribute(5:w980, 6:w979, 7:w982) -> (3:w978:waveform(dbl))  [unwired: 1 in, 2 out]
      n439 = call "downsample 1D array - double.vi"("Ave N"=w983, "Array In"=w981) -> ("Array Out"=w984:dbl[])  [unwired: 1 out]
      n440 = Bundle By Name(cluster=w978, "t0"=w976, "Y"=w984, "dt"=w977) -> (w985:waveform(dbl))
    }
    n441 = call-poly <vilib>:"Mean.vi"("X"=w331) -> ("mean"=w319:dbl)  [unwired: 1 out]
    n442 = call-poly <vilib>:"Mean.vi"("X"=w332) -> ("mean"=w320:dbl)  [unwired: 1 out]
    n443 = Cluster To Array() -> (array=w297:void[])  [unwired: 1 in]
    n444 = Reciprocal(x=w343) -> (1/x=→"Trap Disp. Freq. (Hz)":dbl)
    n445 = To Fixed-Point(number=w319) -> (fixed-point=w317:fxp<+/-,16,1>)  [unwired: 1 in]
    n446 = To Fixed-Point(number=w320) -> (fixed-point=w318:fxp<+/-,16,1>)  [unwired: 1 in]
    n447 = Bundle("Trap 1 Pos.", "Trap 2 Pos.") -> (w339:cluster{string, string})  [unwired: 1 out]
    n448 = local read item#-1() -> ()  [unwired: 1 out]
    n449 = Bundle By Name(cluster=w330, "Set 1"=w318, "Set 2"=w317) -> (→"Trap X AI1 (DMA)":T8)
    n450 = Cluster To Array(cluster=w339) -> (array=w336:string[])
    n451 = for "Trap Position" {
      tunnel: w345 -> [w651] mode=indexing
      tunnel: "Trap Disp. Downsample" -> [w650]
      tunnel: w343 -> [w648]
      tunnel: w341 -> [w647]
      tunnel: w340 -> [w645]
      tunnel: w336 -> [w644] mode=indexing
      tunnel: [w643] -> w295 mode=indexing
      tunnel: w297 -> [_] mode=indexing
      tunnel: w296 -> [w640]
      n452 = call "downsample 1D array - double.vi"("Ave N"=w650, "Array In"=w651) -> ("Array Out"=w649:dbl[])  [unwired: 1 out]
      n453 = Subtract(x=w649) -> (x-y=w642:dbl[])  [unwired: 1 in]
      n454 = Multiply(x=w640, y=w642) -> (x*y=w641:dbl[])
      n455 = Bundle By Name("Y"=w641, "dt"=w648, "t0"=w647) -> (w646:waveform(dbl))  [unwired: 1 out]
      n456 = Set Waveform Attribute(5:w644, 6:w645, 7:w646) -> (3:w643:waveform(dbl))  [unwired: 1 in, 2 out]
    }
    "Trap Positions" <- w295
    n457 = Bundle("APD 1", "APD 2") -> (w506:cluster{string, string})  [unwired: 1 out]
    n458 = Cluster To Array(cluster=w506) -> (array=w503:string[])
    n459 = for "APD" {
      tunnel: w477 -> [w965] mode=indexing
      tunnel: w367 -> [w973]
      tunnel: [w969] -> w374 mode=indexing
      tunnel: "APD Disp. Scale" -> [w970]
      tunnel: w340 -> [w968]
      tunnel: w503 -> [w967] mode=indexing
      tunnel: "APD Disp. Downsample" -> [w963]
      tunnel: [w966] -> w502
      tunnel: w341 -> [w962]
      n460 = call "integrate 1D array interval - double.vi"("Ave N"=w963, "Array In"=w965) -> ("Array Out"=w964:dbl[])  [unwired: 1 out]
      n461 = Multiply(x=w973, y=w963) -> (x*y=w966:dbl)
      n462 = Divide(x=w964, y=w970) -> (x/y=w971:dbl[])
      n463 = Bundle By Name("t0"=w962, "Y"=w971, "dt"=w966) -> (w972:waveform(dbl))  [unwired: 1 out]
      n464 = Set Waveform Attribute(5:w967, 6:w968, 7:w972) -> (3:w969:waveform(dbl))  [unwired: 1 in, 2 out]
    }
    "APD Display Period (s)" <- w502
    n465 = Reciprocal(x=w502) -> (1/x=→"APD Display Freq. (Hz)":dbl)
    n466 = local read "Display Period (s)"() -> (w397:dbl)
    n467 = Increment() -> (x+1=w488:dbl)  [unwired: 1 in]
    n468 = Index Array(array=w295, index=0) -> (element=w293:waveform(dbl))
    n469 = To Double Precision Float(number=w406) -> (double precision float=w405:dbl[])
    n470 = feedback #2(w488) -> (w491:i32)
    n471 = Select(t=0, s=w479, f=w491) -> (s? t:f=w485:i32)
    n472 = Array Size(array=w405) -> (size(s)=w490:i32)
    n473 = Add(x=w490, y=w485) -> (x+y=w486:i32)
    n474 = Unbundle By Name(w293) -> ("Y"=w291:dbl[])
    n475 = feedback #3(w406) -> (w475:u32[])
    n476 = Build Array (concatenate)(w475, w406) -> (w472:u32[])
    n477 = feedback #4(w354) -> (w373:u32[])
    n478 = Divide(x="Bead Sep. Int. Time (s)", y=w397) -> (x/y=w289:dbl)
    n479 = Build Array (concatenate)(w373, w354) -> (w372:u32[])
    n480 = Greater?(x=w486) -> (0:w487:bool)  [unwired: 1 in]
    n481 = feedback #5(w291) -> (w292:dbl[])
    n482 = Build Array (concatenate)(w291, w292) -> (w290:dbl[])
    n483 = Select(t=w485, s=w487, f=w486) -> (s? t:f=w484:i32)
    n484 = feedback-in #2(w484) -> ()
    n485 = Array Size(array=w472) -> (size(s)=w469:i32)
    n486 = Array Size(array=w406) -> (size(s)=w471:i32)
    n487 = local read "MCL Scanning"() -> (w482:bool)
    n488 = local read "APD Integration Time (s)"() -> (w381:dbl)
    n489 = Build Array (concatenate)(w374, w507) -> (w376:waveform(dbl)[])
    "All Signals" <- w376
    n490 = Split 1D Array(array=w290, index=w289) -> (first subarray=w283:dbl[])  [unwired: 1 out]
    n491 = feedback-in #5(w283) -> ()
    n492 = Multiply(x=w471, y="APD Ave N") -> (x*y=w470:dbl)
    n493 = Greater?(x=w469, y=w470) -> (0:w473:bool)
    n494 = Not(x=w487) -> (.not. x?=w481:bool)
    n495 = To Double Precision Float(number=w354) -> (double precision float=w353:dbl[])
    n496 = call-poly <vilib>:"Mean.vi"("X"=w283) -> ("mean"=w282:dbl)  [unwired: 1 out]
    "Mean T1 Position (nm)" <- w282
    n497 = Subtract(x=w283, y=w282) -> (x-y=w288:dbl[])
    n498 = Square(x=w288) -> (x^2=w287:dbl[])
    n499 = And(x=w481, y=w482) -> (x .and. y?=w483:bool)
    n500 = call-poly <vilib>:"Mean.vi"("X"=w287) -> ("mean"=w286:dbl)  [unwired: 1 out]
    n501 = case shown="True" w473 {
      tunnel: w472 -> [w761 w768]
      tunnel: [w761 w766] -> w420
      tunnel: w470 -> [_ w763]
      tunnel: w469 -> [_ w767]
      tunnel: w372 -> [w760 w765]
      tunnel: [w760 w762] -> w369
      frame False {
      }
      frame True {
        n502 = Subtract(x=w767, y=w763) -> (x-y=w764:dbl)
        n503 = Array Subset(array=w768, index=w764, length=w763) -> (w766:u32[])
        n504 = Array Subset(array=w765, index=w764, length=w763) -> (w762:u32[])
      }
    }
    n505 = feedback-in #3(w420) -> ()
    n506 = feedback-in #4(w369) -> ()
    n507 = Or(x=w483, y=w479) -> (x .or. y?=w480:bool)
    n508 = Square Root(x=w286) -> (sqrt(x)=w285:dbl)
    n509 = Equal?(x="Tab Control 6", y=T19."High Res Display") -> (x = y?=w412:bool)
    n510 = Multiply(x="APD Disp. Scale", y=w374) -> (x*y=w383:waveform(dbl)[])
    n511 = Multiply(x="APD Disp. Downsample", y=w381) -> (x*y=w379:dbl)
    n512 = Multiply(x=10.0, y=w285) -> (x*y=→"Trap 1 Position RMS (A)":dbl)
    n513 = Divide(x=w383, y=w379) -> (x/y=w351:waveform(dbl)[])
    n514 = Index Array(array=w351, index=0) -> (element=w361:waveform(dbl))
    n515 = case "For computing FFTs for display" shown="True" "Compute FFT" {
      tunnel: w378 -> [_ w1418]
      frame False {
      }
      frame True {
        n516 = Build Array("FFT 1 Choice 1", "FFT 1 Choice 2", "FFT 2 Choice 1", "FFT 2 Choice 2") -> (w1411:u16[])
        n517 = Array Size(array=w1418) -> (size(s)=w1417:i32)
        n518 = feedback-in #6(w1411) -> ()
        n519 = feedback #6(u16[] [100, 100, 100, 100]) -> (w1412:u16[])
        n520 = feedback-in #7("# Spectra to Ave.") -> ()
        n521 = feedback #7("# Spectra to Ave.") -> (w1409:dbl)
        n522 = Not Equal?(x="# Spectra to Ave.", y=w1409) -> (x != y?=w1408:bool)
        n523 = Not Equal?(x=w1411, y=w1412) -> (x != y?=w1410:bool)
        n524 = feedback #8(1.0) -> (w1395:dbl)
        n525 = Compound Arithmetic op=OR("Reset FFT", w1410, w1408) -> (w1393:bool)
        n526 = Select(t=1.0, s=w1393, f=w1395) -> (s? t:f=w1397:dbl)
        n527 = Greater?(x=w1397, y="# Spectra to Ave.") -> (0:w1416:bool)
        n528 = Increment(x=w1397) -> (x+1=w1396:dbl)
        n529 = feedback-in #8(w1396) -> ()
        n530 = local read item#-1() -> ()  [unwired: 1 out]
        n531 = Multiply(x="# Spectra to Ave.") -> (x*y=→"Ave. Time (s)":dbl)  [unwired: 1 in]
        n532 = Build Array(cluster{"f0":dbl, "df":dbl, "magnitude":dbl[]} {"f0"=0.0, "df"=0.0, "magnitude"=[]} ("PSD")) -> (w1400:cluster{"f0":dbl, "df":dbl, "magnitude":dbl[]}[])
        n533 = Build Array(w1400, w1400, w1400, w1400) -> (w1402:T31)
        n534 = feedback #9(w1402) -> (w1407:T31)
        n535 = for {
          N: 4 -> [_]
          tunnel: w1411 -> [w1440] mode=indexing
          tunnel: w1418 -> [w1441]
          tunnel: w1417 -> [w1443]
          tunnel: w1393 -> [w1436]
          tunnel: w1416 -> [w1435]
          tunnel: "# Spectra to Ave." -> [w1434]
          tunnel: [w1433] -> w1406 mode=indexing
          tunnel: w1407 -> [w1438] mode=indexing
          tunnel: [w1437] -> w1394 mode=indexing
          tunnel: w1397 -> [w1432]
          n536 = Less?(x=w1440, y=w1443) -> (x < y?=w1442:bool)
          n537 = Index Array(array=w1441, index=w1440) -> (element=w1439:waveform(dbl))
          n538 = case shown="True" w1442 {
            tunnel: w1439 -> [_ w1460]
            tunnel: w1438 -> [w1445 w1458]
            tunnel: [w1445 w1446] -> w1437
            tunnel: w1436 -> [_ w1457]
            tunnel: w1435 -> [_ w1450]
            tunnel: w1434 -> [_ w1449]
            tunnel: [cluster{"f0":dbl, "df":dbl, "magnitude":dbl[]} {"f0"=0.0, "df"=0.0, "magnitude"=[]} ("PSD") w1451] -> w1433
            tunnel: w1432 -> [_ w1448]
            frame False {
            }
            frame True {
              n539 = call <vilib>:"Std Deviation and Variance.vi"("X"=w1460) -> ("mean"=w1461:dbl)  [unwired: 1 in, 2 out]
              n540 = Subtract(x=w1460, y=w1461) -> (x-y=w1459:waveform(dbl))
              n541 = xnode "Spectral Measurements"("Signals"=w1459) -> ("PSD"=w1453:cluster{"f0":dbl, "df":dbl, "magnitude":dbl[]})  [unwired: 1 in, 1 out]
              n542 = case shown="False" w1457 {
                tunnel: w1458 -> [w1470 _]
                tunnel: [w1466 w1475] -> w1446
                tunnel: w1453 -> [w1469 w1476]
                tunnel: w1450 -> [w1468 _]
                frame False {
                  n543 = Build Array (concatenate)(w1470, w1469) -> (w1467:cluster{"f0":dbl, "df":dbl, "magnitude":dbl[]}[])
                  n544 = case shown="True" w1468 {
                    tunnel: w1467 -> [w1471 w1474]
                    tunnel: [w1471 w1472] -> w1466
                    frame False {
                    }
                    frame True {
                      n545 = Delete From Array(array=w1474, index=0) -> (array with subset deleted=w1472:cluster{"f0":dbl, "df":dbl, "magnitude":dbl[]}[])  [unwired: 1 in, 1 out]
                    }
                  }
                }
                frame True {
                  n546 = Build Array(w1476) -> (w1475:cluster{"f0":dbl, "df":dbl, "magnitude":dbl[]}[])
                }
              }
              n547 = for {
                tunnel: w1446 -> [w1465] mode=indexing
                tunnel: [w1464] -> w1456 mode=indexing
                workers-P: _ -> [_]
                n548 = Unbundle By Name(w1465) -> ("magnitude"=w1464:dbl[])
              }
              n549 = Transpose 2D Array(2D array=w1456) -> (transposed array=w1455:dbl[][])
              n550 = for {
                tunnel: w1455 -> [w1463] mode=indexing
                tunnel: [w1462] -> w1454 mode=indexing
                workers-P: _ -> [_]
                n551 = Add Array Elements(numeric array=w1463) -> (sum=w1462:dbl)
              }
              n552 = Select(t=w1449, s=w1450, f=w1448) -> (s? t:f=w1447:dbl)
              n553 = Divide(x=w1454, y=w1447) -> (x/y=w1452:dbl[])
              n554 = Bundle By Name(cluster=w1453, "magnitude"=w1452) -> (w1451:cluster{"f0":dbl, "df":dbl, "magnitude":dbl[]})
            }
          }
        }
        n555 = case shown="True" w1393 {
          tunnel: w1394 -> [w1425 w1431]
          tunnel: [w1425 w1426] -> w1392
          frame False {
          }
          frame True {
            n556 = Array Subset(array=w1431, index (row)=0 ("index"), length (row)=4 ("length"), index (col)=0 ("index"), length (col)=1 ("length")) -> (w1426:T31)
          }
        }
        n557 = feedback-in #9(w1392) -> ()
        n558 = Split 1D Array(array=w1406, index=2) -> (first subarray=→"FFT 1":cluster{"f0":dbl, "df":dbl, "magnitude":dbl[]}[], second subarray=→"FFT 2":cluster{"f0":dbl, "df":dbl, "magnitude":dbl[]}[])
      }
    }
    n559 = Index Array(array=w351, index=1) -> (element=w359:waveform(dbl))
    n560 = case "For displaying the high resolution display (no downsampling)" shown="True" w412 {
      tunnel: w378 -> [_ w661]
      frame False {
      }
      frame True {
        n561 = Index Array(array=w661, index="High Res. Display") -> (element=w662:waveform(dbl))
        n562 = call <vilib>:"Std Deviation and Variance.vi"("X"=w662) -> ("mean"=w669:dbl, "standard deviation"=w674:dbl)  [unwired: 1 in, 1 out]
        "Mean Intensity" <- w669
        "Sigma" <- w674
        n563 = Subtract(x=w662, y=w669) -> (x-y=w668:waveform(dbl))
        n564 = Select(t=w668, s="Subtract mean", f=w662) -> (s? t:f=→"1 Channel":waveform(dbl))
        n565 = Divide(x=w674, y=w669) -> (x/y=→"Sigma/Mean":dbl)
        n566 = feedback #10(1) -> (w663:i32)
        n567 = Greater Or Equal?(x=w663, y="Slow mean N ave.") -> (x >= y?=w676:bool)
        n568 = Increment(x=w663) -> (x+1=w678:i32)
        n569 = Select(t=1, s=w676, f=w678) -> (s? t:f=w665:i32)
        n570 = feedback-in #10(w665) -> ()
        n571 = feedback #11() -> (w666:waveform(dbl))  [unwired: 1 out]
        n572 = case shown="Default" w663 {
          tunnel: [w681 w684] -> w667
          tunnel: w666 -> [w683 _]
          tunnel: w662 -> [w682 w684]
          frame Default {
            n573 = call-poly <vilib>:"Append Waveforms.vi"("waveform B"=w682, "waveform A"=w683) -> ("waveform out"=w681:waveform(dbl))  [unwired: 1 in, 8 out]
          }
          frame 1 {
          }
        }
        n574 = feedback-in #11(w667) -> ()
        n575 = case shown="True" w676 {
          tunnel: w667 -> [_ w680]
          frame False {
          }
          frame True {
            n576 = call-poly <vilib>:"Mean.vi"("X"=w680) -> ("mean"=→"Slow mean":dbl)  [unwired: 1 out]
          }
        }
      }
    }
    n577 = case "For plotting results of scanning MCL" shown="True" w480 {
      tunnel: w479 -> [_ w798]
      tunnel: w405 -> [_ w893]
      tunnel: w378 -> [_ w867]
      tunnel: w353 -> [_ w799]
      tunnel: w352 -> [_ w774]
      frame False {
      }
      frame True {
        w781 = u32 0 items=["Horizontal", "Vertical", "Central", "1st Diagonal", "2nd Diagonal"] ("Type of Symmetry")
        w807 = u32 0 items=["Horizontal", "Vertical", "Central", "1st Diagonal", "2nd Diagonal"] ("Type of Symmetry")
        w810 = u32 0 items=["Horizontal", "Vertical", "Central", "1st Diagonal", "2nd Diagonal"] ("Type of Symmetry")
        w838 = u32 0 items=["Horizontal", "Vertical", "Central", "1st Diagonal", "2nd Diagonal"] ("Type of Symmetry")
        n578 = Index Array(array=w867, index=10) -> (element=w873:waveform(dbl))
        n579 = Index Array(array=w867, index=11) -> (element=w870:waveform(dbl))
        n580 = Index Array(array=w867, index="Channel") -> (element=w869:waveform(dbl))
        n581 = Unbundle(w774) -> ("New Image"=w773:T3, "New Image"=w772:T3, "New Image"=w771:T3, "New Image"=w770:T3)
        n582 = Unbundle By Name(w873) -> ("Y"=w825:dbl[])
        n583 = Unbundle By Name(w870) -> ("Y"=w827:dbl[])
        n584 = local read item#-1() -> ()  [unwired: 1 out]
        n585 = Unbundle By Name(w869) -> ("Y"=w832:dbl[])
        n586 = call "downsample 1D array - double.vi"("Array In"=w825) -> ("Array Out"=w824:dbl[])  [unwired: 1 in, 1 out]
        n587 = call "downsample 1D array - double.vi"("Array In"=w827) -> ("Array Out"=w826:dbl[])  [unwired: 1 in, 1 out]
        n588 = call "downsample 1D array - double.vi"("Array In"=w832) -> ("Array Out"=w831:dbl[])  [unwired: 1 in, 1 out]
        n589 = feedback #12(w893) -> (w894:dbl[])
        n590 = Build Array (concatenate)(w894, w893) -> (w875:dbl[])
        n591 = feedback #13(w799) -> (w801:dbl[])
        n592 = Build Array (concatenate)(w801, w799) -> (w800:dbl[])
        n593 = Select(t=w893, s=w798, f=w875) -> (s? t:f=w879:dbl[])
        n594 = feedback-in #12(w879) -> ()
        n595 = Select(t=w799, s=w798, f=w800) -> (s? t:f=w783:dbl[])
        n596 = feedback-in #13(w783) -> ()
        n597 = local read item#-1() -> ()  [unwired: 1 out]
        n598 = local read item#-1() -> ()  [unwired: 1 out]
        n599 = feedback #14(w824) -> (w881:dbl[])
        n600 = Build Array (concatenate)(w881, w824) -> (w872:dbl[])
        n601 = feedback #15(w831) -> (w891:dbl[])
        n602 = Build Array (concatenate)(w891, w831) -> (w890:dbl[])
        n603 = feedback #16(w826) -> (w883:dbl[])
        n604 = Build Array (concatenate)(w883, w826) -> (w884:dbl[])
        n605 = Select(t=w824, s=w798, f=w872) -> (s? t:f=w828:dbl[])
        n606 = feedback-in #14(w828) -> ()
        n607 = Select(t=w831, s=w798, f=w890) -> (s? t:f=w830:dbl[])
        n608 = feedback-in #15(w830) -> ()
        n609 = Select(t=w826, s=w798, f=w884) -> (s? t:f=w829:dbl[])
        n610 = feedback-in #16(w829) -> ()
        n611 = local read item#-1() -> ()  [unwired: 1 out]
        n612 = Multiply(y=u64 2) -> (x*y=w769:u64)  [unwired: 1 in]
        n613 = call "integrate 1D array interval - double.vi"("Array In"=w783) -> ("Array Out"=w794:dbl[])  [unwired: 1 in, 1 out]
        n614 = call "integrate 1D array interval - double.vi"("Array In"=w879) -> ("Array Out"=w878:dbl[])  [unwired: 1 in, 1 out]
        n615 = Array Size(array=w794) -> (size(s)=w795:i32)
        n616 = Array Size(array=w878) -> (size(s)=w880:i32)
        n617 = Multiply(y=w769) -> (x*y=w797:u64)  [unwired: 1 in]
        n618 = Multiply(y=w769) -> (x*y=w888:u64)  [unwired: 1 in]
        n619 = call-poly <vilib>:"Mean.vi"("X"=w828) -> ("mean"=w813:dbl)  [unwired: 1 out]
        n620 = Subtract(x=w797, y=w795) -> (x-y=w788:u64)
        n621 = call-poly <vilib>:"Mean.vi"("X"=w830) -> ("mean"=w818:dbl)  [unwired: 1 out]
        n622 = call-poly <vilib>:"Mean.vi"("X"=w829) -> ("mean"=w816:dbl)  [unwired: 1 out]
        n623 = call-poly <vilib>:"Mean.vi"("X"=w794) -> ("mean"=w785:dbl)  [unwired: 1 out]
        n624 = Subtract(x=w888, y=w880) -> (x-y=w823:u64)
        n625 = call-poly <vilib>:"Mean.vi"("X"=w878) -> ("mean"=w820:dbl)  [unwired: 1 out]
        n626 = Initialize Array(1.0 ("element"), w788) -> (w784:dbl[])
        n627 = Initialize Array(1.0 ("element"), w823) -> (w814:dbl[])
        n628 = Multiply(x=w784, y=w785) -> (x*y=w786:dbl[])
        n629 = Multiply(x=w814, y=w816) -> (x*y=w817:dbl[])
        n630 = Multiply(x=w814, y=w818) -> (x*y=w819:dbl[])
        n631 = Multiply(x=w814, y=w813) -> (x*y=w815:dbl[])
        n632 = Multiply(x=w814, y=w820) -> (x*y=w821:dbl[])
        n633 = Build Array (concatenate)(w828, w815) -> (w882:dbl[])
        n634 = Build Array (concatenate)(w830, w819) -> (w886:dbl[])
        n635 = Build Array (concatenate)(w829, w817) -> (w885:dbl[])
        n636 = Build Array (concatenate)(w794, w786) -> (w796:dbl[])
        n637 = Build Array (concatenate)(w878, w821) -> (w887:dbl[])
        n638 = Reshape Array(w882, w769) -> (w848:dbl[][])  [unwired: 1 in]
        n639 = Reshape Array(w796, w769) -> (w792:dbl[][])  [unwired: 1 in]
        n640 = Reshape Array(w886, w769) -> (w840:dbl[][])  [unwired: 1 in]
        n641 = Reshape Array(w885, w769) -> (w855:dbl[][])  [unwired: 1 in]
        n642 = Reshape Array(w887, w769) -> (w865:dbl[][])  [unwired: 1 in]
        n643 = Array Subset(array=w855, index (col)=0 ("index")) -> (w860:dbl[][])  [unwired: 3 in]
        n644 = Array Subset(array=w855) -> (w858:dbl[][])  [unwired: 4 in]
        n645 = Array Subset(array=w840, index (col)=0 ("index")) -> (w846:dbl[][])  [unwired: 3 in]
        n646 = Array Subset(array=w840) -> (w844:dbl[][])  [unwired: 4 in]
        n647 = Array Subset(array=w792, index (col)=0 ("index")) -> (w791:dbl[][])  [unwired: 3 in]
        n648 = Array Subset(array=w792) -> (w789:dbl[][])  [unwired: 4 in]
        n649 = Array Subset(array=w865, index (col)=0 ("index")) -> (w864:dbl[][])  [unwired: 3 in]
        n650 = Array Subset(array=w865) -> (w862:dbl[][])  [unwired: 4 in]
        n651 = Array Subset(array=w848, index (col)=0 ("index")) -> (w853:dbl[][])  [unwired: 3 in]
        n652 = Array Subset(array=w848) -> (w851:dbl[][])  [unwired: 4 in]
        n653 = for {
          tunnel: w860 -> [w902] mode=indexing
          tunnel: [w901] -> w859 mode=indexing
          workers-P: _ -> [_]
          n654 = Reverse 1D Array(array=w902) -> (reversed array=w901:dbl[])
        }
        n655 = for {
          tunnel: w846 -> [w898] mode=indexing
          tunnel: [w897] -> w845 mode=indexing
          workers-P: _ -> [_]
          n656 = Reverse 1D Array(array=w898) -> (reversed array=w897:dbl[])
        }
        n657 = for {
          tunnel: w791 -> [w896] mode=indexing
          tunnel: [w895] -> w790 mode=indexing
          workers-P: _ -> [_]
          n658 = Reverse 1D Array(array=w896) -> (reversed array=w895:dbl[])
        }
        n659 = for {
          tunnel: w864 -> [w904] mode=indexing
          tunnel: [w903] -> w863 mode=indexing
          workers-P: _ -> [_]
          n660 = Reverse 1D Array(array=w904) -> (reversed array=w903:dbl[])
        }
        n661 = for {
          tunnel: w853 -> [w900] mode=indexing
          tunnel: [w899] -> w852 mode=indexing
          workers-P: _ -> [_]
          n662 = Reverse 1D Array(array=w900) -> (reversed array=w899:dbl[])
        }
        n663 = Index Array(array=w865, index (row)=0) -> (element=→"Waveform Graph":dbl[])  [unwired: 1 in]
        n664 = Add(x=w859, y=w858) -> (x+y=w857:dbl[][])
        n665 = Add(x=w845, y=w844) -> (x+y=w843:dbl[][])
        n666 = Add(x=w790, y=w789) -> (x+y=w776:dbl[][])
        n667 = Add(x=w863, y=w862) -> (x+y=w837:dbl[][])
        n668 = Add(x=w852, y=w851) -> (x+y=w850:dbl[][])
        n669 = Divide(x=w843, y=2) -> (x/y=w841:dbl[][])
        n670 = Divide(x=w857, y=2) -> (x/y=w803:dbl[][])
        n671 = Divide(x=w850, y=2) -> (x/y=w805:dbl[][])
        n672 = To Single Precision Float(number=w837) -> (single precision float=w836:sgl[][])
        n673 = Transpose 2D Array(2D array=w841) -> (transposed array=→"Data map":dbl[][])
        n674 = To Single Precision Float(number=w776) -> (single precision float=w780:sgl[][])
        n675 = To Single Precision Float(number=w803) -> (single precision float=w809:sgl[][])
        n676 = To Single Precision Float(number=w805) -> (single precision float=w806:sgl[][])
        n677 = call "IMAQ ArrayToImage"("Image Pixels (Float)"=w836, "Image"=w773) -> ("Image Out"=w839:T3)  [unwired: 8 in, 1 out]
        n678 = call "IMAQ ArrayToImage"("Image Pixels (Float)"=w780, "Image"=w772) -> ("Image Out"=w782:T3)  [unwired: 8 in, 1 out]
        n679 = call "IMAQ ArrayToImage"("Image Pixels (Float)"=w809, "Image"=w771) -> ("Image Out"=w811:T3)  [unwired: 8 in, 1 out]
        n680 = call "IMAQ ArrayToImage"("Image Pixels (Float)"=w806, "Image"=w770) -> ("Image Out"=w808:T3)  [unwired: 8 in, 1 out]
        n681 = call "IMAQ Symmetry"("Type of Symmetry"=w838, "Image Src"=w839) -> ("Image Dst Out"=w834:T3)  [unwired: 3 in, 1 out]
        n682 = call "IMAQ Symmetry"("Type of Symmetry"=w781, "Image Src"=w782) -> ("Image Dst Out"=w778:T3)  [unwired: 3 in, 1 out]
        n683 = call "IMAQ Symmetry"("Type of Symmetry"=w810, "Image Src"=w811) -> ("Image Dst Out"=→"Detection Laser X":T3)  [unwired: 3 in, 1 out]
        n684 = call "IMAQ Symmetry"("Type of Symmetry"=w807, "Image Src"=w808) -> ("Image Dst Out"=→"Detection Laser Y":T3)  [unwired: 3 in, 1 out]
        n685 = call "IMAQ Set Simple Calibration"("Calibration Axis Info"=T20 {"Origin Pixel"={"X"=0.0, "Y"=0.0}, "Angle Relative to Horizontal (deg)"=0.0, "Axis Reference"=0}, "Grid Descriptor"=T21 {"X Step"=0.3, "Y Step"=0.3, "Unit"=enum."Undefined"}, "Image"=w834) -> ("Calibrated Image"=→"APD 1":T3)  [unwired: 7 in, 1 out]
        n686 = call "IMAQ Set Simple Calibration"("Calibration Axis Info"=T20 {"Origin Pixel"={"X"=0.0, "Y"=0.0}, "Angle Relative to Horizontal (deg)"=0.0, "Axis Reference"=0}, "Grid Descriptor"=T21 {"X Step"=0.3, "Y Step"=0.3, "Unit"=enum."Undefined"}, "Image"=w778) -> ("Calibrated Image"=→"APD 2":T3)  [unwired: 7 in, 1 out]
      }
    }
    n687 = Subtract(x=w359, y="APD 2 Offset") -> (x-y=w356:waveform(dbl))
    n688 = Subtract(x=w361, y="APD 1 Offset") -> (x-y=w357:waveform(dbl))
    n689 = Index Array(array=w376, index=3) -> (element=w430:waveform(dbl))
    n690 = Index Array(array=w376, index=6) -> (element=w427:waveform(dbl))
    n691 = Build Array(w357, w356) -> (→"APD Chart":waveform(dbl)[])
    n692 = Array Size(array=w420) -> (size(s)=w468:i32)
    n693 = call <vilib>:"Std Deviation and Variance.vi"("X"=w369) -> ("standard deviation"=w368:dbl)  [unwired: 1 in, 2 out]
    n694 = Add Array Elements(numeric array=w369) -> (sum=w371:u32)
    n695 = Add Array Elements(numeric array=w420) -> (sum=w478:u32)
    n696 = call <vilib>:"Std Deviation and Variance.vi"("X"=w420) -> ("standard deviation"=w419:dbl)  [unwired: 1 in, 2 out]
    n697 = Divide(x=w368, y=w367) -> (x/y=w364:dbl)
    "Rate sigma (Hz) 2" <- w364
    n698 = Multiply(x=w367, y=w468) -> (x*y=w370:dbl)
    "Int. Time (s)" <- w370
    n699 = Divide(x=w371, y=w370) -> (x/y=w365:dbl)
    "APD 2 Rate (Hz)" <- w365
    n700 = Divide(x=w478, y=w370) -> (x/y=w417:dbl)
    "APD 1 Rate (Hz)" <- w417
    n701 = Divide(x=w419, y=w367) -> (x/y=w418:dbl)
    "Rate sigma (Hz)" <- w418
    n702 = Divide(x=w364, y=w365) -> (x/y=→"Sigma/Mean 2":dbl)
    n703 = Divide(x=w418, y=w417) -> (x/y=→"Sigma/Mean":dbl)
    n704 = case shown="2" "Calibration" {
      tunnel: "T1 alpha_x (nm/V)" -> [_ w737 w758]
      tunnel: "T1 kappa_x (pN/nm)" -> [_ _ w748]
      tunnel: "T2 alpha_x (nm/V)" -> [_ w736 w756]
      tunnel: "T2 kappa_x (pN/nm)" -> [_ _ w749]
      tunnel: w430 -> [w719 w734 w754]
      tunnel: w427 -> [w718 w732 w752]
      tunnel: [w719 w731 w751] -> w237
      tunnel: [w718 w730 w750] -> w243
      tunnel: ["T1 X (V)" ("Label.Text") "T1 X (nm)" ("Label.Text") "T1 X (pN)" ("Label.Text")] -> w448
      tunnel: ["T2 X (V)" ("Label.Text") "T2 X (nm)" ("Label.Text") "T2 X (pN)" ("Label.Text")] -> w447
      tunnel: ["Position (V)" ("Label.Text") "Position (nm)" ("Label.Text") "Force (pN)" ("Label.Text")] -> w449
      tunnel: w429 -> [_ w722 w741]
      tunnel: w431 -> [_ w725 w743]
      tunnel: ["Mean (V)" ("Label.Text") "Mean (nm)" ("Label.Text") "Mean (pN)" ("Label.Text")] -> w444
      tunnel: ["Difference (V)" ("Label.Text") "Difference (nm)" ("Label.Text") "Difference (pN)" ("Label.Text")] -> w384
      frame 0, Default {
      }
      frame 1 {
        # "position"
        n705 = Unbundle By Name(w734) -> ("Y"=w738:dbl[])
        n706 = Unbundle By Name(w732) -> ("Y"=w723:dbl[])
        n707 = Subtract(x=w738, y=w725) -> (x-y=w726:dbl[])
        n708 = Subtract(x=w723, y=w722) -> (x-y=w724:dbl[])
        n709 = Multiply(x=w724, y=w736) -> (x*y=w733:dbl[])
        n710 = Multiply(x=w737, y=w726) -> (x*y=w735:dbl[])
        n711 = Bundle By Name(cluster=w732, "Y"=w733) -> (w730:waveform(dbl))
        n712 = Bundle By Name(cluster=w734, "Y"=w735) -> (w731:waveform(dbl))
      }
      frame 2 {
        # "force"
        n713 = Unbundle By Name(w754) -> ("Y"=w759:dbl[])
        n714 = Unbundle By Name(w752) -> ("Y"=w757:dbl[])
        n715 = Subtract(x=w757, y=w741) -> (x-y=w742:dbl[])
        n716 = Subtract(x=w759, y=w743) -> (x-y=w744:dbl[])
        n717 = Compound Arithmetic op=MULTIPLY(w742, w756, w749) -> (w753:dbl[])
        n718 = Compound Arithmetic op=MULTIPLY(w748, w758, w744) -> (w755:dbl[])
        n719 = Bundle By Name(cluster=w752, "Y"=w753) -> (w750:waveform(dbl))
        n720 = Bundle By Name(cluster=w754, "Y"=w755) -> (w751:waveform(dbl))
      }
    }
    n721 = feedback-in #17("Calibration") -> ()
    n722 = feedback #17(u16 1 ("Calibration")) -> (w451:u16)
    n723 = local read "AOM X Cal (nm/MHz)"() -> (w266:dbl)
    n724 = local read item#-1() -> ()  [unwired: 1 out]
    n725 = local read item#-1() -> ()  [unwired: 1 out]
    n726 = local read item#-1() -> ()  [unwired: 1 out]
    n727 = Not Equal?(x=w451, y="Calibration") -> (x != y?=w410:bool)
    n728 = Multiply(x=w266) -> (x*y=w268:dbl)  [unwired: 1 in]
    n729 = Unbundle By Name(w237) -> ("Y"=w242:dbl[])
    n730 = Unbundle By Name(w243) -> ("Y"=w241:dbl[])
    n731 = Add() -> (x+y=w270:dbl)  [unwired: 2 in]
    n732 = case shown="False" {
      selector: _ -> [_ _]
      tunnel: [-1.0 1.0] -> w437
      frame False {
      }
      frame True {
      }
    }
    n733 = Unbundle By Name(w430) -> ("Y"=w433:dbl[])
    n734 = Unbundle By Name(w427) -> ("Y"=w436:dbl[])
    n735 = Divide(x=w270, y=2.0) -> (x/y=w267:dbl)
    n736 = Subtract(x=w242, y=w241) -> (x-y=w239:dbl[])
    n737 = Subtract(x=w433, y=w431) -> (x-y=w434:dbl[])
    n738 = Subtract(x=w436, y=w429) -> (x-y=w435:dbl[])
    n739 = Divide(x=w239, y=2.0) -> (x/y=w238:dbl[])
    n740 = Multiply(x=w435, y="T2 alpha_x (nm/V)") -> (x*y=w426:dbl[])
    n741 = Multiply(x="T1 alpha_x (nm/V)", y=w434) -> (x*y=w425:dbl[])
    n742 = Multiply(x=w243, y=w437) -> (x*y=w438:waveform(dbl))
    n743 = Bundle By Name(cluster=w237, "Y"=w238) -> (w236:waveform(dbl))
    n744 = case shown="True" "Read Lateness and Rel Phase" {
      tunnel: w248 -> [w685 w707]
      tunnel: w278 -> [w686 w706]
      tunnel: [w685 w705] -> w423
      tunnel: [w686 w704] -> w422
      frame False {
      }
      frame True {
        n745 = xnode "Read/Write Control"("FPGA VI Reference In"=w707, "error in"=w706) -> ("FPGA VI Reference Out"=w705:T13, "error out"=w704:errorcluster, "GI Relative phase"=→"GI relative phase":i16, "Relative phase"=→"Relative phase (AI1)":i16, "AI Late Counter"=→"Late Counter (AI1)":u8, "GI Late Counter"=→"GI Late Counter":u8, "MCL Late Counter"=→"MCL Late Counter":u8, "MCL Relative Phase"=→"Relative Phase (MCL)":i16, "APD Acq Relative Phase"=→"APD Acq Relative Phase":i16, "APD 1 Gate Relative Phase"=→"APD 1 Gate Relative Phase":i16, "APD 2 Gate Relative Phase"=→"APD 2 Gate Relative Phase":i16, "APD Acq Late Counter"=→"APD Acq Late Counter":u16, "APD 1 Gate Late Counter"=→"APD 1 Gate Late Counter":u8, "APD 2 Gate Late Counter"=→"APD 2 Gate Late Counter":u8, "Green FB Relative Phase"=→"Relative phase (Green FB)":i16, "GI Relative phase"=→"GI relative phase 2":i16, "GI Late Counter 2"=→"GI Late Counter 2":u16, "Trap Pos FIFO Timeout"=→"Trap Pos FIFO Timeout":u16, "Trap AI FIFO Timeout"=→"Trap AI FIFO Timeout":u16)
      }
    }
    n746 = Subtract(x=w426, y=w425) -> (x-y=w265:dbl[])
    n747 = call-poly <vilib>:"Mean.vi"("X"=w265) -> ("mean"=w269:dbl)  [unwired: 1 out]
    n748 = Add(x=w268, y=w269) -> (x+y=w272:dbl)
    n749 = Subtract(x=w272, y=w267) -> (x-y=→"Tether Extension (nm, calculated)":dbl)
    n750 = Unbundle By Name(w243) -> ("Y"=w234:dbl[])
    n751 = Unbundle By Name(w237) -> ("Y"=w235:dbl[])
    n752 = Build Array(w237, w438, w236) -> (→"Force":waveform(dbl)[])
    n753 = Subtract(x=w265, y="Offset (nm)") -> (x-y=w401:dbl[])
    n754 = call-poly <vilib>:"Mean.vi"("X"=w234) -> ("mean"=w232:dbl)  [unwired: 1 out]
    "T2 X" <- w232
    n755 = call-poly <vilib>:"Mean.vi"("X"=w235) -> ("mean"=w233:dbl)  [unwired: 1 out]
    "T1 X" <- w233
    n756 = Subtract(x=w235, y=w234) -> (x-y=w403:dbl[])
    n757 = Bundle By Name(cluster=w430, "Y"=w401) -> (w375:waveform(dbl))
    "Bead Separation" <- w375
    n758 = Divide(x=w403, y=2.0) -> (x/y=→"Vec Mean of T1 T2":dbl[])
    n759 = case shown="True" w410 {
      tunnel: w449 -> [_ w712]
      tunnel: w448 -> [_ w711]
      tunnel: w447 -> [_ w710]
      tunnel: w444 -> [_ w709]
      tunnel: w384 -> [_ w708]
      frame False {
      }
      frame True {
        n760 = property on="Force" class="WFChart (strict)"("YScale.NameLbl.Text"=w712) -> ()  [unwired: 2 in, 2 out]
        n761 = property on="T2 X" class="DigNum (strict)"("Caption.Text"=w710) -> ()  [unwired: 2 in, 2 out]
        n762 = property on="T1 X" class="DigNum (strict)"("Caption.Text"=w711) -> ()  [unwired: 2 in, 2 out]
        n763 = property on="Mean" class="DigNum (strict)"("Caption.Text"=w709) -> ()  [unwired: 2 in, 2 out]
        n764 = property on="Difference" class="DigNum (strict)"("Caption.Text"=w708) -> ()  [unwired: 2 in, 2 out]
      }
    }
    n765 = local read item#-1() -> ()  [unwired: 1 out]
    n766 = Subtract(x=w233, y=w232) -> (x-y=w446:dbl)
    n767 = Add(x=w233, y=w232) -> (x+y=→"Difference":dbl)
    n768 = feedback #18(w401) -> (w400:dbl[])
    n769 = Divide(x=w446, y=2.0) -> (x/y=w245:dbl)
    "Mean" <- w245
    n770 = case shown="True" {
      selector: _ -> [_ _]
      tunnel: w245 -> [_ w654]
      frame False {
      }
      frame True {
        n771 = Greater?(x="Lost Tether Alarm Threshold (pN)", y=w654) -> (0:w652:bool)
        n772 = case shown="True" w652 {
          frame False {
          }
          frame True {
            (unwired) FALSE ("Value (Signaling)")
            (unwired) FALSE ("Tether")
            n773 = flat-sequence {
              frame #0 {
                # "stop only if saving"
                n774 = local read item#-1() -> ()  [unwired: 1 out]
                n775 = And() -> ()  [unwired: 2 in, 1 out]
                n776 = local read item#-1() -> ()  [unwired: 1 in]
              }
              frame #1 {
                n777 = case shown="True" {
                  selector: _ -> [_ _]
                  frame False {
                  }
                  frame True {
                    (unwired) FALSE ("Fl. Triggered...")
                    n778 = local read item#-1() -> ()  [unwired: 1 in]
                  }
                }
              }
            }
            n779 = Get Date/Time In Seconds() -> (seconds since 1Jan1904=w660:timestamp)
            n780 = local read item#-1() -> ()  [unwired: 1 out]
            n781 = Subtract(x=w660) -> (x-y=w659:dbl)  [unwired: 1 in]
            n782 = Number To Decimal String(number=w659) -> (decimal integer string=w656:string)  [unwired: 1 out]
            n783 = call <vilib>:"Beep.vi"() -> ()  [unwired: 3 in, 9 out]
            n784 = local read item#-1() -> ()  [unwired: 1 out]
            n785 = Concatenate Strings("Lost tether (" ("Message to add"), w656, " s)." ("string")) -> (w658:string)
            n786 = call "Update messages.vi"("Message to add"=w658) -> ()  [unwired: 1 in, 1 out]
            n787 = local read item#-1() -> ()  [unwired: 1 in]
            n788 = local read item#-1() -> ()  [unwired: 1 in]
          }
        }
      }
    }
    n789 = Build Array (concatenate)(w401, w400) -> (w399:dbl[])
    n790 = Split 1D Array(array=w399, index=w289) -> (first subarray=w396:dbl[])  [unwired: 1 out]
    n791 = feedback-in #18(w396) -> ()
    n792 = call-poly <vilib>:"Mean.vi"("X"=w396) -> ("mean"=w395:dbl)  [unwired: 1 out]
    "Bead Mean (nm)" <- w395
    n793 = Subtract(x=w396, y=w395) -> (x-y=w394:dbl[])
    n794 = Square(x=w394) -> (x^2=w393:dbl[])
    n795 = case shown="True" "Semi Passive ON" {
      tunnel: "Semi Passive mode" -> [_ w551]
      tunnel: "Jump Force (pN)" -> [_ w550]
      tunnel: w245 -> [_ w549]
      frame False {
      }
      frame True {
        n796 = case shown="\"Use Feedback\"" w551 {
          tunnel: w550 -> [_ w554 w566]
          tunnel: w549 -> [_ w553 w565]
          frame "None" {
          }
          frame "Use Feedback" {
            n797 = local read "Target Force (pN)"() -> (w556:dbl)
            n798 = Less?(x=w554, y=w556) -> (x < y?=w555:bool)
            n799 = case shown="True" w555 {
              tunnel: w554 -> [w559 w562]
              tunnel: w553 -> [w558 w561]
              tunnel: [w557 w560] -> w552
              frame False {
                n800 = Less?(x=w559, y=w558) -> (x < y?=w557:bool)
              }
              frame True {
                n801 = Greater?(x=w562, y=w561) -> (0:w560:bool)
              }
            }
            n802 = case shown="True" w552 {
              frame False {
                n803 = local read item#-1() -> ()  [unwired: 1 out]
                n804 = case shown="True" {
                  selector: _ -> [_ _]
                  frame False {
                  }
                  frame True {
                    (unwired) FALSE
                  }
                }
              }
              frame True {
                n805 = local read item#-1() -> ()  [unwired: 1 out]
                n806 = case shown="False" {
                  selector: _ -> [_ _]
                  frame False {
                    (unwired) TRUE
                  }
                  frame True {
                  }
                }
              }
            }
          }
          frame "Sharp Jump" {
            n807 = local read "Target Force (pN)"() -> (w568:dbl)
            n808 = Greater?(x=w566, y=w568) -> (0:w567:bool)
            n809 = case shown="True" w567 {
              tunnel: w566 -> [w581 w585]
              tunnel: w565 -> [w582 w584]
              tunnel: [w580 w583] -> w564
              frame False {
                n810 = Greater?(x=w582, y=w581) -> (0:w580:bool)
              }
              frame True {
                n811 = Less?(x=w585, y=w584) -> (x < y?=w583:bool)
              }
            }
            n812 = Subtract(x=w566, y=w568) -> (x-y=w563:dbl)
            n813 = case shown="True" w564 {
              tunnel: w563 -> [_ w572]
              frame False {
              }
              frame True {
                n814 = local read "T1 kappa_x (pN/nm)"() -> (w577:dbl)
                n815 = local read "T2 kappa_x (pN/nm)"() -> (w578:dbl)
                n816 = Reciprocal(x="DNA stiffness (pN / nm)") -> (1/x=w574:dbl)
                n817 = Reciprocal(x=w577) -> (1/x=w576:dbl)
                n818 = Reciprocal(x=w578) -> (1/x=w575:dbl)
                n819 = Compound Arithmetic op=ADD(w576, w575, w574) -> (w573:dbl)
                n820 = local read "AOM X Cal (nm/MHz)"() -> (w571:dbl)
                n821 = Multiply(x=w573, y=w572) -> (x*y=w570:dbl)
                n822 = local read item#-1() -> ()  [unwired: 1 out]
                n823 = Divide(x=w570, y=w571) -> (x/y=w569:dbl)
                n824 = Subtract(y=w569) -> ()  [unwired: 1 in, 1 out]
              }
            }
          }
        }
      }
    }
    n825 = call-poly <vilib>:"Mean.vi"("X"=w393) -> ("mean"=w392:dbl)  [unwired: 1 out]
    n826 = Square Root(x=w392) -> (sqrt(x)=w391:dbl)
    n827 = Multiply(x=10.0, y=w391) -> (x*y=→"RMS (Ang)":dbl)
    n828 = xnode "Read/Write Control"("FPGA VI Reference In"=w423, "error in"=w422) -> ("FPGA VI Reference Out"=w529:T13, "error out"=w523:errorcluster, "AI2 Y Sum Set 1"=w520:i16, "AI2 Y Sum Set 2"=w519:i16, "AI1 X Set 1"=w322:fxp<+/-,16,1>, "AI1 X Set 2"=w321:fxp<+/-,16,1>, "Trap Pos FB Int Signal"=→"Trap Pos FB Int Signal":fxp<+/-,24,9>, "Trap Pos FB Int-Norm Signal"=→"Trap Pos FB Int-Norm Signal":fxp<+/-,16,1>, "Trap Pos FB Action"=w315:i64, "Scanning"=→"AOD Scanning":bool, "Scan I"=→"AOD Scan I":u64, "Scanning MCL"=w521:bool, "Scan I (MCL)"=→"MCL Scan I":u64, "Green FB Signals"=w463:T32, "BD1 amplitude 1 out"=w231:u16, "BD1 amplitude 2 out"=w216:u16)  [unwired: 1 out]
    "MCL Scanning" <- w521
    "Trap Pos FB Action" <- w315
    n829 = local read item#-1() -> ()  [unwired: 1 out]
    n830 = Bundle By Name("Set 1"=w520, "Set 2"=w519) -> (w517:cluster{})  [unwired: 1 in]
    n831 = Divide(x=w315, y=327.67) -> (x/y=→"Action (%)":dbl)
    n832 = local read "Trap X (AI1)"() -> (w335:T1)
    n833 = Divide(x=w517, y=3276.7) -> ()  [unwired: 1 out]
    n834 = local read item#-1() -> ()  [unwired: 1 in]
    n835 = Bundle(cluster=w335, "Trap 1"=w322, "Trap 2"=w321) -> (→"Trap X (AI1)":T1)
    n836 = Scale By Power Of 2(n=i16 12, x=ext 1.0) -> (x*2^n=w227:ext)
    n837 = Subtract(x=w227, y=ext 1.0) -> (x-y=w224:ext)
    n838 = Divide(x=w463, y=3276.7) -> (x/y=w459:T33)
    n839 = Multiply(x=w231, y=ext 100.0) -> (x*y=w225:ext)
    n840 = Unbundle By Name(w459) -> ("Green FB Ch 0"=w462:dbl, "Green FB Ch 1"=w461:dbl, "Green FB Ch 2"=w460:dbl)
    n841 = Divide(x=w225, y=w224) -> (x/y=w215:ext)
    "Trap 1 amplitude" <- w215
    n842 = Scale By Power Of 2(n=i16 12, x=ext 1.0) -> (x*2^n=w220:ext)
    n843 = local read item#-1() -> ()  [unwired: 1 out]
    n844 = Subtract(x=w220, y=ext 1.0) -> (x-y=w223:ext)
    n845 = Multiply(x=w216, y=ext 100.0) -> (x*y=w222:ext)
    n846 = Divide(x=w462, y=w460) -> (x/y=w458:dbl)
    n847 = Divide(x=w461, y=w460) -> (x/y=w457:dbl)
    n848 = flat-sequence "To save data" {
      tunnel: [w1514] -> w539
      tunnel: [w1515] -> w538
      tunnel: w493 -> [w1508]
      tunnel: _ -> [w1512]
      tunnel: ["Save Calibration"] -> w514
      tunnel: w511 -> [w1511]
      tunnel: [w1504] -> w510
      tunnel: [w1501] -> w509
      tunnel: [w1498] -> w508
      tunnel: w492 -> [w1500]
      tunnel: w408 -> [w1494]
      tunnel: [w1494] -> w407
      tunnel: ["Start Saving"] -> w377
      tunnel: [w1488] -> w304
      tunnel: [w1487] -> w303
      tunnel: w539 -> [w1716]
      tunnel: w538 -> [w1715]
      tunnel: w305 -> [w1714]
      tunnel: w514 -> [w1713]
      tunnel: w510 -> [w1712]
      tunnel: w509 -> [w1711]
      tunnel: w508 -> [w1710]
      tunnel: w386 -> [w1709]
      tunnel: _ -> [w1708]
      tunnel: w407 -> [w1707]
      tunnel: w377 -> [w1706]
      tunnel: w375 -> [w1705]
      tunnel: w351 -> [w1704]
      tunnel: w304 -> [w1703]
      tunnel: w303 -> [w1702]
      tunnel: w302 -> [w1701]
      frame #0 {
        n849 = Or(x="Save N Sets", y="Start Saving") -> (x .or. y?=w1495:bool)
        n850 = To Double Precision Float(number=w1511) -> (double precision float=w1505:dbl)
        n851 = Build Array(w1495, "Save Calibration", w1508, w1500) -> (w1510:bool[])
        n852 = Compound Arithmetic op=OR("Save Calibration", w1508, w1495, w1500) -> (w1513:bool)
        n853 = Boolean Array To Number(Boolean array=w1510) -> (number=w1507:u32)
        n854 = feedback #19(FALSE ("Save APD Data\nwith Trap Data")) -> (w1489:bool)
        n855 = feedback #20(refnum<k0> refnum) -> (w1516:refnum<file>)
        n856 = feedback #21(refnum<k0> refnum) -> (w1491:refnum<file>)
        n857 = feedback #22(FALSE ("Save APD Data\nwith Trap Data")) -> (w1499:bool)
        n858 = feedback #23(refnum<k0> refnum) -> (w1502:refnum<file>)
        n859 = feedback #24(0) -> (w1518:i32)
        n860 = feedback #25() -> (w1506:u32)  [unwired: 1 out]
        n861 = case shown="True" w1513 {
          tunnel: [w1525 1] -> w1514
          tunnel: w1518 -> [w1527 _]
          tunnel: [w1526 w1543] -> w1515
          tunnel: w1516 -> [w1526 _]
          tunnel: w1512 -> [_ w1562]
          tunnel: w1505 -> [_ w1561]
          tunnel: w1507 -> [_ w1563]
          tunnel: [w1524 w1542] -> w1504
          tunnel: w1506 -> [w1524 _]
          tunnel: [w1523 w1541] -> w1501
          tunnel: w1502 -> [w1523 _]
          tunnel: [w1522 w1540] -> w1498
          tunnel: w1499 -> [w1522 _]
          tunnel: "Start Saving" -> [_ w1538]
          tunnel: w1494 -> [_ w1537]
          tunnel: [w1521 w1529] -> w1487
          tunnel: w1491 -> [w1521 _]
          tunnel: [w1520 w1528] -> w1488
          tunnel: w1489 -> [w1520 _]
          frame False {
            n862 = Increment(x=w1527) -> (x+1=w1525:i32)
          }
          frame True {
            w1534 = FALSE ("Start Saving")
            w1539 = 9.0  # File Version
            (unwired) TRUE ("Saving...")
            w1546 = FALSE ("prepend array or string size? (T)")
            w1544 = T26."big-endian, network order" ("byte order (0:big-endian, network order)")
            # "write file headers"
            n863 = Array Size(array=w1537) -> (size(s)=w1536:i32)
            n864 = To Double Precision Float(number=w1536) -> (double precision float=w1535:dbl)
            n865 = local read item#-1() -> (w1560)
            n866 = local read item#-1() -> (w1559)
            n867 = local read item#-1() -> (w1558)
            n868 = local read item#-1() -> (w1557)
            n869 = local read item#-1() -> (w1556)
            n870 = local read item#-1() -> (w1555)
            n871 = local write "Save Calibration"(w1534) -> ()
            n872 = local write "Start Saving"(w1534) -> ()
            n873 = Build Array("Save APD Data\nwith Trap Data", "Save Trap Pos. Data") -> (w1531:bool[])
            n874 = Boolean Array To Number(Boolean array=w1531) -> (number=w1530:u32)
            n875 = Build Array(w1560, w1559, w1558, w1557, w1556, w1555) -> (w1554:void[])
            n876 = case shown="4" w1563 {
              tunnel: w1562 -> [_ _ _ _]
              tunnel: w1535 -> [w1634 w1652 w1673 w1699]
              tunnel: w1561 -> [w1633 w1651 w1672 w1698]
              tunnel: [w1631 w1648 w1666 w1692] -> w1552
              tunnel: [w1623 "Cal sets to save" w1661 w1687] -> w1542
              tunnel: w1554 -> [_ _ _ _]
              tunnel: "Save APD Data\nwith Trap Data" -> [w1630 _ w1658 w1685]
              tunnel: [w1630 w1641 w1658 w1685] -> w1540
              tunnel: w1539 -> [w1626 w1642 w1656 w1683]
              tunnel: w1538 -> [w1625 _ _ _]
              tunnel: [w1617 w1641 w1655 w1676] -> w1528
              tunnel: "Save Trap Pos. Data" -> [w1617 _ w1655 w1676]
              tunnel: w1530 -> [w1616 _ w1654 w1675]
              frame 1, Default {
                # "timeseries"
                n877 = case shown="True" {
                  selector: _ -> [_ _]
                  tunnel: [w1636 w1639] -> w1621
                  tunnel: [w1636 w1638] -> w1620
                  tunnel: [w1636 w1637] -> w1619
                  tunnel: [w1636 _] -> w1618
                  frame False {
                    w1636 = 0.0 ("f")
                  }
                  frame True {
                    n878 = local read "Current Position"() -> (w1640:dbl[])
                    n879 = local read item#-1() -> ()  [unwired: 1 out]
                    n880 = call "subVI_explode3array.vi"("Array"=w1640) -> ("x"=w1639:dbl, "y"=w1638:dbl, "z"=w1637:dbl)  [unwired: 12 in]
                  }
                }
                n881 = local read item#-1() -> ()  [unwired: 1 out]
                n882 = Multiply() -> (x*y=w1635:dbl)  [unwired: 2 in]
                n883 = To Double Precision Float(number=w1616) -> (double precision float=w1629:dbl)
                n884 = Build Array(w1626, w1635, w1634, w1633, 0.0 ("f")) -> (w1632:dbl[])  [unwired: 1 in]
                n885 = Build Array(w1629, w1621, w1620, w1619, w1618) -> (w1627:dbl[])
                n886 = Select(t=u32 4000000000, s=w1625, f="N sets to save") -> (s? t:f=w1623:u32)
                n887 = Build Array (concatenate)(w1632, w1627) -> (w1631:dbl[])  [unwired: 1 in]
              }
              frame 2 {
                w1644 = 0.0 ("f")
                w1641 = FALSE ("Save APD Data\nwith Trap Data")
                # "calibration"
                n888 = Boolean To (0,1)(Boolean=w1641) -> (0, 1=w1646:i16)
                n889 = To Double Precision Float(number=w1646) -> (double precision float=w1645:dbl)
                n890 = Build Array(w1645, w1644, w1644, w1644, w1644) -> (w1643:dbl[])
                n891 = Build Array(w1642, w1652, w1651, 1.0 ("t")) -> (w1649:dbl[])  [unwired: 2 in]
                n892 = Build Array (concatenate)(w1649, w1643) -> (w1648:dbl[])  [unwired: 1 in]
                "Calibrating Trap..." <- TRUE ("Calibrating...")
              }
              frame 4 {
                w1659 = 0.0 ("f")
                # "write file header for a trap \nraster scan"
                # "scan dir (x/y = 0/1)"
                # "cycles/step"
                # "n scans (f/b)"
                # "steps"
                # "freq. range"
                # "AOD raster scan"
                n893 = local read item#-1() -> ()  [unwired: 1 out]
                n894 = local read item#-1() -> ()  [unwired: 1 out]
                n895 = local read item#-1() -> ()  [unwired: 1 out]
                n896 = local read item#-1() -> ()  [unwired: 1 out]
                n897 = local read item#-1() -> ()  [unwired: 1 out]
                n898 = local read item#-1() -> ()  [unwired: 1 out]
                n899 = Boolean To (0,1)() -> (0, 1=w1670:i16)  [unwired: 1 in]
                n900 = To Double Precision Float() -> (double precision float=w1663:dbl)  [unwired: 1 in]
                n901 = To Double Precision Float() -> (double precision float=w1665:dbl)  [unwired: 1 in]
                n902 = To Double Precision Float() -> (double precision float=w1664:dbl)  [unwired: 1 in]
                n903 = To Double Precision Float(number=w1670) -> (double precision float=w1669:dbl)
                n904 = Multiply() -> (x*y=w1674:dbl)  [unwired: 2 in]
                n905 = To Double Precision Float(number=w1654) -> (double precision float=w1660:dbl)
                n906 = Build Array(w1660, w1659, w1659, w1659, w1659) -> (w1657:dbl[])
                n907 = Build Array(w1669, w1665, w1664, w1663) -> (w1667:dbl[])  [unwired: 1 in]
                n908 = Build Array(w1656, w1674, w1673, w1672, 2.0 ("t")) -> (w1668:dbl[])  [unwired: 1 in]
                n909 = local read item#-1() -> ()  [unwired: 1 out]
                n910 = Round Toward +Infinity() -> (ceil(x): smallest int >= x=w1662:dbl)  [unwired: 1 in]
                n911 = Build Array (concatenate)(w1668, w1657, w1667) -> (w1666:dbl[])  [unwired: 1 in]
                n912 = To Unsigned Long Integer(number=w1662) -> (unsigned 32bit integer=w1661:u32)
              }
              frame 8 {
                w1682 = 0.0 ("f")
                # "MCL raster scan"
                n913 = local read item#-1() -> (w1678)
                n914 = local read item#-1() -> (w1677)
                n915 = local read item#-1() -> ()  [unwired: 1 out]
                n916 = Select(t=w1677, f=w1678) -> (s? t:f=w1679:dbl)  [unwired: 1 in]
                n917 = local read item#-1() -> ()  [unwired: 1 out]
                n918 = Boolean To (0,1)() -> (0, 1=w1681:i16)  [unwired: 1 in]
                n919 = local read item#-1() -> ()  [unwired: 1 out]
                n920 = local read item#-1() -> ()  [unwired: 1 out]
                n921 = local read item#-1() -> ()  [unwired: 1 out]
                n922 = local read item#-1() -> ()  [unwired: 1 out]
                n923 = local read item#-1() -> ()  [unwired: 1 out]
                n924 = local read item#-1() -> ()  [unwired: 1 out]
                n925 = To Double Precision Float(number=w1681) -> (double precision float=w1680:dbl)
                n926 = Boolean To (0,1)() -> (0, 1=w1696:i16)  [unwired: 1 in]
                n927 = To Double Precision Float(number=w1679) -> (double precision float=w1689:dbl)
                n928 = To Double Precision Float() -> (double precision float=w1691:dbl)  [unwired: 1 in]
                n929 = To Double Precision Float() -> (double precision float=w1690:dbl)  [unwired: 1 in]
                n930 = To Double Precision Float(number=w1696) -> (double precision float=w1695:dbl)
                n931 = Multiply() -> (x*y=w1700:dbl)  [unwired: 2 in]
                n932 = To Double Precision Float(number=w1675) -> (double precision float=w1686:dbl)
                n933 = Build Array(w1686, w1680, w1682, w1682, w1682) -> (w1684:dbl[])
                n934 = Build Array(w1695, w1691, w1690, w1689) -> (w1693:dbl[])  [unwired: 3 in]
                n935 = Build Array(w1683, w1700, w1699, w1698, 3.0 ("t")) -> (w1694:dbl[])  [unwired: 1 in]
                n936 = local read item#-1() -> ()  [unwired: 1 out]
                n937 = Round Toward +Infinity() -> (ceil(x): smallest int >= x=w1688:dbl)  [unwired: 1 in]
                n938 = Build Array (concatenate)(w1694, w1684, w1693) -> (w1692:dbl[])  [unwired: 1 in]
                n939 = To Unsigned Long Integer(number=w1688) -> (unsigned 32bit integer=w1687:u32)
              }
            }
            n940 = local read item#-1() -> ()  [unwired: 1 out]
            n941 = call "Create new save file.vi"("Insert"="", "Ext"=".dat") -> ()  [unwired: 1 in, 2 out]
            n942 = local read item#-1() -> ()  [unwired: 1 in]
            n943 = local read item#-1() -> ()  [unwired: 1 in]
            n944 = local read item#-1() -> ()  [unwired: 1 in]
            n945 = Array Size(array=w1552) -> (size(s)=w1553:i32)
            n946 = Open/Create/Replace File(operation (0:open)=T25."create", access (0:read/write)=enum16{"read/write", "read-only", "write-only"}."write-only") -> (refnum out=w1565:refnum<file>)  [unwired: 2 in, 4 out]
            n947 = To Double Precision Float(number=w1553) -> (double precision float=w1551:dbl)
            n948 = local read item#-1() -> ()  [unwired: 1 in]
            n949 = String Length(string="Comment (data description)") -> (length=w1549:i32)
            n950 = To Double Precision Float(number=w1549) -> (double precision float=w1548:dbl)
            n951 = Deny Access(7:w1565) -> (3:w1564:refnum<file>)  [unwired: 1 in, 2 out]
            n952 = Build Array (concatenate)(w1551, w1552, w1548) -> (w1550:dbl[])
            n953 = case "If fluorescence data to be saved" shown="True" w1540 {
              tunnel: _ -> [_ w1615]
              tunnel: [refnum<k0> refnum w1595] -> w1541
              frame False {
              }
              frame True {
                w1594 = 0.0
                n954 = local read "APD Integration Time (s)"() -> (w1600:dbl)
                n955 = Path To String(path=w1615) -> (string=w1614:string)
                n956 = local read item#-1() -> ()  [unwired: 1 out]
                n957 = String Length(string=w1614) -> (length=w1613:i32)
                n958 = Subtract(x=w1613, y=4) -> (x-y=w1611:i32)
                n959 = String Subset(string=w1614, length (rest)=w1611) -> (substring=w1610:string)  [unwired: 1 out]
                n960 = Build Array(w1600, w1594, w1594, w1594, w1594, w1594, w1594) -> (w1597:dbl[])  [unwired: 1 in]
                n961 = Concatenate Strings(w1610, "_fl.dat" ("string")) -> (w1608:string)
                n962 = Array Size(array=w1597) -> (size(s)=w1599:i32)
                n963 = String To Path(string=w1608) -> (path=w1604:path)
                n964 = Open/Create/Replace File(file path (use dialog)=w1604, operation (0:open)=T25."create", access (0:read/write)=enum16{"read/write", "read-only", "write-only"}."write-only") -> (refnum out=w1605:refnum<file>)  [unwired: 1 in, 4 out]
                n965 = Deny Access(7:w1605) -> (3:w1601:refnum<file>)  [unwired: 1 in, 2 out]
                n966 = To Double Precision Float(number=w1599) -> (double precision float=w1598:dbl)
                n967 = Build Array (concatenate)(w1598, w1597) -> (w1596:dbl[])
                n968 = Write to Binary File(file (use dialog)=w1601, data=w1596, 5:FALSE ("prepend array or string size? (T)"), 9:T26."big-endian, network order" ("byte order (0:big-endian, network order)")) -> (refnum out=w1595:refnum<file>)  [unwired: 1 in, 3 out]
              }
            }
            n969 = case shown="True" w1528 {
              tunnel: _ -> [_ w1578]
              tunnel: [refnum<k0> refnum w1577] -> w1529
              frame False {
              }
              frame True {
                w1573 = 0.0 ("element")
                n970 = Path To String(path=w1578) -> (string=w1592:string)
                n971 = Build Array(w1573, w1573, w1573, w1573, w1573, w1573, w1573, w1573) -> (w1574:dbl[])
                n972 = String Length(string=w1592) -> (length=w1591:i32)
                n973 = Subtract(x=w1591, y=4) -> (x-y=w1589:i32)
                n974 = Array Size(array=w1574) -> (size(s)=w1576:i32)
                n975 = String Subset(string=w1592, length (rest)=w1589) -> (substring=w1588:string)  [unwired: 1 out]
                n976 = To Double Precision Float(number=w1576) -> (double precision float=w1575:dbl)
                n977 = Concatenate Strings(w1588, "_pos.dat" ("string")) -> (w1586:string)
                n978 = Build Array (concatenate)(w1575, w1574) -> (w1572:dbl[])
                n979 = String To Path(string=w1586) -> (path=w1582:path)
                n980 = Open/Create/Replace File(file path (use dialog)=w1582, operation (0:open)=T25."create", access (0:read/write)=enum16{"read/write", "read-only", "write-only"}."write-only") -> (refnum out=w1583:refnum<file>)  [unwired: 1 in, 4 out]
                n981 = Deny Access(7:w1583) -> (3:w1579:refnum<file>)  [unwired: 1 in, 2 out]
                n982 = Write to Binary File(file (use dialog)=w1579, data=w1572, 5:FALSE ("prepend array or string size? (T)"), 9:T26."big-endian, network order" ("byte order (0:big-endian, network order)")) -> (refnum out=w1577:refnum<file>)  [unwired: 1 in, 3 out]
              }
            }
            n983 = Write to Binary File(file (use dialog)=w1564, data=w1550, 5:w1546, 9:w1544) -> (refnum out=w1547:refnum<file>)  [unwired: 1 in, 3 out]
            n984 = Write to Binary File(file (use dialog)=w1547, data="Comment (data description)", 5:w1546, 9:w1544) -> (refnum out=w1543:refnum<file>)  [unwired: 1 in, 3 out]
          }
        }
        n985 = feedback-in #19(w1488) -> ()
        n986 = feedback-in #20(w1515) -> ()
        n987 = feedback-in #21(w1487) -> ()
        n988 = feedback-in #22(w1498) -> ()
        n989 = feedback-in #23(w1501) -> ()
        n990 = feedback-in #24(w1514) -> ()
        n991 = feedback-in #25(w1504) -> ()
      }
      frame #1 {
        n992 = local read item#-1() -> ()  [unwired: 1 out]
        n993 = case shown="True" {
          selector: _ -> [_ _]
          tunnel: w1716 -> [_ w1725]
          tunnel: w1715 -> [_ w1738]
          tunnel: w1714 -> [_ w1734]
          tunnel: w1713 -> [_ w1733]
          tunnel: w1712 -> [_ w1732]
          tunnel: w1711 -> [_ w1728]
          tunnel: w1710 -> [_ w1727]
          tunnel: w1709 -> [_ w1726]
          tunnel: w1708 -> [_ _]
          tunnel: w1707 -> [_ w1723]
          tunnel: w1706 -> [_ w1722]
          tunnel: w1705 -> [_ w1721]
          tunnel: w1704 -> [_ w1720]
          tunnel: w1703 -> [_ w1719]
          tunnel: w1702 -> [_ w1718]
          tunnel: w1701 -> [_ w1717]
          frame False {
          }
          frame True {
            n994 = Multiply(x=w1725) -> (x*y=→"Time (s)":i32)  [unwired: 1 in]
            n995 = Less Or Equal?(x=w1725, y=w1732) -> (x <= y?=w1736:bool)
            n996 = Or(y="Abort save 2") -> (x .or. y?=w1729:bool)  [unwired: 1 out]
            n997 = Not(x=w1729) -> (.not. x?=w1737:bool)
            n998 = And(x=w1736, y=w1737) -> (x .and. y?=w1735:bool)
            n999 = case shown="True" w1735 {
              tunnel: w1738 -> [w1744 w1810]
              tunnel: [0.0 w1813] -> w1731
              tunnel: w1725 -> [_ w1811]
              tunnel: w1732 -> [_ w1812]
              tunnel: w1734 -> [_ w1807]
              tunnel: w1733 -> [_ _]
              tunnel: w1728 -> [w1742 w1800]
              tunnel: w1727 -> [w1741 w1801]
              tunnel: w1726 -> [_ w1799]
              tunnel: w1723 -> [_ w1798]
              tunnel: w1722 -> [_ w1753]
              tunnel: w1721 -> [_ w1791]
              tunnel: w1720 -> [_ w1769]
              tunnel: w1719 -> [w1739 w1751]
              tunnel: w1718 -> [w1740 w1750]
              tunnel: w1717 -> [_ w1748]
              frame False {
                (unwired) FALSE
                n1000 = Close File(refnum=w1744) -> ()  [unwired: 1 in, 2 out]
                n1001 = case shown="True" w1741 {
                  tunnel: w1742 -> [_ w1746]
                  frame False {
                  }
                  frame True {
                    n1002 = Close File(refnum=w1746) -> ()  [unwired: 1 in, 2 out]
                  }
                }
                n1003 = case shown="True" w1739 {
                  tunnel: w1740 -> [_ w1745]
                  frame False {
                  }
                  frame True {
                    n1004 = Close File(refnum=w1745) -> ()  [unwired: 1 in, 2 out]
                  }
                }
                n1005 = local read "Calibrating Trap..."() -> ()  [unwired: 1 in]
                n1006 = call <vilib>:"Beep.vi"() -> ()  [unwired: 3 in, 9 out]
                n1007 = local read item#-1() -> ()  [unwired: 1 in]
              }
              frame True {
                n1008 = local read "Calibrating Trap..."() -> (w1802:bool)
                n1009 = case "Write fl. data" shown="True" w1801 {
                  tunnel: w1800 -> [_ w1834]
                  tunnel: w1799 -> [_ w1833]
                  frame False {
                  }
                  frame True {
                    n1010 = Write to Binary File(file (use dialog)=w1834, data=w1833, 5:FALSE ("prepend array or string size? (T)"), 9:T26."big-endian, network order" ("byte order (0:big-endian, network order)")) -> ()  [unwired: 1 in, 4 out]
                  }
                }
                n1011 = Greater?(y=1.0) -> (0:w1805:bool)  [unwired: 1 in]
                n1012 = Not(x=w1802) -> (.not. x?=w1804:bool)
                n1013 = And(x=w1804, y=w1805) -> (x .and. y?=w1749:bool)
                n1014 = case shown="True" w1749 {
                  tunnel: w1748 -> [w1816 w1826]
                  tunnel: [w1816 w1819] -> w1747
                  frame False {
                  }
                  frame True {
                    w1817 = 2 ("dimension size")
                    n1015 = Array Size(array=w1826) -> (size(s)=w1820:i32)
                    n1016 = Divide(x=w1820, y=w1817) -> (x/y=w1824:dbl)
                    n1017 = Reshape Array(w1826, w1824, w1817) -> (w1825:u64[][])
                    n1018 = Transpose 2D Array(2D array=w1825) -> (transposed array=w1823:u64[][])
                    n1019 = for {
                      tunnel: w1823 -> [w1828] mode=indexing
                      tunnel: [w1827] -> w1818 mode=indexing
                      workers-P: _ -> [_]
                      n1020 = call "downsample 1D array - U64.vi"("Array In"=w1828) -> ("Array Out"=w1827:u64[])  [unwired: 2 in]
                    }
                    n1021 = Transpose 2D Array(2D array=w1818) -> (transposed array=w1822:u64[][])
                    n1022 = Divide(x=w1820) -> (x/y=w1821:dbl)  [unwired: 1 out]
                    n1023 = Reshape Array(w1822, w1821) -> (w1819:u64[])
                  }
                }
                n1024 = case shown="True" w1749 {
                  tunnel: w1807 -> [w1837 w1848]
                  tunnel: [w1837 w1841] -> w1803
                  tunnel: w1798 -> [_ w1840]
                  frame False {
                    # "don't downsample data for trap calibration"
                  }
                  frame True {
                    n1025 = Array Size(array=w1848) -> (size(s)=w1842:i32)
                    n1026 = Array Size(array=w1840) -> (size(s)=w1839:i32)
                    n1027 = Divide(x=w1842, y=w1839) -> (x/y=w1846:dbl)
                    n1028 = Reshape Array(w1848, w1846, w1839) -> (w1847:i16[][])
                    n1029 = Transpose 2D Array(2D array=w1847) -> (transposed array=w1845:i16[][])
                    n1030 = for {
                      tunnel: w1845 -> [w1850] mode=indexing
                      tunnel: [w1849] -> w1838 mode=indexing
                      workers-P: _ -> [_]
                      n1031 = call "downsample 1D array - I16.vi"("Array In"=w1850) -> ("Array Out"=w1849:i16[])  [unwired: 1 in, 1 out]
                    }
                    n1032 = Transpose 2D Array(2D array=w1838) -> (transposed array=w1844:i16[][])
                    n1033 = Divide(x=w1842) -> (x/y=w1843:dbl)  [unwired: 1 out]
                    n1034 = Reshape Array(w1844, w1843) -> (w1841:i16[])
                  }
                }
                n1035 = Index Array(array=w1769, index=1) -> (element=w1772:waveform(dbl))
                n1036 = Index Array(array=w1769, index=0) -> (element=w1774:waveform(dbl))
                n1037 = Unbundle By Name(w1772) -> ("Y"=w1776:dbl[])
                n1038 = Unbundle By Name(w1774) -> ("Y"=w1784:dbl[])
                n1039 = case "Write trap pos. data" shown="True" w1751 {
                  tunnel: w1750 -> [_ w1830]
                  tunnel: w1747 -> [_ w1829]
                  frame False {
                  }
                  frame True {
                    n1040 = Write to Binary File(file (use dialog)=w1830, data=w1829, 5:FALSE ("prepend array or string size? (T)"), 9:T26."big-endian, network order" ("byte order (0:big-endian, network order)")) -> ()  [unwired: 1 in, 4 out]
                  }
                }
                n1041 = Write to Binary File(file (use dialog)=w1810, data=w1803, 5:FALSE ("prepend array or string size? (T)"), 9:T26."big-endian, network order" ("byte order (0:big-endian, network order)")) -> ()  [unwired: 1 in, 4 out]
                n1042 = feedback #26(w1776) -> (w1778:dbl[])
                n1043 = Build Array (concatenate)(w1778, w1776) -> (w1777:dbl[])
                n1044 = Select(t=w1776, s=w1753, f=w1777) -> (s? t:f=w1763:dbl[])
                n1045 = feedback-in #26(w1763) -> ()
                n1046 = feedback #27(w1784) -> (w1797:dbl[])
                n1047 = Build Array (concatenate)(w1797, w1784) -> (w1796:dbl[])
                n1048 = Select(t=w1784, s=w1753, f=w1796) -> (s? t:f=w1771:dbl[])
                n1049 = feedback-in #27(w1771) -> ()
                n1050 = Divide(x=w1811, y=w1812) -> (x/y=w1814:dbl)
                n1051 = Multiply(x=w1814, y=100.0) -> (x*y=w1813:dbl)
                n1052 = Build Array(w1771, w1763) -> (→"Saved APD":dbl[][])
                n1053 = Array Size(array=w1771) -> (size(s)=w1789:i32)
                n1054 = Unbundle By Name(w1791) -> ("Y"=w1795:dbl[])
                n1055 = Subtract(x=w1789) -> (x-y=w1765:i32)  [unwired: 1 in]
                n1056 = Multiply(y=u16 2) -> (x*y=w1766:u16)  [unwired: 1 in]
                n1057 = Subtract(x=w1789, y=w1766) -> (x-y=w1764:i32)
                n1058 = feedback #28(w1795) -> (w1794:dbl[])
                n1059 = Build Array (concatenate)(w1794, w1795) -> (w1793:dbl[])
                n1060 = Select(t=w1795, s=w1753, f=w1793) -> (s? t:f=w1792:dbl[])
                "Trap Delta Graph" <- w1792
                n1061 = feedback-in #28(w1792) -> ()
                n1062 = Array Subset(array=w1771, index=w1765) -> (w1788:dbl[])  [unwired: 1 in]
                n1063 = Array Subset(array=w1771, index=w1764) -> (w1787:dbl[])  [unwired: 1 in]
                n1064 = Array Subset(array=w1763, index=w1765) -> (w1768:dbl[])  [unwired: 1 in]
                n1065 = Array Subset(array=w1763, index=w1764) -> (w1767:dbl[])  [unwired: 1 in]
                n1066 = call-poly <vilib>:"Mean.vi"("X"=w1788) -> ("mean"=w1786:dbl)  [unwired: 1 out]
                n1067 = call-poly <vilib>:"Mean.vi"("X"=w1768) -> ("mean"=w1762:dbl)  [unwired: 1 out]
                n1068 = call-poly <vilib>:"Mean.vi"("X"=w1787) -> ("mean"=w1785:dbl)  [unwired: 1 out]
                n1069 = call-poly <vilib>:"Mean.vi"("X"=w1767) -> ("mean"=w1761:dbl)  [unwired: 1 out]
                n1070 = Subtract(x=w1762, y=w1761) -> (x-y=w1752:dbl)
                "Delta Fl. 2" <- w1752
                n1071 = Subtract(x=w1786, y=w1785) -> (x-y=w1783:dbl)
                "Delta Fl. 1" <- w1783
                n1072 = Initialize Array(w1783, 1 ("dimension size")) -> (w1780:dbl[])
                n1073 = Initialize Array(w1752, 1 ("dimension size")) -> (w1758:dbl[])
                n1074 = feedback #29(w1780) -> (w1781:dbl[])
                n1075 = Build Array (concatenate)(w1781, w1780) -> (w1779:dbl[])
                n1076 = feedback #30(w1758) -> (w1759:dbl[])
                n1077 = Build Array (concatenate)(w1759, w1758) -> (w1757:dbl[])
                n1078 = Select(t=w1780, s=w1753, f=w1779) -> (s? t:f=w1756:dbl[])
                n1079 = feedback-in #29(w1756) -> ()
                n1080 = Select(t=w1758, s=w1753, f=w1757) -> (s? t:f=w1755:dbl[])
                n1081 = feedback-in #30(w1755) -> ()
                n1082 = Build Array(w1756, w1755) -> (→"Save APD Deriv":dbl[][])
              }
            }
            "Progress" <- w1731
            "Progress 2" <- w1731
          }
        }
      }
    }
    n1083 = Divide(x=w222, y=w223) -> (x/y=w214:ext)
    "Trap 2 amplitude" <- w214
    n1084 = Bundle By Name(cluster=w459, "Green FB Ch 0"=w458, "Green FB Ch 1"=w457) -> (w443:T33)
    "Green FB Signals (V)" <- w443
    n1085 = case shown="True" {
      selector: _ -> [_ _]
      tunnel: w215 -> [_ w544]
      tunnel: w214 -> [_ w543]
      frame False {
      }
      frame True {
        w545 = 50.0
        n1086 = Greater?(x=w543, y=w545) -> (0:w541:bool)
        n1087 = Greater?(x=w544, y=w545) -> (0:w542:bool)
        n1088 = Or(x=w542, y=w541) -> (x .or. y?=w540:bool)
        n1089 = case shown="True" w540 {
          frame False {
          }
          frame True {
            (unwired) FALSE
            "Feedback overload" <- TRUE
          }
        }
      }
    }
    n1090 = Unbundle By Name(w443) -> ("Green FB Ch 2"=→"Green FB Plot":dbl)
    n1091 = local read "wait to reset values"() -> (w524:bool)
    n1092 = Not(x=w521) -> (.not. x?=w525:bool)
    n1093 = And(x=w525, y=w524) -> (x .and. y?=w526:bool)
    n1094 = case "Part of MCL raster scanning: returns to initial positions after scan done" shown="True" w526 {
      tunnel: w529 -> [w1326 w1331]
      tunnel: [w1326 w1330] -> w528
      tunnel: w523 -> [w1325 w1329]
      tunnel: [w1325 w1328] -> w522
      frame False {
      }
      frame True {
        w1337 = 10.0 ("y")
        w1336 = 32767.0 ("y")
        # "to return scan values\nafter a synchronous \nAOM scan"
        n1095 = local read item#-1() -> ()  [unwired: 1 out]
        n1096 = local read item#-1() -> ()  [unwired: 1 out]
        n1097 = local write "wait to reset values"(FALSE ("wait to reset values")) -> ()
        n1098 = Multiply(y=w1336) -> (x*y=w1333:dbl)  [unwired: 1 in]
        n1099 = Multiply(y=w1336) -> (x*y=w1335:dbl)  [unwired: 1 in]
        n1100 = Divide(x=w1333, y=w1337) -> (x/y=w1332:dbl)
        n1101 = Divide(x=w1335, y=w1337) -> (x/y=w1334:dbl)
        n1102 = To Word Integer(number=w1332) -> (16bit integer=w1338:i16)
        n1103 = To Word Integer(number=w1334) -> (16bit integer=w1339:i16)
        n1104 = local read item#-1() -> ()  [unwired: 1 out]
        n1105 = xnode "Read/Write Control"("FPGA VI Reference In"=w1331, "error in"=w1329, "AO1 (Y)"=w1338, "AO2 (X)"=w1339) -> ("FPGA VI Reference Out"=w1330:T13, "error out"=w1328:errorcluster)  [unwired: 1 in]
        n1106 = local read item#-1() -> ()  [unwired: 1 out]
      }
    }
    n1107 = node-c288() -> ()  [unwired: 2 out]
  }
  n1108 = node-c288(w114) -> ()  [unwired: 1 out]
  n1109 = flat-sequence {
    tunnel: w39 -> [w1855]
    tunnel: [w1854] -> w41
    tunnel: [w1851] -> w40
    tunnel: w38 -> [w1852]
    tunnel: w41 -> [w1858]
    tunnel: w40 -> [w1857]
    frame #0 {
      w1853 = FALSE ("APD to FIFO")
      n1110 = xnode "Read/Write Control"("FPGA VI Reference In"=w1855, "error in"=w1852, "APD to FIFO"=w1853, "AI to FIFO"=w1853) -> ("FPGA VI Reference Out"=w1854:T13, "error out"=w1851:errorcluster)
    }
    frame #1 {
      n1111 = xnode "Invoke Method"("FPGA VI Reference In"=w1858, "error in"=w1857) -> ("FPGA VI Reference Out"=w1856:T13)  [unwired: 1 out]
      n1112 = xnode "Close FPGA VI Reference"("FPGA VI Reference In"=w1856) -> ()  [unwired: 1 in, 1 out]
    }
  }
  "X RF Amplitude Limits (%)" <- w88
  "Y RF Amplitude Limits (%)" <- w86
